vi "main4Ch v2.0.2.vi"() -> ()   [LabVIEW 2024]
doc: "Main VI for FLS imaging system."
uses:
  SubVI/DigitizerConfiguration/FLImDAQ.ctl
  <instrlib>/niScope/Controls/niScope trigger source.ctl
  SubVI/LabJack/LJ Pin Setting.ctl
  ConfigFiles/AimingBeamVideoConfig.ctl
  LaguerreDeconLib/DeconEngineClass/LaguerreDeconEngineClass.lvclass/LaguerreDeconEngineClass.ctl
  <vilib>/Utility/error.llb/DialogType.ctl
  LaguerreDeconLib/DeconEngineClass/LaguerreDeconEngineClass.lvclass
  <vilib>/event_ctls.llb/usereventprio.ctl
  <vilib>/Utility/miscctls.llb/LVMinMaxIncTypeDef.ctl
  SubVI/APD/APDClass.lvclass
  <vilib>/Analysis/baseanly.llb/Mean (DBL).vi
  SubVI/GlobalVariables.vi
  <vilib>/addons/control/pid/pid.llb/PID (DBL).vi
  <instrlib>/niScope/Acquire/Fetch/niScope Multi Fetch Binary 16.vi
  <vilib>/Instr/_visa.llb/VISA Configure Serial Port (Instr).vi
  <vilib>/Python/Open Anaconda Python Session.vi
  C:/Users/MarcuLab/Documents/GitHub/NetDeconForLV/Source/DotNETAssembly1.0.3/output/build/LaguerreDeconRTNative.dll
  Documents/GitHub/NetDeconForLV/Source/DotNETAssembly1.0.3/output/build/LaguerreDeconRTNative.dll
  <userlib>/_OpenG.lib/file/file.llb/openg_file.lvlib
  <userlib>/_OpenG.lib/time/time.llb/openg_time.lvlib
  <vilib>/Analysis/NI_AALBase.lvlib
  <vilib>/Utility/miscctls.llb/LVPointTypeDef.ctl
  <vilib>/addons/control/pid/NI_PID_pid.lvlib
panel:
  out "error out":errorcluster
  in  "488nm Power":u16(ring)=32 items=["3.30mW"=60, "2.35mW"=50, "2.00mW"=47, "1.75mW"=44, "1.48mW"=41, "1.16mW"=38, "0.87mW"=35, "0.57mW"=32, "0.28mW"=29]
  out "Decon Loop timing (ms)":dbl
  out "Ch3 Lifetime (ns)":dbl caption="Lifetime (ns)"
  out "Ch2 Lifetime (ns)":dbl caption="Lifetime (ns)"
  out "Ch1 Lifetime (ns)":dbl caption="Lifetime (ns)"
  out "Cancer Prob":dbl
  in  "Overlay selection":u16(ring) items=["Gain", "Lifetime", "CancerProbability"]
  out "Record Backlog 2":i32
  in  "Auto gain ch4":bool=TRUE caption="Auto gain ch3"
  in  "V 4":dbl caption="Gain 3" min=0.0 max=4.67 step=0.1
  out "Gain4":dbl
  out "IntR4":dbl format="%#_2g"
  out "SNR4":dbl format="%#_3g"
  out "Channel 4":dbl[][](graph) caption="Channel 3"
  out "RunStartTime":u32
  out "Dig1 Temp":dbl
  out "Dig2 Temp":dbl
  out "Visualization PC video source":T1
  in  "V target(1.0)":dbl=1.0 caption="V target(1.5)" min=0.3 max=1.5 step=0.1 format="%#_4g"
  out "SNR3":dbl format="%#_3g"
  out "SNR2":dbl format="%#_3g"
  out "SNR1":dbl format="%#_3g"
  in  "Show BG removed?":bool=TRUE
  out "IntR3":dbl format="%#_2g"
  out "IntR2":dbl format="%#_2g"
  out "IntR1":dbl format="%#_2g"
  in  "Video Display":bool
  out "Gain3":dbl
  out "Gain2":dbl
  out "Gain1":dbl
  in  "Skip Data Save?":bool
  out "Aq Loop?":bool
  out "ML?":bool
  out "aquisition loop Error Out":errorcluster
  out "Laser f (Hz)":dbl
  out "Record Backlog":i32
  out "Fetch Record #":i32
  out "Sync Success?":bool
  out "Disclamer":picture
  out "Calibration #":i8
  out "BG #":i8
  in  "TCP Connect":bool
  out "Help":string
  in  "355nm Laser toggle":bool caption="355nm 460Hz"
  in  "Cali&iRF alignment":bool
  in  "Background":bool
  in  "Aiming beam toggle":bool caption="488nm 0Hz"
  in  "Auto gain ch3":bool=TRUE
  in  "Auto gain ch2":bool=TRUE
  in  "Auto gain ch1":bool=TRUE
  out "Run #":i8
  in  "StopButton":bool caption="Stop"
  out "Aquisition Status:":bool
  in  "StartButton":bool caption="Start"
  in  "V 3":dbl caption="Gain 3" min=0.0 max=4.65 step=0.1
  in  "V 2":dbl caption="Gain 2" min=0.0 max=4.59 step=0.1
  in  "V 1":dbl caption="Gain 1" min=0.0 max=4.63 step=0.1 format="%#_4g"
  in  "Video Source":enum32{"Camera", "FrameGrabber"}(radio)
  out "Case #":string
  out "System Hardware Connection Status":T2
  out "Channel 3":dbl[][](graph)
  out "Channel 2":dbl[][](graph)
  out "Channel 1":dbl[][](graph)
  in  "Tab Control":T3(tab)
  out "display loop timing(ms)":u32
  out "Aquisition loop timing(ms)":u32 format="%.2f"
  out "DisplayLoop":i32
  out "PID loop":i32 caption="processing loop"
  out "PID loop timing(ms)":u32 caption="processing loop timing(ms)"
  out "Communication loop(ms)":u32
  out "laser EM lamp V":dbl format="%0.6f"
  out "Auisition Loop idx":i32
  out "LJ process (ms)":u32
  out "LJ time(ms)":u32[](array[numeric])
  out "output variable":i32
  out ".NetInitialized?":bool
  out "BG Graph":dbl[][](graph)
  out "Lifetime (ns)":cluster{dbl, dbl, dbl}(graph)
  out "DeCon Speed(ms)":dbl(graph)
  out "iRF Graph":dbl[][](graph)
  in  "Show BG":bool
  out "iRF length":i32
  out "BG length":i32
  out "data length":i32
  out "WarmupTime(ms)":u32
  out "BGAll":dbl[][](array[numeric])
  out "DeConOut":dbl[](array[numeric])
  in  "Ch1GainLim":dbl=350.0 format="%#_13g"
  in  "Ch2GainLim":dbl=1750.0 format="%#_13g"
  in  "Ch3GainLim":dbl=1750.0
  out "LJ Pinout":T4={"Ch1 Bias"="DAC0", "Ch2 Bias"="DAC1", "Ch3 Bias"="DAC2", "Ch4 Bias"="DAC0", "355 PWM"="FIO0", "AimingBeam PWM"="FIO2", "Laser Ready"="FIO3", "Interlock"="FIO1", "Laser Start/Stop"="FIO1", "Red LED"="FIO1", "Green LED"="DIO3", "Foot Pedal"="DIO15"}
  out "FLImDAQ":T5={"Digitizer 1"="", "Digitizer 2"="", "Channel"=enum."Channel 0", "trigger source"="VAL_EXTERNAL", "trigger level"=0.5, "trigger delay"=1.35e-07, "min sample rate"=12500000000.0, "min record length"=2500, "vertical range"=1.0, "vertical offset"=-0.25, "Waveform to Avg"=2000} caption="FLIm DAQ Configuration" {"trigger delay" format="%^#.4e"; "trigger level" min=0.0 max=3.5 step=0.5 format="%.2f"; "vertical offset" format="%.4f"; "vertical range" format="%.2f"; "min sample rate" format="%#.2p"}
  in  "Sys Reconfig":bool
  out "data out(communcation loop)":string
  out "PID loop error out":errorcluster caption="processing Error Out"
  out "decon error out":errorcluster
  out "Laser Rep Rate":dbl
  out "V4 Size":i32 caption="V3 Size"
  in  "Data Class":enum16{"Data", "BG", "Cali"}(ring)=enum."BG"
  out "V1 Size":i32
  out "V2 Size":i32
  out "V3 Size":i32
  out "data Size":i32[](array[numeric])
  out "State log":string
  out "SysConfigCluster":T7
  in  "Ch4 PID gains":T8={"proportional gain (Kc)"=30.0, "integral time (Ti, min)"=0.0003, "derivative time (Td, min)"=1e-05}
  in  "Ch3 PID gains":T8={"proportional gain (Kc)"=30.0, "integral time (Ti, min)"=0.0003, "derivative time (Td, min)"=1e-05}
  in  "Ch2 PID gains":T8={"proportional gain (Kc)"=30.0, "integral time (Ti, min)"=0.0003, "derivative time (Td, min)"=1e-05}
  in  "Ch1 PID gains":T8={"proportional gain (Kc)"=30.0, "integral time (Ti, min)"=0.0003, "derivative time (Td, min)"=1e-05}
  in  "Brain model path":path=path "C:/Users/MarcuLab/Desktop/V6 APD LV/V6 APD LV/ClassifierFile/Brain_Agnostic_Model.pkl"
  in  "module path":path=path "C:/Users/MarcuLab/Documents/GitHub/NetDeconForLV/Classifier/ClassifierModule.py"
  in  "HN model path":path=path "C:/Users/MarcuLab/Desktop/V6 APD LV/V6 APD LV/ClassifierFile/xgb_model.pkl"
  in  "Env name":string="HNClassifier"
  in  "Python version":string="3.10"
  out "Python session":refnum<k35>
  out "OverlaySelection":T9(ring)=enum."HN Classifier"
  in  "CancerThreshold":dbl=0.15
  in  "Quit":bool
  in  "Radio Buttons":T10(radio)=enum."Ch2" caption="DeCon Chan"
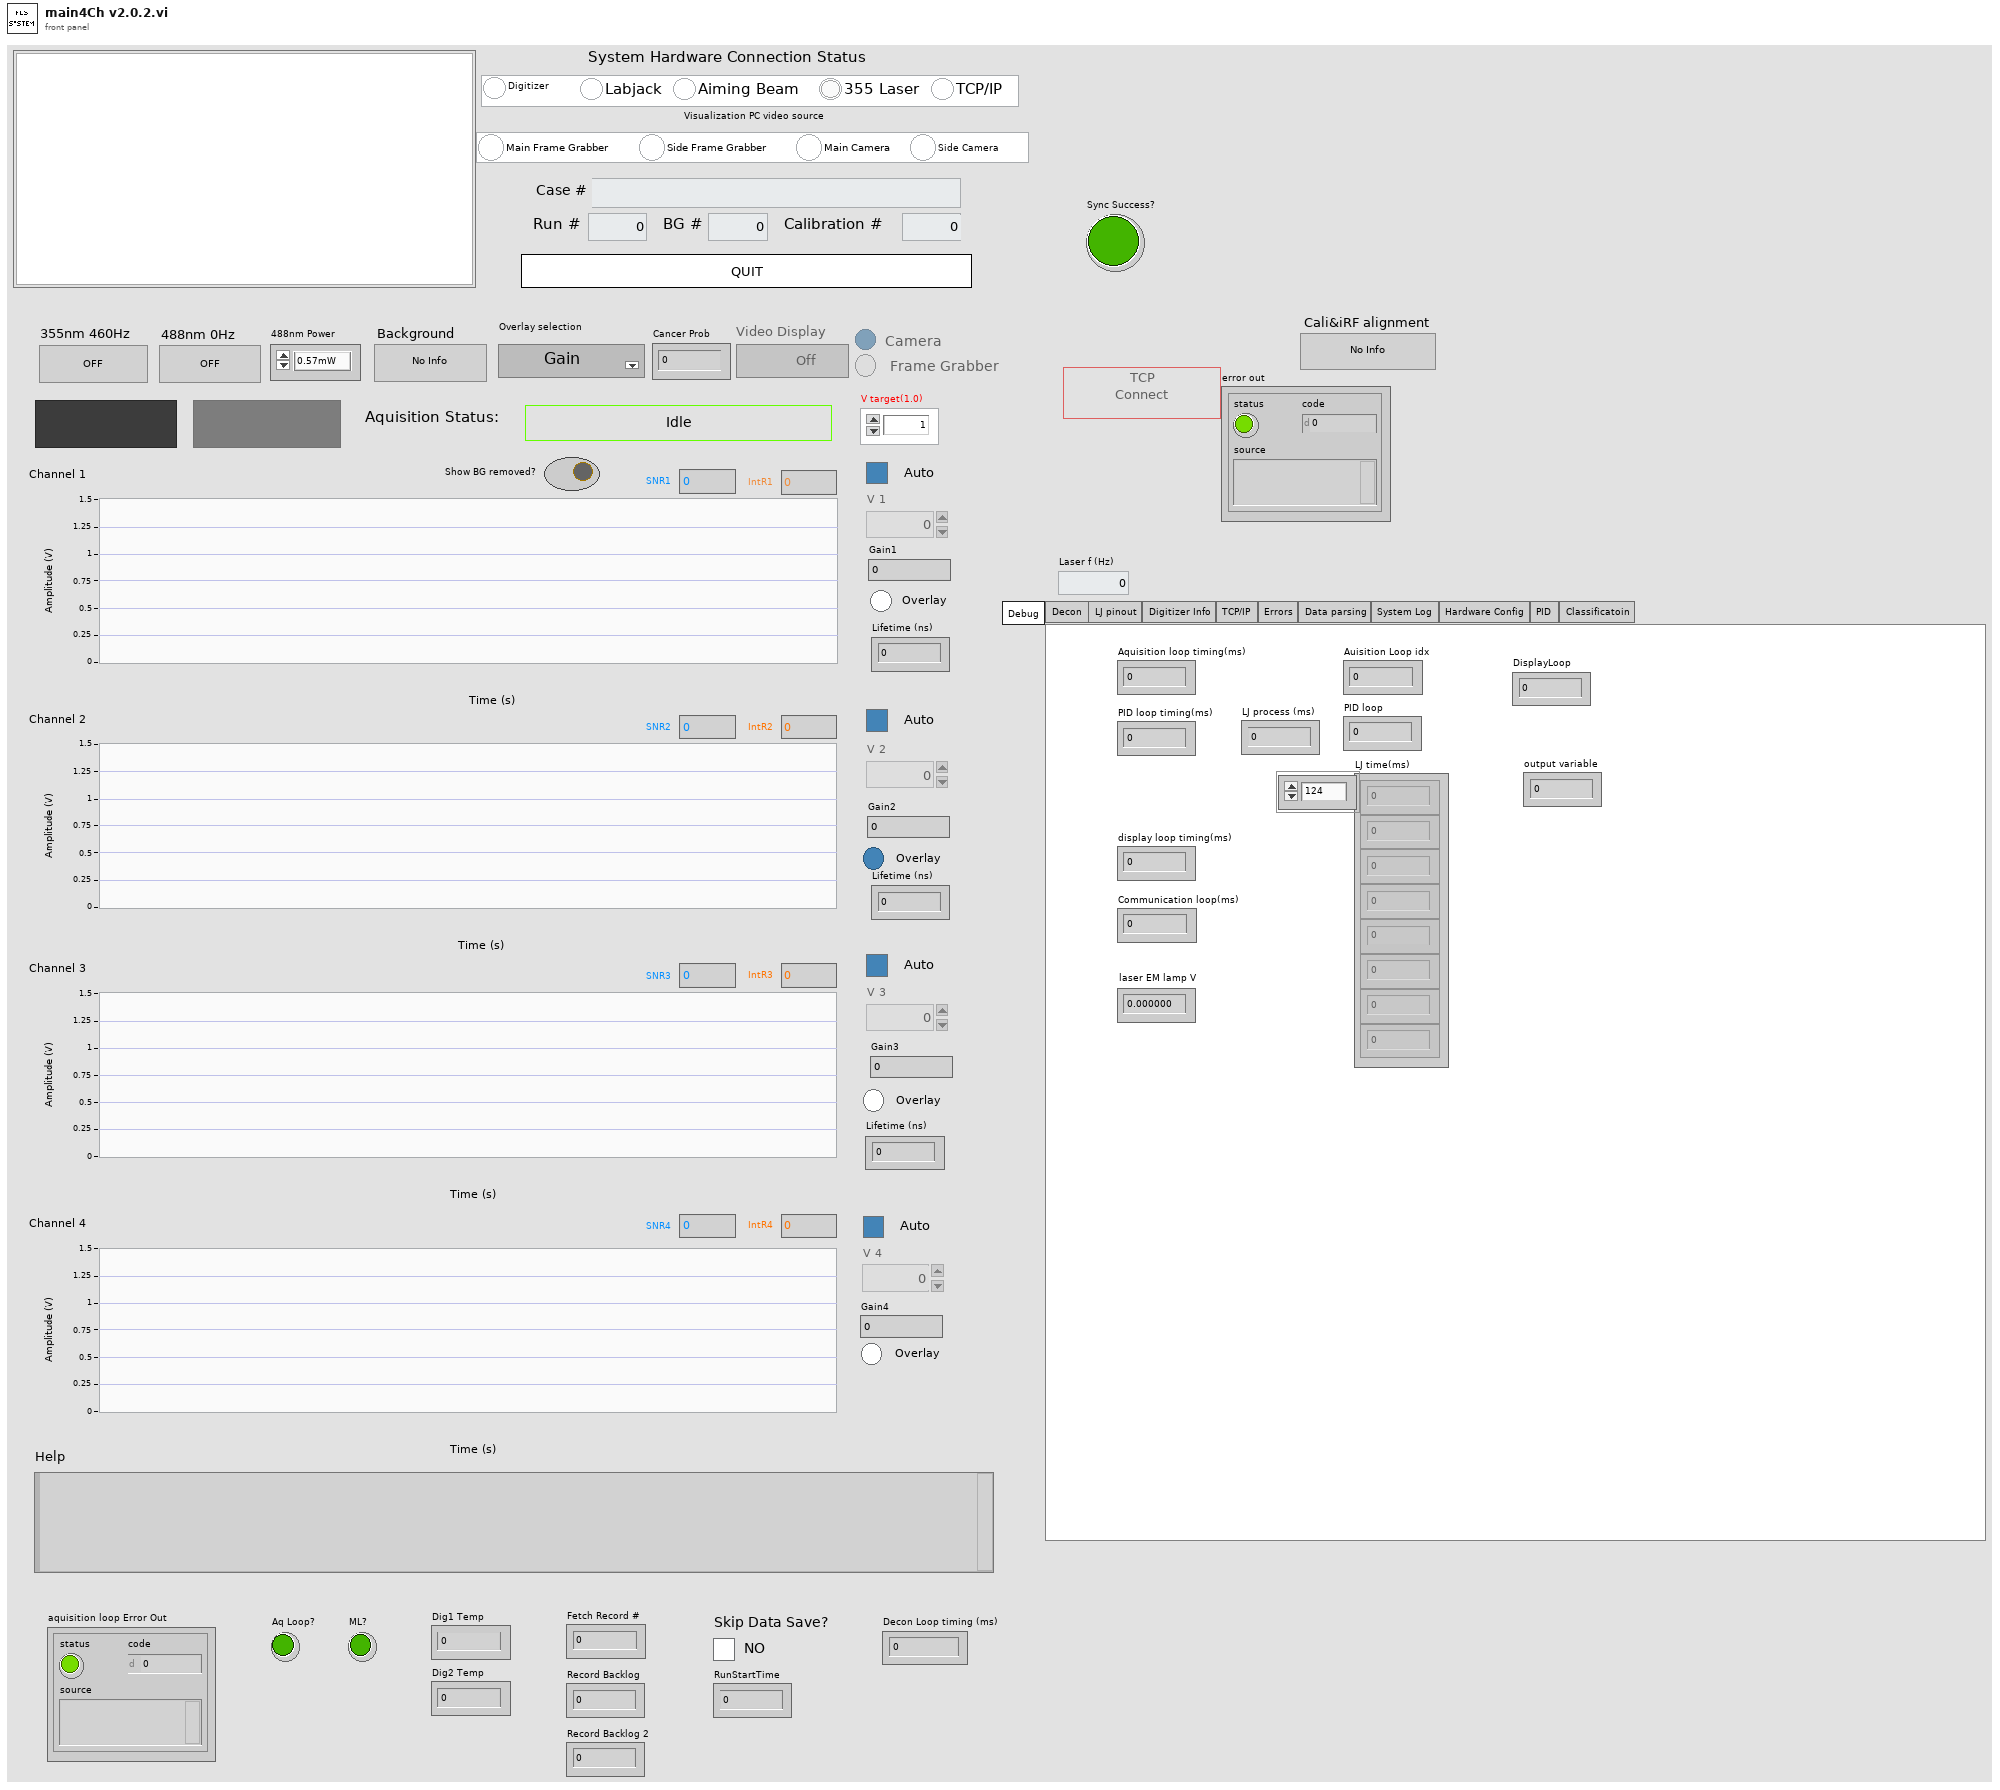
[diagram p1: front panel]
types:
  T1 = cluster{"Main Frame Grabber":bool, "Side Frame Grabber":bool, "Main Camera":bool, "Side Camera":bool}
  T2 = cluster{"Digitizer":bool, "Labjack":bool, "Aiming Beam":bool, "355 Laser":bool, "TCP/IP":bool}
  T3 = enum32{"Debug", "Decon", "LJ pinout", "Digitizer Info", "TCP/IP", "Errors", "Data parsing", "System Log", "Hardware Config", "PID", "Classificatoin"}
  T4 = typedef "LJ Pin Setting.ctl" = cluster{"Ch1 Bias":string, "Ch2 Bias":string, "Ch3 Bias":string, "Ch4 Bias":string, "355 PWM":string, "AimingBeam PWM":string, "Laser Ready":string, "Interlock":string, "Laser Start/Stop":string, "Red LED":string, "Green LED":string, "Foot Pedal":string}
  T5 = typedef "FLImDAQ.ctl" = cluster{"Digitizer 1":refnum<k15>, "Digitizer 2":refnum<k15>, "Channel":enum16{"Channel 0", "Channel 1", "Channel 0&1"}, "trigger source":T6, "trigger level":dbl, "trigger delay":dbl, "min sample rate":dbl, "min record length":i32, "vertical range":dbl, "vertical offset":dbl, "Waveform to Avg":i16}
  T6 = typedef "niScope trigger source.ctl" = string
  T7 = cluster{"Ch1Enable?":bool, "Ch2Enable?":bool, "Ch3Enable?":bool, "Ch1AutoGain?":bool, "Ch2AutoGain?":bool, "Ch3AutoGain?":bool, "AimingBeamEnable?":bool}
  T8 = cluster{"proportional gain (Kc)":dbl, "integral time (Ti, min)":dbl, "derivative time (Td, min)":dbl}
  T9 = enum16{"Gain", "HN Classifier", "Brain Classifier", "Window Close"}
  T10 = enum32{"No Selection", "Ch1", "Ch2", "Ch3", "Ch4"}
  T11 = cluster{"idx":i32, "CH1&2":dbl[][], "CH3&4":dbl[][], "V cluster":cluster{"V1":dbl, "V2":dbl, "V3":dbl, "V4":dbl}}
  T12 = cluster{"remote start event":refnum<user-event>, "remote stop  event":refnum<user-event>}
  T13 = enum8{"Enabled", "Disabled", "Disabled and Grayed Out"}
  T14 = enum16{"open", "replace", "create", "open or create", "replace or create", "replace or create with confirmation"}
  T15 = cluster{"CH1":dbl[][], "CH2":dbl[][], "CH3":dbl[][], "CH4":dbl[][], "Gain cluster":cluster{"V1":dbl, "V2":dbl, "V3":dbl, "V4":dbl}}
  T16 = enum16{"open", "open or create", "create or replace", "create", "open (read-only)"}
  T17 = cluster{"Ch1 iRF":dbl[], "Ch2 iRF":dbl[], "Ch3 iRF":dbl[], "Ch4 iRF":dbl[]}
  T18 = enum32{"Invalid", "Standard", "Closed", "Hidden", "Minimized", "Maximized"}
  T19 = enum32{"invalid app kind", "Development System", "Run Time System", "Student Edition", "Embedded LabVIEW", "Evaluation", "Custom"}
  T20 = typedef "usereventprio.ctl" = enum32{"high priority", "normal priority"}
  T21 = enum32{"Bad", "Idle", "Run top level", "Running"}
  T22 = enum16{"Standard", "Buffered", "CRLF", "Immediate"}
  T23 = typedef "AimingBeamVideoConfig.ctl" = cluster{"DeCon Channel":enum16{"1", "2", "3"}, "Scale Bar":bool, "Scale Low":dbl, "Scale High":dbl, "ANSI":dbl, "Radius":dbl, "3D?":bool, "Firefly?":bool, "Pentero?":bool}
  T24 = cluster{"Core":cluster{"Current VI Reference":refnum<vi>, "Close Panel on Exit?":bool}, "SysConfigCluster":cluster{"Ch1Enable?":bool, "Ch2Enable?":bool, "Ch3Enable?":bool, "Ch1AutoGain?":bool, "Ch2AutoGain?":bool, "Ch3AutoGain?":bool, "AimingBeamEnable?":bool}, "System Status":cluster{"Digitizer":bool, "Labjack":bool, "Aiming Beam":bool, "355 Laser":bool, "TCP/IP":bool}, "IDs":cluster{"RunID":i8, "BG ID":i8, "Cali ID":i8}, "CaseID":string, "DefaultPath":path, "Pathes":cluster{"DataPath":path, "BG Path":path, "iRFPath":path, "CaliPath":path}, "FLImDAQ":cluster{"resource name":refnum<k15>, "resource name 2":refnum<k15>, "Channel":enum16{"Channel 0", "Channel 1", "Channel 0&1"}, "trigger source":T6, "trigger level":dbl, "trigger delay":dbl, "min sample rate":dbl, "min record length":i32, "vertical range":dbl, "vertical offset":dbl, "Waveform to Avg":i32}, "SysRunning?":bool, "AB Cluster":cluster{"Aiming Beam COM Port":refnum<visa-resource-name>, "Min Current":dbl, "Max Current":dbl, "Default Current":dbl, "Freq":i32}, "LJ Pinout":T4, "355 PWM setting":cluster{"DIO_EF_CLOCK1_DIVISOR":i16, "DIO_EF_CLOCK1_ROLL_VALUE":i32, "DIO#_EF_INDEX":i16, "DIO#_EF_OPTIONS":i16, "DIO#_EF_CONFIG_A":i32}, "AB PWM setting":cluster{"DIO_EF_CLOCK1_DIVISOR":i16, "DIO_EF_CLOCK1_ROLL_VALUE":i32, "DIO#_EF_INDEX":i16, "DIO#_EF_OPTIONS":i16, "DIO#_EF_CONFIG_A":i32}, "Last Trigger":u32, "niTClk sessions":refnum<k20>[], "Laser start tic":u32, "TCP attempt count":i32, "Ch1Data":dbl[][], "Ch2Data":dbl[][], "Ch3Data":dbl[][], "Ch4Data":dbl[][], "V1":dbl[], "V2":dbl[], "V3":dbl[], "V4":dbl[], "SlowTimer":u32, "FastTimer":u32, "listener ID":refnum<k5>, "TempPath":path, "CaliPath":path, "LED vi reference":refnum<vi>, "Aquisition Timer":u32, "APDSerialNum":cluster{"Ch1APDSerial#":string, "Ch2APDSerial#":string, "Ch3APDSerial#":string, "Ch4APDSerial#":string}, "VideoConfig":T23, "LED vi ref open?":bool, "video source":cluster{"Main Frame Grabber":bool, "Side Frame Grabber":bool, "Main Camera":bool, "Side Camera":bool}, "bothVidSourceAvail":bool, "OverlaySelection":u16}
  T25 = typedef "LVCursorListTypeDef.ctl" = cluster{"Name":string, "Color":u32, "Style":u8, "Point Style":u8, "Name Visible":bool, "Allow Drag":bool, "Cursor Mode":u32, "Plot":i32, "Index":i32, "Position":cluster{"X":dbl, "Y":dbl}, "X Scale":u32, "Y Scale":u32, "Watch Plots":i32[], "Watch All Plots":bool, "Plot Area":i32, "Label Offset":cluster{"X":dbl, "Y":dbl}}[]
  T26 = cluster{"Name":string, "Color":u32, "Style":u8, "Point Style":u8, "Name Visible":bool, "Allow Drag":bool, "Cursor Mode":u32, "Plot":i32, "Index":i32, "Position":cluster{"X":dbl, "Y":dbl}, "X Scale":u32, "Y Scale":u32, "Watch Plots":i32[], "Watch All Plots":bool, "Plot Area":i32, "Label Offset":cluster{"X":dbl, "Y":dbl}}
  T27 = cluster{"Ch1APDSerial#":string, "Ch2APDSerial#":string, "Ch3APDSerial#":string, "Ch4APDSerial#":string}
  T28 = cluster{"DataPath":path, "BG Path":path, "iRFPath":path, "CaliPath":path}
  T29 = cluster{"DIO_EF_CLOCK1_DIVISOR":i16, "DIO_EF_CLOCK1_ROLL_VALUE":i32, "DIO#_EF_INDEX":i16, "DIO#_EF_OPTIONS":i16, "DIO#_EF_CONFIG_A":i32}
  T30 = cluster{"Aiming Beam COM Port":refnum<visa-resource-name>, "Min Current":dbl, "Max Current":dbl, "Default Current":dbl, "Freq":i32}
  T31 = cluster{"resource name":refnum<k15>, "resource name 2":refnum<k15>, "Channel":enum16{"Channel 0", "Channel 1", "Channel 0&1"}, "trigger source":T6, "trigger level":dbl, "trigger delay":dbl, "min sample rate":dbl, "min record length":i32, "vertical range":dbl, "vertical offset":dbl, "Waveform to Avg":i32}
  T32 = cluster{"Current VI Reference":refnum<vi>, "Close Panel on Exit?":bool}
  T33 = cluster{"Channel 1":dbl[], "Channel 2":dbl[], "Channel 3":dbl[], "Channel 4":dbl[]}
  T34 = cluster{"V 1":dbl[], "V 2":dbl[], "V 3":dbl[], "V 4":dbl[]}
  T35 = cluster{"Ch1 WF":dbl[], "Ch2 WF":dbl[], "Ch3 WF":dbl[], "Ch4 WF":dbl[], "V1":dbl, "V2":dbl, "V3":dbl, "V4":dbl}
  T36 = typedef "iRFData.ctl" = cluster{"dt":dbl, "NumOfWFs":i32, "WFLength":i32, "iRFCtrlV":dbl[], "iRFWFsAvg":dbl[][], "iRFRaw":dbl[][]}
  T37 = cluster{"mean":dbl, "mean":dbl, "mean":dbl, "mean":dbl}
  T38 = cluster{"V1":dbl, "V2":dbl, "V3":dbl, "V4":dbl}[]
  T39 = cluster{"DataPath":path, "CaseID":string, "RunID":i16, "Ch1Data":dbl[][], "Ch2Data":dbl[][], "Ch3Data":dbl[][], "Ch4Data":dbl[][], "V1":dbl[], "V2":dbl[], "V3":dbl[], "V4":dbl[], "LaserRepRate":u16, "WFAverage":i16, "RunStartTime":u64}
  T40 = typedef "DialogType.ctl" = u16
  T41 = typedef "APD.ctl" = cluster{"gainV":dbl[], "gain":dbl[], "irfV":dbl[], "irfTNorm":dbl[][]}
  T42 = typedef "LJ PWM Setting.ctl" = cluster{"DIO_EF_CLOCK1_DIVISOR":i16, "DIO_EF_CLOCK1_ROLL_VALUE":i32, "DIO#_EF_INDEX":i16, "DIO#_EF_OPTIONS":i16, "DIO#_EF_CONFIG_A":i32}
  T43 = typedef "AimingBeam.ctl" = cluster{"Aiming Beam COM Port":refnum<visa-resource-name>, "Min Current":dbl, "Max Current":dbl, "Default Current":dbl, "Frequency(Hz)":u32}
  T44 = cluster{"DC1":i32, "DC2":i32, "BG1":i32, "BG2":i32}
  T45 = typedef "LVMinMaxIncTypeDef.ctl" = cluster{"Minimum":dbl, "Maximum":dbl, "Increment":dbl}
  T46 = typedef "LVBoundsTypeDef.ctl" = cluster{"Width":u32, "Height":u32}
  T47 = typedef "imagedata.ctl" = cluster{"image type":i32, "image depth":i32, "image":u8[], "mask":u8[], "colors":u32[], "Rectangle":cluster{"left":i16, "top":i16, "right":i16, "bottom":i16}}
  T48 = enum16{"Left Button", "Center Button", "Right Button", "Window Close"}
  T49 = cluster{"DC Idx1":i32, "DC Idx2":i32, "BG Idx1":i32, "BG Idx2":i32}
  T50 = cluster{dbl[][], dbl[][], dbl[][], dbl[][], "V cluster":cluster{"V1":dbl, "V2":dbl, "V3":dbl, "V4":dbl}}
  T51 = cluster{"V1 out":dbl, "V2 out":dbl, "V3 out":dbl, "V3 out":dbl}
  T52 = cluster{"actualSamples":i32, "absoluteInitialX":dbl, "relativeInitialX":dbl, "xIncrement":dbl, "offset":dbl, "gain":dbl, "reserved1":dbl, "reserved2":dbl}[]
  T53 = cluster{i32, dbl[][], dbl[][], cluster{"V1 out":dbl, "V2 out":dbl, "V3 out":dbl, "V3 out":dbl}}
  T54 = typedef "LVPointTypeDef.ctl" = cluster{"Horizontal":i16, "Vertical":i16}
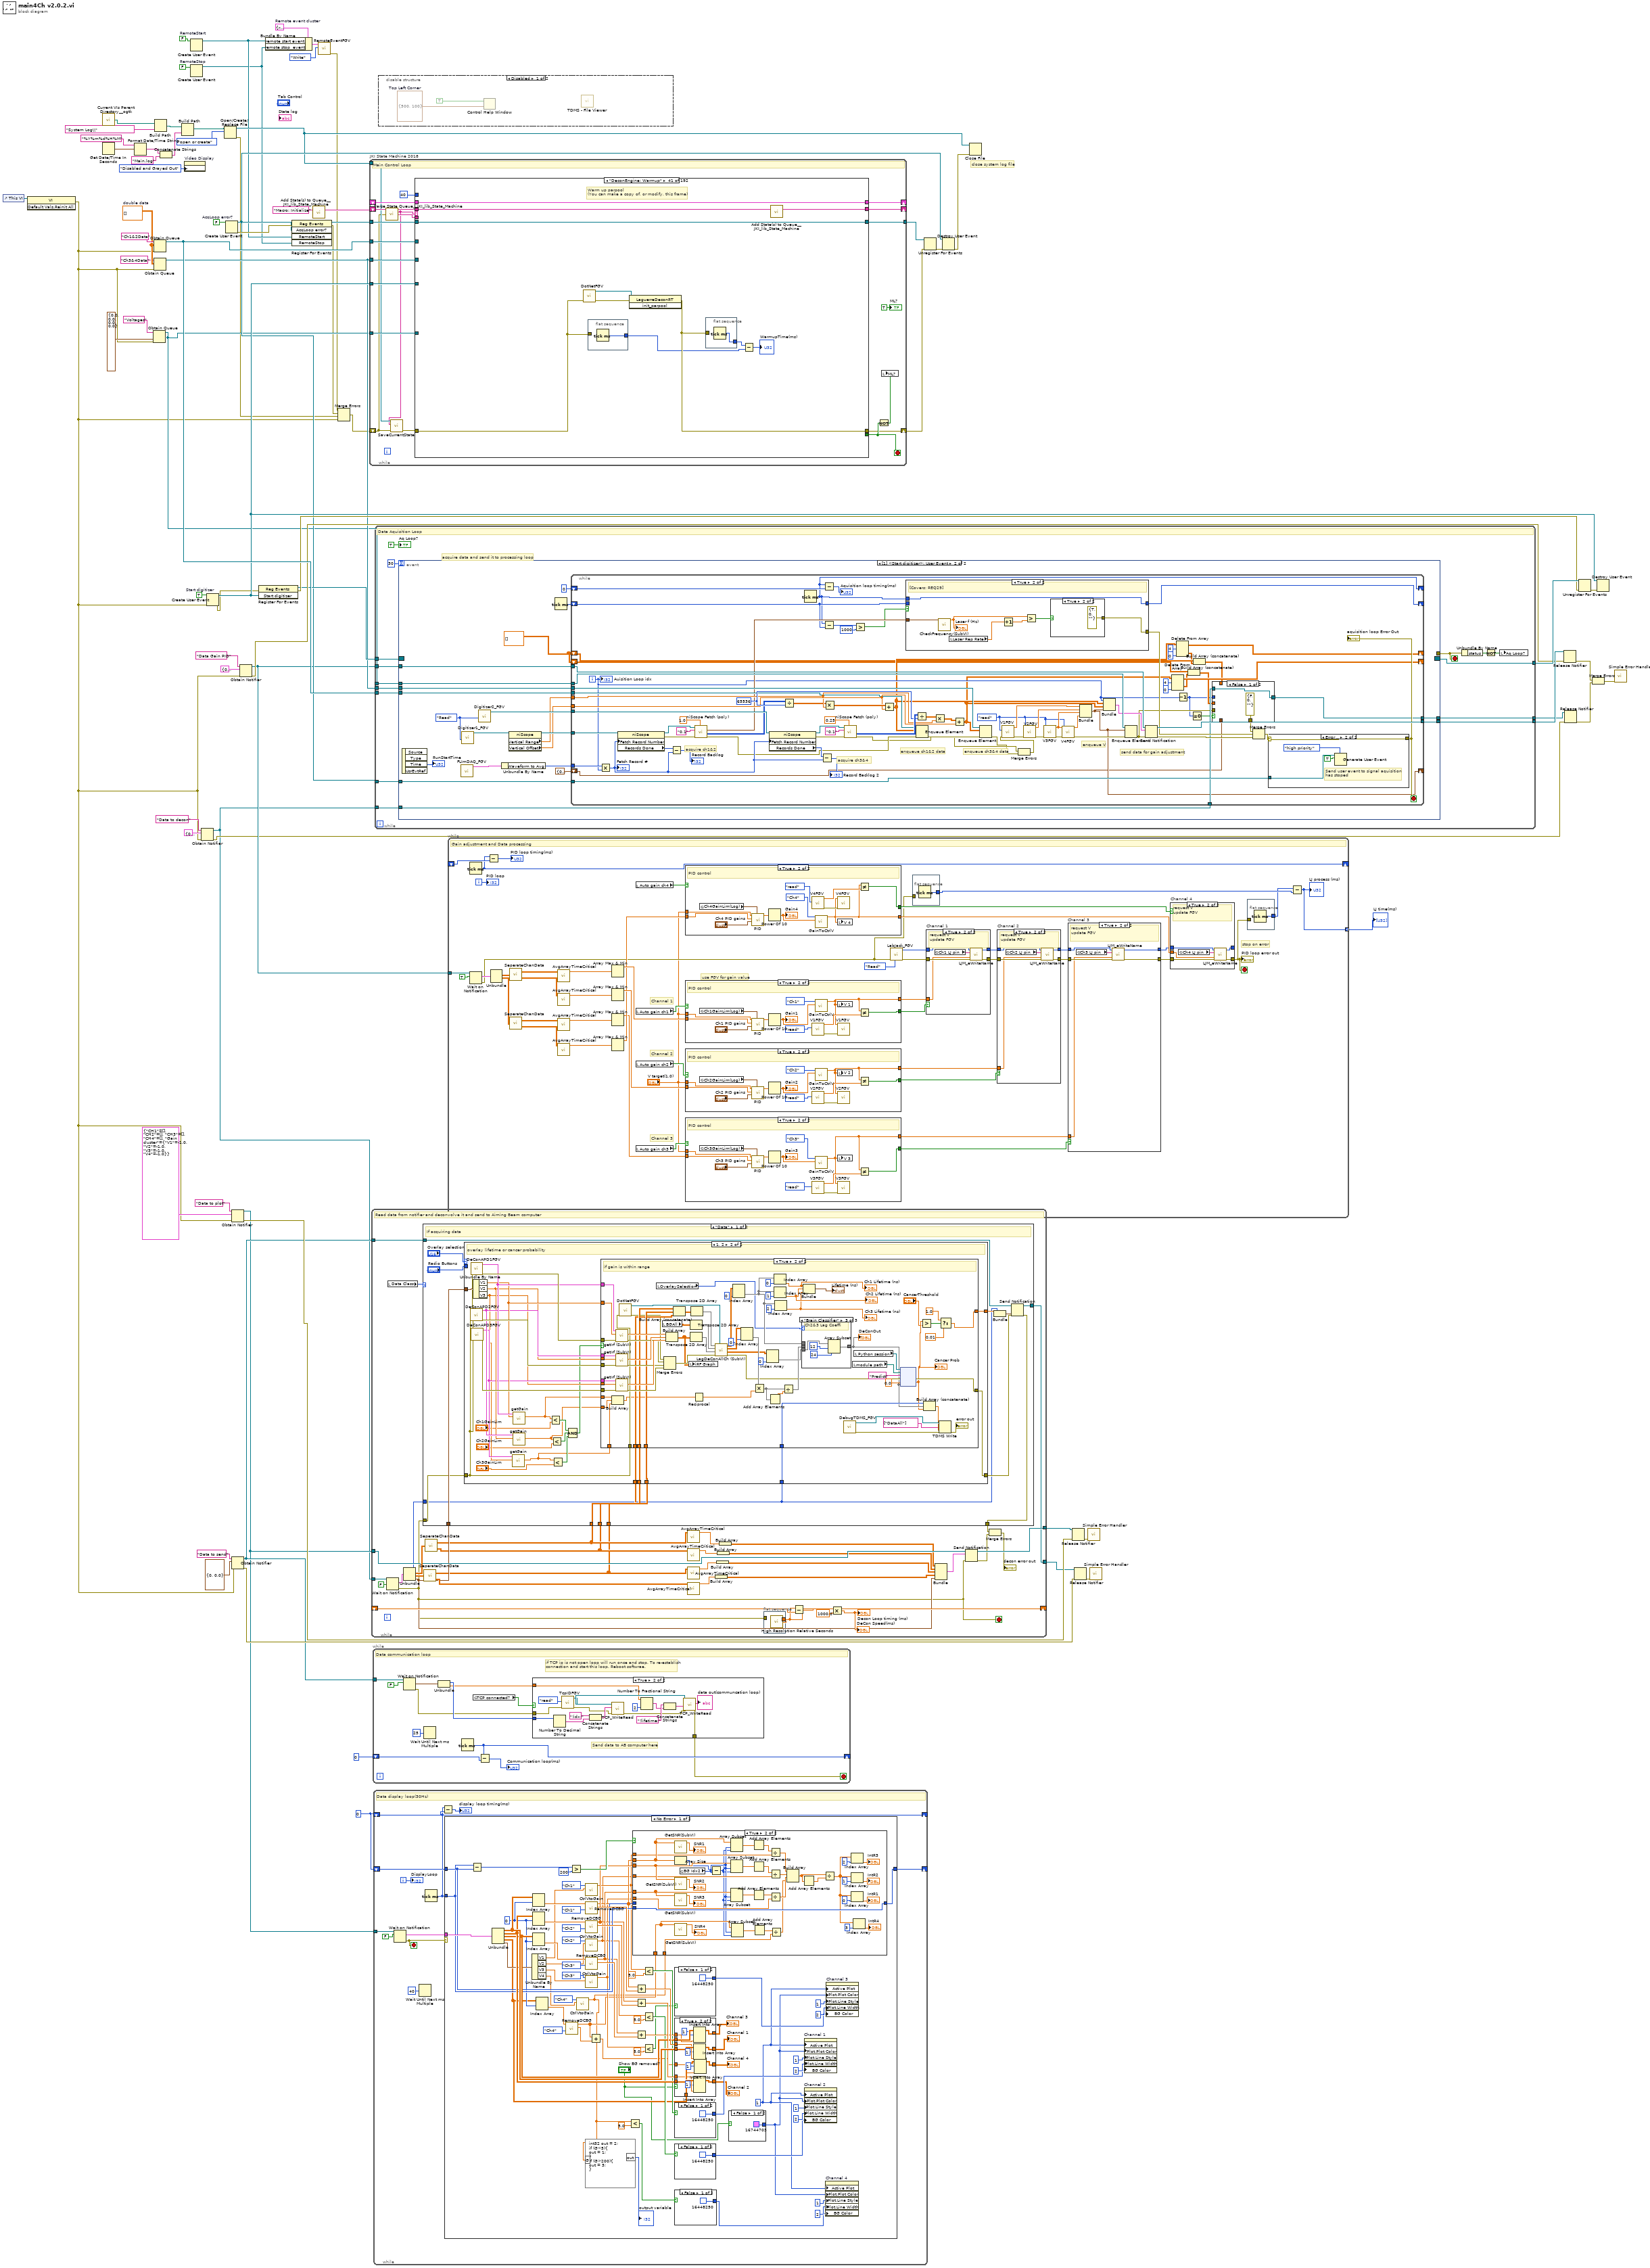
[diagram p0: block diagram]
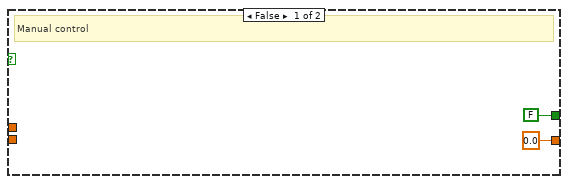
[diagram p6: hidden frame]
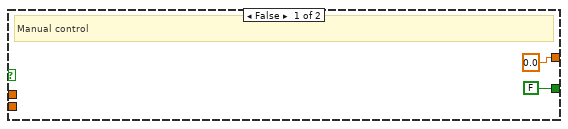
[diagram p7: hidden frame]
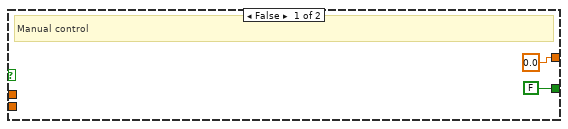
[diagram p8: hidden frame]
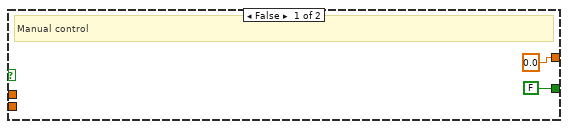
[diagram p9: hidden frame]
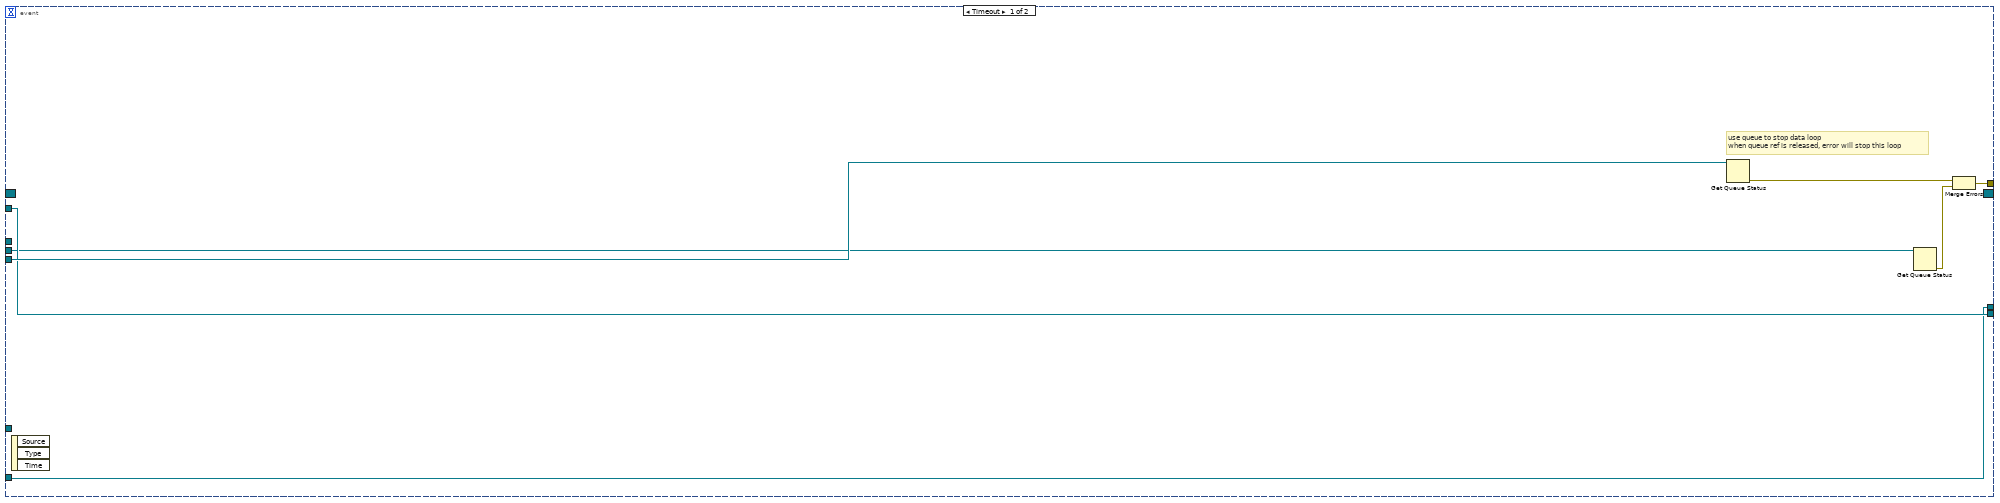
[diagram p10: hidden frame]
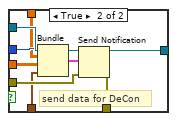
[diagram p11: hidden frame]
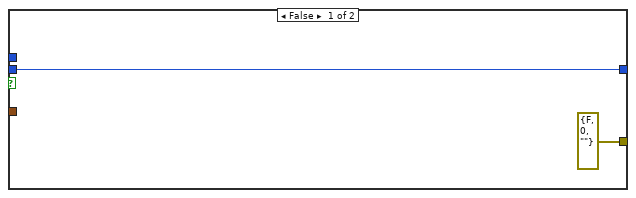
[diagram p12: hidden frame]
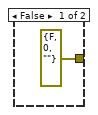
[diagram p13: hidden frame]
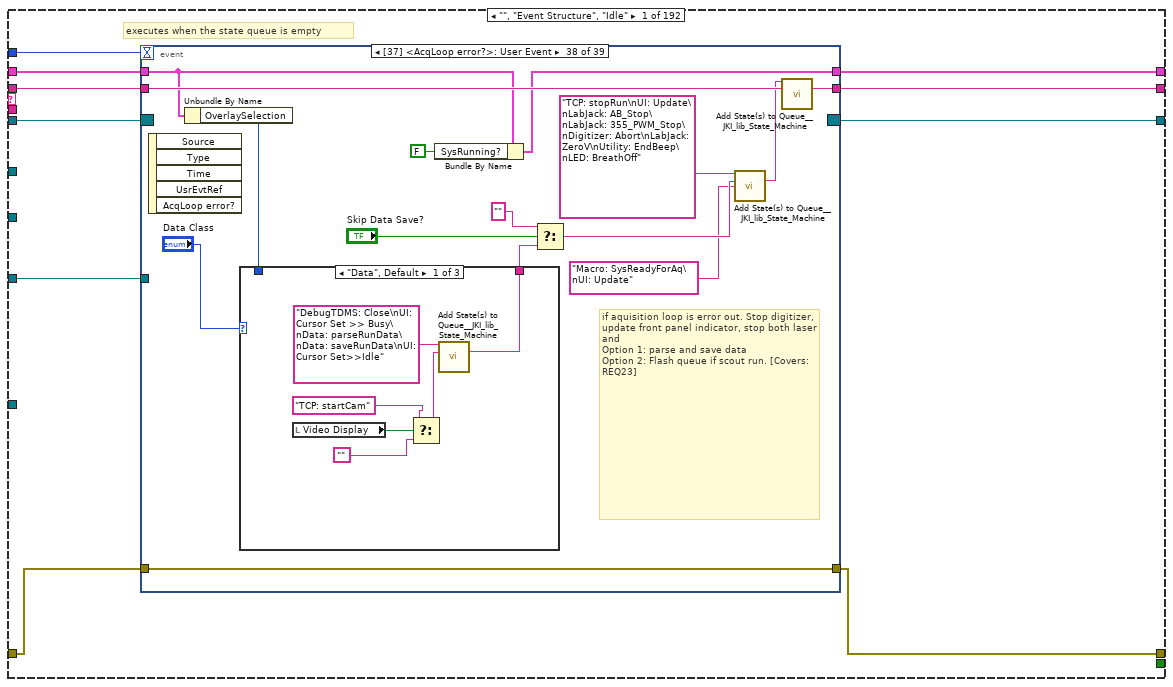
[diagram p15: hidden frame]
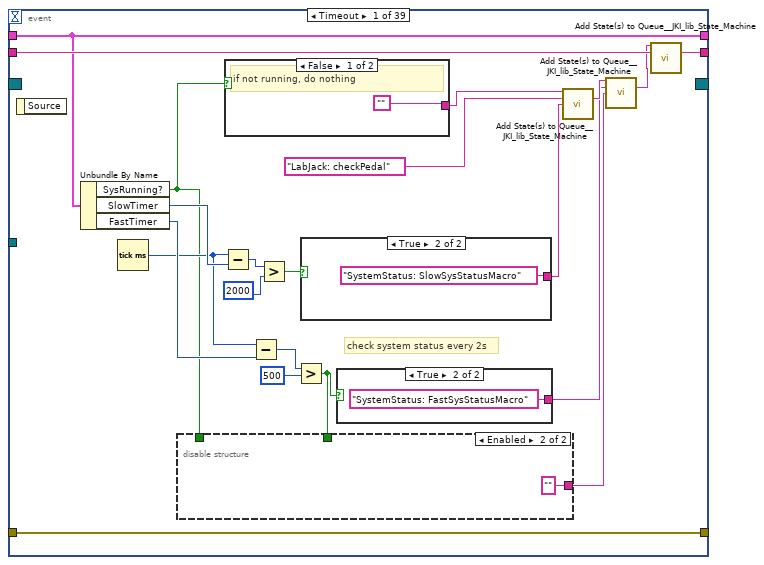
[diagram p16: hidden frame]
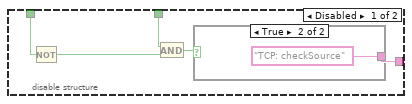
[diagram p17: hidden frame]
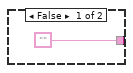
[diagram p18: hidden frame]
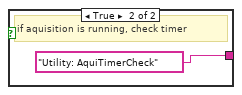
[diagram p19: hidden frame]
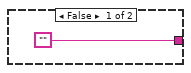
[diagram p20: hidden frame]
diagram:
  w18 = T12 {"remote start event"=refnum, "remote stop  event"=refnum}  # Remote event cluster
  w21 = FALSE  # RemoteStop
  w22 = FALSE  # RemoteStart
  w24 = u32 0 ("millisecond timer value")
  w62 = FALSE  # AcqLoop error?
  w71 = TRUE  # Start digitizer
  w74 = dbl[][] []  # double data
  # "close system log file"
  n1 = control-ref of="This VI"() -> (w76:refnum<vi>)
  n2 = invoke on="Invoke Node" class="VI" method="Default Vals.Reinit All"(reference=w76) -> (error out=w8:errorcluster)  [unwired: 2 in, 2 out]
  n3 = call <userlib>:"Current VIs Parent Directory__ogtk.vi"() -> ("Parent Directory (+ Relative)"=w42:path)  [unwired: 5 in]
  n4 = Get Date/Time In Seconds() -> (seconds since 1Jan1904=w40:timestamp)
  n5 = Format Date/Time String(time format string (%c)="%Y%m%d%H%M", seconds (now)=w40) -> (date/time string=w37:string)  [unwired: 1 in]
  n6 = Obtain Queue(name (unnamed)="Voltages", element data type=cluster{"V1":dbl, "V2":dbl, "V3":dbl, "V4":dbl} {"V1"=0.0, "V2"=0.0, "V3"=0.0, "V4"=0.0}, error in (no error)=w8) -> (queue out=w43:refnum<queue>)  [unwired: 2 in, 2 out]
  n7 = Obtain Queue(name (unnamed)="Ch3&4Data", element data type=w74, error in (no error)=w8) -> (queue out=w56:refnum<queue>)  [unwired: 2 in, 2 out]
  n8 = Obtain Queue(name (unnamed)="Ch1&2Data", element data type=w74, error in (no error)=w8) -> (queue out=w72:refnum<queue>)  [unwired: 2 in, 2 out]
  n9 = Build Path(base path=w42, name or relative path="System Log\\") -> (appended path=w33:path)
  n10 = Concatenate Strings(w37, "Main.log" ("string")) -> (w35:string)
  n11 = Build Path(base path=w33, name or relative path=w35) -> (appended path=w38:path)
  n12 = property on="Video Display" class="Bool (strict)"("DisabledEnum"=T13."Disabled and Grayed Out" ("Disabled")) -> ()  [unwired: 2 in, 2 out]
  n13 = Create User Event(user event datatype=w22) -> (user event=w20:refnum<user-event>)  [unwired: 1 in, 1 out]
  n14 = Create User Event(user event datatype=w21) -> (user event=w19:refnum<user-event>)  [unwired: 1 in, 1 out]
  n15 = Obtain Notifier(name (unnamed)="Data to decon", notification data type=T11 {"idx"=0, "CH1&2"=[], "CH3&4"=[], "V cluster"={"V1"=0.0, "V2"=0.0, "V3"=0.0, "V4"=0.0}}, error in (no error)=w8) -> (notifier out=w2:refnum<notifier>, error out=w6:errorcluster)  [unwired: 1 in, 1 out]
  n16 = Create User Event(user event datatype=w71, error in=w8) -> (user event=w61:refnum<user-event>, error out=w48:errorcluster)
  n17 = Open/Create/Replace File(file path (use dialog)=w38, operation (0:open)=T14."open or create") -> (refnum out=w30:refnum<file>, error out=w31:errorcluster)  [unwired: 4 in, 1 out]
  n18 = Create User Event(user event datatype=w62) -> (user event=w47:refnum<user-event>, error out=w49:errorcluster)  [unwired: 1 in]
  n19 = Obtain Notifier(name (unnamed)="Data to plot", notification data type=T15 {"CH1"=[], "CH2"=[], "CH3"=[], "CH4"=[], "Gain cluster"={"V1"=-1.0, "V2"=-1.0, "V3"=-1.0, "V4"=-1.0}}, error in (no error)=w8) -> (notifier out=w7:refnum<notifier>, error out=w57:errorcluster)  [unwired: 1 in, 1 out]
  n20 = Obtain Notifier(name (unnamed)="Data to send", notification data type=cluster{"idx":i32, "lifetime":dbl} {"idx"=0, "lifetime"=0.0}, error in (no error)=w8) -> (notifier out=w27:refnum<notifier>, error out=w46:errorcluster)  [unwired: 1 in, 1 out]
  n21 = Obtain Notifier(name (unnamed)="Data Gain PID", notification data type=T11 {"idx"=0, "CH1&2"=[], "CH3&4"=[], "V cluster"={"V1"=0.0, "V2"=0.0, "V3"=0.0, "V4"=0.0}}, error in (no error)=w8) -> (notifier out=w28:refnum<notifier>, error out=w65:errorcluster)  [unwired: 1 in, 1 out]
  n22 = register-events(error in=w48, w61) -> (reference out=w63:refnum<event-registration>, error out=w68:errorcluster)  [unwired: 1 in]
  n23 = Bundle By Name(cluster=w18, "remote start event"=w20, "remote stop  event"=w19) -> (w16:T12)
  n24 = register-events(error in=w49, w47, w20, w19) -> (reference out=w55:refnum<event-registration>, error out=w15:errorcluster)  [unwired: 1 in]
  n25 = call <vilib>:"Add State(s) to Queue__JKI_lib_State_Machine.vi"("State(s) in (\"\")"="Macro: Initialize") -> ("States Out"=w78:string)  [unwired: 14 in]
  n26 = call "RemoteEventFGV.vi"("Operation (Read)"=enum16{"Read", "Write"}."Write", "Remote Event in"=w16) -> ("Error Out"=w12:errorcluster)  [unwired: 8 in, 1 out]
  n27 = Merge Errors(w12, w15, w31, w8) -> (w32:errorcluster)
  n28 = while "JKI State Machine 2018" {
    shift-right: [w95] -> _
    shift-left: _ -> [w94]
    shift-right: [w79] -> w14
    shift-left: w32 -> [w81]
    shift-right: [w96] -> _
    shift-left: w78 -> [w97]
    tunnel: w72 -> [w92]
    tunnel: w56 -> [w91]
    tunnel: w61 -> [w90]
    tunnel: w55 -> [w89]
    tunnel: [w88] -> w54
    tunnel: w43 -> [w84]
    tunnel: w30 -> [w83]
    stop <- w87 stop-if-true
    # "Main Control Loop"
    n29 = call <vilib>:"Parse State Queue__JKI_lib_State_Machine.vi"("State Queue"=w97, "Error In (no error)"=w81) -> ("Remaining States"=w99:string, "Current State"=w82:string, "Arguments"=w98:string)  [unwired: 11 in]
    n30 = call "SaveCurrentState.vi"("error in (no error)"=w81, "Current State"=w82, "Byte Stream File in"=w83) -> ("error out"=w80:errorcluster)  [unwired: 8 in]
    n31 = case shown="\"DeconEngine: Warmup\"" w82 {
      selector: w82 -> [_ _ _ _ _ _ _ _ _ _ _ _ _ _ _ _ _ _ _ _ _ _ _ _ _ _ _ _ w1169 _ _ _ _ _ _ _ _ _ _ _ _ _ _ _ _ _ _ _ _ _ _ _ _ _ _ _ _ _ _ _ _ _ _ _ _ _ _ _ _ _ _ _ _ _ _ _ _ _ _ _ _ _ _ _ _ _ _ _ _ _ _ _ _ _ _ _ _ _ _ _ _ _ _ _ _ _ _ _ _ _ _ _ _ _ _ _ _ _ _ _ _ _ _ _ _ _ _ _ _ _ _ _ _ _ _ _ _ _ _ _ _ _ _ _ _ _ _ _ _ _ _ _ _ _ _ _ _ _ _ _ _ _ _ _ _ _ _ _ _ _ _ _ _ _ _ _ _ _ _ _ _ _ _ _ _ _ _ _ _ _ _ _]
      tunnel: w99 -> [w109 w529 w538 w544 w551 w559 w584 w599 w642 w648 w675 w700 w712 w783 w798 w829 w856 w888 w907 w936 w966 w983 w988 w1073 w1110 w1149 w1162 w1167 w1173 w1201 w1209 w1232 w1237 w1250 w1269 w1297 w1325 w1363 w1368 w1377 w1389 w1419 w1427 w1433 w1457 w1481 w1505 w1529 w1534 w1551 w1598 w1620 w1636 w1651 w1671 w1676 w1688 w1717 w1743 w1755 w1793 w1806 w1812 w1823 w1835 w1866 w1879 w1893 w1908 w1927 w1962 w1967 w1981 w1991 w2007 w2019 w2031 w2059 w2074 w2079 w2091 w2103 w2108 w2116 w2124 w2133 w2142 w2147 w2155 w2164 w2182 w2199 w2219 w2230 w2248 w2263 w2280 w2285 w2293 w2301 w2306 w2314 w2321 w2329 w2336 w2346 w2374 w2382 w2389 w2397 w2402 w2410 w2417 w2423 w2432 w2448 w2453 w2460 w2478 w2491 w2561 w2573 w2582 w2596 w2605 w2622 w2645 w2662 w2673 w2686 w2711 w2734 w2740 w2756 w2778 w2786 w2792 w2797 w2804 w2814 w2826 w2835 w2840 w2852 w2857 w2867 w2873 w2879 w2884 w2889 w2894 w2904 w2928 w2949 w2954 w2965 w2990 w3017 w3040 w3045 w3060 w3111 w3157 w3202 w3213 w3231 w3251 w3265 w3278 w3286 w3303 w3325 w3349 w3368 w3386 w3404 w3422 w3436 w3450 w3469 w3483 w3498 w3513 w3522 w3527 w3544 w3554 w3561 w3580 w3588 w3593 w3598]
      tunnel: w98 -> [_ _ _ _ _ _ _ _ _ _ _ _ _ _ _ _ _ _ _ _ _ _ _ _ _ _ _ _ _ _ _ _ _ _ _ _ _ _ _ _ _ _ _ _ _ _ _ _ _ _ _ _ _ _ _ _ _ _ _ _ _ _ _ _ w1833 _ _ _ _ _ _ _ _ _ _ _ _ _ _ _ _ _ _ _ _ _ _ _ _ _ _ _ _ _ _ _ _ _ _ _ _ _ _ _ _ w2337 _ _ _ _ _ _ _ _ _ _ _ w2455 _ w2485 _ _ _ _ w2602 w2619 _ _ _ _ _ w2730 _ _ _ _ _ _ w2799 _ _ _ _ _ _ w2863 _ _ _ _ _ _ _ _ _ _ _ _ _ _ _ _ _ _ _ _ _ _ _ _ _ _ _ _ _ _ _ _ _ _ _ _ _ _ _ _ _ _ _ _ _ _]
      tunnel: w94 -> [w107 w526 w534 w541 w546 w556 w581 w596 _ w644 w671 w697 w708 w780 w789 w826 w848 w879 w904 w933 w963 w980 w985 w1034 w1102 w1137 w1157 w1164 w1171 w1194 w1206 w1230 w1234 w1238 w1259 w1289 w1317 w1359 w1365 w1375 w1387 w1417 w1425 w1430 w1438 w1462 w1487 w1511 w1531 w1544 w1588 w1617 w1621 w1648 w1668 w1673 w1677 w1706 w1733 w1748 w1776 w1804 w1809 w1816 w1831 w1849 w1874 w1885 w1903 w1920 w1945 w1964 w1977 w1985 w2004 w2016 w2028 w2047 w2063 w2076 w2089 w2101 w2105 w2110 w2117 w2129 w2138 w2144 w2151 w2161 w2169 w2186 w2214 w2220 w2245 w2256 w2278 w2282 w2286 w2294 w2303 w2312 w2318 w2326 w2333 w2343 w2371 w2379 w2386 w2394 w2399 w2404 w2415 w2420 w2426 w2445 w2450 w2458 w2469 w2487 w2558 w2563 w2576 w2594 w2603 w2620 w2635 w2659 w2670 w2680 w2704 w2731 w2737 w2749 w2774 w2783 w2789 w2794 w2801 w2808 w2822 w2832 w2837 w2849 w2854 w2860 w2870 w2876 w2881 w2886 w2891 w2901 w2926 w2947 w2951 w2963 w2988 w3015 w3038 w3042 w3053 w3105 w3153 w3199 w3209 w3226 w3246 w3260 w3274 w3280 w3298 w3320 w3344 w3363 w3381 w3399 w3417 w3431 w3445 w3464 w3478 w3493 w3510 w3520 w3524 w3529 w3552 w3558 w3564 w3586 w3590 w3595]
      tunnel: [w100 w527 w536 w542 w549 w557 w582 w597 w640 w646 w667 w685 w704 w757 w785 w827 w836 w868 w898 w924 w956 w967 w986 w1010 w1099 w1136 w1158 w1165 w1175 w1198 errorcluster {"status"=FALSE, "code"=0, "source"=""} ("error out") w1229 w1235 w1248 w1267 w1281 w1304 w1361 w1366 w1370 w1382 w1392 w1421 w1431 w1439 w1463 w1488 w1512 w1532 w1535 w1580 w1611 w1625 w1649 w1659 w1674 w1680 w1704 w1732 w1747 w1763 w1798 w1810 w1821 w1825 w1840 w1869 w1881 w1899 w1919 w1936 w1965 w1969 w1987 w2002 w2014 w2026 w2049 w2064 w2077 w2081 w2098 w2106 w2114 w2122 w2126 w2135 w2145 w2148 w2157 w2172 w2194 w2213 w2224 w2238 w2260 w2276 w2283 w2291 w2299 w2304 w2311 w2319 w2327 w2334 w2344 w2372 w2380 w2387 w2395 w2400 w2408 w2414 w2421 w2429 w2446 w2451 w2456 w2477 w2488 w2559 w2567 w2579 w2586 w2599 w2616 w2636 w2660 w2669 w2682 w2706 w2732 w2738 w2746 w2768 w2784 w2790 w2795 w2802 w2812 w2824 w2833 w2838 w2850 w2855 w2865 w2871 w2877 w2882 w2887 w2892 w2902 w2916 w2940 w2952 w2956 w2975 w3007 w3032 w3043 w3047 w3106 w3154 w3200 w3208 w3228 w3248 w3262 w3276 w3282 w3300 w3322 w3346 w3365 w3383 w3401 w3419 w3433 w3447 w3466 w3480 w3494 w3511 w3518 w3525 w3533 w3547 w3559 w3563 w3582 w3591 w3596] -> w79
      tunnel: w80 -> [w106 w527 w536 w542 w549 w557 w582 w597 w640 w646 w668 w692 w702 w757 w784 w827 w837 w875 w889 w914 w957 w975 w986 w1010 w1100 w1139 w1159 w1165 w1174 w1198 w1202 w1229 w1235 w1248 w1267 w1280 w1316 w1361 w1366 w1371 w1383 w1397 w1420 w1431 w1443 w1467 w1492 w1516 w1532 w1542 w1583 w1610 w1624 w1649 w1661 w1674 w1679 w1705 w1723 w1753 w1774 w1797 w1810 w1818 w1828 w1839 w1868 w1884 w1898 w1918 w1935 w1965 w1975 w1988 w2001 w2013 w2025 w2048 w2065 w2077 w2080 w2093 w2106 w2114 w2122 w2125 w2134 w2145 w2149 w2158 w2177 w2193 w2212 w2223 w2244 w2259 w2275 w2283 w2291 w2299 w2304 w2311 w2319 w2327 w2334 w2344 w2372 w2380 w2387 w2395 w2400 w2408 w2414 w2421 w2429 w2446 w2451 w2457 w2477 w2489 w2559 w2568 w2578 w2585 w2598 w2615 w2637 w2660 w2669 w2677 w2709 w2732 w2738 w2751 w2767 w2784 w2790 w2795 w2802 w2812 w2824 w2833 w2838 w2850 w2855 w2865 w2871 w2877 w2882 w2887 w2892 w2902 w2915 w2939 w2952 w2955 w2974 w2997 w3023 w3043 _ w3107 w3154 w3200 w3207 w3227 w3247 w3261 w3276 w3281 w3299 w3321 w3345 w3364 w3382 w3400 w3418 w3432 w3446 w3465 w3479 w3492 w3511 w3517 w3525 w3538 w3549 w3559 w3562 w3581 w3591 w3596]
      tunnel: [w108 w528 w537 w543 w550 w558 w583 w598 w641 w647 w674 w699 w711 w782 w797 w828 w855 w887 w906 w935 w965 w982 w987 w1072 w1109 w1148 w1161 w1166 w1172 w1200 w1208 w1231 w1236 w1249 w1268 w1296 w1324 w1362 w1367 w1376 w1388 w1418 w1426 w1432 w1456 w1480 w1504 w1528 w1533 w1550 w1597 w1619 w1635 w1650 w1670 w1675 w1687 w1716 w1742 w1754 w1792 w1805 w1811 w1822 w1834 w1865 w1878 w1892 w1907 w1926 w1961 w1966 w1980 w1990 w2006 w2018 w2030 w2058 w2073 w2078 w2090 w2102 w2107 w2115 w2123 w2132 w2141 w2146 w2154 w2163 w2181 w2198 w2218 w2229 w2247 w2262 w2279 w2284 w2292 w2300 w2305 w2313 w2320 w2328 w2335 w2345 w2373 w2381 w2388 w2396 w2401 w2409 w2416 w2422 w2431 w2447 w2452 w2459 w2478 w2490 w2560 w2572 w2581 w2595 w2604 w2621 w2644 w2661 w2672 w2685 w2710 w2733 w2739 w2755 w2777 w2785 w2791 w2796 w2803 w2813 w2825 w2834 w2839 w2851 w2856 w2866 w2872 w2878 w2883 w2888 w2893 w2903 w2927 w2948 w2953 w2964 w2989 w3016 w3039 w3044 w3059 w3110 w3156 w3201 w3212 w3230 w3250 w3264 w3277 w3285 w3302 w3324 w3348 w3367 w3385 w3403 w3421 w3435 w3449 w3468 w3482 w3497 w3512 w3521 w3526 w3543 w3553 w3560 w3579 w3587 w3592 w3597] -> w96
      tunnel: [_ _ _ _ _ _ _ _ _ _ _ _ _ _ _ _ _ _ _ _ _ _ _ _ _ _ _ _ _ _ _ TRUE _ _ _ _ _ _ _ _ _ _ _ _ _ _ _ _ _ _ _ _ _ _ _ _ _ _ _ _ _ _ _ _ _ _ _ _ _ _ _ _ _ _ _ _ _ _ _ _ _ _ _ _ _ _ _ _ _ _ _ _ _ _ _ _ _ _ _ _ _ _ _ _ _ _ _ _ _ _ _ _ _ _ _ _ _ _ _ _ _ _ _ _ _ _ _ _ _ _ _ _ _ _ _ _ _ _ _ _ _ _ _ _ _ _ _ _ _ _ _ _ _ _ _ _ _ _ _ _ _ _ _ _ _ _ _ _ _ _ _ _ _ _ _ _ _ _ _ _ _ _ _ _ _ _ _ _ _ _ _ _] -> w87
      tunnel: [w105 w526 w534 w541 w546 w556 w581 w596 w615 w644 w671 w697 w708 w780 w789 w826 w848 w879 w904 w933 w963 w980 w985 w1034 w1103 w1138 w1157 w1164 w1171 w1199 w1206 w1230 w1234 w1239 w1260 w1290 w1318 w1360 w1365 w1375 w1387 w1417 w1425 w1430 w1438 w1462 w1487 w1511 w1531 w1544 w1589 w1617 w1622 w1648 w1669 w1673 w1678 w1706 w1733 w1752 w1776 w1804 w1809 w1819 w1831 w1849 w1874 w1885 w1903 w1920 w1945 w1964 w1978 w1985 w2004 w2016 w2028 w2047 w2063 w2076 w2089 w2101 w2105 w2111 w2118 w2130 w2139 w2144 w2152 w2162 w2170 w2192 w2201 w2225 w2246 w2257 w2278 w2282 w2287 w2295 w2303 w2312 w2318 w2326 w2333 w2343 w2371 w2379 w2386 w2394 w2399 w2404 w2415 w2420 w2426 w2445 w2450 w2458 w2468 w2487 w2558 w2564 w2577 w2594 w2603 w2620 w2635 w2659 w2670 w2681 w2705 w2731 w2737 w2750 w2774 w2783 w2789 w2794 w2801 w2809 w2822 w2832 w2837 w2849 w2854 w2860 w2870 w2876 w2881 w2886 w2891 w2901 w2926 w2947 w2951 w2963 w2988 w3015 w3038 w3042 w3058 w3104 w3153 w3199 w3209 w3226 w3246 w3260 w3274 w3280 w3298 w3320 w3344 w3363 w3381 w3399 w3417 w3431 w3445 w3464 w3478 w3495 w3510 w3520 w3524 w3529 w3552 w3558 w3564 w3586 w3590 w3595] -> w95
      tunnel: 40 ("Timeout") -> [w104 _ _ _ _ _ _ _ _ _ _ _ _ _ _ _ _ _ _ _ _ _ _ _ _ _ _ _ _ _ _ _ _ _ _ _ _ _ _ _ _ _ _ _ _ _ _ _ _ _ _ _ _ _ _ _ _ _ _ _ _ _ _ _ _ _ _ _ _ _ _ _ _ _ _ _ _ _ _ _ _ _ _ _ _ _ _ _ _ _ _ _ _ _ _ _ _ _ _ _ _ _ _ _ _ _ _ _ _ _ _ _ _ _ _ _ _ _ _ _ _ _ _ _ _ _ _ _ _ _ _ _ _ _ _ _ _ _ _ _ _ _ _ _ _ _ _ _ _ _ _ _ _ _ _ _ _ _ _ _ _ _ _ _ _ _ _ _ _ _ _ _ _ _ _ _ _ _ _ _ _ _ _ _ _ _ _ _ _ _ _ _]
      tunnel: w92 -> [_ _ _ _ _ _ _ _ _ _ _ _ _ _ _ _ _ _ _ _ _ _ _ _ w1107 _ _ _ _ _ _ _ _ _ _ _ _ _ _ _ _ _ _ _ _ _ _ _ _ _ _ _ _ _ _ _ _ _ _ _ _ _ _ _ _ _ _ _ _ _ _ _ _ _ _ _ _ _ _ _ w2086 w2097 _ _ _ _ _ _ _ _ _ _ _ _ _ _ _ _ _ _ _ _ _ _ _ _ _ _ _ _ _ _ _ _ _ _ _ _ _ _ _ _ _ _ _ _ _ _ _ _ _ _ _ _ _ _ _ _ _ _ _ _ _ _ _ _ _ _ _ _ _ _ _ _ _ _ _ _ _ _ _ _ _ _ _ _ _ _ _ _ _ _ _ _ _ _ _ _ _ _ _ _ _ _ _ _ _ _ _ _ _ _]
      tunnel: w91 -> [_ _ _ _ _ _ _ _ _ _ _ _ _ _ _ _ _ _ _ _ _ _ _ _ w1106 _ _ _ _ _ _ _ _ _ _ _ _ _ _ _ _ _ _ _ _ _ _ _ _ _ _ _ _ _ _ _ _ _ _ _ _ _ _ _ _ _ _ _ _ _ _ _ _ _ _ _ _ _ _ _ w2087 w2096 _ _ _ _ _ _ _ _ _ _ _ _ _ _ _ _ _ _ _ _ _ _ _ _ _ _ _ _ _ _ _ _ _ _ _ _ _ _ _ _ _ _ _ _ _ _ _ _ _ _ _ _ _ _ _ _ _ _ _ _ _ _ _ _ _ _ _ _ _ _ _ _ _ _ _ _ _ _ _ _ _ _ _ _ _ _ _ _ _ _ _ _ _ _ _ _ _ _ _ _ _ _ _ _ _ _ _ _ _ _]
      tunnel: w90 -> [w103 _ _ _ _ _ _ _ _ _ _ _ _ _ _ _ _ _ _ _ _ _ _ _ _ _ _ _ _ _ _ _ _ _ _ _ _ _ _ _ _ _ _ _ _ _ _ _ _ _ _ w1613 _ _ _ _ _ _ _ _ _ _ _ _ _ _ _ _ _ _ _ _ _ _ _ _ _ _ _ _ _ _ _ _ _ _ _ _ _ _ _ _ _ _ _ _ _ _ _ _ _ _ _ _ _ _ _ _ _ _ _ _ _ _ _ _ _ _ _ _ _ _ _ _ _ _ _ _ _ _ _ _ _ _ _ _ _ _ _ _ _ _ _ _ _ _ _ _ _ _ _ _ _ _ _ _ _ _ _ _ _ _ _ _ _ _ _ _ _ _ _ _ _ _ _ _ _ _ _ _ _ _ _ _ _ _ _ _ _ _ _ _]
      tunnel: w89 -> [w102 w525 w535 w540 w548 w555 w573 w595 w625 w645 w673 w698 w710 w781 w796 w825 w854 w886 w905 w934 w964 w981 w984 w1071 w1108 w1147 w1156 w1163 w1168 w1186 w1205 w1228 w1233 w1247 w1266 w1295 w1315 w1358 w1364 w1374 w1386 w1416 w1424 w1429 w1437 w1461 w1486 w1510 w1530 w1539 w1563 w1618 w1634 w1647 w1656 w1672 w1686 w1715 w1741 w1746 w1791 w1796 w1808 w1815 w1824 w1836 w1867 w1883 w1897 w1917 w1932 w1963 w1979 w1989 w2005 w2017 w2029 w2057 w2060 w2075 w2088 w2095 w2104 w2113 w2121 w2128 w2137 w2143 w2153 w2156 w2168 w2187 w2202 w2221 w2243 w2261 w2277 w2281 w2289 w2297 w2302 w2310 w2317 w2325 w2332 w2342 w2370 w2378 w2385 w2390 w2398 w2407 w2413 w2419 w2428 w2440 w2449 w2454 w2476 w2484 w2557 w2562 w2574 w2584 w2597 w2614 w2643 w2658 w2671 w2683 w2707 w2727 w2735 w2748 w2776 w2781 w2787 w2793 w2800 w2811 w2823 w2831 w2836 w2848 w2853 w2864 w2869 w2875 w2880 w2885 w2890 w2900 w2925 w2946 w2950 w2962 w2987 w3014 w3037 w3041 w3057 w3109 w3155 w3196 w3211 w3229 w3249 w3263 w3275 w3284 w3301 w3323 w3347 w3366 w3384 w3402 w3420 w3434 w3448 w3467 w3481 w3496 w3509 w3519 w3523 w3542 w3551 w3557 w3578 w3585 w3589 w3594]
      tunnel: [w101 w525 w535 w540 w548 w555 w573 w595 w625 w645 w673 w698 w710 w781 w796 w825 w854 w886 w905 w934 w964 w981 w984 w1071 w1108 w1147 w1156 w1163 w1168 w1186 w1205 w1228 w1233 w1247 w1266 w1295 w1315 w1358 w1364 w1374 w1386 w1416 w1424 w1429 w1437 w1461 w1486 w1510 w1530 w1539 w1563 w1618 w1634 w1647 w1656 w1672 w1686 w1715 w1741 w1746 w1791 w1796 w1808 w1815 w1824 w1836 w1867 w1883 w1897 w1917 w1932 w1963 w1979 w1989 w2005 w2017 w2029 w2057 w2060 w2075 w2088 w2095 w2104 w2113 w2121 w2128 w2137 w2143 w2153 w2156 w2168 w2187 w2202 w2221 w2243 w2261 w2277 w2281 w2289 w2297 w2302 w2310 w2317 w2325 w2332 w2342 w2370 w2378 w2385 w2390 w2398 w2407 w2413 w2419 w2428 w2440 w2449 w2454 w2476 w2484 w2557 w2562 w2574 w2584 w2597 w2614 w2643 w2658 w2671 w2683 w2707 w2727 w2735 w2748 w2776 w2781 w2787 w2793 w2800 w2811 w2823 w2831 w2836 w2848 w2853 w2864 w2869 w2875 w2880 w2885 w2890 w2900 w2925 w2946 w2950 w2962 w2987 w3014 w3037 w3041 w3057 w3109 w3155 w3196 w3211 w3229 w3249 w3263 w3275 w3284 w3301 w3323 w3347 w3366 w3384 w3402 w3420 w3434 w3448 w3467 w3481 w3496 w3509 w3519 w3523 w3542 w3551 w3557 w3578 w3585 w3589 w3594] -> w88
      tunnel: w84 -> [_ _ _ _ _ _ _ _ _ _ _ _ _ _ _ _ _ _ _ _ _ _ _ _ w1101 _ _ _ _ _ _ _ _ _ _ _ _ _ _ _ _ _ _ _ _ _ _ _ _ _ _ _ _ _ _ _ _ _ _ _ _ _ _ _ _ _ _ _ _ _ _ _ _ _ _ _ _ _ _ _ w2085 w2094 _ _ _ _ _ _ _ _ _ _ _ _ _ _ _ _ _ _ _ _ _ _ _ _ _ _ _ _ _ _ _ _ _ _ _ _ _ _ _ _ _ _ _ _ _ _ _ _ _ _ _ _ _ _ _ _ _ _ _ _ _ _ _ _ _ _ _ _ _ _ _ _ _ _ _ _ _ _ _ _ _ _ _ _ _ _ _ _ _ _ _ _ _ _ _ _ _ _ _ _ _ _ _ _ _ _ _ _ _ _]
      frame "", "Event Structure", "Idle" {
        # "executes when the state queue is empty"
        n32 = event shown="[37] <AcqLoop error?>: User Event" {
          selector: w102 -> [_ _ _ _ _ _ _ _ _ _ _ _ _ _ _ _ _ _ _ _ _ _ _ _ _ _ _ _ _ _ _ _ _ _ _ _ _ _ _]
          dyn-events: [_ _ _ _ _ _ _ _ _ _ _ _ _ _ _ _ _ _ _ _ _ _ _ _ _ _ _ _ _ _ _ _ _ _ _ _ _ _ _] -> w101
          timeout: w104 -> [_ _ _ _ _ _ _ _ _ _ _ _ _ _ _ _ _ _ _ _ _ _ _ _ _ _ _ _ _ _ _ _ _ _ _ _ _ _ _]
          tunnel: w109 -> [w129 w148 w156 w160 w164 w172 w178 w186 w194 w204 w211 w240 w260 w280 w300 w304 w311 w334 w348 w362 w376 w381 w384 w390 w397 w404 w410 w416 w422 w429 w442 w453 w465 w472 w476 w480 w487 w502 w524]
          tunnel: [w130 w148 w155 w160 w163 w172 w178 w186 w194 w204 w210 w240 w260 w280 w300 w304 w310 w334 w348 w362 w376 w380 w383 w390 w398 w405 w409 w415 w422 w430 w443 w453 w466 w472 w476 w479 w486 w503 w523] -> w108
          tunnel: w107 -> [w113 w146 w150 w158 w165 w171 w179 w187 w195 w202 w206 w238 w258 w278 w298 w302 w306 w333 w347 w361 w375 w377 w385 w388 w393 w400 w412 w417 w420 w424 w437 w451 w461 w470 w474 w481 w488 w491 w521]
          tunnel: [w128 w147 w151 w159 w166 w170 w177 w185 w193 w203 w212 w239 w259 w279 w299 w303 w312 w331 w335 w358 w373 w379 w386 w389 w394 w401 w413 w418 w421 w428 w441 w452 w462 w471 w475 w482 w489 w504 w522] -> w100
          tunnel: w106 -> [w128 w147 w151 w159 w166 w170 w177 w185 w193 w203 w212 w239 w259 w279 w299 w303 w312 w328 w337 w349 w365 w379 w386 w389 w394 w401 w413 w418 w421 w428 w441 w452 w464 w471 w475 w482 w489 w504 w522]
          tunnel: [w113 w146 w150 w158 w165 w171 w179 w187 w195 w202 w207 w238 w258 w278 w298 w302 w307 w333 w347 w361 w375 w377 w385 w388 w395 w402 w412 w417 w420 w425 w438 w451 w467 w470 w474 w481 w488 w501 w521] -> w105
          tunnel: w103 -> [_ _ _ _ _ _ _ _ _ _ _ _ _ _ _ _ _ _ _ _ _ _ _ _ _ _ _ _ _ _ _ _ _ _ _ _ _ _ _]
          event Timeout {
            # "check system status every 2s"
            n33 = event-data() -> ()  [unwired: 1 in, 1 out]
            n34 = Unbundle By Name(w113) -> ("SysRunning?"=w111:bool, "SlowTimer"=w127:u32, "FastTimer"=w121:u32)
            n35 = Tick Count (ms)() -> (millisecond timer value=w114:u32)
            n36 = Subtract(x=w114, y=w127) -> (x-y=w124:u32)
            n37 = case shown="False" w111 {
              tunnel: ["" "Utility: AquiTimerCheck" ("State(s) in Front (\"\")")] -> w119
              frame False {
                # "if not running, do nothing"
              }
              frame True {
                # "if aquisition is running, check timer"
              }
            }
            n38 = Subtract(x=w114, y=w121) -> (x-y=w122:u32)
            n39 = Greater?(x=w124, y=u32 2000) -> (0:w125:bool)
            n40 = Greater?(x=w122, y=u32 500) -> (0:w112:bool)
            n41 = disable-structure shown="Enabled" {
              disable-tunnel: w112 -> [w135 _]
              disable-tunnel: w111 -> [w134 _]
              disable-tunnel: [w131 "" ("State(s) at Back (\"\")")] -> w110
              frame Disabled {
                n42 = Not(x=w134) -> (.not. x?=w133:bool)
                n43 = And(x=w135, y=w133) -> (x .and. y?=w132:bool)
                n44 = case shown="True" w132 {
                  tunnel: ["" ("Empty String Constant") "TCP: checkSource" ("State(s) in Front (\"\")")] -> w131
                  frame False {
                  }
                  frame True {
                  }
                }
              }
              frame Enabled {
              }
            }
            n45 = case shown="True" w125 {
              tunnel: ["" ("Empty String Constant") "SystemStatus: SlowSysStatusMacro" ("State(s) in Front (\"\")")] -> w117
              frame False {
              }
              frame True {
              }
            }
            n46 = case shown="True" w112 {
              tunnel: ["" ("Empty String Constant") "SystemStatus: FastSysStatusMacro" ("State(s) in Front (\"\")")] -> w115
              frame False {
              }
              frame True {
              }
            }
            n47 = call <vilib>:"Add State(s) to Queue__JKI_lib_State_Machine.vi"("State(s) in Front (\"\")"=w119, "State(s) in (\"\")"="LabJack: checkPedal" ("State(s) in Front (\"\")"), "State(s) at Back (\"\")"=w117) -> ("States Out"=w116:string)  [unwired: 12 in]
            n48 = call <vilib>:"Add State(s) to Queue__JKI_lib_State_Machine.vi"("State(s) in Front (\"\")"=w116, "State(s) in (\"\")"=w115, "State(s) at Back (\"\")"=w110) -> ("States Out"=w120:string)  [unwired: 12 in]
            n49 = call <vilib>:"Add State(s) to Queue__JKI_lib_State_Machine.vi"("State(s) in Front (\"\")"=w120, "State(s) in (\"\")"=w129) -> ("States Out"=w130:string)  [unwired: 13 in]
          }
          event "355nm Laser toggle": Mouse Enter {
            n50 = event-data() -> ()  [unwired: 1 in, 4 out]
            n51 = local write "Help"("Toggle 355nm laser." ("Help")) -> ()
          }
          event "355nm Laser toggle": Value Change {
            # "[Covers: REQ34]"
            n52 = event-data() -> ()  [unwired: 1 in, 6 out]
            n53 = Select(t="LabJack: 355_PWM_Start\nLabJack: AB_Start", s="355nm Laser toggle", f="LabJack: 355_PWM_Stop\nLabJack: AB_Stop") -> (s? t:f=w153:string)
            n54 = call <vilib>:"Add State(s) to Queue__JKI_lib_State_Machine.vi"("State(s) in Front (\"\")"=w153, "State(s) in (\"\")"=w156) -> ("States Out"=w155:string)  [unwired: 13 in]
          }
          event "Aiming beam toggle": Mouse Enter {
            n55 = event-data() -> ()  [unwired: 1 in, 4 out]
            n56 = local write "Help"("Toggle aiming beam laser." ("Help")) -> ()
          }
          event "Aiming beam toggle": Value Change {
            # "[Covers: REQ33]"
            n57 = event-data() -> ()  [unwired: 1 in, 6 out]
            n58 = case shown="True" "Aiming beam toggle" {
              tunnel: ["LabJack: AB_Stop" ("State(s) in Front (\"\")") "LabJack: AB_Start" ("State(s) in Front (\"\")")] -> w162
              frame False {
              }
              frame True {
              }
            }
            n59 = call <vilib>:"Add State(s) to Queue__JKI_lib_State_Machine.vi"("State(s) in Front (\"\")"=w162, "State(s) in (\"\")"=w164) -> ("States Out"=w163:string)  [unwired: 13 in]
          }
          event "Auto gain ch1": Value Change {
            n60 = event-data() -> ("NewVal"=w169:bool)  [unwired: 1 in, 5 out]
            n61 = case shown="True" w169 {
              frame False {
                n62 = local read "V 1"() -> (w173:dbl)
                n63 = call "V1FGV.vi"("action (write)"=enum16{"write", "read"}."write" ("action"), "V1 in"=w173) -> ()  [unwired: 8 in, 2 out]
                n64 = property on="V 1" class="DigNum (strict)"("DisabledEnum"=T13."Enabled" ("Disabled")) -> ()  [unwired: 2 in, 2 out]
              }
              frame True {
                n65 = property on="V 1" class="DigNum (strict)"("DisabledEnum"=T13."Disabled and Grayed Out" ("Disabled")) -> ()  [unwired: 2 in, 2 out]
              }
            }
          }
          event "Auto gain ch2": Value Change {
            n66 = event-data() -> ("NewVal"=w180:bool)  [unwired: 1 in, 5 out]
            n67 = case shown="False" w180 {
              frame False {
                n68 = local read "V 2"() -> (w181:dbl)
                n69 = property on="V 2" class="DigNum (strict)"("DisabledEnum"=T13."Enabled" ("Disabled")) -> ()  [unwired: 2 in, 2 out]
                n70 = call "V2FGV.vi"("action(write)"=enum16{"write", "read"}."write" ("action"), "V2 in"=w181) -> ()  [unwired: 8 in, 2 out]
              }
              frame True {
                n71 = property on="V 2" class="DigNum (strict)"("DisabledEnum"=T13."Disabled and Grayed Out" ("Disabled")) -> ()  [unwired: 2 in, 2 out]
              }
            }
          }
          event "Auto gain ch3": Value Change {
            n72 = event-data() -> ("NewVal"=w188:bool)  [unwired: 1 in, 5 out]
            n73 = case shown="False" w188 {
              frame False {
                n74 = local read "V 3"() -> (w189:dbl)
                n75 = property on="V 3" class="DigNum (strict)"("DisabledEnum"=T13."Enabled" ("Disabled")) -> ()  [unwired: 2 in, 2 out]
                n76 = call "V3FGV.vi"("action(write)"=enum16{"write", "read"}."write" ("action"), "V3 in"=w189) -> ()  [unwired: 8 in, 2 out]
              }
              frame True {
                n77 = property on="V 3" class="DigNum (strict)"("DisabledEnum"=T13."Disabled and Grayed Out" ("Disabled")) -> ()  [unwired: 2 in, 2 out]
              }
            }
          }
          event "Auto gain ch4": Value Change {
            n78 = event-data() -> ("NewVal"=w196:bool)  [unwired: 1 in, 5 out]
            n79 = case shown="False" w196 {
              frame False {
                n80 = local read "V 4"() -> (w197:dbl)
                n81 = property on="V 4" class="DigNum (strict)"("DisabledEnum"=T13."Enabled" ("Disabled")) -> ()  [unwired: 2 in, 2 out]
                n82 = call "V4FGV.vi"("action(write)"=enum16{"write", "read"}."write" ("action"), "V3 in"=w197) -> ()  [unwired: 8 in, 2 out]
              }
              frame True {
                n83 = property on="V 4" class="DigNum (strict)"("DisabledEnum"=T13."Disabled and Grayed Out" ("Disabled")) -> ()  [unwired: 2 in, 2 out]
              }
            }
          }
          event "Background": Mouse Enter {
            n84 = event-data() -> ()  [unwired: 1 in, 4 out]
            n85 = local write "Help"("Click to record a background." ("Help")) -> ()
          }
          event "Background": Value Change {
            n86 = event-data() -> ("NewVal"=w208:bool)  [unwired: 1 in, 5 out]
            n87 = case shown="False" w208 {
              tunnel: ["Utility: SetAllChanManualGain\nQueue: Flash\nUtility: Dewelling >> 2500\nLabJack: 355_PWM_Stop\nLabJack: AB_Stop" "Utility: SetDataClass >> Bg\nUI: Update\nLabJack: 355_PWM_Start\nLabJack: AB_Start\nUtility: SaveDeconChan\nUtility: Dewelling >> 50\nLabJack: SetV\nDigitizer: Start\nUtility: AquiTimerReset\nLED: BreathGreen\nUI: duringBGAcquire"] -> w209
              tunnel: [FALSE TRUE] -> w205
              frame False {
                n88 = local read "Skip Data Save?"() -> (w213:bool)
                n89 = case shown="False" w213 {
                  frame False {
                    n90 = property on="Background" class="Bool (strict)"("BoolText.Text"="Done!" ("Boolean Text.Text")) -> ()  [unwired: 2 in, 2 out]
                  }
                  frame True {
                  }
                }
              }
              frame True {
                # "[Covers: REQ6]"
                n91 = property on="Background" class="Bool (strict)"("BoolText.Text"="Running" ("Boolean Text.Text"), "Colors [4]"=cluster{u32, u32}[] [{6618880, 6618880}, {16711680, 16711680}]) -> ()  [unwired: 2 in, 2 out]
              }
            }
            n92 = Bundle By Name(cluster=w206, "SysRunning?"=w205) -> (w207:T24)
            n93 = call <vilib>:"Add State(s) to Queue__JKI_lib_State_Machine.vi"("State(s) in Front (\"\")"=w209, "State(s) in (\"\")"=w211) -> ("States Out"=w210:string)  [unwired: 13 in]
          }
          event "Channel 1": Cursor Move {
            n94 = event-data() -> ("CursIdx"=w224:i32, "CursLoc"=w236:cluster{"X":dbl, "Y":dbl})  [unwired: 1 in, 7 out]
            n95 = property on="Channel 3" class="WFGraph (strict)"() -> ("CrsrList"=w231:T25)  [unwired: 2 in, 2 out]
            n96 = property on="Channel 4" class="WFGraph (strict)"() -> ("CrsrList"=w223:T25)  [unwired: 2 in, 2 out]
            n97 = property on="Channel 2" class="WFGraph (strict)"() -> ("CrsrList"=w234:T25)  [unwired: 2 in, 2 out]
            n98 = Index Array(array=w231, index=w224) -> (element=w235:T26)
            n99 = Index Array(array=w223, index=w224) -> (element=w226:T26)
            n100 = Unbundle By Name(w236) -> ("X"=w225:dbl)
            n101 = Index Array(array=w234, index=w224) -> (element=w237:T26)
            n102 = Bundle By Name(cluster=w235, "Position.X"=w225) -> (w230:T26)
            n103 = Bundle By Name(cluster=w226, "Position.X"=w225) -> (w222:T26)
            n104 = Bundle By Name(cluster=w237, "Position.X"=w225) -> (w233:T26)
            n105 = control-ref of="Channel 1"() -> (w227:refnum<vi>)
            n106 = Replace Array Subset(array=w231, new element=w230, index=w224) -> (w229:T25)
            n107 = Replace Array Subset(array=w223, new element=w222, index=w224) -> (w221:T25)
            n108 = Replace Array Subset(array=w234, new element=w233, index=w224) -> (w232:T25)
            n109 = property on="Channel 3" class="WFGraph (strict)"("CrsrList"=w229) -> (error out=w228:errorcluster)  [unwired: 2 in, 1 out]
            n110 = property on="Channel 4" class="WFGraph (strict)"("CrsrList"=w221) -> ()  [unwired: 2 in, 2 out]
            n111 = property on="Channel 2" class="WFGraph (strict)"("CrsrList"=w232) -> ()  [unwired: 2 in, 2 out]
            n112 = call "UpdateCurserIdx(SubVI).vi"("error in (no error)"=w228, "WaveformGraph in"=w227) -> ()  [unwired: 9 in, 1 out]
          }
          event "Channel 2": Cursor Move {
            n113 = event-data() -> ("CursIdx"=w243:i32, "CursLoc"=w257:cluster{"X":dbl, "Y":dbl})  [unwired: 1 in, 7 out]
            n114 = Unbundle By Name(w257) -> ("X"=w245:dbl)
            n115 = property on="Channel 1" class="WFGraph (strict)"() -> ("CrsrList"=w251:T25)  [unwired: 2 in, 2 out]
            n116 = property on="Channel 3" class="WFGraph (strict)"() -> ("CrsrList"=w253:T25)  [unwired: 2 in, 2 out]
            n117 = property on="Channel 4" class="WFGraph (strict)"() -> ("CrsrList"=w244:T25)  [unwired: 2 in, 2 out]
            n118 = Index Array(array=w251, index=w243) -> (element=w256:T26)
            n119 = Index Array(array=w253, index=w243) -> (element=w255:T26)
            n120 = Index Array(array=w244, index=w243) -> (element=w246:T26)
            n121 = Bundle By Name(cluster=w246, "Position.X"=w245) -> (w242:T26)
            n122 = Bundle By Name(cluster=w256, "Position.X"=w245) -> (w254:T26)
            n123 = Bundle By Name(cluster=w255, "Position.X"=w245) -> (w252:T26)
            n124 = Replace Array Subset(array=w251, new element=w254, index=w243) -> (w250:T25)
            n125 = Replace Array Subset(array=w253, new element=w252, index=w243) -> (w249:T25)
            n126 = Replace Array Subset(array=w244, new element=w242, index=w243) -> (w241:T25)
            n127 = control-ref of="Channel 1"() -> (w248:refnum<vi>)
            n128 = property on="Channel 1" class="WFGraph (strict)"("CrsrList"=w250) -> ()  [unwired: 2 in, 2 out]
            n129 = property on="Channel 3" class="WFGraph (strict)"("CrsrList"=w249) -> (error out=w247:errorcluster)  [unwired: 2 in, 1 out]
            n130 = property on="Channel 4" class="WFGraph (strict)"("CrsrList"=w241) -> ()  [unwired: 2 in, 2 out]
            n131 = call "UpdateCurserIdx(SubVI).vi"("error in (no error)"=w247, "WaveformGraph in"=w248) -> ()  [unwired: 9 in, 1 out]
          }
          event "Channel 3": Cursor Move {
            n132 = event-data() -> ("CursIdx"=w263:i32, "CursLoc"=w277:cluster{"X":dbl, "Y":dbl})  [unwired: 1 in, 7 out]
            n133 = Unbundle By Name(w277) -> ("X"=w265:dbl)
            n134 = property on="Channel 4" class="WFGraph (strict)"() -> ("CrsrList"=w264:T25)  [unwired: 2 in, 2 out]
            n135 = property on="Channel 1" class="WFGraph (strict)"() -> ("CrsrList"=w274:T25)  [unwired: 2 in, 2 out]
            n136 = property on="Channel 2" class="WFGraph (strict)"() -> ("CrsrList"=w272:T25)  [unwired: 2 in, 2 out]
            n137 = Index Array(array=w264, index=w263) -> (element=w266:T26)
            n138 = Index Array(array=w274, index=w263) -> (element=w276:T26)
            n139 = Index Array(array=w272, index=w263) -> (element=w275:T26)
            n140 = Bundle By Name(cluster=w266, "Position.X"=w265) -> (w262:T26)
            n141 = Bundle By Name(cluster=w276, "Position.X"=w265) -> (w273:T26)
            n142 = Bundle By Name(cluster=w275, "Position.X"=w265) -> (w271:T26)
            n143 = Replace Array Subset(array=w264, new element=w262, index=w263) -> (w261:T25)
            n144 = Replace Array Subset(array=w274, new element=w273, index=w263) -> (w270:T25)
            n145 = Replace Array Subset(array=w272, new element=w271, index=w263) -> (w269:T25)
            n146 = control-ref of="Channel 1"() -> (w267:refnum<vi>)
            n147 = property on="Channel 4" class="WFGraph (strict)"("CrsrList"=w261) -> ()  [unwired: 2 in, 2 out]
            n148 = property on="Channel 1" class="WFGraph (strict)"("CrsrList"=w270) -> ()  [unwired: 2 in, 2 out]
            n149 = property on="Channel 2" class="WFGraph (strict)"("CrsrList"=w269) -> (error out=w268:errorcluster)  [unwired: 2 in, 1 out]
            n150 = call "UpdateCurserIdx(SubVI).vi"("error in (no error)"=w268, "WaveformGraph in"=w267) -> ()  [unwired: 9 in, 1 out]
          }
          event "Channel 4": Cursor Move {
            n151 = event-data() -> ("CursIdx"=w285:i32, "CursLoc"=w297:cluster{"X":dbl, "Y":dbl})  [unwired: 1 in, 7 out]
            n152 = Unbundle By Name(w297) -> ("X"=w283:dbl)
            n153 = property on="Channel 1" class="WFGraph (strict)"() -> ("CrsrList"=w295:T25)  [unwired: 2 in, 2 out]
            n154 = property on="Channel 2" class="WFGraph (strict)"() -> ("CrsrList"=w291:T25)  [unwired: 2 in, 2 out]
            n155 = property on="Channel 3" class="WFGraph (strict)"() -> ("CrsrList"=w286:T25)  [unwired: 2 in, 2 out]
            n156 = Index Array(array=w295, index=w285) -> (element=w296:T26)
            n157 = Index Array(array=w291, index=w285) -> (element=w292:T26)
            n158 = Index Array(array=w286, index=w285) -> (element=w288:T26)
            n159 = Bundle By Name(cluster=w296, "Position.X"=w283) -> (w294:T26)
            n160 = Bundle By Name(cluster=w292, "Position.X"=w283) -> (w290:T26)
            n161 = Bundle By Name(cluster=w288, "Position.X"=w283) -> (w287:T26)
            n162 = Replace Array Subset(array=w295, new element=w294, index=w285) -> (w293:T25)
            n163 = Replace Array Subset(array=w291, new element=w290, index=w285) -> (w289:T25)
            n164 = Replace Array Subset(array=w286, new element=w287, index=w285) -> (w284:T25)
            n165 = control-ref of="Channel 1"() -> (w281:refnum<vi>)
            n166 = call "UpdateCurserIdx(SubVI).vi"() -> ()  [unwired: 11 in, 1 out]
            n167 = call "UpdateCurserIdx(SubVI).vi"() -> ()  [unwired: 11 in, 1 out]
            n168 = property on="Channel 1" class="WFGraph (strict)"("CrsrList"=w293) -> ()  [unwired: 2 in, 2 out]
            n169 = property on="Channel 2" class="WFGraph (strict)"("CrsrList"=w289) -> ()  [unwired: 2 in, 2 out]
            n170 = property on="Channel 3" class="WFGraph (strict)"("CrsrList"=w284) -> (error out=w282:errorcluster)  [unwired: 2 in, 1 out]
            n171 = call "UpdateCurserIdx(SubVI).vi"("error in (no error)"=w282, "WaveformGraph in"=w281) -> ()  [unwired: 9 in, 1 out]
          }
          event "Cali&iRF alignment": Mouse Enter {
            n172 = event-data() -> ()  [unwired: 1 in, 4 out]
            n173 = local write "Help"("Click to run system intensity calibration and irf alignment" ("Help")) -> ()
          }
          event "Cali&iRF alignment": Value Change {
            n174 = event-data() -> ("NewVal"=w308:bool)  [unwired: 1 in, 5 out]
            n175 = case shown="False" w308 {
              tunnel: ["Utility: SetAllChanManualGain\nQueue: Flash\nUtility: Dewelling >> 2500\nLabJack: 355_PWM_Stop\nLabJack: AB_Stop" "Utility: SetDataClass >> Cali\nUI: Update\nUtility: SaveDeconChan\nLabJack: 355_PWM_Start\nLabJack: AB_Start\nLabJack: SetV\nDigitizer: Start\nUtility: AquiTimerReset\nLED: BreathGreen\nUI: duringIRFAlign"] -> w309
              tunnel: [FALSE TRUE] -> w305
              frame False {
                n176 = local read "Skip Data Save?"() -> (w313:bool)
                n177 = case shown="False" w313 {
                  frame False {
                    n178 = property on="Cali&iRF alignment" class="Bool (strict)"("BoolText.Text"="Done!" ("Boolean Text.Text")) -> ()  [unwired: 2 in, 2 out]
                  }
                  frame True {
                  }
                }
              }
              frame True {
                n179 = property on="Cali&iRF alignment" class="Bool (strict)"("BoolText.Text"="Running" ("Boolean Text.Text"), "Colors [4]"=cluster{u32, u32}[] [{6618880, 6618880}, {16711680, 16711680}]) -> ()  [unwired: 2 in, 2 out]
              }
            }
            n180 = Bundle By Name(cluster=w306, "SysRunning?"=w305) -> (w307:T24)
            n181 = call <vilib>:"Add State(s) to Queue__JKI_lib_State_Machine.vi"("State(s) in Front (\"\")"=w309, "State(s) in (\"\")"=w311) -> ("States Out"=w310:string)  [unwired: 13 in]
          }
          event "V 1": Value Change {
            n182 = event-data() -> ()  [unwired: 1 in, 6 out]
            n183 = call "LabJack_FGV.vi"("Operation(Read)"=enum16{"Write", "Read"}."Read" ("Operation"), "error in (no error)"=w328) -> ("error out"=w325:errorcluster, "Read data"=w326:i32)  [unwired: 8 in]
            n184 = global read "GlobalVariables.vi" "Ch1 LJ pin"() -> (w324:string)
            n185 = call "LJM_eWriteName.vi"("Handle In"=w326, "Name"=w324, "Value"="V 1", "error in"=w325) -> ("error out"=w322:errorcluster)  [unwired: 10 in, 1 out]
            n186 = call "V1FGV.vi"("Error In"=w322, "action (write)"=enum16{"write", "read"}."write" ("action"), "V1 in"="V 1") -> ("Error Out"=w321:errorcluster)  [unwired: 7 in, 1 out]
            n187 = call "CtrlVtoGain.vi"("error in (no error)"=w321, "CtrlV(V)"="V 1", "Channel"=enum16{"Ch1", "Ch2", "Ch3"}."Ch1" ("Enum")) -> ("error out"=w331:errorcluster, "Gain"=w330:dbl)  [unwired: 7 in]
            n188 = local write "Gain1"(w330) -> ()
          }
          event "V 2": Value Change {
            n189 = event-data() -> ()  [unwired: 1 in, 6 out]
            n190 = call "LabJack_FGV.vi"("Operation(Read)"=enum16{"Write", "Read"}."Read" ("Operation"), "error in (no error)"=w337) -> ("error out"=w342:errorcluster, "Read data"=w343:i32)  [unwired: 8 in]
            n191 = global read "GlobalVariables.vi" "Ch2 LJ pin"() -> (w341:string)
            n192 = call "LJM_eWriteName.vi"("Handle In"=w343, "Name"=w341, "Value"="V 2", "error in"=w342) -> ("error out"=w340:errorcluster)  [unwired: 10 in, 1 out]
            n193 = call "V2FGV.vi"("Error In"=w340, "action(write)"=enum16{"write", "read"}."write" ("action"), "V2 in"="V 2") -> ("Error Out"=w339:errorcluster)  [unwired: 7 in, 1 out]
            n194 = call "CtrlVtoGain.vi"("error in (no error)"=w339, "CtrlV(V)"="V 2", "Channel"=enum16{"Ch1", "Ch2", "Ch3"}."Ch2" ("Enum")) -> ("error out"=w335:errorcluster, "Gain"=w336:dbl)  [unwired: 7 in]
            n195 = local write "Gain2"(w336) -> ()
          }
          event "V 3": Value Change {
            n196 = event-data() -> ()  [unwired: 1 in, 6 out]
            n197 = call "LabJack_FGV.vi"("Operation(Read)"=enum16{"Write", "Read"}."Read" ("Operation"), "error in (no error)"=w349) -> ("error out"=w354:errorcluster, "Read data"=w355:i32)  [unwired: 8 in]
            n198 = global read "GlobalVariables.vi" "Ch3 LJ pin"() -> (w353:string)
            n199 = call "LJM_eWriteName.vi"("Handle In"=w355, "Name"=w353, "Value"="V 3", "error in"=w354) -> ("error out"=w351:errorcluster)  [unwired: 10 in, 1 out]
            n200 = call "V3FGV.vi"("Error In"=w351, "action(write)"=enum16{"write", "read"}."write" ("action"), "V3 in"="V 3") -> ("Error Out"=w350:errorcluster)  [unwired: 7 in, 1 out]
            n201 = call "CtrlVtoGain.vi"("error in (no error)"=w350, "CtrlV(V)"="V 3", "Channel"=enum16{"Ch1", "Ch2", "Ch3"}."Ch3" ("Enum")) -> ("error out"=w358:errorcluster, "Gain"=w357:dbl)  [unwired: 7 in]
            n202 = local write "Gain3"(w357) -> ()
          }
          event "V 4": Value Change {
            n203 = event-data() -> ()  [unwired: 1 in, 6 out]
            n204 = call "LabJack_FGV.vi"("Operation(Read)"=enum16{"Write", "Read"}."Read" ("Operation"), "error in (no error)"=w365) -> ("error out"=w369:errorcluster, "Read data"=w370:i32)  [unwired: 8 in]
            n205 = global read "GlobalVariables.vi" "Ch4 LJ pin"() -> (w368:string)
            n206 = call "LJM_eWriteName.vi"("Handle In"=w370, "Name"=w368, "Value"="V 4", "error in"=w369) -> ("error out"=w367:errorcluster)  [unwired: 10 in, 1 out]
            n207 = call "V4FGV.vi"("Error In"=w367, "action(write)"=enum16{"write", "read"}."write" ("action"), "V3 in"="V 4") -> ("Error Out"=w366:errorcluster)  [unwired: 7 in, 1 out]
            n208 = call "CtrlVtoGain.vi"("error in (no error)"=w366, "CtrlV(V)"="V 4", "Channel"=enum16{"Ch1", "Ch2", "Ch3", "Ch4"}."Ch4") -> ("error out"=w373:errorcluster, "Gain"=w372:dbl)  [unwired: 7 in]
            n209 = local write "Gain4"(w372) -> ()
          }
          event "Quit": Value Change {
            # "Exit Button Value Change (pressed) Event\n(when pressed.  quite)"
            n210 = event-data() -> ()  [unwired: 1 in, 1 out]
            n211 = call <vilib>:"Add State(s) to Queue__JKI_lib_State_Machine.vi"("State(s) in Front (\"\")"="LED: Off\nMacro: Exit", "State(s) in (\"\")"=w381) -> ("States Out"=w380:string)  [unwired: 13 in]
          }
          event "Show BG": Value Change {
            n212 = event-data() -> ()  [unwired: 1 in, 6 out]
            n213 = call <vilib>:"Add State(s) to Queue__JKI_lib_State_Machine.vi"("State(s) in Front (\"\")"="Data: showBG" ("State(s) in Front (\"\")"), "State(s) in (\"\")"=w384) -> ("States Out"=w383:string)  [unwired: 13 in]
          }
          event "StartButton": Mouse Enter {
            n214 = event-data() -> ()  [unwired: 1 in, 4 out]
            n215 = local write "Help"("Press to start aquisition." ("Help")) -> ()
          }
          event "StartButton": Value Change {
            # "[Covers: REQ32]"
            # "start PWM before acquisition"
            # "Initialize both digitizer aquisition and\n send user event to trigger aquisition loop"
            n216 = event-data() -> ()  [unwired: 1 in, 6 out]
            n217 = local write "StartButton"(FALSE ("StartButton")) -> ()
            n218 = Bundle By Name(cluster=w393, "SysRunning?"=TRUE) -> (w395:T24)
            n219 = call <vilib>:"Add State(s) to Queue__JKI_lib_State_Machine.vi"("State(s) in Front (\"\")"="TCP: stopCam\nUtility: SetDataClass >> Data\nQueue: Flash\nUI: Update\nDebugTDMS: Open\nUtility: StartBeep\nLabJack: 355_PWM_Start\nLabJack: AB_Start\nLabJack: SetV\nDigitizer: Start\nUtility: AquiTimerReset\nUI: DuringAquisition\nLED: BreathGreen\nTCP: sendRunNum\nTCP: sendVideoSource\nTCP: sendChannel\nTCP: startRun", "State(s) in (\"\")"=w397) -> ("States Out"=w398:string)  [unwired: 13 in]
          }
          event User Event {
            # "[Covers: REQ32]"
            # "start PWM before acquisition"
            # "Initialize both digitizer aquisition and\n send user event to trigger aquisition loop"
            n220 = event-data() -> ()  [unwired: 1 in, 5 out]
            n221 = Bundle By Name(cluster=w400, "SysRunning?"=TRUE) -> (w402:T24)
            n222 = call <vilib>:"Add State(s) to Queue__JKI_lib_State_Machine.vi"("State(s) in Front (\"\")"="TCP: stopCam\nUtility: SetDataClass >> Data\nQueue: Flash\nUI: Update\nUtility: StartBeep\nLabJack: 355_PWM_Start\nLabJack: AB_Start\nLabJack: SetV\nDigitizer: Start\nUtility: AquiTimerReset\nUI: DuringAquisition\nLED: BreathGreen\nTCP: sendRunNum\nTCP: sendVideoSource\nTCP: sendChannel\nTCP: startRun", "State(s) in (\"\")"=w404) -> ("States Out"=w405:string)  [unwired: 13 in]
          }
          event "Video Display": Value Change {
            n223 = event-data() -> ("NewVal"=w411:bool)  [unwired: 1 in, 5 out]
            n224 = Select(t="TCP: startCam", s=w411, f="TCP: stopCam") -> (s? t:f=w408:string)
            n225 = call <vilib>:"Add State(s) to Queue__JKI_lib_State_Machine.vi"("State(s) in (\"\")"=w410, "State(s) at Back (\"\")"=w408) -> ("States Out"=w409:string)  [unwired: 13 in]
          }
          event "Video Source": Value Change {
            n226 = event-data() -> ()  [unwired: 1 in, 6 out]
            n227 = call <vilib>:"Add State(s) to Queue__JKI_lib_State_Machine.vi"("State(s) in Front (\"\")"="TCP: sendVideoSource" ("State(s) in Front (\"\")"), "State(s) in (\"\")"=w416) -> ("States Out"=w415:string)  [unwired: 13 in]
          }
          event "StopButton": Mouse Enter {
            n228 = event-data() -> ()  [unwired: 1 in, 4 out]
            n229 = local write "Help"("Press to stop data aquisition." ("Help")) -> ()
          }
          event "StopButton": Value Change {
            # "if system is running, send stop command, if not do nothing."
            # "stop aquisition\nupdate UI"
            n230 = event-data() -> ()  [unwired: 1 in, 6 out]
            n231 = Unbundle By Name(w424) -> ("SysRunning?"=w426:bool)
            n232 = case shown="True" w426 {
              tunnel: ["" ("Empty String Constant") "LabJack: AB_Stop\nLabJack: 355_PWM_Stop\n/*Digitizer: Abort"] -> w427
              tunnel: w424 -> [w431 w435]
              tunnel: [w431 w434] -> w425
              frame False {
              }
              frame True {
                n233 = Bundle By Name(cluster=w435, "SysRunning?"=FALSE) -> (w434:T24)
              }
            }
            n234 = call <vilib>:"Add State(s) to Queue__JKI_lib_State_Machine.vi"("State(s) in Front (\"\")"=w427, "State(s) in (\"\")"=w429) -> ("States Out"=w430:string)  [unwired: 13 in]
            n235 = local write "StopButton"(FALSE ("StopButton")) -> ()
          }
          event User Event {
            # "if system is running, send stop command, if not do nothing."
            # "stop aquisition\nupdate UI"
            n236 = event-data() -> ()  [unwired: 1 in, 5 out]
            n237 = Unbundle By Name(w437) -> ("SysRunning?"=w439:bool)
            n238 = case shown="True" w439 {
              tunnel: ["" ("Empty String Constant") "LabJack: AB_Stop\nLabJack: 355_PWM_Stop\n/*Digitizer: Abort"] -> w440
              tunnel: w437 -> [w444 w448]
              tunnel: [w444 w447] -> w438
              frame False {
              }
              frame True {
                n239 = Bundle By Name(cluster=w448, "SysRunning?"=FALSE) -> (w447:T24)
              }
            }
            n240 = call <vilib>:"Add State(s) to Queue__JKI_lib_State_Machine.vi"("State(s) in Front (\"\")"=w440, "State(s) in (\"\")"=w442) -> ("States Out"=w443:string)  [unwired: 13 in]
          }
          event "Sys Reconfig": Mouse Enter {
            n241 = event-data() -> ()  [unwired: 1 in, 4 out]
            n242 = local write "Help"("Click to reconfig digitizer settings." ("Help")) -> ()
          }
          event "Sys Reconfig": Value Change {
            # "everytime the user change data aquisition setting, need to reinitilize decon engine and realign iRF.\ncheck whether data length has changed, if changed, reinitialize Decon engine\nreset BG ready, need a new BG"
            # "update DAQ FGV"
            n243 = event-data() -> ()  [unwired: 1 in, 6 out]
            n244 = call "SystemConfigEditorV6.vi"("error in"=w464) -> ("error out"=w463:errorcluster, "FLImDAQ out"=w458:T5)  [unwired: 1 in]
            n245 = Unbundle By Name(w461) -> ("FLImDAQ.min record length"=w460:i32)
            n246 = Unbundle By Name(w458) -> ("min record length"=w459:i32)
            n247 = call "FLImDAQ_FGV.vi"("error in (no error)"=w463, "Operation (Read)"=enum16{"Write", "Read"}."Write" ("Operation"), "Write data"=w458) -> ("error out"=w462:errorcluster, "Read data"=w457:T5)  [unwired: 7 in]
            n248 = Equal?(x=w460, y=w459) -> (x = y?=w456:bool)
            n249 = case shown="False" w456 {
              tunnel: ["UI: Cursor Set >> Busy\nDigitizer: Config\nDeconEngine: InitializeCh1\nDeconEngine: InitializeCh2\nDeconEngine: InitializeCh3\nUI: CaliAndiRFNotReady\n/*UI iRF not ready\nUI: Update\nUI: Cursor Set >> Idle" "UI: Cursor Set >> Busy\nDigitizer: Config\nUI: Update\nUI: Cursor Set >> Idle"] -> w455
              frame False {
              }
              frame True {
              }
            }
            n250 = Bundle By Name(cluster=w461, "FLImDAQ"=w457) -> (w467:T24)
            n251 = call <vilib>:"Add State(s) to Queue__JKI_lib_State_Machine.vi"("State(s) in Front (\"\")"=w455, "State(s) in (\"\")"=w465) -> ("States Out"=w466:string)  [unwired: 13 in]
          }
          event "System Hardware Connection Status", "StartButton", "StopButton", "355nm Laser toggle", "Aiming beam toggle", "Cali&iRF alignment", "Background", "Sys Reconfig": Mouse Leave {
            n252 = event-data() -> ()  [unwired: 1 in, 4 out]
            n253 = invoke on="Help" class="Str" method="Reinit To Default"() -> ()  [unwired: 3 in, 3 out]
          }
          event "System Hardware Connection Status.Digitizer": Mouse Enter {
            n254 = event-data() -> ()  [unwired: 1 in, 4 out]
            n255 = local write "Help"("Status of hardware connections. TCP/IP is optional." ("Help")) -> ()
          }
          event "TCP Connect": Value Change {
            n256 = event-data() -> ("NewVal"=w477:bool)  [unwired: 1 in, 5 out]
            n257 = case shown="True" w477 {
              tunnel: ["TCP: Close\nUI: Update" ("State(s) in Front (\"\")") "TCP: SendSettingMacro\nUI: Update" ("State(s) in Front (\"\")")] -> w478
              frame False {
              }
              frame True {
              }
            }
            n258 = call <vilib>:"Add State(s) to Queue__JKI_lib_State_Machine.vi"("State(s) in Front (\"\")"=w478, "State(s) in (\"\")"=w480) -> ("States Out"=w479:string)  [unwired: 13 in]
          }
          event "488nm Power": Value Change {
            n259 = event-data() -> ()  [unwired: 1 in, 6 out]
            n260 = call <vilib>:"Add State(s) to Queue__JKI_lib_State_Machine.vi"("State(s) in Front (\"\")"="AimingBeam: Set Current" ("State(s) in Front (\"\")"), "State(s) in (\"\")"=w487) -> ("States Out"=w486:string)  [unwired: 13 in]
          }
          event User Event {
            # "if aquisition loop is error out. Stop digitizer, update front panel indicator, stop both laser and \nOption 1: parse and save data\nOption 2: Flash queue if scout run. [Covers: REQ23]"
            n261 = event-data() -> ()  [unwired: 1 in, 5 out]
            n262 = Unbundle By Name(w491) -> ("OverlaySelection"=w490:u16)
            n263 = case shown="\"Data\", Default" "Data Class" {
              tunnel: [w508 "UI: Cursor Set >> Busy\nUtility: SetAllChanAutoGain\nUtility: RestoreDeConChan\nData: parseRunData\nData: irfAlignment\nUI: Cursor Set >> Idle" w512] -> w499
              tunnel: w490 -> [_ _ w515]
              frame "Data", Default {
                n264 = local read "Video Display"() -> (w510:bool)
                n265 = Select(t="TCP: startCam", s=w510, f="") -> (s? t:f=w506:string)
                n266 = call <vilib>:"Add State(s) to Queue__JKI_lib_State_Machine.vi"("State(s) in Front (\"\")"="DebugTDMS: Close\nUI: Cursor Set >> Busy\nData: parseRunData\nData: saveRunData\nUI: Cursor Set>>Idle" ("State(s) in Front (\"\")"), "State(s) in (\"\")"=w506) -> ("States Out"=w508:string)  [unwired: 13 in]
              }
              frame "Cali" {
              }
              frame "BG" {
                w516 = "UI: Cursor Set >> Busy\nUtility: SetAllChanAutoGain\nUtility: RestoreDeConChan\nData: parseRunData\nData: saveBGtoFGV\nData: saveBGtoFile\nUI: Cursor Set >> Idle\nData: showBG\nRun: BGIncrement"  # UI: Cursor Set >> Busy Utility: SetAllChanAutoGain Utility: RestoreDeConChan Data: parseRunData Data: saveBGtoFGV Data: saveBGtoFile UI: Cursor Set >> Idle Data: showBG Run: BGIncrement
                n267 = Greater Than 0?(x=w515) -> (x > 0?=w514:bool)
                n268 = case shown="True" w514 {
                  tunnel: ["" ("State(s) in (\"\")") "Data: processDeConBG\nData: saveDeConBGtoFile" ("State(s) in (\"\")")] -> w513
                  frame False {
                  }
                  frame True {
                  }
                }
                n269 = call <vilib>:"Add State(s) to Queue__JKI_lib_State_Machine.vi"("State(s) in Front (\"\")"=w516, "State(s) in (\"\")"=w513) -> ("States Out"=w512:string)  [unwired: 13 in]
              }
            }
            n270 = Bundle By Name(cluster=w491, "SysRunning?"=FALSE) -> (w501:T24)
            n271 = Select(t="" ("State(s) in Front (\"\")"), s="Skip Data Save?", f=w499) -> (s? t:f=w496:string)
            n272 = call <vilib>:"Add State(s) to Queue__JKI_lib_State_Machine.vi"("State(s) in Front (\"\")"="TCP: stopRun\nUI: Update\nLabJack: AB_Stop\nLabJack: 355_PWM_Stop\nDigitizer: Abort\nLabJack: ZeroV\nUtility: EndBeep\nLED: BreathOff" ("State(s) in Front (\"\")"), "State(s) in (\"\")"=w496, "State(s) at Back (\"\")"="Macro: SysReadyForAq\nUI: Update" ("State(s) in Front (\"\")")) -> ("States Out"=w494:string)  [unwired: 12 in]
            n273 = call <vilib>:"Add State(s) to Queue__JKI_lib_State_Machine.vi"("State(s) in Front (\"\")"=w494, "State(s) in (\"\")"=w502) -> ("States Out"=w503:string)  [unwired: 13 in]
          }
          event Panel Close? {
            # "Discard the event because we'll close the front panel ourselves in Macro: Exit"
            # "Close Panel button (pressed) Event\n(this executes Macro: Exit to terminate the VI)"
            n274 = event-data() -> ()  [unwired: 1 in, 1 out]
            n275 = event-data ("Event Filter Node")("Discard?"=TRUE) -> ()  [unwired: 1 in, 1 out]
            n276 = call <vilib>:"Add State(s) to Queue__JKI_lib_State_Machine.vi"("State(s) in Front (\"\")"="Macro: Exit", "State(s) in (\"\")"=w524) -> ("States Out"=w523:string)  [unwired: 13 in]
          }
        }
      }
      frame "---------- Macro ----------" {
        # "Do not put any code in this frame.\n(It is a separator no-op. You can make a copy of this frame to create a new Macro frame)"
        n277 = call <vilib>:"Add State(s) to Queue__JKI_lib_State_Machine.vi"("State(s) in (\"\")"=w529) -> ("States Out"=w528:string)  [unwired: 14 in]
      }
      frame "Macro: Initialize" {
        # "load Labjack setting 1st as it contaisn laser pin infortmation"
        # "start laser 1st, need 7.5s for laser to get ready"
        # "Initialization Macro\n(This is called once, when the VI starts)"
        n278 = call <vilib>:"Add State(s) to Queue__JKI_lib_State_Machine.vi"("State(s) in Front (\"\")"="UI: showDisclaimer\nData: Initialize\nInitialize Core Data\nUI: OverlayDialog\nUI: Cursor Set >> Busy\nUI: Initialize\nUI: Front Panel State >> Open\nMacro: LoadSysConfig\nTCP: InitializeNew\nTCP: checkSource\nUI: Update\nLabJack: Open\nLabJack: SetDefaultSub\nLED: OpenVIRef\nLED: BreathOrange\nUI: Update\n355 Laser: CheckControllerStatus\n355 Laser: Laser enable\n355 Laser: Dewelling>>500\n355 Laser: CheckControllerStatus\nUI: Update\nLabJack: 355_PWM_Config\nLabJack: AB_PWM_Config", "State(s) in (\"\")"="Digitizer: Initialize\nDigitizer: Config\nUI: Update\nAimingBeam: Initialize\nAimingBeam: Set APC Status>>Disable\nAimingBeam: Set ACC Status>>Enable\nAimingBeam: Set Current\nUI: Update\n355 Laser: Check Dewelling\nUI: Cursor Set >> Idle\nCase: GetID\nUI: Update\nTCP: SendSettingMacro\nCase: CreatFileStruct\nUI: Update\nData: loadLastUseMacro\nGraph: SetXMultiplier\nGraph: AddCursors\nAPD: Initialize\nAPD: LoadFromSerial\nAPD: UpdateCtrlVLimit\nAPD: GetGainLimits\nPID: loadPID\nMacro: InitDeConAndClassifier\nLED: BreathOff\nMacro: SysReadyForAq") -> ("States Out"=w530:string)  [unwired: 13 in]
        n279 = call <vilib>:"Add State(s) to Queue__JKI_lib_State_Machine.vi"("State(s) in Front (\"\")"=w530, "State(s) in (\"\")"=w538) -> ("States Out"=w537:string)  [unwired: 13 in]
        "Help" <- "Hover over controls to see help!" ("Help")
      }
      frame "Macro: LoadSysConfig" {
        # "System configuration Macro. [Covers: REQ15]\n(Load configurations for different component of the system)"
        n280 = call <vilib>:"Add State(s) to Queue__JKI_lib_State_Machine.vi"("State(s) in Front (\"\")"="SysConfig: Load Sys Config\nSysConfig: Load Digitizer Setting\nSysConfig: Load AB setting\nSysConfig: Load LJ Pinout\nSysConfig: Load 355 PWM\nSysConfig: LoadAPDSerialNumber\nSysConfig: LoadABVideoSetting\nSysConfig: LoadCursorLocation", "State(s) in (\"\")"=w544) -> ("States Out"=w543:string)  [unwired: 13 in]
      }
      frame "Macro: InitDeConAndClassifier" {
        # "Initilized realtime Decon and classifier if needed"
        n281 = Unbundle By Name(w546) -> ("OverlaySelection"=w545:u16)
        n282 = case shown="1, 2" w545 {
          tunnel: ["" ("State(s) in Front (\"\")") "DeconEngine: InitDotNet\nDeconEngine: loadIRF\nDeconEngine: Warmup\nClassifier: Init" ("State(s) in Front (\"\")")] -> w547
          frame 0, Default {
          }
          frame 1, 2 {
          }
        }
        n283 = call <vilib>:"Add State(s) to Queue__JKI_lib_State_Machine.vi"("State(s) in Front (\"\")"=w547, "State(s) in (\"\")"=w551) -> ("States Out"=w550:string)  [unwired: 13 in]
      }
      frame "Macro: SysReadyForAq" {
        # "Macro for system ready\n(It is a separator no-op. You can make a copy of this frame to create a new Macro frame)"
        n284 = call <vilib>:"Add State(s) to Queue__JKI_lib_State_Machine.vi"("State(s) in Front (\"\")"="UI: ReadyForAquisition\nLED: Green" ("State(s) in Front (\"\")"), "State(s) in (\"\")"=w559) -> ("States Out"=w558:string)  [unwired: 13 in]
      }
      frame "Macro: Exit" {
        # "close LJ last"
        # "check whether hardware is initilized, if so close, if not do nothing"
        # "Exit Macro, close all hardware\n(This is called once, when the VI exits)"
        n285 = Unbundle By Name(w581) -> ("System Status.Digitizer"=w577:bool, "System Status.Aiming Beam"=w576:bool, "System Status.355 Laser"=w575:bool, "System Status.Labjack"=w567:bool, "Core.Close Panel on Exit?"=w571:bool)
        n286 = local read ".NetInitialized?"() -> (w560:bool)
        n287 = case shown="True" w560 {
          tunnel: ["" "DeconEngine: CloseNetRef\nClassifier: Close"] -> w562
          frame False {
          }
          frame True {
          }
        }
        n288 = case shown="True" w567 {
          tunnel: ["" ("Empty String Constant") "LabJack: SetDefaultAndClose"] -> w564
          frame False {
          }
          frame True {
          }
        }
        n289 = case shown="True" w576 {
          tunnel: ["" ("Empty String Constant") "AimingBeam: Set ACC Status >> Disable\nAimingBeam: Close"] -> w566
          frame False {
          }
          frame True {
          }
        }
        n290 = case shown="True" w575 {
          tunnel: ["" ("Empty String Constant") "355 Laser: Close\n355 Laser: CheckControllerStatus"] -> w565
          frame False {
          }
          frame True {
          }
        }
        n291 = case shown="True" w577 {
          tunnel: ["" ("Empty String Constant") "Digitizer: Close"] -> w572
          frame False {
          }
          frame True {
          }
        }
        n292 = call <vilib>:"Add State(s) to Queue__JKI_lib_State_Machine.vi"("State(s) in Front (\"\")"="TCP: Close", "State(s) in (\"\")"=w562) -> ("States Out"=w561:string)  [unwired: 13 in]
        n293 = Select(t="UI: Front Panel State >> Close", s=w571, f="" ("Empty String Constant")) -> (s? t:f=w568:string)
        n294 = call <vilib>:"Add State(s) to Queue__JKI_lib_State_Machine.vi"("State(s) in Front (\"\")"=w561, "State(s) in (\"\")"=w572, "State(s) at Back (\"\")"=w566) -> ("States Out"=w574:string)  [unwired: 12 in]
        n295 = call <vilib>:"Add State(s) to Queue__JKI_lib_State_Machine.vi"("State(s) in Front (\"\")"=w574, "State(s) in (\"\")"=w565, "State(s) at Back (\"\")"=w564) -> ("States Out"=w570:string)  [unwired: 12 in]
        n296 = call <vilib>:"Add State(s) to Queue__JKI_lib_State_Machine.vi"("State(s) in Front (\"\")"=w570, "State(s) in (\"\")"="UI: Update\nUI: Reset\nGraph: SaveCursorLoc\nLED: CloseVIRef\nQueue: Destory\nData: Cleanup\nExit", "State(s) at Back (\"\")"=w568) -> ("States Out"=w578:string)  [unwired: 12 in]
        n297 = call <vilib>:"Add State(s) to Queue__JKI_lib_State_Machine.vi"("State(s) in Front (\"\")"=w578, "State(s) in (\"\")"=w584) -> ("States Out"=w583:string)  [unwired: 13 in]
      }
      frame "---------- Data ----------" {
        # "Do not put any code in this frame.\n(It is a separator no-op. You can make a copy of this frame to create a new Data frame)"
        n298 = call <vilib>:"Add State(s) to Queue__JKI_lib_State_Machine.vi"("State(s) in (\"\")"=w599) -> ("States Out"=w598:string)  [unwired: 14 in]
      }
      frame "Data: Initialize" {
        w600 = u16 0  # OverlaySelection
        w601 = path ""  # CaliPath
        w602 = dbl[] []  # V4
        w603 = dbl[][] []  # Ch4Data
        w604 = FALSE  # bothVidSourceAvail
        w605 = T1 {"Main Frame Grabber"=FALSE, "Side Frame Grabber"=FALSE, "Main Camera"=FALSE, "Side Camera"=FALSE}  # video source
        w606 = FALSE  # LED vi ref open?
        w608 = T23 {"DeCon Channel"=enum."1", "Scale Bar"=FALSE, "Scale Low"=3.0, "Scale High"=8.0, "ANSI"=20.0, "Radius"=1.0, "3D?"=FALSE, "Firefly?"=FALSE, "Pentero?"=FALSE}  # VideoConfig
        w609 = T27 {"Ch1APDSerial#"="", "Ch2APDSerial#"="", "Ch3APDSerial#"="", "Ch4APDSerial#"=""}  # APDSerialNum
        w610 = u32 0  # Aquisition Timer
        w611 = cluster{"RunID":i8, "BG ID":i8, "Cali ID":i8} {"RunID"=1, "BG ID"=1, "Cali ID"=1}  # IDs
        w612 = refnum<vi> refnum  # LED vi reference
        w613 = path ""  # TempPath
        w614 = T28 {"DataPath"=path "", "BG Path"=path "", "iRFPath"=path "", "CaliPath"=path ""}  # Pathes
        w616 = dbl[] []  # V3
        w617 = dbl[] []  # V2
        w618 = dbl[] []  # V1
        w620 = u32 0  # FastTimer
        w621 = u32 0  # SlowTimer
        w622 = dbl[][] []  # Ch3Data
        w623 = dbl[][] []  # Ch2Data
        w607 = dbl[][] []  # Ch1Data
        w626 = T2 {"Digitizer"=FALSE, "Labjack"=FALSE, "Aiming Beam"=FALSE, "355 Laser"=FALSE, "TCP/IP"=FALSE}  # System Status
        w627 = T29 {"DIO_EF_CLOCK1_DIVISOR"=16, "DIO_EF_CLOCK1_ROLL_VALUE"=25000, "DIO#_EF_INDEX"=0, "DIO#_EF_OPTIONS"=1, "DIO#_EF_CONFIG_A"=6250}  # AB PWM setting
        w628 = T4 {"Ch1 Bias"="TDA11", "Ch2 Bias"="DAC10", "Ch3 Bias"="DAC0", "Ch4 Bias"="DAC0", "355 PWM"="FIO0", "AimingBeam PWM"="FIO2", "Laser Ready"="FIO3", "Interlock"="FIO1", "Laser Start/Stop"="FIO1", "Red LED"="FIO1", "Green LED"="FIO1", "Foot Pedal"="DIO15"}  # LJ Pinout
        w629 = 0  # TCP attempt count
        w630 = u32 0  # Laser start tic
        w631 = refnum<k20>[] []  # niTClk sessions
        w632 = u32 0  # Last Trigger
        w633 = T29 {"DIO_EF_CLOCK1_DIVISOR"=16, "DIO_EF_CLOCK1_ROLL_VALUE"=25000, "DIO#_EF_INDEX"=0, "DIO#_EF_OPTIONS"=1, "DIO#_EF_CONFIG_A"=6250}  # 355 PWM setting
        w634 = T30 {"Aiming Beam COM Port"="COM3", "Min Current"=0.0, "Max Current"=63.0, "Default Current"=20.0, "Freq"=0}  # AB Cluster
        w635 = T31 {"resource name"="", "resource name 2"="", "Channel"=enum."Channel 0", "trigger source"="VAL_EXTERNAL", "trigger level"=0.5, "trigger delay"=1.35e-07, "min sample rate"=12500000000.0, "min record length"=2500, "vertical range"=1.0, "vertical offset"=-0.25, "Waveform to Avg"=2000}  # FLImDAQ
        w636 = FALSE  # SysRunning?
        w624 = path ""  # DefaultPath
        w637 = ""  # CaseID
        w638 = T7 {"Ch1Enable?"=FALSE, "Ch2Enable?"=FALSE, "Ch3Enable?"=FALSE, "Ch1AutoGain?"=FALSE, "Ch2AutoGain?"=FALSE, "Ch3AutoGain?"=FALSE, "AimingBeamEnable?"=FALSE}  # SysConfigCluster
        w639 = T32 {"Current VI Reference"=refnum, "Close Panel on Exit?"=FALSE}  # Core
        # "Initialize the shift-register data, here.\n(data names are defined by what you wire into the bundle function)"
        n299 = Bundle("Core"=w639, "SysConfigCluster"=w638, "System Status"=w626, "IDs"=w611, "CaseID"=w637, "DefaultPath"=w624, "Pathes"=w614, "FLImDAQ"=w635, "SysRunning?"=w636, "AB Cluster"=w634, "LJ Pinout"=w628, "355 PWM setting"=w633, "AB PWM setting"=w627, "Last Trigger"=w632, "niTClk sessions"=w631, "Laser start tic"=w630, "TCP attempt count"=w629, "Ch1Data"=w607, "Ch2Data"=w623, "Ch3Data"=w622, "Ch4Data"=w603, "V1"=w618, "V2"=w617, "V3"=w616, "V4"=w602, "SlowTimer"=w621, "FastTimer"=w620, "listener ID"=refnum<k5> refnum, "TempPath"=w613, "CaliPath"=w601, "LED vi reference"=w612, "Aquisition Timer"=w610, "APDSerialNum"=w609, "VideoConfig"=w608, "LED vi ref open?"=w606, "video source"=w605, "bothVidSourceAvail"=w604, "OverlaySelection"=w600) -> (w615:T24)  [unwired: 1 in]
        n300 = call <vilib>:"Add State(s) to Queue__JKI_lib_State_Machine.vi"("State(s) in (\"\")"=w642) -> ("States Out"=w641:string)  [unwired: 14 in]
      }
      frame "Data: loadLastUseMacro" {
        # "Load last use BG and Cali and iRF.\n(It is a separator no-op. You can make a copy of this frame to create a new Data frame)"
        n301 = call <vilib>:"Add State(s) to Queue__JKI_lib_State_Machine.vi"("State(s) in Front (\"\")"="Data: loadLastUseBG\nData: LoadRealtimeDeConBG\nData: loadSystemCali\nData: loadLastUseiRF\n/*Data: LoadiRFFromAPDFile\nUI: CaliAndiRFLoaded\nData: ShowiRF" ("State(s) in Front (\"\")"), "State(s) in (\"\")"=w648) -> ("States Out"=w647:string)  [unwired: 13 in]
      }
      frame "Data: loadLastUseBG" {
        w652 = enum16{"write", "read"}."write" ("action")
        # "Load last use BG.\n()"
        n302 = Unbundle By Name(w671) -> ("TempPath"=w670:path)
        n303 = call "FLImDAQ_FGV.vi"() -> ("Read data"=w666:T5)  [unwired: 10 in, 1 out]
        n304 = Build Path(base path=w670, name or relative path="Background.tdms") -> (appended path=w669:path)
        n305 = call "ReadBGorCali (SubVI).vi"("DataType"=enum16{"BG", "Cali"}."BG", "error in (no error)"=w668, "file path in"=w669) -> ("error out"=w667:errorcluster, "AvgDataCluster"=w662:T33)  [unwired: 6 in, 1 out]
        n306 = Unbundle By Name(w662) -> ("Channel 1"=w649:dbl[], "Channel 2"=w661:dbl[], "Channel 3"=w654:dbl[], "Channel 4"=w651:dbl[])
        n307 = Unbundle By Name(w666) -> ("min record length"=w658:i32)
        n308 = Array Size(array=w649) -> (size(s)=w660:i32)
        "BG length" <- w660
        n309 = Equal?(x=w660, y=w658) -> (x = y?=w659:bool)
        n310 = Select(t="UI: BGLoaded" ("State(s) in Front (\"\")"), s=w659, f="UI: BGSizeError" ("State(s) in Front (\"\")")) -> (s? t:f=w663:string)
        n311 = case shown="True" w659 {
          tunnel: w649 -> [_ w682]
          tunnel: w661 -> [_ w681]
          tunnel: w654 -> [_ w680]
          tunnel: w658 -> [w677 _]
          tunnel: [w676 w682] -> w657
          tunnel: [w676 w681] -> w656
          tunnel: [w676 w680] -> w655
          tunnel: w651 -> [_ w679]
          tunnel: [w676 w679] -> w650
          frame False {
            # "If error set BG all 0, update UI"
            n312 = for {
              N: w677 -> [_]
              tunnel: [0.0] -> w676 mode=indexing
            }
          }
          frame True {
            # "If no error, check size match"
          }
        }
        n313 = call "BG4FGV.vi"("action"=w652, "BG4 in"=w650) -> ()  [unwired: 8 in, 2 out]
        n314 = call "BG3FGV.vi"("action"=w652, "BG3 in"=w655) -> ()  [unwired: 8 in, 2 out]
        n315 = call "BG1FGV.vi"("action"=w652, "BG1 in"=w657) -> ()  [unwired: 8 in, 2 out]
        n316 = call "BG2FGV.vi"("action"=w652, "BG2 in"=w656) -> ()  [unwired: 8 in, 2 out]
        n317 = call <vilib>:"Add State(s) to Queue__JKI_lib_State_Machine.vi"("State(s) in Front (\"\")"=w663, "State(s) in (\"\")"=w675) -> ("States Out"=w674:string)  [unwired: 13 in]
      }
      frame "Data: LoadRealtimeDeConBG" {
        # "Load saved realtime DeCon BG from Temp file"
        n318 = Unbundle By Name(w697) -> ("TempPath"=w696:path)
        n319 = Build Path(base path=w696, name or relative path="RealTimeDeConBGTemp.tdms") -> (appended path=w694:path)
        n320 = TDMS Open(8:w692, 10:T16."open" ("operation (0:open)"), 11:w694) -> (0:w689:errorcluster, 3:w691:refnum<k34>)  [unwired: 4 in]
        n321 = TDMS Read(0:w691, 5:"Realtime DeCon BG" ("group name in (Untitled)"), 7:string[] ["Ch1", "Ch2", "Ch3"], 11:w689, 12:dbl[][] [] ("BGAll")) -> (4:w687:refnum<k34>, 10:w683:dbl[][], 15:w686:errorcluster)  [unwired: 3 in, 3 out]
        n322 = local write "BGAll"(w683) -> ()
        n323 = TDMS Close(8:w686, 11:w687) -> (0:w685:errorcluster)  [unwired: 1 out]
        n324 = local write "BG Graph"(w683) -> ()
        n325 = call <vilib>:"Add State(s) to Queue__JKI_lib_State_Machine.vi"("State(s) in (\"\")"=w700) -> ("States Out"=w699:string)  [unwired: 14 in]
      }
      frame "Data: loadSystemCali" {
        # "Load last use calibration.\n()"
        n326 = Unbundle By Name(w708) -> ("CaliPath"=w707:path)
        n327 = Build Path(base path=w707, name or relative path="Calibration.tdms") -> (appended path=w703:path)
        n328 = call "ReadBGorCali (SubVI).vi"("DataType"=enum16{"BG", "Cali"}."Cali", "error in (no error)"=w702, "file path in"=w703) -> ("error out"=w704:errorcluster, "CtrlVCluster"=w706:T34, "AvgDataCluster"=w705:T33)  [unwired: 6 in]
        n329 = case shown="No Error" w704 {
          tunnel: w706 -> [w727 _]
          tunnel: w705 -> [w726 _]
          frame No Error {
            w717 = T35 {"Ch1 WF"=[], "Ch2 WF"=[], "Ch3 WF"=[], "Ch4 WF"=[], "V1"=0.0, "V2"=0.0, "V3"=0.0, "V4"=0.0}  # SysCaliData
            n330 = Unbundle By Name(w726) -> ("Channel 1"=w725:dbl[], "Channel 2"=w724:dbl[], "Channel 3"=w723:dbl[], "Channel 4"=w716:dbl[])
            n331 = Unbundle By Name(w727) -> ("V 1"=w722:dbl[], "V 2"=w721:dbl[], "V 3"=w715:dbl[], "V 4"=w713:dbl[])
            n332 = Index Array(array=w722) -> (element=w720:dbl)  [unwired: 1 in]
            n333 = Index Array(array=w721) -> (element=w719:dbl)  [unwired: 1 in]
            n334 = Index Array(array=w715) -> (element=w718:dbl)  [unwired: 1 in]
            n335 = Index Array(array=w713) -> (element=w714:dbl)  [unwired: 1 in]
            n336 = Bundle By Name(cluster=w717, "Ch1 WF"=w725, "Ch2 WF"=w724, "Ch3 WF"=w723, "Ch4 WF"=w716, "V1"=w720, "V2"=w719, "V3"=w718, "V4"=w714) -> (w728:T35)
            n337 = global write "GlobalVariables.vi" "SysCaliData"(w728) -> ()
          }
          frame Error {
          }
        }
        n338 = call <vilib>:"Add State(s) to Queue__JKI_lib_State_Machine.vi"("State(s) in (\"\")"=w712) -> ("States Out"=w711:string)  [unwired: 14 in]
      }
      frame "Data: LoadiRFFromAPDFile" {
        w758 = T17 {"Ch1 iRF"=[], "Ch2 iRF"=[], "Ch3 iRF"=[], "Ch4 iRF"=[]}  # LastUseiRF
        # "only load the last 5th  iRF for the moment"
        # "Load APD detector data\n(It is a separator no-op. You can make a copy of this frame to create a new Data frame)"
        n339 = Unbundle By Name(w780) -> ("APDSerialNum.Ch1APDSerial#"=w779:string, "APDSerialNum.Ch2APDSerial#"=w760:string, "APDSerialNum.Ch3APDSerial#"=w759:string, "APDSerialNum.Ch4APDSerial#"=w756:string)
        n340 = call "CreatFromSerialNumNoRaw.vi"("error in (no error)"=w757, "APD Serial #"=w779) -> ("error out"=w777:errorcluster, "APDClass out"=w778:refnum<class "APDClass.lvclass">)  [unwired: 8 in]
        n341 = call "CreatFromSerialNumNoRaw.vi"("error in (no error)"=w757, "APD Serial #"=w760) -> ("error out"=w768:errorcluster, "APDClass out"=w769:refnum<class "APDClass.lvclass">)  [unwired: 8 in]
        n342 = call "CreatFromSerialNumNoRaw.vi"("error in (no error)"=w757, "APD Serial #"=w759) -> ("error out"=w762:errorcluster, "APDClass out"=w763:refnum<class "APDClass.lvclass">)  [unwired: 8 in]
        n343 = call "CreatFromSerialNumNoRaw.vi"("error in (no error)"=w757, "APD Serial #"=w756) -> ("error out"=w754:errorcluster, "APDClass out"=w755:refnum<class "APDClass.lvclass">)  [unwired: 8 in]
        n344 = call-dynamic "Read iRFData.vi"("error in (no error)"=w777, "APDClass in"=w778) -> ("iRFData"=w776:T36)  [unwired: 7 in, 2 out]
        n345 = call-dynamic "Read iRFData.vi"("error in (no error)"=w768, "APDClass in"=w769) -> ("iRFData"=w772:T36)  [unwired: 7 in, 2 out]
        n346 = call-dynamic "Read iRFData.vi"("error in (no error)"=w762, "APDClass in"=w763) -> ("iRFData"=w766:T36)  [unwired: 7 in, 2 out]
        n347 = call-dynamic "Read iRFData.vi"("error in (no error)"=w754, "APDClass in"=w755) -> ("iRFData"=w753:T36)  [unwired: 7 in, 2 out]
        n348 = Unbundle By Name(w776) -> ("iRFWFsAvg"=w775:dbl[][])
        n349 = Unbundle By Name(w772) -> ("iRFWFsAvg"=w771:dbl[][])
        n350 = Unbundle By Name(w766) -> ("iRFWFsAvg"=w765:dbl[][])
        n351 = Unbundle By Name(w753) -> ("iRFWFsAvg"=w750:dbl[][])
        n352 = Array Size(array=w775) -> (size(s)=w774:i32[])
        n353 = Array Size(array=w771) -> (size(s)=w767:i32[])
        n354 = Array Size(array=w765) -> (size(s)=w761:i32[])
        n355 = Array Size(array=w750) -> (size(s)=w751:i32[])
        n356 = Index Array(array=w774, index=0) -> (element=w749:i32)
        n357 = Index Array(array=w767, index=0) -> (element=w745:i32)
        n358 = Index Array(array=w761, index=0) -> (element=w742:i32)
        n359 = Index Array(array=w751, index=0) -> (element=w739:i32)
        n360 = Subtract(x=w749, y=5) -> (x-y=w747:i32)
        n361 = Subtract(x=w745, y=5) -> (x-y=w744:i32)
        n362 = Subtract(x=w742, y=5) -> (x-y=w741:i32)
        n363 = Subtract(x=w739, y=5) -> (x-y=w738:i32)
        n364 = Index Array(array=w775, index (row)=w747) -> (element=w737:dbl[])  [unwired: 1 in]
        n365 = Index Array(array=w771, index (row)=w744) -> (element=w736:dbl[])  [unwired: 1 in]
        n366 = Index Array(array=w765, index (row)=w741) -> (element=w735:dbl[])  [unwired: 1 in]
        n367 = Index Array(array=w750, index (row)=w738) -> (element=w734:dbl[])  [unwired: 1 in]
        n368 = call "DownSampleAndShiftiRF (SubVI).vi"("ArrayIn"=w737) -> ("ArrayOut"=w733:dbl[])  [unwired: 10 in]
        n369 = call "DownSampleAndShiftiRF (SubVI).vi"("ArrayIn"=w736) -> ("ArrayOut"=w729:dbl[])  [unwired: 10 in]
        n370 = call "DownSampleAndShiftiRF (SubVI).vi"("ArrayIn"=w735) -> ("ArrayOut"=w730:dbl[])  [unwired: 10 in]
        n371 = call "DownSampleAndShiftiRF (SubVI).vi"("ArrayIn"=w734) -> ("ArrayOut"=w732:dbl[])  [unwired: 10 in]
        n372 = call <vilib>:"Add State(s) to Queue__JKI_lib_State_Machine.vi"("State(s) in (\"\")"=w783) -> ("States Out"=w782:string)  [unwired: 14 in]
        n373 = Bundle(cluster=w758, "Ch1 iRF"=w733, "Ch2 iRF"=w729, "Ch3 iRF"=w730, "Ch4 iRF"=w732) -> (w731:T17)
        n374 = global write "GlobalVariables.vi" "LastUseiRF"(w731) -> ()
      }
      frame "Data: loadLastUseiRF" {
        # "Load last use iRF.\n()"
        n375 = Unbundle By Name(w789) -> ("TempPath"=w788:path)
        n376 = Build Path(base path=w788, name or relative path="iRF.tdms") -> (appended path=w794:path)
        n377 = TDMS Open(8:w784, 11:w794) -> (0:w792:errorcluster, 3:w793:refnum<k34>)  [unwired: 5 in]
        n378 = TDMS Read(0:w793, 11:w792, 12:dbl[][] []) -> (4:w787:refnum<k34>, 10:w790:dbl[][], 15:w786:errorcluster)  [unwired: 5 in, 3 out]
        n379 = TDMS Close(8:w786, 11:w787) -> (0:w785:errorcluster)  [unwired: 1 out]
        n380 = case shown="No Error" w786 {
          tunnel: w790 -> [w804 _]
          frame No Error {
            w807 = T17 {"Ch1 iRF"=[], "Ch2 iRF"=[], "Ch3 iRF"=[], "Ch4 iRF"=[]}  # LastUseiRF
            n381 = Index Array(array=w804, index (row)=0) -> (element=w799:dbl[])  [unwired: 1 in]
            n382 = Index Array(array=w804, index (row)=1) -> (element=w800:dbl[])  [unwired: 1 in]
            n383 = Index Array(array=w804, index (row)=2) -> (element=w801:dbl[])  [unwired: 1 in]
            n384 = Index Array(array=w804, index (row)=3) -> (element=w802:dbl[])  [unwired: 1 in]
            n385 = Add Array Elements(numeric array=w799) -> (sum=w813:dbl)
            n386 = Add Array Elements(numeric array=w800) -> (sum=w811:dbl)
            n387 = Add Array Elements(numeric array=w801) -> (sum=w809:dbl)
            n388 = Add Array Elements(numeric array=w802) -> (sum=w805:dbl)
            n389 = Divide(x=w799, y=w813) -> (x/y=w812:dbl[])
            n390 = Divide(x=w800, y=w811) -> (x/y=w810:dbl[])
            n391 = Divide(x=w801, y=w809) -> (x/y=w808:dbl[])
            n392 = Divide(x=w802, y=w805) -> (x/y=w803:dbl[])
            n393 = Bundle(cluster=w807, "Ch1 iRF"=w812, "Ch2 iRF"=w810, "Ch3 iRF"=w808, "Ch4 iRF"=w803) -> (w815:T17)
            n394 = Array Size(array=w799) -> (size(s)=→"iRF length":i32)
            n395 = global write "GlobalVariables.vi" "LastUseiRF"(w815) -> ()
          }
          frame Error {
          }
        }
        n396 = call <vilib>:"Add State(s) to Queue__JKI_lib_State_Machine.vi"("State(s) in (\"\")"=w798) -> ("States Out"=w797:string)  [unwired: 14 in]
      }
      frame "Data: ShowiRF" {
        # "Show loaded iRF.\n(It is a separator no-op. You can make a copy of this frame to create a new Data frame)"
        n397 = global read "GlobalVariables.vi" "LastUseiRF"() -> (w824:T17)
        n398 = Unbundle By Name(w824) -> ("Ch1 iRF"=w823:dbl[], "Ch2 iRF"=w822:dbl[], "Ch3 iRF"=w821:dbl[], "Ch4 iRF"=w820:dbl[])
        n399 = Build Array(w823, w822, w821, w820) -> (→"iRF Graph":dbl[][])
        n400 = call <vilib>:"Add State(s) to Queue__JKI_lib_State_Machine.vi"("State(s) in (\"\")"=w829) -> ("States Out"=w828:string)  [unwired: 14 in]
      }
      frame "Data: saveCalibration" {
        # "Average data and save calibration file. [Covers: REQ11]\n(It is a separator no-op. You can make a copy of this frame to create a new Data frame)"
        n401 = Unbundle By Name(w848) -> ("Ch1Data"=w847:dbl[][], "V1"=w846:dbl[], "Ch2Data"=w845:dbl[][], "V2"=w844:dbl[], "Ch3Data"=w843:dbl[][], "V3"=w842:dbl[], "Ch4Data"=w833:dbl[][], "V4"=w832:dbl[], "Pathes.CaliPath"=w851:path, "IDs.Cali ID"=w850:i8)
        n402 = Increment(x=w850) -> (x+1=w834:i8)
        n403 = Bundle("Ch1Data"=w847, "V1"=w846) -> (w841:cluster{"Ch1Data":dbl[][], "V1":dbl[]})  [unwired: 1 in]
        n404 = Bundle("Ch4Data"=w833, "V4"=w832) -> (w831:cluster{"Ch4Data":dbl[][], "V4":dbl[]})  [unwired: 1 in]
        n405 = Bundle("Ch2Data"=w845, "V2"=w844) -> (w840:cluster{"Ch2Data":dbl[][], "V2":dbl[]})  [unwired: 1 in]
        n406 = Bundle("Ch3Data"=w843, "V3"=w842) -> (w839:cluster{"Ch3Data":dbl[][], "V3":dbl[]})  [unwired: 1 in]
        n407 = Format Value(string ("")="Calibration" ("default name"), format string="%02d", value (0)=w834) -> (output string=w853:string)
        n408 = Build Path(base path=w851, name or relative path=w853) -> (appended path=w838:path)
        n409 = call "SaveBGorCali(SubVI).vi"("Channel1"=w841, "BG path"=w838, "DataType"=enum16{"BG", "Cali"}."Cali", "Channel 2"=w840, "Channel 3"=w839, "Channel 4"=w831, "error in (no error)"=w837, "SytemID"="UCDVetMed") -> ("error out"=w836:errorcluster)  [unwired: 7 in]
        n410 = call <vilib>:"Add State(s) to Queue__JKI_lib_State_Machine.vi"("State(s) in (\"\")"=w856) -> ("States Out"=w855:string)  [unwired: 14 in]
      }
      frame "Data: saveiRF" {
        w862 = enum16{"write", "read"}."read" ("action")
        # "Get iRF from decon stracture and save it on disk.\n(It is a separator no-op. You can make a copy of this frame to create a new Data frame)"
        n411 = Unbundle By Name(w879) -> ("TempPath"=w878:path)
        n412 = call "Ch1DeconEngineFGV.vi"("action(read)"=w862) -> ("Error Out"=w884:errorcluster, "Ch1DeconEngine out"=w885:refnum<class "LaguerreDeconEngineClass.lvclass">)  [unwired: 9 in]
        n413 = call "Ch2DeconEngineFGV.vi"("action(read)"=w862) -> ("Error Out"=w882:errorcluster, "Ch2DeconEngine out"=w883:refnum<class "LaguerreDeconEngineClass.lvclass">)  [unwired: 9 in]
        n414 = call "Ch3DeconEngineFGV.vi"("action(read)"=w862) -> ("Error Out"=w880:errorcluster, "Ch3DeconEngine out"=w881:refnum<class "LaguerreDeconEngineClass.lvclass">)  [unwired: 9 in]
        n415 = call "Ch4DeconEngineFGV.vi"("action(read)"=w862) -> ("Error Out"=w861:errorcluster, "Ch3DeconEngine out"=w860:refnum<class "LaguerreDeconEngineClass.lvclass">)  [unwired: 9 in]
        n416 = Build Path(base path=w878, name or relative path="iRF" ("default name")) -> (appended path=w876:path)
        n417 = call "getIRF.vi"("error in (no error)"=w861, "LaguerreDeconEngineClass in"=w860) -> ("iRF"=w859:dbl[])  [unwired: 7 in, 2 out]
        n418 = call "getIRF.vi"("error in (no error)"=w884, "LaguerreDeconEngineClass in"=w885) -> ("iRF"=w867:dbl[])  [unwired: 7 in, 2 out]
        n419 = call "getIRF.vi"("error in (no error)"=w882, "LaguerreDeconEngineClass in"=w883) -> ("iRF"=w866:dbl[])  [unwired: 7 in, 2 out]
        n420 = call "getIRF.vi"("error in (no error)"=w880, "LaguerreDeconEngineClass in"=w881) -> ("iRF"=w865:dbl[])  [unwired: 7 in, 2 out]
        n421 = TDMS Open(8:w875, 10:T16."create or replace" ("operation (0:open)"), 11:w876) -> (0:w872:errorcluster, 3:w873:refnum<k34>)  [unwired: 4 in]
        n422 = Bundle(cluster=T17 {"Ch1 iRF"=[], "Ch2 iRF"=[], "Ch3 iRF"=[], "Ch4 iRF"=[]} ("LastUseiRF"), "Ch1 iRF"=w867, "Ch2 iRF"=w866, "Ch3 iRF"=w865, "Ch4 iRF"=w859) -> (w863:T17)
        n423 = Build Array(w867, w866, w865, w859) -> (w871:dbl[][])
        n424 = global write "GlobalVariables.vi" "LastUseiRF"(w863) -> ()
        n425 = TDMS Write(0:w873, 5:"iRF" ("group name in (Untitled)"), 7:string[] ["Ch1", "Ch2", "Ch3", "Ch4"] ("channel name(s) in (Untitled)"), 9:w871, 11:w872) -> (4:w870:refnum<k34>, 15:w869:errorcluster)  [unwired: 1 in, 2 out]
        n426 = TDMS Close(8:w869, 11:w870) -> (0:w868:errorcluster)  [unwired: 1 out]
        n427 = call <vilib>:"Add State(s) to Queue__JKI_lib_State_Machine.vi"("State(s) in (\"\")"=w888) -> ("States Out"=w887:string)  [unwired: 14 in]
      }
      frame "Data: saveBGtoFGV" {
        w903 = enum16{"write", "read"}."write" ("action")
        # "Save BG and pass it to FGV.\n(save BG to disk and set it to FGV)"
        n428 = Unbundle By Name(w904) -> ("Ch1Data"=w897:dbl[][], "Ch2Data"=w895:dbl[][], "Ch3Data"=w893:dbl[][], "Ch4Data"=w891:dbl[][])
        n429 = call "AvgArrayTimeCritical.vi"("2D array"=w895) -> ("1D Avg"=w894:dbl[])  [unwired: 10 in]
        n430 = call "AvgArrayTimeCritical.vi"("2D array"=w893) -> ("1D Avg"=w892:dbl[])  [unwired: 10 in]
        n431 = call "AvgArrayTimeCritical.vi"("2D array"=w897) -> ("1D Avg"=w896:dbl[])  [unwired: 10 in]
        n432 = call "AvgArrayTimeCritical.vi"("2D array"=w891) -> ("1D Avg"=w890:dbl[])  [unwired: 10 in]
        n433 = call "BG1FGV.vi"("Error In"=w889, "action"=w903, "BG1 in"=w896) -> ("Error Out"=w902:errorcluster)  [unwired: 7 in, 1 out]
        n434 = call "BG2FGV.vi"("Error In"=w889, "action"=w903, "BG2 in"=w894) -> ("Error Out"=w901:errorcluster)  [unwired: 7 in, 1 out]
        n435 = call "BG3FGV.vi"("Error In"=w889, "action"=w903, "BG3 in"=w892) -> ("Error Out"=w900:errorcluster)  [unwired: 7 in, 1 out]
        n436 = call "BG4FGV.vi"("Error In"=w889, "action"=w903, "BG4 in"=w890) -> ("Error Out"=w899:errorcluster)  [unwired: 7 in, 1 out]
        n437 = Merge Errors(w902, w901, w900, w899) -> (w898:errorcluster)
        n438 = call <vilib>:"Add State(s) to Queue__JKI_lib_State_Machine.vi"("State(s) in (\"\")"=w907) -> ("States Out"=w906:string)  [unwired: 14 in]
      }
      frame "Data: saveBGtoFile" {
        w929 = "Background" ("name or relative path")
        # "Save BG to file.\n(save BG to disk both data folder and temp folder)"
        n439 = Unbundle By Name(w933) -> ("Pathes.BG Path"=w926:path, "IDs.BG ID"=w925:i8, "Ch1Data"=w923:dbl[][], "V1"=w922:dbl[], "Ch2Data"=w921:dbl[][], "V2"=w920:dbl[], "Ch3Data"=w919:dbl[][], "V3"=w918:dbl[], "Ch4Data"=w910:dbl[][], "V4"=w909:dbl[], "TempPath"=w931:path)
        n440 = Increment(x=w925) -> (x+1=w930:i8)
        n441 = Format Value(string ("")=w929, format string="%02d", value (0)=w930) -> (output string=w928:string)
        n442 = Build Path(base path=w931, name or relative path=w929) -> (appended path=w912:path)
        n443 = call "File Dialog2"("start path"=w926, "prompt"="Please select BG name, DO NOT CANCEL!", "default name"=w928) -> ("selected path"=w913:path)  [unwired: 9 in, 3 out]
        n444 = Bundle("Ch1Data"=w923, "V1"=w922) -> (w917:cluster{"Ch1Data":dbl[][], "V1":dbl[]})  [unwired: 1 in]
        n445 = Bundle("Ch4Data"=w910, "V4"=w909) -> (w908:cluster{"Ch4Data":dbl[][], "V4":dbl[]})  [unwired: 1 in]
        n446 = Bundle("Ch2Data"=w921, "V2"=w920) -> (w916:cluster{"Ch2Data":dbl[][], "V2":dbl[]})  [unwired: 1 in]
        n447 = Bundle("Ch3Data"=w919, "V3"=w918) -> (w915:cluster{"Ch3Data":dbl[][], "V3":dbl[]})  [unwired: 1 in]
        n448 = Build Array(w913, w912) -> (w911:path[])
        n449 = for {
          tunnel: w917 -> [w944]
          tunnel: w916 -> [w943]
          tunnel: w915 -> [w942]
          shift-right: [w945] -> w924
          shift-left: w914 -> [w941]
          tunnel: w911 -> [w940] mode=indexing
          tunnel: w908 -> [w938]
          n450 = call "SaveBGorCali(SubVI).vi"("Channel1"=w944, "BG path"=w940, "DataType"=enum16{"BG", "Cali"}."BG", "Channel 2"=w943, "Channel 3"=w942, "Channel 4"=w938, "error in (no error)"=w941, "SytemID"="UCDMC") -> ("error out"=w945:errorcluster)  [unwired: 7 in]
        }
        n451 = call <vilib>:"Add State(s) to Queue__JKI_lib_State_Machine.vi"("State(s) in (\"\")"=w936) -> ("States Out"=w935:string)  [unwired: 14 in]
      }
      frame "Data: processDeConBG" {
        # "Save BG and pass it to FGV.\n(save BG to disk and set it to FGV)"
        n452 = call "DotNetFGV.vi"("Error In"=w957) -> ("Error Out"=w958:errorcluster, "reference out"=w959:refnum<k24>)  [unwired: 9 in]
        n453 = Unbundle By Name(w963) -> ("Ch1Data"=w952:dbl[][], "Ch2Data"=w950:dbl[][], "Ch3Data"=w951:dbl[][])  [unwired: 1 out]
        n454 = Transpose 2D Array(2D array=w952) -> (transposed array=w962:dbl[][])
        n455 = Transpose 2D Array(2D array=w950) -> (transposed array=w961:dbl[][])
        n456 = Transpose 2D Array(2D array=w951) -> (transposed array=w960:dbl[][])
        n457 = call "WaveformTUABG(SubVI).vi"("error in (no error)"=w958, "WF in"=w962, "new reference"=w959) -> ("error out"=w949:errorcluster, "WF out"=w953:dbl[])  [unwired: 6 in, 1 out]
        n458 = call "WaveformTUABG(SubVI).vi"("error in (no error)"=w958, "WF in"=w961, "new reference"=w959) -> ("error out"=w948:errorcluster, "WF out"=w955:dbl[])  [unwired: 6 in, 1 out]
        n459 = call "WaveformTUABG(SubVI).vi"("error in (no error)"=w958, "WF in"=w960, "new reference"=w959) -> ("error out"=w947:errorcluster, "WF out"=w954:dbl[])  [unwired: 6 in, 1 out]
        n460 = Build Array(w953, w955, w954) -> (→"BGAll" →"BG Graph":dbl[][])
        n461 = Merge Errors(w949, w948, w947) -> (w956:errorcluster)
        n462 = call <vilib>:"Add State(s) to Queue__JKI_lib_State_Machine.vi"("State(s) in (\"\")"=w966) -> ("States Out"=w965:string)  [unwired: 14 in]
      }
      frame "Data: saveDeConBGtoFile" {
        # "Save realtime DeCon BG to temp file.\n(It is a separator no-op. You can make a copy of this frame to create a new Data frame)"
        n463 = Unbundle By Name(w980) -> ("TempPath"=w979:path)
        n464 = Build Path(base path=w979, name or relative path="RealTimeDeConBGTemp") -> (appended path=w977:path)
        n465 = local read "BGAll"() -> (w973:dbl[][])
        n466 = TDMS Open(8:w975, 10:T16."create or replace" ("operation (0:open)"), 11:w977) -> (0:w972:errorcluster, 3:w974:refnum<k34>)  [unwired: 4 in]
        n467 = TDMS Write(0:w974, 5:"Realtime DeCon BG" ("group name in (Untitled)"), 7:string[] ["Ch1", "Ch2", "Ch3"], 9:w973, 11:w972) -> (4:w969:refnum<k34>, 15:w968:errorcluster)  [unwired: 1 in, 2 out]
        n468 = TDMS Close(8:w968, 11:w969) -> (0:w967:errorcluster)  [unwired: 1 out]
        n469 = call <vilib>:"Add State(s) to Queue__JKI_lib_State_Machine.vi"("State(s) in (\"\")"=w983) -> ("States Out"=w982:string)  [unwired: 14 in]
      }
      frame "Data: showBG" {
        # "Show BG in seperate window.\n()"
        n470 = call "showBG.vi"() -> ()  [unwired: 12 in]
        n471 = call <vilib>:"Add State(s) to Queue__JKI_lib_State_Machine.vi"("State(s) in (\"\")"=w988) -> ("States Out"=w987:string)  [unwired: 14 in]
      }
      frame "Data: irfAlignment" {
        w989 = enum16{"write", "read"}."write" ("action")
        # "do iRF alignment in this state\n(It is a separator no-op. You can make a copy of this frame to create a new Data frame)"
        n472 = Unbundle By Name(w1034) -> ("Ch1Data"=w1070:dbl[][], "Ch2Data"=w1069:dbl[][], "Ch3Data"=w1068:dbl[][], "Ch4Data"=w1011:dbl[][])
        n473 = call "Ch1DeconEngineFGV.vi"("Error In"=w1010) -> ("Error Out"=w1066:errorcluster, "Ch1DeconEngine out"=w1067:refnum<class "LaguerreDeconEngineClass.lvclass">)  [unwired: 9 in]
        n474 = call "Ch2DeconEngineFGV.vi"("Error In"=w1010) -> ("Error Out"=w1064:errorcluster, "Ch2DeconEngine out"=w1065:refnum<class "LaguerreDeconEngineClass.lvclass">)  [unwired: 9 in]
        n475 = call "Ch3DeconEngineFGV.vi"("Error In"=w1010) -> ("Error Out"=w1062:errorcluster, "Ch3DeconEngine out"=w1063:refnum<class "LaguerreDeconEngineClass.lvclass">)  [unwired: 9 in]
        n476 = call "Ch4DeconEngineFGV.vi"("Error In"=w1010) -> ("Error Out"=w1001:errorcluster, "Ch3DeconEngine out"=w1000:refnum<class "LaguerreDeconEngineClass.lvclass">)  [unwired: 9 in]
        n477 = call "AvgArray.vi"("2D array in"=w1069) -> ("1D Avg out"=w1016:dbl[])  [unwired: 10 in]
        n478 = call "AvgArray.vi"("2D array in"=w1068) -> ("1D Avg out"=w1015:dbl[])  [unwired: 10 in]
        n479 = call "AvgArray.vi"("2D array in"=w1011) -> ("1D Avg out"=w990:dbl[])  [unwired: 10 in]
        n480 = call "AvgArray.vi"("2D array in"=w1070) -> ("1D Avg out"=w1017:dbl[])  [unwired: 10 in]
        n481 = call "RemoveDCBG.vi"("WF in"=w1017) -> ("DC"=w1024:dbl, "WF out"=w1014:dbl[])  [unwired: 8 in, 1 out]
        n482 = call "RemoveDCBG.vi"("WF in"=w1016) -> ("DC"=w1021:dbl, "WF out"=w1027:dbl[])  [unwired: 8 in, 1 out]
        n483 = call "RemoveDCBG.vi"("WF in"=w1015) -> ("DC"=w1019:dbl, "WF out"=w1026:dbl[])  [unwired: 8 in, 1 out]
        n484 = call "RemoveDCBG.vi"("WF in"=w990) -> ("DC"=w994:dbl, "WF out"=w992:dbl[])  [unwired: 8 in, 1 out]
        n485 = call "computeIRFAlignment.vi"("error in (no error)"=w1066, "fIRF temp"=w1014, "LaguerreDeconEngineClass in"=w1067) -> ("error out"=w1058:errorcluster, "LaguerreDeconEngineClass out"=w1059:refnum<class "LaguerreDeconEngineClass.lvclass">)  [unwired: 6 in, 1 out]
        n486 = call "computeIRFAlignment.vi"("error in (no error)"=w1064, "fIRF temp"=w1027, "LaguerreDeconEngineClass in"=w1065) -> ("error out"=w1056:errorcluster, "LaguerreDeconEngineClass out"=w1057:refnum<class "LaguerreDeconEngineClass.lvclass">)  [unwired: 6 in, 1 out]
        n487 = call "computeIRFAlignment.vi"("error in (no error)"=w1062, "fIRF temp"=w1026, "LaguerreDeconEngineClass in"=w1063) -> ("error out"=w1060:errorcluster, "LaguerreDeconEngineClass out"=w1061:refnum<class "LaguerreDeconEngineClass.lvclass">)  [unwired: 6 in, 1 out]
        n488 = call "computeIRFAlignment.vi"("error in (no error)"=w1001, "fIRF temp"=w992, "LaguerreDeconEngineClass in"=w1000) -> ("error out"=w1008:errorcluster, "LaguerreDeconEngineClass out"=w1009:refnum<class "LaguerreDeconEngineClass.lvclass">)  [unwired: 6 in, 1 out]
        n489 = call "Ch1DeconEngineFGV.vi"("Error In"=w1058, "action(read)"=w989, "Ch1DeconEngine in"=w1059) -> ("Error Out"=w1054:errorcluster, "Ch1DeconEngine out"=w1055:refnum<class "LaguerreDeconEngineClass.lvclass">)  [unwired: 7 in]
        n490 = call "Ch2DeconEngineFGV.vi"("Error In"=w1056, "action(read)"=w989, "Ch2DeconEngine in"=w1057) -> ("Error Out"=w1044:errorcluster, "Ch2DeconEngine out"=w1045:refnum<class "LaguerreDeconEngineClass.lvclass">)  [unwired: 7 in]
        n491 = call "Ch3DeconEngineFGV.vi"("Error In"=w1060, "action(read)"=w989, "Ch3DeconEngine in"=w1061) -> ("Error Out"=w1038:errorcluster, "Ch3DeconEngine out"=w1039:refnum<class "LaguerreDeconEngineClass.lvclass">)  [unwired: 7 in]
        n492 = call "Ch4DeconEngineFGV.vi"("Error In"=w1008, "action(read)"=w989, "Ch3DeconEngine in"=w1009) -> ("Error Out"=w1002:errorcluster, "Ch3DeconEngine out"=w1003:refnum<class "LaguerreDeconEngineClass.lvclass">)  [unwired: 7 in]
        n493 = call "setfIRF.vi"("error in (no error)"=w1038, "fIRF"=w1026, "LaguerreDeconEngineClass in"=w1039) -> ("error out"=w1042:errorcluster, "LaguerreDeconEngineClass out"=w1043:refnum<class "LaguerreDeconEngineClass.lvclass">)  [unwired: 7 in]
        n494 = call "setfIRF.vi"("error in (no error)"=w1002, "fIRF"=w992, "LaguerreDeconEngineClass in"=w1003) -> ("error out"=w1006:errorcluster, "LaguerreDeconEngineClass out"=w1007:refnum<class "LaguerreDeconEngineClass.lvclass">)  [unwired: 7 in]
        n495 = call "setfIRF.vi"("error in (no error)"=w1044, "fIRF"=w1027, "LaguerreDeconEngineClass in"=w1045) -> ("error out"=w1048:errorcluster, "LaguerreDeconEngineClass out"=w1049:refnum<class "LaguerreDeconEngineClass.lvclass">)  [unwired: 7 in]
        n496 = call "setfIRF.vi"("error in (no error)"=w1054, "fIRF"=w1014, "LaguerreDeconEngineClass in"=w1055) -> ("error out"=w1052:errorcluster, "LaguerreDeconEngineClass out"=w1053:refnum<class "LaguerreDeconEngineClass.lvclass">)  [unwired: 7 in]
        n497 = Unbundle By Name(w1034) -> ("V1"=w1013:dbl[], "V2"=w1033:dbl[], "V3"=w1032:dbl[], "V4"=w999:dbl[])
        n498 = call "computeLCs.vi"("error in (no error)"=w1052, "LaguerreDeconClass in"=w1053) -> ("error out"=w1050:errorcluster, "LaguerreDeconClass out"=w1051:refnum<class "LaguerreDeconEngineClass.lvclass">)  [unwired: 8 in]
        n499 = call "computeLCs.vi"("error in (no error)"=w1048, "LaguerreDeconClass in"=w1049) -> ("error out"=w1046:errorcluster, "LaguerreDeconClass out"=w1047:refnum<class "LaguerreDeconEngineClass.lvclass">)  [unwired: 8 in]
        n500 = call "computeLCs.vi"("error in (no error)"=w1042, "LaguerreDeconClass in"=w1043) -> ("error out"=w1040:errorcluster, "LaguerreDeconClass out"=w1041:refnum<class "LaguerreDeconEngineClass.lvclass">)  [unwired: 8 in]
        n501 = call "computeLCs.vi"("error in (no error)"=w1006, "LaguerreDeconClass in"=w1007) -> ("error out"=w1004:errorcluster, "LaguerreDeconClass out"=w1005:refnum<class "LaguerreDeconEngineClass.lvclass">)  [unwired: 8 in]
        n502 = call-poly <vilib>:"Mean.vi"("X"=w1013) -> ("mean"=w1012:dbl)  [unwired: 1 out]
        n503 = call-poly <vilib>:"Mean.vi"("X"=w999) -> ("mean"=w998:dbl)  [unwired: 1 out]
        n504 = call-poly <vilib>:"Mean.vi"("X"=w1033) -> ("mean"=w1031:dbl)  [unwired: 1 out]
        n505 = call "getFitting.vi"("error in (no error)"=w1050, "LaguerreDeconEngineClass in"=w1051) -> ("Fitting"=w1023:dbl[])  [unwired: 7 in, 2 out]
        n506 = call "getFitting.vi"("error in (no error)"=w1046, "LaguerreDeconEngineClass in"=w1047) -> ("Fitting"=w1020:dbl[])  [unwired: 7 in, 2 out]
        n507 = call "getFitting.vi"("error in (no error)"=w1040, "LaguerreDeconEngineClass in"=w1041) -> ("Fitting"=w996:dbl[])  [unwired: 7 in, 2 out]
        n508 = call "getFitting.vi"("error in (no error)"=w1004, "LaguerreDeconEngineClass in"=w1005) -> ("Fitting"=w995:dbl[])  [unwired: 7 in, 2 out]
        n509 = Add(x=w1024, y=w1023) -> (x+y=w1025:dbl[])
        n510 = Add(x=w1021, y=w1020) -> (x+y=w1022:dbl[])
        n511 = call-poly <vilib>:"Mean.vi"("X"=w1032) -> ("mean"=w1030:dbl)  [unwired: 1 out]
        n512 = Add(x=w1019, y=w996) -> (x+y=w1018:dbl[])
        n513 = Build Array(w1017, w1025) -> (w1037:dbl[][])
        n514 = Build Array(w1016, w1022) -> (w1036:dbl[][])
        n515 = Build Array(w1015, w1018) -> (w1035:dbl[][])
        n516 = Add(x=w994, y=w995) -> (x+y=w993:dbl[])
        n517 = Bundle("mean"=w1012, "mean"=w1031, "mean"=w1030, "mean"=w998) -> (w997:T37)  [unwired: 1 in]
        n518 = Build Array(w990, w993) -> (w991:dbl[][])
        n519 = call "Calib_and_iRFAlign_confirm.vi"("Current V"=w997, "Ch4 Data"=w991, "Ch3 Data"=w1035, "Ch2 Data"=w1036, "Ch1 Data"=w1037) -> ("Save?"=w1029:bool)  [unwired: 6 in]
        n520 = case shown="True" w1029 {
          tunnel: ["" ("Empty String Constant") "Data: saveCalibration\nData: saveiRF\nRun: CaliIncrement"] -> w1028
          frame False {
          }
          frame True {
            # "[Covers: REQ2]"
          }
        }
        n521 = call <vilib>:"Add State(s) to Queue__JKI_lib_State_Machine.vi"("State(s) in Front (\"\")"=w1028, "State(s) in (\"\")"=w1073) -> ("States Out"=w1072:string)  [unwired: 13 in]
      }
      frame "Data: parseRunData" {
        # "All APD bias"
        # "flash queue"
        # "Ch3&4"
        # "Ch1&2"
        # "Flash data from queue and save it in structure\n()"
        n522 = Flush Queue(queue=w1101, error in (no error)=w1100) -> (remaining elements=w1095:T38, error out=w1096:errorcluster)  [unwired: 1 out]
        n523 = Flush Queue(queue=w1106, error in (no error)=w1100) -> (remaining elements=w1104:cluster{"double data":dbl[][]}[], error out=w1097:errorcluster)  [unwired: 1 out]
        n524 = Flush Queue(queue=w1107, error in (no error)=w1100) -> (remaining elements=w1105:cluster{"double data":dbl[][]}[], error out=w1098:errorcluster)  [unwired: 1 out]
        n525 = for {
          tunnel: w1105 -> [w1123] mode=indexing
          tunnel: [w1121] -> w1090 mode=concatenating
          tunnel: [w1120] -> w1091 mode=concatenating
          n526 = Unbundle By Name(w1123) -> ("double data"=w1122:dbl[][])
          n527 = call "SeperateChanData.vi"("Input (Ch1&2)"=w1122) -> ("Ch1"=w1121:dbl[][], "Ch2"=w1120:dbl[][])
        }
        n528 = for {
          tunnel: w1104 -> [w1119] mode=indexing
          tunnel: [w1118] -> w1080 mode=concatenating
          tunnel: [w1116] -> w1081 mode=concatenating
          n529 = Unbundle By Name(w1119) -> ("double data"=w1117:dbl[][])
          n530 = call "SeperateChanData.vi"("Input (Ch1&2)"=w1117) -> ("Ch1"=w1118:dbl[][], "Ch2"=w1116:dbl[][])
        }
        n531 = call "FLImDAQ_FGV.vi"() -> ("Read data"=w1088:T5)  [unwired: 10 in, 1 out]
        n532 = Unbundle By Name(w1088) -> ("Waveform to Avg"=w1078:i16)
        n533 = for {
          tunnel: w1095 -> [w1115] mode=indexing
          tunnel: [w1114] -> w1087 mode=indexing
          tunnel: [w1113] -> w1085 mode=indexing
          tunnel: [w1112] -> w1083 mode=indexing
          tunnel: [w1111] -> w1079 mode=indexing
          n534 = Unbundle By Name(w1115) -> ("V1"=w1114:dbl, "V2"=w1113:dbl, "V3"=w1112:dbl, "V4"=w1111:dbl)
        }
        n535 = call "DuplicateV(SubVI).vi"("Averaging"=w1078, "V in"=w1087) -> ("V out"=w1086:dbl[])  [unwired: 9 in]
        n536 = Array Size(array=w1080) -> (size(s)=→"data Size":i32[])
        n537 = call "DuplicateV(SubVI).vi"("Averaging"=w1078, "V in"=w1085) -> ("V out"=w1084:dbl[])  [unwired: 9 in]
        n538 = call "DuplicateV(SubVI).vi"("Averaging"=w1078, "V in"=w1083) -> ("V out"=w1082:dbl[])  [unwired: 9 in]
        n539 = call "DuplicateV(SubVI).vi"("Averaging"=w1078, "V in"=w1079) -> ("V out"=w1076:dbl[])  [unwired: 9 in]
        n540 = Bundle By Name(cluster=w1102, "Ch1Data"=w1090, "Ch2Data"=w1091, "Ch3Data"=w1080, "Ch4Data"=w1081, "V1"=w1086, "V2"=w1084, "V3"=w1082, "V4"=w1076) -> (w1103:T24)
        n541 = Merge Errors(w1098, w1097, w1096) -> (w1099:errorcluster)
        n542 = Array Size(array=w1086) -> (size(s)=→"V1 Size":i32)
        n543 = Array Size(array=w1084) -> (size(s)=→"V2 Size":i32)
        n544 = Array Size(array=w1082) -> (size(s)=→"V3 Size":i32)
        n545 = Array Size(array=w1076) -> (size(s)=→"V4 Size":i32)
        n546 = call <vilib>:"Add State(s) to Queue__JKI_lib_State_Machine.vi"("State(s) in (\"\")"=w1110) -> ("States Out"=w1109:string)  [unwired: 14 in]
      }
      frame "Data: saveRunData" {
        w1126 = T39 {"DataPath"=path "", "CaseID"="", "RunID"=0, "Ch1Data"=[], "Ch2Data"=[], "Ch3Data"=[], "Ch4Data"=[], "V1"=[], "V2"=[], "V3"=[], "V4"=[], "LaserRepRate"=0, "WFAverage"=0, "RunStartTime"=0}  # Data cluster
        # "Save FLIm data to disk.\n(Save to LV tdms file format)"
        n547 = Unbundle By Name(w1137) -> ("Pathes.DataPath"=w1133:path, "CaseID"=w1145:string, "IDs.RunID"=w1135:i8, "Ch1Data"=w1144:dbl[][], "Ch2Data"=w1143:dbl[][], "Ch3Data"=w1132:dbl[][], "Ch4Data"=w1125:dbl[][], "V1"=w1127:dbl[], "V2"=w1142:dbl[], "V3"=w1141:dbl[], "V4"=w1124:dbl[])
        n548 = call "FLImDAQ_FGV.vi"() -> ("Read data"=w1130:T5)  [unwired: 10 in, 1 out]
        n549 = Unbundle By Name(w1130) -> ("Waveform to Avg"=w1129:i16)
        n550 = local read "RunStartTime"() -> (w1128:u32)
        n551 = local read "Laser Rep Rate"() -> (w1131:dbl)
        n552 = Increment(x=w1135) -> (x+1=w1134:i8)
        n553 = Bundle By Name(cluster=w1126, "DataPath"=w1133, "CaseID"=w1145, "RunID"=w1134, "Ch1Data"=w1144, "Ch2Data"=w1143, "Ch3Data"=w1132, "Ch4Data"=w1125, "V1"=w1127, "V2"=w1142, "V3"=w1141, "V4"=w1124, "LaserRepRate"=w1131, "WFAverage"=w1129, "RunStartTime"=w1128) -> (w1140:T39)
        n554 = call "SaveRunData(SubVI).vi"("Data cluster"=w1140, "error in (no error)"=w1139) -> ("error out"=w1136:errorcluster)  [unwired: 13 in]
        n555 = flat-sequence {
          tunnel: w1137 -> [w1153]
          tunnel: [w1152] -> w1138
          tunnel: w1136 -> [_]
          frame #0 {
            w1150 = dbl[][] [] ("Ch1Data")
            w1151 = dbl[] [] ("V1")
            # "reset local data"
            n556 = Bundle By Name(cluster=w1153, "Ch1Data"=w1150, "Ch2Data"=w1150, "Ch3Data"=w1150, "Ch4Data"=w1150, "V1"=w1151, "V2"=w1151, "V3"=w1151, "V4"=w1151) -> (w1152:T24)
          }
        }
        n557 = case shown="No Error" w1136 {
          tunnel: ["Run: Increment" "" ("Empty String Constant")] -> w1146
          frame No Error {
          }
          frame Error {
          }
        }
        n558 = call <vilib>:"Add State(s) to Queue__JKI_lib_State_Machine.vi"("State(s) in Front (\"\")"=w1146, "State(s) in (\"\")"=w1149) -> ("States Out"=w1148:string)  [unwired: 13 in]
      }
      frame "Data: Cleanup" {
        # "Cleanup any data and references, here.\n(this is called automatically, by the Macro: Exit)"
        n559 = Unbundle By Name(w1157) -> ("Core.Current VI Reference"=w1160:refnum<vi>)
        n560 = Close Reference(reference=w1160, error in (no error)=w1159) -> (error out=w1158:errorcluster)
        n561 = call <vilib>:"Add State(s) to Queue__JKI_lib_State_Machine.vi"("State(s) in (\"\")"=w1162) -> ("States Out"=w1161:string)  [unwired: 14 in]
      }
      frame "---------- Core ----------" {
        # "Do not put any code in this frame.\n(it is a separator no-op)"
        n562 = call <vilib>:"Add State(s) to Queue__JKI_lib_State_Machine.vi"("State(s) in (\"\")"=w1167) -> ("States Out"=w1166:string)  [unwired: 14 in]
      }
      frame Default {
        w1178 = 42 items=["No error", "Argument error", "Memory is full", "Out of zone", "End of file", "File already open", "Generic file I/O error", "File not found", "File permission error", "Disk is full", "Duplicate path", "Too many files open", "System feature not enabled", "Resource file not found", "Cannot add resource", "Resource not found", "Image not found", "Image memory error", "Pen does not exist", "Config type invalid", "Config token not found", "Config parse error", "Config memory error", "Bad external code format", "Bad external code offset", "External code not present", "Null window", "Destroy window error", "Null menu", "Print aborted", "Bad print record", "Print driver error", "Windows error during printing", "Memory error during printing", "Print dialog error", "Generic print error", "Invalid device refnum", "Device not found", "Device parameter error", "Device unit error", "Cannot open device", "Device call aborted", "Generic error", "Cancelled by user", "Object ID too low", "Object ID too high", "Object not in heap", "Unknown heap", "Unknown object (invalid DefProc)", "Unknown object (DefProc not in table)", "Message out of range", "Invalid (null) method", "Unknown message", "Manager call not supported", "Bad address", "Network operation in progress", "Network operation timed out", "Connection is busy", "Network attribute not supported", "Network error", "Address in use", "System out of memory", "Connection aborted", "Connection refused", "Not connected", "Already connected", "Connection closed", "Initialization error (interapplication manager)", "Bad occurrence", "Wait on unbound occurrence handler", "Occurrence queue overflow", "Datalog type conflict", "Unused", "Unrecognized type (interapplication manager)", "Memory corrupt", "Failed to make temporary DLL", "Old CIN version", "Drag socket not found", "Failed to load drop-object", "Failed to register OLE object", "Failed to release OLE object", "Format specifier type mismatch", "Unknown format specifier", "Too few format specifiers", "Too many format specifiers", "Scan failed", "Newer CIN version", "Error converting to variant", "Runtime menu error", "Password tampered", "Variant attribute not found", "Incompatible variant data type", "Event data is not available", "Event Store is not present", "Occurrence is not found", "Event Queue is not created", "Event info is not available", "Refnum passed is NULL", "Error retrieving Class GUID", "Error retrieving CoClass GUID", "Error retrieving TypeLib GUID.", "Bad built application magic bytes.", "Specific driver is different from the specific driver associated with the Logical Name.", "There is no session opened to the class driver.", "Max Error", "MAX - Error with config objects", "MAX - Error loading configuration", "MAX - Group not supported"]
        # "Current State"
        # "Do not delete, rename, or modify this frame.\n(this is used to capture unhandled states and typos)"
        # "Handle mistyped state name (developer tool)"
        n563 = Format Into String(format string="Software Exception: Unhandled State \"%s\"." ("message"), error in=w1174, w1169) -> (resulting string=w1177:string, error out=w1176:errorcluster)  [unwired: 1 in]
        n564 = call <vilib>:"Error Cluster From Error Code.vi"("show call chain? (False)"=TRUE, "error in (no error)"=w1176, "error message (\"\")"=w1177, "error code (0)"=w1178) -> ("error out"=w1175:errorcluster)  [unwired: 5 in]
        n565 = call <vilib>:"Add State(s) to Queue__JKI_lib_State_Machine.vi"("State(s) in (\"\")"=w1173) -> ("States Out"=w1172:string)  [unwired: 14 in]
      }
      frame "Initialize Core Data" {
        # "Build default path based on the location of project"
        # "Do not delete, rename, or modify this frame.\n(this is used to determine panel behavior on exit)"
        # "originally closed?"
        # "exe?"
        # "If panel starts closed or is an EXE, then close it when we exit"
        n566 = call <vilib>:"Application Directory.vi"() -> ("Application Directory"=w1181:path)
        n567 = property on="Property Node" class="App"() -> ("App.Kind"=w1197:T19)  [unwired: 2 in, 2 out]
        n568 = property on="Property Node" class="VI"() -> ("FP.State"=w1191:T18)  [unwired: 2 in, 2 out]
        n569 = control-ref of="Current VI Reference"() -> (w1192:refnum<vi>)
        n570 = Equal?(x=w1191, y=T18."Closed" ("Front Panel Window:State")) -> (x = y?=w1189:bool)
        n571 = Strip Path(path=w1181) -> (stripped path=w1180:path)  [unwired: 1 out]
        n572 = Equal?(x=w1197, y=T19."Run Time System" ("Application:Kind")) -> (x = y?=w1195:bool)
        n573 = Build Path(base path=w1180, name or relative path="Data") -> (appended path=w1187:path)
        n574 = Build Path(base path=w1181, name or relative path="SystemTemp") -> (appended path=w1184:path)
        n575 = Build Path(base path=w1181, name or relative path="SystemCalibrationFile") -> (appended path=w1182:path)
        n576 = Or(x=w1189, y=w1195) -> (x .or. y?=w1193:bool)
        n577 = Bundle By Name(cluster=w1194, "Core.Current VI Reference"=w1192, "Core.Close Panel on Exit?"=w1193, "DefaultPath"=w1187, "TempPath"=w1184, "CaliPath"=w1182) -> (w1199:T24)
        n578 = call <vilib>:"Add State(s) to Queue__JKI_lib_State_Machine.vi"("State(s) in (\"\")"=w1201) -> ("States Out"=w1200:string)  [unwired: 14 in]
      }
      frame "Error Handler" {
        # "Unhandled Error -- Display it"
        # "Handle any errors here.\nYou can also output any states to clean-up after errors occur"
        # "Clear error"
        n579 = Unbundle By Name(w1202) -> ("code"=w1204:i32)
        n580 = case shown="Default" w1204 {
          tunnel: ["Macro: Exit" w1214 w1220] -> w1203
          tunnel: w1202 -> [w1210 _ _]
          frame Default {
            w1212 = T40 1 items=["no dialog", "OK message", "continue or stop message", "OK message + warnings", "continue/stop + warnings"] ("type of dialog (OK msg:1)")
            n581 = call <vilib>:"General Error Handler.vi"("type of dialog (OK msg:1)"=w1212, "error in (no error)"=w1210) -> ()  [unwired: 9 in, 5 out]
          }
          frame 5002 {
            n582 = Two Button Dialog(message="Laser interlock open! Please close interlock and try again! ", 1:"Safely Shutdown" ("F button name (\"Cancel\")"), 2:"OK" ("T button name (\"OK\")")) -> (T button?=w1215:bool)
            n583 = case shown="True" w1215 {
              tunnel: ["Macro: Exit" "355 Laser: CheckControllerStatus"] -> w1214
              frame False {
              }
              frame True {
              }
            }
          }
          frame 5001 {
            n584 = Two Button Dialog(message="Unable to connect to imaging computer, do you want to run data aquisiton alone? ", 1:"No" ("F button name (\"Cancel\")"), 2:"Yes" ("T button name (\"OK\")")) -> (T button?=w1221:bool)
            n585 = case shown="False" w1221 {
              tunnel: ["Macro: Exit" "" ("Empty String Constant")] -> w1220
              frame False {
              }
              frame True {
              }
            }
          }
        }
        n586 = call <vilib>:"Add State(s) to Queue__JKI_lib_State_Machine.vi"("State(s) in Front (\"\")"=w1203, "State(s) in (\"\")"=w1209) -> ("States Out"=w1208:string)  [unwired: 13 in]
      }
      frame "Exit" {
        # "Do not put any code in this frame.\n(No errors that occur here will be handled.)"
        n587 = call <vilib>:"Add State(s) to Queue__JKI_lib_State_Machine.vi"("State(s) in (\"\")"=w1232) -> ("States Out"=w1231:string)  [unwired: 14 in]
      }
      frame "---------- Case ----------" {
        # "Template Separator\n(You can make a copy of, or modify, this frame)"
        n588 = call <vilib>:"Add State(s) to Queue__JKI_lib_State_Machine.vi"("State(s) in (\"\")"=w1237) -> ("States Out"=w1236:string)  [unwired: 14 in]
      }
      frame "Case: getCaliID" {
        # "Get Calibration file #\n(You can make a copy of, or modify, this frame)"
        n589 = Unbundle By Name(w1238) -> ("Pathes.CaliPath"=w1241:path)
        n590 = call <vilib>:"Recursive File List.vi"("pattern"="*.tdms", "Treat LLBs as Folders?"=FALSE, "Folder Path"=w1241) -> ("All Files in Dir"=w1246:path[])  [unwired: 4 in, 4 out]
        n591 = for {
          tunnel: w1246 -> [w1256] mode=indexing
          tunnel: [w1255] -> w1245 mode=indexing
          tunnel: "Calibration" -> [w1252]
          n592 = Strip Path(path=w1256) -> (name=w1253:string)  [unwired: 1 out]
          n593 = Search and Replace String(input string=w1253, search string=w1252) -> (result string=w1251:string)  [unwired: 6 in, 3 out]
          n594 = Scan From String(format string="%d" ("string"), input string=w1251) -> (output 1=w1255:i32)  [unwired: 3 in, 3 out]
        }
        n595 = Array Max & Min(array=w1245) -> (max value=w1244:i32)  [unwired: 3 out]
        n596 = Bundle By Name(cluster=w1238, "IDs.Cali ID"=w1244) -> (w1239:T24)
        n597 = call <vilib>:"Add State(s) to Queue__JKI_lib_State_Machine.vi"("State(s) in (\"\")"=w1250) -> ("States Out"=w1249:string)  [unwired: 14 in]
      }
      frame "Case: getBGID" {
        # "Get background #\n(You can make a copy of, or modify, this frame)"
        n598 = Unbundle By Name(w1259) -> ("Pathes.BG Path"=w1264:path)
        n599 = call <vilib>:"Recursive File List.vi"("pattern"="*.tdms", "Treat LLBs as Folders?"=FALSE, "Folder Path"=w1264) -> ("All Files in Dir"=w1262:path[])  [unwired: 4 in, 4 out]
        n600 = for {
          tunnel: w1262 -> [w1279] mode=indexing
          tunnel: "Background" ("name or relative path") -> [w1277]
          shift-right: [w1270] -> w1257
          shift-left: 0 -> [w1274]
          n601 = Strip Path(path=w1279) -> (name=w1278:string)  [unwired: 1 out]
          n602 = Search and Replace String(input string=w1278, search string=w1277) -> (number of replacements=w1276:i32)  [unwired: 6 in, 3 out]
          n603 = Greater Than 0?(x=w1276) -> (x > 0?=w1275:bool)
          n604 = Select(t=1, s=w1275, f=0) -> (s? t:f=w1273:i32)
          n605 = Add(x=w1273, y=w1274) -> (x+y=w1270:i32)
        }
        n606 = Bundle By Name(cluster=w1259, "IDs.BG ID"=w1257) -> (w1260:T24)
        n607 = call <vilib>:"Add State(s) to Queue__JKI_lib_State_Machine.vi"("State(s) in (\"\")"=w1269) -> ("States Out"=w1268:string)  [unwired: 14 in]
      }
      frame "Case: getRunID" {
        # "Check folder for run ID\n(You can make a copy of, or modify, this frame)"
        n608 = Unbundle By Name(w1289) -> ("Pathes.DataPath"=w1288:path, "CaseID"=w1284:string)
        n609 = Build Array("Background" ("name or relative path"), "Calibration", "3DScanData" ("element")) -> (w1294:string[])
        n610 = call <vilib>:"Recursive File List.vi"("Folders to Exclude"=w1294, "pattern"="*.tdms", "Treat LLBs as Folders?"=FALSE, "Folder Path"=w1288) -> ("All Files in Dir"=w1285:path[])  [unwired: 3 in, 4 out]
        n611 = for {
          tunnel: w1285 -> [w1303] mode=indexing
          tunnel: [w1302] -> w1291 mode=indexing
          tunnel: w1284 -> [w1299]
          n612 = Strip Path(path=w1303) -> (name=w1300:string)  [unwired: 1 out]
          n613 = Search and Replace String(input string=w1300, search string=w1299) -> (result string=w1298:string)  [unwired: 6 in, 3 out]
          n614 = Scan From String(format string="_%d" ("string"), input string=w1298) -> (output 1=w1302:i32)  [unwired: 3 in, 3 out]
        }
        n615 = Array Max & Min(array=w1291) -> (max value=w1282:i32)  [unwired: 3 out]
        n616 = Bundle By Name(cluster=w1289, "IDs.RunID"=w1282) -> (w1290:T24)
        n617 = call "RunIDFGV.vi"("Error In"=w1280, "RunID in"=w1282) -> ("Error Out"=w1281:errorcluster)  [unwired: 8 in, 1 out]
        n618 = call <vilib>:"Add State(s) to Queue__JKI_lib_State_Machine.vi"("State(s) in (\"\")"=w1297) -> ("States Out"=w1296:string)  [unwired: 14 in]
      }
      frame "Case: CreatFileStruct" {
        # "Creat case file structure"
        n619 = Unbundle By Name(w1317) -> ("DefaultPath"=w1323:path, "CaseID"=w1310:string)
        n620 = Build Path(base path=w1323, name or relative path=w1310) -> (appended path=w1322:path)
        n621 = call <vilib>:"Check if File or Folder Exists.vi"("error in (no error)"=w1316, "path"=w1322) -> ("error out"=w1319:errorcluster, "file or folder exists?"=w1321:bool, "dup path"=w1320:path)  [unwired: 7 in]
        n622 = case shown="True" w1321 {
          tunnel: w1320 -> [w1340 w1348]
          tunnel: w1319 -> [w1338 w1343]
          tunnel: [w1332 w1348] -> w1308
          tunnel: [w1336 w1350] -> w1307
          tunnel: [u32 0 u32 0] -> w1306
          tunnel: [w1334 w1353] -> w1314
          tunnel: "Background" ("name or relative path") -> [w1333 w1345]
          tunnel: "Calibration" -> [w1331 w1344]
          tunnel: [w1327 w1346] -> w1311
          tunnel: w1310 -> [_ _]
          tunnel: ["" ("Empty String Constant") "Case: getRunID\nCase: getBGID\nCase: getCaliID\nUI: Update"] -> w1309
          frame False {
            # "Folder not exist. Creat folders."
            n623 = Create Folder(path (use dialog)=w1340, error in=w1338) -> (created path=w1332:path, error out=w1329:errorcluster)  [unwired: 1 in, 1 out]
            n624 = Build Path(base path=w1332, name or relative path=w1331) -> (appended path=w1330:path)
            n625 = Build Path(base path=w1332, name or relative path=w1333) -> (appended path=w1339:path)
            n626 = Create Folder(path (use dialog)=w1339, error in=w1329) -> (created path=w1334:path, error out=w1335:errorcluster)  [unwired: 1 in, 1 out]
            n627 = Create Folder(path (use dialog)=w1330, error in=w1329) -> (created path=w1327:path, error out=w1328:errorcluster)  [unwired: 1 in, 1 out]
            n628 = Merge Errors(w1335, w1328) -> (w1336:errorcluster)
          }
          frame True {
            # "Folder exsit, check file #"
            n629 = Build Path(base path=w1348, name or relative path=w1344) -> (appended path=w1349:path)
            n630 = Build Path(base path=w1348, name or relative path=w1345) -> (appended path=w1354:path)
            n631 = call <vilib>:"Check if File or Folder Exists.vi"("path"=w1349) -> ("file or folder exists?"=w1347:bool, "dup path"=w1346:path)  [unwired: 8 in, 1 out]
            n632 = call <vilib>:"Check if File or Folder Exists.vi"("path"=w1354) -> ("file or folder exists?"=w1352:bool, "dup path"=w1353:path)  [unwired: 8 in, 1 out]
            n633 = And(x=w1352, y=w1347) -> (x .and. y?=w1351:bool)
            n634 = case shown="False" w1351 {
              tunnel: w1343 -> [_ w1356]
              tunnel: [errorcluster {"status"=TRUE, "code"=5003, "source"="File structure error."} ("error out") w1356] -> w1350
              frame False {
              }
              frame True {
              }
            }
          }
        }
        n635 = Bundle By Name(cluster=w1317, "Pathes.DataPath"=w1308, "Pathes.BG Path"=w1314, "Pathes.CaliPath"=w1311, "IDs.RunID"=w1306, "IDs.BG ID"=w1306, "IDs.Cali ID"=w1306) -> (w1318:T24)
        n636 = call "DataRootPathFGV.vi"("Error In"=w1307, "PathIn"=w1308) -> ("Error Out"=w1305:errorcluster)  [unwired: 8 in, 1 out]
        n637 = call "RunIDFGV.vi"("Error In"=w1305, "RunID in"=w1306) -> ("Error Out"=w1304:errorcluster)  [unwired: 8 in, 1 out]
        n638 = call <vilib>:"Add State(s) to Queue__JKI_lib_State_Machine.vi"("State(s) in Front (\"\")"=w1309, "State(s) in (\"\")"=w1325) -> ("States Out"=w1324:string)  [unwired: 13 in]
      }
      frame "Case: GetID" {
        # "Template Separator\n(You can make a copy of, or modify, this frame)"
        n639 = call "set_subjectID.vi"() -> ("subject_id"=w1357:string)  [unwired: 10 in]
        n640 = Bundle By Name(cluster=w1359, "CaseID"=w1357) -> (w1360:T24)
        n641 = call <vilib>:"Add State(s) to Queue__JKI_lib_State_Machine.vi"("State(s) in (\"\")"=w1363) -> ("States Out"=w1362:string)  [unwired: 14 in]
      }
      frame "---------- DeconEngine ----------" {
        # "start data aquisition and then set irfAligh to ture and decon channel to 1,2 and 3."
        # "Template Separator\n(You can make a copy of, or modify, this frame)"
        n642 = call <vilib>:"Add State(s) to Queue__JKI_lib_State_Machine.vi"("State(s) in (\"\")"=w1368) -> ("States Out"=w1367:string)  [unwired: 14 in]
      }
      frame "DeconEngine: InitDotNet" {
        # "Initialize Dot Net Decon and save the FGV"
        # "Initilize Dot Net \n(You can make a copy of, or modify, this frame)"
        n643 = constructor on="Constructor Node" class="LaguerreDeconRT"(error in=w1371) -> (reference out=w1369:refnum<k24>, error out=w1372:errorcluster)  [unwired: 2 in, 1 out]
        n644 = call "DotNetFGV.vi"("Error In"=w1372, "Operation (Read)"=enum16{"Read", "Write"}."Write", "reference in"=w1369) -> ("Error Out"=w1370:errorcluster)  [unwired: 7 in, 1 out]
        n645 = case shown="No Error" w1370 {
          frame No Error {
            ".NetInitialized?" <- TRUE (".NetInitialized?")
          }
          frame Error {
          }
        }
        n646 = call <vilib>:"Add State(s) to Queue__JKI_lib_State_Machine.vi"("State(s) in (\"\")"=w1377) -> ("States Out"=w1376:string)  [unwired: 14 in]
      }
      frame "DeconEngine: Warmup" {
        # "Warm up parpool\n(You can make a copy of, or modify, this frame)"
        n647 = call "DotNetFGV.vi"("Error In"=w1383) -> ("Error Out"=w1384:errorcluster, "reference out"=w1385:refnum<k24>)  [unwired: 9 in]
        n648 = flat-sequence {
          tunnel: w1383 -> [_]
          tunnel: [w1391] -> w1380
          frame #0 {
            n649 = Tick Count (ms)() -> (millisecond timer value=w1391:u32)
          }
        }
        n650 = invoke class="LaguerreDeconRT" method="init_parpool"(reference=w1385, error in=w1384) -> (error out=w1382:errorcluster)  [unwired: 1 in, 2 out]
        n651 = flat-sequence {
          tunnel: w1382 -> [_]
          tunnel: [w1390] -> w1381
          frame #0 {
            n652 = Tick Count (ms)() -> (millisecond timer value=w1390:u32)
          }
        }
        n653 = Subtract(x=w1381, y=w1380) -> (x-y=→"WarmupTime(ms)":u32)
        n654 = call <vilib>:"Add State(s) to Queue__JKI_lib_State_Machine.vi"("State(s) in (\"\")"=w1389) -> ("States Out"=w1388:string)  [unwired: 14 in]
      }
      frame "DeconEngine: loadIRF" {
        # "Load IRF for decon and save to FGV\n(You can make a copy of, or modify, this frame)"
        n655 = Current VI's Path() -> (path=w1409:path)
        n656 = Strip Path(path=w1409) -> (stripped path=w1408:path)  [unwired: 1 out]
        n657 = Build Path(base path=w1408, name or relative path="DotNetDecon") -> (appended path=w1396:path)
        n658 = Build Path(base path=w1396, name or relative path="Channel1.tdms") -> (appended path=w1413:path)
        n659 = Build Path(base path=w1396, name or relative path="Channel3.tdms") -> (appended path=w1398:path)
        n660 = Build Path(base path=w1396, name or relative path="Channel2.tdms") -> (appended path=w1399:path)
        n661 = call "LoadIRF.vi"("error in (no error)"=w1397, "file path"=w1413) -> ("error out"=w1411:errorcluster, "APD"=w1412:T41)  [unwired: 8 in]
        n662 = call "LoadIRF.vi"("error in (no error)"=w1397, "file path"=w1399) -> ("error out"=w1404:errorcluster, "APD"=w1405:T41)  [unwired: 8 in]
        n663 = call "LoadIRF.vi"("error in (no error)"=w1397, "file path"=w1398) -> ("error out"=w1401:errorcluster, "APD"=w1402:T41)  [unwired: 8 in]
        n664 = call "DeConAPD1FGV.vi"("Error In"=w1411, "Operation (Read)"=enum16{"Read", "Write"}."Write", "APDClass in"=w1412) -> ("Error Out"=w1395:errorcluster)  [unwired: 7 in, 1 out]
        n665 = call "DeConAPD2FGV.vi"("Error In"=w1404, "Operation (Read)"=enum16{"Read", "Write"}."Write", "APDClass in"=w1405) -> ("Error Out"=w1394:errorcluster)  [unwired: 7 in, 1 out]
        n666 = call "DeConAPD3FGV.vi"("Error In"=w1401, "Operation (Read)"=enum16{"Read", "Write"}."Write", "APDClass in"=w1402) -> ("Error Out"=w1393:errorcluster)  [unwired: 7 in, 1 out]
        n667 = Merge Errors(w1395, w1394, w1393) -> (w1392:errorcluster)
        n668 = call <vilib>:"Add State(s) to Queue__JKI_lib_State_Machine.vi"("State(s) in (\"\")"=w1419) -> ("States Out"=w1418:string)  [unwired: 14 in]
      }
      frame "DeconEngine: CloseNetRef" {
        # "Template Separator\n(You can make a copy of, or modify, this frame)"
        n669 = call "DotNetFGV.vi"("Error In"=w1420) -> ("Error Out"=w1422:errorcluster, "reference out"=w1423:refnum<k24>)  [unwired: 9 in]
        n670 = Close Reference(reference=w1423, error in (no error)=w1422) -> (error out=w1421:errorcluster)
        n671 = call <vilib>:"Add State(s) to Queue__JKI_lib_State_Machine.vi"("State(s) in (\"\")"=w1427) -> ("States Out"=w1426:string)  [unwired: 14 in]
      }
      frame "DeconEngine: InitilizeMacro" {
        # "start data aquisition and then set irfAligh to ture and decon channel to 1,2 and 3."
        # "Initilize Decon Engine for all channel\n(You can make a copy of, or modify, this frame)"
        n672 = call <vilib>:"Add State(s) to Queue__JKI_lib_State_Machine.vi"("State(s) in Front (\"\")"="DeconEngine: InitializeCh1\nDeconEngine: InitializeCh2\nDeconEngine: InitializeCh3\nDeconEngine: InitializeCh4" ("State(s) in Front (\"\")"), "State(s) in (\"\")"=w1433) -> ("States Out"=w1432:string)  [unwired: 13 in]
      }
      frame "DeconEngine: InitializeCh1" {
        w1455 = refnum<class "LaguerreDeconEngineClass.lvclass"> refnum  # Ch1DeconObj
        # "Initilize Laguerre Deconvolution engine Object\n(You can make a copy of, or modify, this frame)"
        n673 = global read "GlobalVariables.vi" "LastUseiRF"() -> (w1436:T17)
        n674 = call "setLaguerreOrder.vi"("error in (no error)"=w1443, "LaguerreOrder"=u32 12, "LaguerreDeconClass in"=w1455) -> ("error out"=w1452:errorcluster, "LaguerreDeconClass out"=w1453:refnum<class "LaguerreDeconEngineClass.lvclass">)  [unwired: 7 in]
        n675 = Unbundle By Name(w1436) -> ("Ch1 iRF"=w1435:dbl[])
        n676 = call "setDataLength.vi"("error in (no error)"=w1452, "dataLength"=u32 600, "LaguerreDeconClass in"=w1453) -> ("error out"=w1451:errorcluster, "LaguerreDeconClass out"=w1450:refnum<class "LaguerreDeconEngineClass.lvclass">)  [unwired: 7 in]
        n677 = call "setIRF.vi"("error in (no error)"=w1451, "iRF"=w1435, "LaguerreDeconClass in"=w1450) -> ("error out"=w1448:errorcluster, "LaguerreDeconClass out"=w1449:refnum<class "LaguerreDeconEngineClass.lvclass">)  [unwired: 7 in]
        n678 = call "computeAlpha.vi"("error in (no error)"=w1448, "LaguerreDeconClass in"=w1449) -> ("error out"=w1446:errorcluster, "LaguerreDeconClass out"=w1447:refnum<class "LaguerreDeconEngineClass.lvclass">)  [unwired: 8 in]
        n679 = call "dataInitilize.vi"("error in (no error)"=w1446, "LaguerreDeconClass in"=w1447) -> ("error out"=w1444:errorcluster, "LaguerreDeconClass out"=w1445:refnum<class "LaguerreDeconEngineClass.lvclass">)  [unwired: 8 in]
        n680 = call "computeDeconMatrix.vi"("error in (no error)"=w1444, "LaguerreDeconClass in"=w1445) -> ("error out"=w1440:errorcluster, "LaguerreDeconClass out"=w1442:refnum<class "LaguerreDeconEngineClass.lvclass">)  [unwired: 8 in]
        n681 = call "Ch1DeconEngineFGV.vi"("Error In"=w1440, "action(read)"=enum16{"write", "read"}."write" ("action"), "Ch1DeconEngine in"=w1442) -> ("Error Out"=w1439:errorcluster)  [unwired: 7 in, 1 out]
        n682 = call <vilib>:"Add State(s) to Queue__JKI_lib_State_Machine.vi"("State(s) in (\"\")"=w1457) -> ("States Out"=w1456:string)  [unwired: 14 in]
      }
      frame "DeconEngine: InitializeCh2" {
        w1479 = refnum<class "LaguerreDeconEngineClass.lvclass"> refnum  # Ch2DeconObj
        # "Initilize Laguerre Deconvolution engine Object\n(You can make a copy of, or modify, this frame)"
        n683 = global read "GlobalVariables.vi" "LastUseiRF"() -> (w1460:T17)
        n684 = call "setLaguerreOrder.vi"("error in (no error)"=w1467, "LaguerreOrder"=u32 12, "LaguerreDeconClass in"=w1479) -> ("error out"=w1476:errorcluster, "LaguerreDeconClass out"=w1477:refnum<class "LaguerreDeconEngineClass.lvclass">)  [unwired: 7 in]
        n685 = Unbundle By Name(w1460) -> ("Ch2 iRF"=w1459:dbl[])
        n686 = call "setDataLength.vi"("error in (no error)"=w1476, "dataLength"=u32 600, "LaguerreDeconClass in"=w1477) -> ("error out"=w1475:errorcluster, "LaguerreDeconClass out"=w1474:refnum<class "LaguerreDeconEngineClass.lvclass">)  [unwired: 7 in]
        n687 = call "setIRF.vi"("error in (no error)"=w1475, "iRF"=w1459, "LaguerreDeconClass in"=w1474) -> ("error out"=w1472:errorcluster, "LaguerreDeconClass out"=w1473:refnum<class "LaguerreDeconEngineClass.lvclass">)  [unwired: 7 in]
        n688 = call "computeAlpha.vi"("error in (no error)"=w1472, "LaguerreDeconClass in"=w1473) -> ("error out"=w1470:errorcluster, "LaguerreDeconClass out"=w1471:refnum<class "LaguerreDeconEngineClass.lvclass">)  [unwired: 8 in]
        n689 = call "dataInitilize.vi"("error in (no error)"=w1470, "LaguerreDeconClass in"=w1471) -> ("error out"=w1468:errorcluster, "LaguerreDeconClass out"=w1469:refnum<class "LaguerreDeconEngineClass.lvclass">)  [unwired: 8 in]
        n690 = call "computeDeconMatrix.vi"("error in (no error)"=w1468, "LaguerreDeconClass in"=w1469) -> ("error out"=w1464:errorcluster, "LaguerreDeconClass out"=w1466:refnum<class "LaguerreDeconEngineClass.lvclass">)  [unwired: 8 in]
        n691 = call "Ch2DeconEngineFGV.vi"("Error In"=w1464, "action(read)"=enum16{"write", "read"}."write" ("action"), "Ch2DeconEngine in"=w1466) -> ("Error Out"=w1463:errorcluster)  [unwired: 7 in, 1 out]
        n692 = call <vilib>:"Add State(s) to Queue__JKI_lib_State_Machine.vi"("State(s) in (\"\")"=w1481) -> ("States Out"=w1480:string)  [unwired: 14 in]
      }
      frame "DeconEngine: InitializeCh3" {
        w1483 = refnum<class "LaguerreDeconEngineClass.lvclass"> refnum  # Ch3DeconObj
        # "Initilize Laguerre Deconvolution engine Object\n(You can make a copy of, or modify, this frame)"
        n693 = global read "GlobalVariables.vi" "LastUseiRF"() -> (w1485:T17)
        n694 = call "setLaguerreOrder.vi"("error in (no error)"=w1492, "LaguerreOrder"=u32 12, "LaguerreDeconClass in"=w1483) -> ("error out"=w1501:errorcluster, "LaguerreDeconClass out"=w1502:refnum<class "LaguerreDeconEngineClass.lvclass">)  [unwired: 7 in]
        n695 = Unbundle By Name(w1485) -> ("Ch3 iRF"=w1484:dbl[])
        n696 = call "setDataLength.vi"("error in (no error)"=w1501, "dataLength"=600, "LaguerreDeconClass in"=w1502) -> ("error out"=w1500:errorcluster, "LaguerreDeconClass out"=w1499:refnum<class "LaguerreDeconEngineClass.lvclass">)  [unwired: 7 in]
        n697 = call "setIRF.vi"("error in (no error)"=w1500, "iRF"=w1484, "LaguerreDeconClass in"=w1499) -> ("error out"=w1497:errorcluster, "LaguerreDeconClass out"=w1498:refnum<class "LaguerreDeconEngineClass.lvclass">)  [unwired: 7 in]
        n698 = call "computeAlpha.vi"("error in (no error)"=w1497, "LaguerreDeconClass in"=w1498) -> ("error out"=w1495:errorcluster, "LaguerreDeconClass out"=w1496:refnum<class "LaguerreDeconEngineClass.lvclass">)  [unwired: 8 in]
        n699 = call "dataInitilize.vi"("error in (no error)"=w1495, "LaguerreDeconClass in"=w1496) -> ("error out"=w1493:errorcluster, "LaguerreDeconClass out"=w1494:refnum<class "LaguerreDeconEngineClass.lvclass">)  [unwired: 8 in]
        n700 = call "computeDeconMatrix.vi"("error in (no error)"=w1493, "LaguerreDeconClass in"=w1494) -> ("error out"=w1489:errorcluster, "LaguerreDeconClass out"=w1491:refnum<class "LaguerreDeconEngineClass.lvclass">)  [unwired: 8 in]
        n701 = call "Ch3DeconEngineFGV.vi"("Error In"=w1489, "action(read)"=enum16{"write", "read"}."write" ("action"), "Ch3DeconEngine in"=w1491) -> ("Error Out"=w1488:errorcluster)  [unwired: 7 in, 1 out]
        n702 = call <vilib>:"Add State(s) to Queue__JKI_lib_State_Machine.vi"("State(s) in (\"\")"=w1505) -> ("States Out"=w1504:string)  [unwired: 14 in]
      }
      frame "DeconEngine: InitializeCh4" {
        w1507 = refnum<class "LaguerreDeconEngineClass.lvclass"> refnum  # Ch3DeconObj
        # "Initilize Laguerre Deconvolution engine Object\n(You can make a copy of, or modify, this frame)"
        n703 = global read "GlobalVariables.vi" "LastUseiRF"() -> (w1509:T17)
        n704 = call "setLaguerreOrder.vi"("error in (no error)"=w1516, "LaguerreOrder"=u32 12, "LaguerreDeconClass in"=w1507) -> ("error out"=w1525:errorcluster, "LaguerreDeconClass out"=w1526:refnum<class "LaguerreDeconEngineClass.lvclass">)  [unwired: 7 in]
        n705 = Unbundle By Name(w1509) -> ("Ch4 iRF"=w1508:dbl[])
        n706 = call "setDataLength.vi"("error in (no error)"=w1525, "dataLength"=u32 600, "LaguerreDeconClass in"=w1526) -> ("error out"=w1524:errorcluster, "LaguerreDeconClass out"=w1523:refnum<class "LaguerreDeconEngineClass.lvclass">)  [unwired: 7 in]
        n707 = call "setIRF.vi"("error in (no error)"=w1524, "iRF"=w1508, "LaguerreDeconClass in"=w1523) -> ("error out"=w1521:errorcluster, "LaguerreDeconClass out"=w1522:refnum<class "LaguerreDeconEngineClass.lvclass">)  [unwired: 7 in]
        n708 = call "computeAlpha.vi"("error in (no error)"=w1521, "LaguerreDeconClass in"=w1522) -> ("error out"=w1519:errorcluster, "LaguerreDeconClass out"=w1520:refnum<class "LaguerreDeconEngineClass.lvclass">)  [unwired: 8 in]
        n709 = call "dataInitilize.vi"("error in (no error)"=w1519, "LaguerreDeconClass in"=w1520) -> ("error out"=w1517:errorcluster, "LaguerreDeconClass out"=w1518:refnum<class "LaguerreDeconEngineClass.lvclass">)  [unwired: 8 in]
        n710 = call "computeDeconMatrix.vi"("error in (no error)"=w1517, "LaguerreDeconClass in"=w1518) -> ("error out"=w1513:errorcluster, "LaguerreDeconClass out"=w1515:refnum<class "LaguerreDeconEngineClass.lvclass">)  [unwired: 8 in]
        n711 = call "Ch4DeconEngineFGV.vi"("Error In"=w1513, "action(read)"=enum16{"write", "read"}."write" ("action"), "Ch3DeconEngine in"=w1515) -> ("Error Out"=w1512:errorcluster)  [unwired: 7 in, 1 out]
        n712 = call <vilib>:"Add State(s) to Queue__JKI_lib_State_Machine.vi"("State(s) in (\"\")"=w1529) -> ("States Out"=w1528:string)  [unwired: 14 in]
      }
      frame "---------- Digitizer ----------" {
        # "Template Separator\n(You can make a copy of, or modify, this frame)"
        n713 = call <vilib>:"Add State(s) to Queue__JKI_lib_State_Machine.vi"("State(s) in (\"\")"=w1534) -> ("States Out"=w1533:string)  [unwired: 14 in]
      }
      frame "Digitizer: Initialize" {
        # "reset digitizer to everytime the system runs"
        # "reset digitizer to everytime the system runs"
        # "Initialize digitizer.\nInitialize both digitizer and update status."
        n714 = call "FLImDAQ_FGV.vi"("error in (no error)"=w1542) -> ("error out"=w1536:errorcluster, "Read data"=w1541:T5)  [unwired: 9 in]
        n715 = Unbundle By Name(w1544) -> ("SysConfigCluster.Ch1Enable?"=w1549:bool, "SysConfigCluster.Ch2Enable?"=w1548:bool, "SysConfigCluster.Ch3Enable?"=w1546:bool)
        n716 = Unbundle By Name(w1541) -> ("Digitizer 1"=w1537:refnum<k15>, "Digitizer 2"=w1540:refnum<k15>)
        n717 = property on="Digitizer" class="Bool (strict)"("Blinking"=TRUE) -> ()  [unwired: 2 in, 2 out]
        n718 = Or(x=w1549, y=w1548) -> (x .or. y?=w1547:bool)
        n719 = case shown="True" w1547 {
          tunnel: w1536 -> [w1557 w1560]
          tunnel: [w1557 w1559] -> w1538
          tunnel: w1537 -> [_ w1561]
          frame False {
          }
          frame True {
            n720 = call <instrlib>:"niScope Initialize.vi"("resource name"=w1561, "reset device"=TRUE, "error in"=w1560) -> ("error out"=w1559:errorcluster)  [unwired: 11 in, 1 out]
          }
        }
        n721 = case shown="True" w1546 {
          tunnel: w1536 -> [w1552 w1554]
          tunnel: [w1552 w1556] -> w1543
          tunnel: w1540 -> [_ w1555]
          frame False {
          }
          frame True {
            n722 = call <instrlib>:"niScope Initialize.vi"("resource name"=w1555, "reset device"=TRUE, "error in"=w1554) -> ("error out"=w1556:errorcluster)  [unwired: 11 in, 1 out]
          }
        }
        n723 = Merge Errors(w1538, w1543) -> (w1535:errorcluster)
        n724 = call <vilib>:"Add State(s) to Queue__JKI_lib_State_Machine.vi"("State(s) in (\"\")"=w1551) -> ("States Out"=w1550:string)  [unwired: 14 in]
      }
      frame "Digitizer: Config" {
        # "Synchronize is taking time ~3s."
        # "Config  digitizer\nCall subVi to config digitizer"
        n725 = call "FLImDAQ_FGV.vi"() -> ("Read data"=w1579:T5)  [unwired: 10 in, 1 out]
        n726 = Unbundle By Name(w1588) -> ("SysConfigCluster.Ch1Enable?"=w1596:bool, "SysConfigCluster.Ch2Enable?"=w1595:bool, "SysConfigCluster.Ch3Enable?"=w1593:bool, "FLImDAQ"=w1590:T31)
        n727 = Unbundle By Name(w1579) -> ("Digitizer 1"=w1582:refnum<k15>, "Digitizer 2"=w1581:refnum<k15>)
        n728 = property on="Digitizer" class="Bool (strict)"(error in=w1583, "Blinking"=TRUE) -> (error out=w1584:errorcluster)  [unwired: 1 in, 1 out]
        n729 = Or(x=w1596, y=w1595) -> (x .or. y?=w1594:bool)
        n730 = case shown="True" w1594 {
          tunnel: w1590 -> [_ w1609]
          tunnel: w1584 -> [w1605 w1608]
          tunnel: [w1605 w1607] -> w1591
          tunnel: w1582 -> [_ w1606]
          frame False {
          }
          frame True {
            n731 = call "DigitizerConfig.vi"("error in (no error)"=w1608, "FLImDAQ"=w1609, "IVI Refnum in"=w1606) -> ("error out"=w1607:errorcluster)  [unwired: 7 in, 1 out]
          }
        }
        n732 = case shown="True" w1593 {
          tunnel: w1590 -> [_ w1604]
          tunnel: w1591 -> [w1599 w1603]
          tunnel: [w1599 w1602] -> w1567
          tunnel: w1581 -> [_ w1600]
          frame False {
          }
          frame True {
            n733 = call "DigitizerConfig.vi"("Config Trigger? (T)"=FALSE ("Config Trigge(T)r:"), "error in (no error)"=w1603, "FLImDAQ"=w1604, "IVI Refnum in"=w1600) -> ("error out"=w1602:errorcluster)  [unwired: 6 in, 1 out]
          }
        }
        n734 = call "Digitizer1_FGV.vi"("error in (no error)"=w1567) -> ("error out"=w1577:errorcluster, "Read data"=w1578:refnum<k15>)  [unwired: 9 in]
        n735 = call <instrlib>:"niScope Get Session Reference.vi"("instrument handle"=w1578, "error in"=w1577) -> ("session reference"=w1571:refnum<k20>, "error out"=w1569:errorcluster)  [unwired: 11 in, 1 out]
        n736 = call "Digitizer2_FGV.vi"("error in (no error)"=w1569) -> ("error out"=w1575:errorcluster, "Read data"=w1576:refnum<k15>)  [unwired: 9 in]
        n737 = call <instrlib>:"niScope Get Session Reference.vi"("instrument handle"=w1576, "error in"=w1575) -> ("session reference"=w1570:refnum<k20>, "error out"=w1568:errorcluster)  [unwired: 11 in, 1 out]
        n738 = Build Array(w1571, w1570) -> (w1574:refnum<k20>[])
        n739 = call <instrlib>:"niTClk Configure For Homogeneous Triggers.vi"("error in (no error)"=w1568, "sessions"=w1574) -> ("error out"=w1573:errorcluster, "sessions out"=w1572:refnum<k20>[])  [unwired: 8 in]
        n740 = call <instrlib>:"niTClk Synchronize.vi"("error in (no error)"=w1573, "sessions"=w1572) -> ("error out"=w1566:errorcluster, "sessions out"=w1564:refnum<k20>[])  [unwired: 8 in]
        n741 = call <userlib>:"Wait (ms)__ogtk.vi"("error in (no error)"=w1566, "milliseconds to wait"=u32 1500) -> ("error out"=w1562:errorcluster)  [unwired: 8 in, 1 out]
        n742 = Unbundle By Name(w1562) -> ("status"=w1587:bool)
        n743 = Not(x=w1587) -> (.not. x?=w1586:bool)
        n744 = Bundle By Name(cluster=w1588, "System Status.Digitizer"=w1586, "niTClk sessions"=w1564) -> (w1589:T24)
        n745 = property on="Digitizer" class="Bool (strict)"(error in=w1562, "Blinking"=FALSE) -> (error out=w1580:errorcluster)  [unwired: 1 in, 1 out]
        n746 = call <vilib>:"Add State(s) to Queue__JKI_lib_State_Machine.vi"("State(s) in (\"\")"=w1598) -> ("States Out"=w1597:string)  [unwired: 14 in]
      }
      frame "Digitizer: Start" {
        # "send trigger to start acquisition loop"
        # "initilize aquisition"
        # "Start Digitizer\n(TClk start)"
        n747 = Unbundle By Name(w1617) -> ("niTClk sessions"=w1616:refnum<k20>[])
        n748 = call <instrlib>:"niTClk Initiate.vi"("error in (no error)"=w1610, "sessions"=w1616) -> ("error out"=w1612:errorcluster)  [unwired: 8 in, 1 out]
        n749 = Generate User Event(priority (normal)=usereventprio."high priority", user event=w1613, event data cluster=TRUE ("event data"), error in=w1612) -> (error out=w1611:errorcluster)  [unwired: 1 out]
        n750 = call <vilib>:"Add State(s) to Queue__JKI_lib_State_Machine.vi"("State(s) in (\"\")"=w1620) -> ("States Out"=w1619:string)  [unwired: 14 in]
      }
      frame "Digitizer: Abort" {
        # "Template Separator\n(You can make a copy of, or modify, this frame)"
        n751 = call "Digitizer1_FGV.vi"("error in (no error)"=w1624, "Operation (Read)"=enum16{"Write", "Read"}."Read" ("Operation")) -> ("error out"=w1631:errorcluster, "Read data"=w1628:refnum<k15>)  [unwired: 8 in]
        n752 = call "Digitizer2_FGV.vi"("error in (no error)"=w1624, "Operation (Read)"=enum16{"Write", "Read"}."Read" ("Operation")) -> ("error out"=w1627:errorcluster, "Read data"=w1629:refnum<k15>)  [unwired: 8 in]
        n753 = Bundle By Name(cluster=w1621, "SysRunning?"=FALSE ("System Status")) -> (w1622:T24)
        n754 = call <instrlib>:"niScope Abort.vi"("instrument handle"=w1628, "error in"=w1631) -> ("error out"=w1633:errorcluster)  [unwired: 12 in, 1 out]
        n755 = call <instrlib>:"niScope Abort.vi"("instrument handle"=w1629, "error in"=w1627) -> ("error out"=w1632:errorcluster)  [unwired: 12 in, 1 out]
        n756 = Merge Errors(w1633, w1632) -> (w1625:errorcluster)
        n757 = call <vilib>:"Add State(s) to Queue__JKI_lib_State_Machine.vi"("State(s) in (\"\")"=w1636) -> ("States Out"=w1635:string)  [unwired: 14 in]
      }
      frame "Digitizer: checkTemp" {
        w1639 = 65.0 ("y")
        w1644 = enum16{"Write", "Read"}."Read" ("Operation")
        # "Template Separator\n(You can make a copy of, or modify, this frame)"
        n758 = call "Digitizer1_FGV.vi"("Operation (Read)"=w1644) -> ("error out"=w1645:errorcluster, "Read data"=w1646:refnum<k15>)  [unwired: 9 in]
        n759 = call "Digitizer2_FGV.vi"("Operation (Read)"=w1644) -> ("error out"=w1642:errorcluster, "Read data"=w1643:refnum<k15>)  [unwired: 9 in]
        n760 = property on="Property Node" class="niScope"(reference=w1643, error in=w1642) -> ("Device Temperature"=w1640:dbl)  [unwired: 2 out]
        "Dig2 Temp" <- w1640
        n761 = property on="Property Node" class="niScope"(reference=w1646, error in=w1645) -> ("Device Temperature"=w1641:dbl)  [unwired: 2 out]
        "Dig1 Temp" <- w1641
        n762 = Greater?(x=w1641, y=w1639) -> (0:w1638:bool)
        n763 = Greater?(x=w1640, y=w1639) -> (0:w1637:bool)
        n764 = case shown="True" w1638 {
          frame False {
          }
          frame True {
            n765 = One Button Dialog(message="Digitizer 1 over heating!", button name ("OK")="OK") -> ()  [unwired: 1 out]
          }
        }
        n766 = case shown="True" w1637 {
          frame False {
          }
          frame True {
            n767 = One Button Dialog(message="Digitizer 2 over heating!", button name ("OK")="OK") -> ()  [unwired: 1 out]
          }
        }
        n768 = call <vilib>:"Add State(s) to Queue__JKI_lib_State_Machine.vi"("State(s) in (\"\")"=w1651) -> ("States Out"=w1650:string)  [unwired: 14 in]
      }
      frame "Digitizer: Close" {
        # "Close Digitizer"
        n769 = call "Digitizer1_FGV.vi"("error in (no error)"=w1661, "Operation (Read)"=enum16{"Write", "Read"}."Read" ("Operation")) -> ("error out"=w1663:errorcluster, "Read data"=w1667:refnum<k15>)  [unwired: 8 in]
        n770 = call "Digitizer2_FGV.vi"("error in (no error)"=w1661, "Operation (Read)"=enum16{"Write", "Read"}."Read" ("Operation")) -> ("error out"=w1662:errorcluster, "Read data"=w1665:refnum<k15>)  [unwired: 8 in]
        n771 = call <instrlib>:"niScope Close.vi"("instrument handle"=w1667, "error in"=w1663) -> ("error out"=w1660:errorcluster)  [unwired: 13 in]
        n772 = call <instrlib>:"niScope Close.vi"("instrument handle"=w1665, "error in"=w1662) -> ("error out"=w1659:errorcluster)  [unwired: 13 in]
        n773 = Merge Errors(w1660, w1659) -> (w1658:errorcluster)
        n774 = Unbundle By Name(w1658) -> ("status"=w1657:bool)
        n775 = Bundle By Name(cluster=w1668, "System Status.Digitizer"=w1657) -> (w1669:T24)
        n776 = call <vilib>:"Add State(s) to Queue__JKI_lib_State_Machine.vi"("State(s) in (\"\")"=w1671) -> ("States Out"=w1670:string)  [unwired: 14 in]
      }
      frame "---------- LabJack ----------" {
        # "Template Separator\n(You can make a copy of, or modify, this frame)"
        n777 = call <vilib>:"Add State(s) to Queue__JKI_lib_State_Machine.vi"("State(s) in (\"\")"=w1676) -> ("States Out"=w1675:string)  [unwired: 14 in]
      }
      frame "LabJack: checkPedal" {
        # "Template Separator\n(You can make a copy of, or modify, this frame)"
        n778 = Unbundle By Name(w1677) -> ("LJ Pinout.Foot Pedal"=w1681:string)
        n779 = call "LabJack_FGV.vi"("Operation(Read)"=enum16{"Write", "Read"}."Read" ("Operation"), "error in (no error)"=w1679) -> ("error out"=w1683:errorcluster, "Read data"=w1684:i32)  [unwired: 8 in]
        n780 = call "LJM_eReadName.vi"("Handle In"=w1684, "Name"=w1681, "error in"=w1683) -> ("Value"=w1682:dbl, "error out"=w1680:errorcluster)  [unwired: 10 in, 1 out]
        n781 = case shown="1" w1682 {
          tunnel: w1677 -> [w1689 w1692]
          tunnel: [w1689 w1690] -> w1678
          frame 0, Default {
          }
          frame 1 {
            # "If Pedal pressed"
            n782 = Tick Count (ms)() -> (millisecond timer value=w1696:u32)
            n783 = Unbundle By Name(w1692) -> ("Last Trigger"=w1691:u32)
            n784 = Subtract(x=w1696, y=w1691) -> (x-y=w1695:u32)
            n785 = Greater Or Equal?(x=w1695, y=u32 2000) -> (x >= y?=w1693:bool)
            n786 = case shown="True" w1693 {
              tunnel: w1692 -> [w1697 w1698]
              tunnel: w1691 -> [_ _]
              tunnel: [w1697 w1699] -> w1690
              frame False {
              }
              frame True {
                n787 = Tick Count (ms)() -> (millisecond timer value=w1700:u32)
                n788 = Unbundle By Name(w1698) -> ("SysRunning?"=w1701:bool)
                n789 = case shown="False" w1701 {
                  frame False {
                    n790 = property on="StartButton" class="Bool (strict)"("Val(Sgnl)"=TRUE ("Value (Signaling)")) -> ()  [unwired: 2 in, 2 out]
                  }
                  frame True {
                    n791 = property on="StopButton" class="Bool (strict)"("Val(Sgnl)"=TRUE ("Value (Signaling)")) -> ()  [unwired: 2 in, 2 out]
                  }
                }
                n792 = Bundle By Name(cluster=w1698, "Last Trigger"=w1700) -> (w1699:T24)
              }
            }
          }
        }
        n793 = call <vilib>:"Add State(s) to Queue__JKI_lib_State_Machine.vi"("State(s) in (\"\")"=w1688) -> ("States Out"=w1687:string)  [unwired: 14 in]
      }
      frame "LabJack: ZeroV" {
        # "Just Zero V\nDO not update FGV and front panel\nWIll resume from last V"
        # "set bias to 0"
        # "Zero APD bias\n(You can make a copy of, or modify, this frame)"
        n794 = Unbundle By Name(w1706) -> ("LJ Pinout.Ch1 Bias"=w1711:string, "LJ Pinout.Ch2 Bias"=w1710:string, "LJ Pinout.Ch3 Bias"=w1709:string)
        n795 = Build Array(w1711, w1710, w1709) -> (w1708:string[])
        n796 = call "LabJack_FGV.vi"("Operation(Read)"=enum16{"Write", "Read"}."Read" ("Operation"), "error in (no error)"=w1705) -> ("error out"=w1712:errorcluster, "Read data"=w1713:i32)  [unwired: 8 in]
        n797 = call "LJM_eWriteNames.vi"("Handle In"=w1713, "aNames"=w1708, "aValuesIn"=dbl[] [0.0, 0.0, 0.0], "error in"=w1712) -> ("error out"=w1704:errorcluster)  [unwired: 9 in, 2 out]
        n798 = call <vilib>:"Add State(s) to Queue__JKI_lib_State_Machine.vi"("State(s) in (\"\")"=w1717) -> ("States Out"=w1716:string)  [unwired: 14 in]
      }
      frame "LabJack: SetV" {
        w1724 = enum16{"write", "read"}."read" ("action (write)")
        # "set bias to user specifid"
        # "Set APD bias\n(You can make a copy of, or modify, this frame)"
        n799 = Unbundle By Name(w1733) -> ("LJ Pinout.Ch1 Bias"=w1737:string, "LJ Pinout.Ch2 Bias"=w1736:string, "LJ Pinout.Ch3 Bias"=w1735:string, "LJ Pinout.Ch4 Bias"=w1727:string)
        n800 = call "V2FGV.vi"("Error In"=w1723, "action(write)"=w1724) -> ("Error Out"=w1721:errorcluster, "V2 out"=w1729:dbl)  [unwired: 8 in]
        n801 = call "V4FGV.vi"("Error In"=w1723, "action(write)"=w1724) -> ("Error Out"=w1719:errorcluster, "V3 out"=w1725:dbl)  [unwired: 8 in]
        n802 = call "V1FGV.vi"("Error In"=w1723, "action (write)"=w1724) -> ("Error Out"=w1722:errorcluster, "V1 out"=w1726:dbl)  [unwired: 8 in]
        n803 = call "V3FGV.vi"("Error In"=w1723, "action(write)"=w1724) -> ("Error Out"=w1720:errorcluster, "V3 out"=w1728:dbl)  [unwired: 8 in]
        n804 = local write "V 3"(w1728) -> ()
        n805 = local write "V 2"(w1729) -> ()
        n806 = local write "V 4"(w1725) -> ()
        n807 = local write "V 1"(w1726) -> ()
        n808 = Build Array(w1737, w1736, w1735, w1727) -> (w1734:string[])
        n809 = call "LabJack_FGV.vi"("Operation(Read)"=enum16{"Write", "Read"}."Read" ("Operation"), "error in (no error)"=w1723) -> ("error out"=w1738:errorcluster, "Read data"=w1739:i32)  [unwired: 8 in]
        n810 = Build Array(w1726, w1729, w1728, w1725) -> (w1730:dbl[])
        n811 = call "LJM_eWriteNames.vi"("Handle In"=w1739, "aNames"=w1734, "aValuesIn"=w1730, "error in"=w1738) -> ("error out"=w1731:errorcluster)  [unwired: 9 in, 2 out]
        n812 = Merge Errors(w1722, w1721, w1720, w1719) -> (w1718:errorcluster)
        n813 = call <vilib>:"Add State(s) to Queue__JKI_lib_State_Machine.vi"("State(s) in (\"\")"=w1743) -> ("States Out"=w1742:string)  [unwired: 14 in]
        n814 = Merge Errors(w1718, w1731) -> (w1732:errorcluster)
      }
      frame "LabJack: Open" {
        # "Initialize LabJack T7\nEstablish connection and initialize pins"
        n815 = call "LJ_Open.vi"("error in"=w1753, "DeviceType"="LJM_dtT7") -> ("error out"=w1750:errorcluster, "Success?"=w1751:bool, "Handle Out"=w1745:i32)  [unwired: 7 in]
        n816 = call "LabJack_FGV.vi"("Operation(Read)"=enum16{"Write", "Read"}."Write" ("Operation"), "error in (no error)"=w1750, "Write data"=w1745) -> ("error out"=w1747:errorcluster)  [unwired: 7 in, 1 out]
        n817 = Bundle By Name(cluster=w1748, "System Status.Labjack"=w1751) -> (w1752:T24)
        n818 = call <vilib>:"Add State(s) to Queue__JKI_lib_State_Machine.vi"("State(s) in (\"\")"=w1755) -> ("States Out"=w1754:string)  [unwired: 14 in]
      }
      frame "LabJack: SetDefaultSub" {
        w1765 = enum16{"write", "read"}."write" ("action")
        w1766 = 0.0 ("V1 in")
        w1779 = "_EF_ENABLE" ("string")
        # "1. Disable PWM\n2. Set all V to 0\n3. Set 355 relay to open\n4. Set LED to off"
        # "read once to set DIO to input"
        # "set all initila V to 0. Set footpedal to input. Set PWM to low. Set laser relay to open. Set LEDs to yellow."
        # "Set Labjack to correct input and output state and initial values"
        n819 = disable-structure shown="Disabled" {
          frame Disabled {
            (unwired) dbl[] [0.0, 0.0, 0.0, 0.0, 0.0, 0.0, 0.0, 0.0, 0.0] ("aValuesIn")
          }
          frame Enabled {
          }
        }
        n820 = Unbundle By Name(w1776) -> ("LJ Pinout.355 PWM"=w1781:string, "LJ Pinout.AimingBeam PWM"=w1780:string, "LJ Pinout.Ch1 Bias"=w1786:string, "LJ Pinout.Ch2 Bias"=w1756:string, "LJ Pinout.Ch3 Bias"=w1790:string, "LJ Pinout.Ch4 Bias"=w1770:string, "LJ Pinout.Laser Start/Stop"=w1789:string, "LJ Pinout.Red LED"=w1788:string, "LJ Pinout.Green LED"=w1787:string)
        n821 = call "V1FGV.vi"("Error In"=w1774, "action (write)"=w1765, "V1 in"=w1766) -> ("Error Out"=w1769:errorcluster, "V1 out"=w1773:dbl)  [unwired: 7 in]
        n822 = local write "V 1"(w1773) -> ()
        n823 = call "V2FGV.vi"("Error In"=w1769, "action(write)"=w1765, "V2 in"=w1766) -> ("Error Out"=w1768:errorcluster, "V2 out"=w1772:dbl)  [unwired: 7 in]
        n824 = call "LabJack_FGV.vi"("Operation(Read)"=enum16{"Write", "Read"}."Read" ("Operation"), "error in (no error)"=w1774) -> ("error out"=w1762:errorcluster, "Read data"=w1784:i32)  [unwired: 8 in]
        n825 = Concatenate Strings(w1781, w1779) -> (w1778:string)
        n826 = Concatenate Strings(w1780, w1779) -> (w1777:string)
        n827 = local write "V 2"(w1772) -> ()
        n828 = call "V3FGV.vi"("Error In"=w1768, "action(write)"=w1765, "V3 in"=w1766) -> ("Error Out"=w1767:errorcluster, "V3 out"=w1771:dbl)  [unwired: 7 in]
        n829 = Build Array(w1778, w1777, w1786, w1756, w1790, w1770, w1789, w1788, w1787) -> (w1760:string[])
        n830 = local write "V 3"(w1771) -> ()
        n831 = call "V4FGV.vi"("Error In"=w1767, "action(write)"=w1765, "V3 in"=w1766) -> ("Error Out"=w1763:errorcluster, "V3 out"=w1764:dbl)  [unwired: 7 in]
        n832 = Array Size(array=w1760) -> (size(s)=w1759:i32)
        n833 = local write "V 4"(w1764) -> ()
        n834 = Initialize Array(0.0 ("element"), w1759) -> (w1757:dbl[])
        n835 = Unbundle By Name(w1776) -> ("LJ Pinout.Foot Pedal"=w1775:string)
        n836 = call "LJM_eWriteNames.vi"("Handle In"=w1784, "aNames"=w1760, "aValuesIn"=w1757, "error in"=w1762) -> ("Handle Out"=w1783:i32, "error out"=w1782:errorcluster)  [unwired: 9 in, 1 out]
        n837 = call "LJM_eReadName.vi"("Handle In"=w1783, "Name"=w1775, "error in"=w1782) -> ("error out"=w1761:errorcluster)  [unwired: 10 in, 2 out]
        n838 = case shown="Error .." w1761 {
          frame No Error {
            # "no error"
          }
          frame Error {
            # "handle error"
            n839 = One Button Dialog(message="Labjack error! The pin assignment is likely wrong. Please check pin setting of Labjack. Program will terminate.", button name ("OK")="OK") -> ()  [unwired: 1 out]
          }
        }
        n840 = call <vilib>:"Add State(s) to Queue__JKI_lib_State_Machine.vi"("State(s) in (\"\")"=w1793) -> ("States Out"=w1792:string)  [unwired: 14 in]
      }
      frame "LabJack: FootPedalConfig" {
        # "Setup footPedal\n(You can make a copy of, or modify, this frame)"
        n841 = call "LabJack_FGV.vi"("Operation(Read)"=enum16{"Write", "Read"}."Read" ("Operation"), "error in (no error)"=w1797) -> ("error out"=w1801:errorcluster, "Read data"=w1802:i32)  [unwired: 8 in]
        n842 = call "LJM_eWriteName.vi"("Handle In"=w1802, "Name"="DIO15", "Value"=1.0, "error in"=w1801) -> ("error out"=w1798:errorcluster)  [unwired: 10 in, 1 out]
        n843 = call <vilib>:"Add State(s) to Queue__JKI_lib_State_Machine.vi"("State(s) in (\"\")"=w1806) -> ("States Out"=w1805:string)  [unwired: 14 in]
      }
      frame "LabJack: SetDefaultAndClose" {
        # "Template Separator\n(You can make a copy of, or modify, this frame)"
        n844 = call <vilib>:"Add State(s) to Queue__JKI_lib_State_Machine.vi"("State(s) in Front (\"\")"="LabJack: SetDefaultSub\nLabJack: Close" ("State(s) in Front (\"\")"), "State(s) in (\"\")"=w1812) -> ("States Out"=w1811:string)  [unwired: 13 in]
      }
      frame "LabJack: Close" {
        # "Close LabJack Refnum"
        n845 = call "LabJack_FGV.vi"("Operation(Read)"=enum16{"Write", "Read"}."Read" ("Operation"), "error in (no error)"=w1818) -> ("error out"=w1813:errorcluster, "Read data"=w1814:i32)  [unwired: 8 in]
        n846 = Bundle By Name(cluster=w1816, "System Status.Labjack"=FALSE ("System Status.Gain Control")) -> (w1819:T24)
        n847 = call "LJM_Close.vi"("error in"=w1813, "Handle"=w1814) -> ("error out"=w1821:errorcluster)  [unwired: 9 in]
        n848 = call <vilib>:"Add State(s) to Queue__JKI_lib_State_Machine.vi"("State(s) in (\"\")"=w1823) -> ("States Out"=w1822:string)  [unwired: 14 in]
      }
      frame "LabJack: Interlock enable/disable" {
        w1832 = i8 0  # int8
        # "[Covers: REQ8]"
        # "Interlock enable/disable\n(Usage: \"LabJack: Interlock enable/disable >> 1|0\")"
        n849 = Fract/Exp String To Number(string=w1833, default (0 dbl)=w1832) -> (number=w1829:i8)  [unwired: 2 in, 1 out]
        n850 = Unbundle By Name(w1831) -> ("LJ Pinout.Interlock"=w1830:string)
        n851 = call "LabJack_FGV.vi"("Operation(Read)"=enum16{"Write", "Read"}."Read" ("Operation")) -> ("Read data"=w1827:i32)  [unwired: 9 in, 1 out]
        n852 = call "LJM_eWriteName.vi"("Handle In"=w1827, "Name"=w1830, "Value"=w1829, "error in"=w1828) -> ("error out"=w1825:errorcluster)  [unwired: 10 in, 1 out]
        n853 = call <vilib>:"Add State(s) to Queue__JKI_lib_State_Machine.vi"("State(s) in (\"\")"=w1835) -> ("States Out"=w1834:string)  [unwired: 14 in]
      }
      frame "LabJack: 355_PWM_Config" {
        w1837 = 0.0 ("element")
        w1857 = "DIO_EF_CLOCK1_ENABLE"
        # "Config PWM frequency"
        n854 = Unbundle By Name(w1849) -> ("LJ Pinout.355 PWM"=w1856:string)
        n855 = Unbundle By Name(w1849) -> ("355 PWM setting.DIO_EF_CLOCK1_DIVISOR"=w1848:i16, "355 PWM setting.DIO_EF_CLOCK1_ROLL_VALUE"=w1847:i32, "355 PWM setting.DIO#_EF_INDEX"=w1844:i16, "355 PWM setting.DIO#_EF_OPTIONS"=w1843:i16, "355 PWM setting.DIO#_EF_CONFIG_A"=w1842:i32)
        n856 = Concatenate Strings(w1856, "_EF_ENABLE" ("string")) -> (w1852:string)
        n857 = Concatenate Strings(w1856, "_EF_INDEX") -> (w1855:string)
        n858 = Concatenate Strings(w1856, "_EF_OPTIONS") -> (w1854:string)
        n859 = Concatenate Strings(w1856, "_EF_CONFIG_A") -> (w1853:string)
        n860 = call "LabJack_FGV.vi"("Operation(Read)"=enum16{"Write", "Read"}."Read" ("Operation")) -> ("Read data"=w1850:i32)  [unwired: 9 in, 1 out]
        n861 = Build Array(w1837, w1837, w1848, w1847, 1.0 ("element"), 0.0 ("element"), w1844, w1843, w1842) -> (w1841:dbl[])
        n862 = Build Array("DIO_EF_CLOCK0_ENABLE", w1857, "DIO_EF_CLOCK1_DIVISOR", "DIO_EF_CLOCK1_ROLL_VALUE", w1857, w1852, w1855, w1854, w1853) -> (w1851:string[])
        n863 = call "LJM_eWriteNames.vi"("Handle In"=w1850, "aNames"=w1851, "aValuesIn"=w1841, "error in"=w1839) -> ("error out"=w1840:errorcluster)  [unwired: 9 in, 2 out]
        n864 = call <vilib>:"Add State(s) to Queue__JKI_lib_State_Machine.vi"("State(s) in (\"\")"=w1866) -> ("States Out"=w1865:string)  [unwired: 14 in]
      }
      frame "LabJack: 355_PWM_Start" {
        # "Template Separator\n(You can make a copy of, or modify, this frame)"
        n865 = Unbundle By Name(w1874) -> ("LJ Pinout.355 PWM"=w1873:string)
        n866 = call "LabJack_FGV.vi"("Operation(Read)"=enum16{"Write", "Read"}."Read" ("Operation"), "error in (no error)"=w1868) -> ("error out"=w1875:errorcluster, "Read data"=w1876:i32)  [unwired: 8 in]
        n867 = Concatenate Strings(w1873, "_EF_ENABLE" ("string")) -> (w1871:string)
        n868 = call "LJM_eWriteName.vi"("Handle In"=w1876, "Name"=w1871, "Value"=1.0, "error in"=w1875) -> ("error out"=w1869:errorcluster)  [unwired: 10 in, 1 out]
        n869 = call <vilib>:"Add State(s) to Queue__JKI_lib_State_Machine.vi"("State(s) in (\"\")"=w1879) -> ("States Out"=w1878:string)  [unwired: 14 in]
      }
      frame "LabJack: 355_PWM_Stop" {
        # "Template Separator\n(You can make a copy of, or modify, this frame)"
        n870 = Unbundle By Name(w1885) -> ("LJ Pinout.355 PWM"=w1889:string)
        n871 = call "LabJack_FGV.vi"("Operation(Read)"=enum16{"Write", "Read"}."Read" ("Operation"), "error in (no error)"=w1884) -> ("error out"=w1890:errorcluster, "Read data"=w1882:i32)  [unwired: 8 in]
        n872 = Concatenate Strings(w1889, "_EF_ENABLE" ("string")) -> (w1887:string)
        n873 = call "LJM_eWriteName.vi"("Handle In"=w1882, "Name"=w1887, "Value"=0.0, "error in"=w1890) -> ("error out"=w1881:errorcluster)  [unwired: 10 in, 1 out]
        n874 = local write "355nm Laser toggle"(FALSE ("355nm Laser toggle")) -> ()
        n875 = call <vilib>:"Add State(s) to Queue__JKI_lib_State_Machine.vi"("State(s) in (\"\")"=w1893) -> ("States Out"=w1892:string)  [unwired: 14 in]
      }
      frame "LabJack: AB_Start" {
        # "Aiming Beam Start\n(Based on aimging beam frequency, set LabJack pin)"
        n876 = Unbundle By Name(w1903) -> ("AB Cluster.Freq"=w1895:i32, "LJ Pinout.AimingBeam PWM"=w1902:string)
        n877 = Greater Than 0?(x=w1895) -> (x > 0?=w1894:bool)
        n878 = case shown="False" w1894 {
          tunnel: w1902 -> [w1909 w1912]
          tunnel: [w1909 w1910] -> w1901
          frame False {
            # "if 0 freq, set PWM pin"
          }
          frame True {
            # "if non zero freq, set PWM enable"
            n879 = Concatenate Strings(w1912, "_EF_ENABLE" ("string")) -> (w1910:string)
          }
        }
        n880 = call "LabJack_FGV.vi"("Operation(Read)"=enum16{"Write", "Read"}."Read" ("Operation"), "error in (no error)"=w1898) -> ("error out"=w1904:errorcluster, "Read data"=w1905:i32)  [unwired: 8 in]
        n881 = call "LJM_eWriteName.vi"("Handle In"=w1905, "Name"=w1901, "Value"=1.0, "error in"=w1904) -> ("error out"=w1899:errorcluster)  [unwired: 10 in, 1 out]
        n882 = local write "Aiming beam toggle"(TRUE ("Aiming beam toggle")) -> ()
        n883 = call <vilib>:"Add State(s) to Queue__JKI_lib_State_Machine.vi"("State(s) in (\"\")"=w1908) -> ("States Out"=w1907:string)  [unwired: 14 in]
      }
      frame "LabJack: AB_Stop" {
        # "Aiming Beam Stop\n(Based on aiming beam frequency, set LabJack pin low)"
        n884 = Unbundle By Name(w1920) -> ("AB Cluster.Freq"=w1915:i32, "LJ Pinout.AimingBeam PWM"=w1922:string)
        n885 = Greater Than 0?(x=w1915) -> (x > 0?=w1914:bool)
        n886 = case shown="False" w1914 {
          tunnel: w1922 -> [w1928 w1931]
          tunnel: [w1928 w1929] -> w1913
          frame False {
          }
          frame True {
            n887 = Concatenate Strings(w1931, "_EF_ENABLE" ("string")) -> (w1929:string)
          }
        }
        n888 = call "LabJack_FGV.vi"("Operation(Read)"=enum16{"Write", "Read"}."Read" ("Operation"), "error in (no error)"=w1918) -> ("error out"=w1923:errorcluster, "Read data"=w1924:i32)  [unwired: 8 in]
        n889 = call "LJM_eWriteName.vi"("Handle In"=w1924, "Name"=w1913, "Value"=0.0, "error in"=w1923) -> ("error out"=w1919:errorcluster)  [unwired: 10 in, 1 out]
        n890 = local write "Aiming beam toggle"(FALSE ("Aiming beam toggle")) -> ()
        n891 = call <vilib>:"Add State(s) to Queue__JKI_lib_State_Machine.vi"("State(s) in (\"\")"=w1927) -> ("States Out"=w1926:string)  [unwired: 14 in]
      }
      frame "LabJack: AB_PWM_Config" {
        w1933 = 0.0 ("element")
        w1953 = "DIO_EF_CLOCK2_ENABLE"
        # "Config PWM frequency"
        n892 = Unbundle By Name(w1945) -> ("LJ Pinout.AimingBeam PWM"=w1952:string)
        n893 = Unbundle By Name(w1945) -> ("AB PWM setting.DIO_EF_CLOCK1_DIVISOR"=w1944:i16, "AB PWM setting.DIO_EF_CLOCK1_ROLL_VALUE"=w1943:i32, "AB PWM setting.DIO#_EF_INDEX"=w1940:i16, "AB PWM setting.DIO#_EF_OPTIONS"=w1939:i16, "AB PWM setting.DIO#_EF_CONFIG_A"=w1938:i32)
        n894 = Concatenate Strings(w1952, "_EF_ENABLE" ("string")) -> (w1948:string)
        n895 = Concatenate Strings(w1952, "_EF_INDEX") -> (w1951:string)
        n896 = Concatenate Strings(w1952, "_EF_OPTIONS") -> (w1950:string)
        n897 = Concatenate Strings(w1952, "_EF_CONFIG_A") -> (w1949:string)
        n898 = call "LabJack_FGV.vi"("Operation(Read)"=enum16{"Write", "Read"}."Read" ("Operation")) -> ("Read data"=w1946:i32)  [unwired: 9 in, 1 out]
        n899 = Build Array(w1933, w1933, w1944, w1943, 1.0 ("element"), 0.0 ("element"), w1940, w1939, w1938) -> (w1937:dbl[])
        n900 = Build Array("DIO_EF_CLOCK0_ENABLE", w1953, "DIO_EF_CLOCK2_DIVISOR", "DIO_EF_CLOCK2_ROLL_VALUE", w1953, w1948, w1951, w1950, w1949) -> (w1947:string[])
        n901 = call "LJM_eWriteNames.vi"("Handle In"=w1946, "aNames"=w1947, "aValuesIn"=w1937, "error in"=w1935) -> ("error out"=w1936:errorcluster)  [unwired: 9 in, 2 out]
        n902 = call <vilib>:"Add State(s) to Queue__JKI_lib_State_Machine.vi"("State(s) in (\"\")"=w1962) -> ("States Out"=w1961:string)  [unwired: 14 in]
      }
      frame "---------- LED ----------" {
        # "Template Separator\n(You can make a copy of, or modify, this frame)"
        n903 = call <vilib>:"Add State(s) to Queue__JKI_lib_State_Machine.vi"("State(s) in (\"\")"=w1967) -> ("States Out"=w1966:string)  [unwired: 14 in]
      }
      frame "LED: OpenVIRef" {
        # "Template Separator\n(You can make a copy of, or modify, this frame)"
        n904 = call <vilib>:"Application Directory.vi"() -> ("Application Directory"=w1974:path)
        n905 = Build Path(base path=w1974, name or relative path="SubVI") -> (appended path=w1972:path)
        n906 = Build Path(base path=w1972, name or relative path="LEDBreath.vi") -> (appended path=w1970:path)
        n907 = Open VI Reference(vi path=w1970, error in (no error)=w1975) -> (vi reference=w1976:refnum<vi>, error out=w1969:errorcluster)  [unwired: 4 in]
        n908 = case shown="Error .." w1969 {
          tunnel: [TRUE FALSE] -> w1968
          frame No Error {
          }
          frame Error {
          }
        }
        n909 = Bundle By Name(cluster=w1977, "LED vi reference"=w1976, "LED vi ref open?"=w1968) -> (w1978:T24)
        n910 = call <vilib>:"Add State(s) to Queue__JKI_lib_State_Machine.vi"("State(s) in (\"\")"=w1981) -> ("States Out"=w1980:string)  [unwired: 14 in]
      }
      frame "LED: CloseVIRef" {
        # "Template Separator\n(You can make a copy of, or modify, this frame)"
        n911 = Unbundle By Name(w1985) -> ("LED vi reference"=w1986:refnum<vi>, "LED vi ref open?"=w1984:bool)
        n912 = case shown="True" w1984 {
          tunnel: w1988 -> [w1992 w1995]
          tunnel: [w1992 w1994] -> w1987
          tunnel: w1986 -> [_ w1993]
          frame False {
          }
          frame True {
            n913 = Close Reference(reference=w1993, error in (no error)=w1995) -> (error out=w1994:errorcluster)
          }
        }
        n914 = call <vilib>:"Add State(s) to Queue__JKI_lib_State_Machine.vi"("State(s) in (\"\")"=w1991) -> ("States Out"=w1990:string)  [unwired: 14 in]
      }
      frame "LED: BreathGreen" {
        w1996 = FALSE ("Wait Until Done")
        # "Breath system LED\n(LED: Breath >> True/False)"
        n915 = Unbundle By Name(w2004) -> ("LED vi reference"=w2003:refnum<vi>)
        n916 = invoke class="VI" method="Ctrl Val.Set"(reference=w2003, error in=w2001, "Control Name"="Color", "Value"=0) -> (reference out=w2000:refnum<vi>, error out=w1999:errorcluster)  [unwired: 1 in, 3 out]
        n917 = invoke on="Invoke Node" class="VI" method="Run VI"(reference=w2000, error in=w1999, "Wait until done"=w1996, "Auto Dispose Ref"=w1996) -> (error out=w2002:errorcluster)  [unwired: 1 in, 4 out]
        n918 = call <vilib>:"Add State(s) to Queue__JKI_lib_State_Machine.vi"("State(s) in (\"\")"=w2007) -> ("States Out"=w2006:string)  [unwired: 14 in]
      }
      frame "LED: BreathOrange" {
        w2008 = FALSE ("Wait Until Done")
        # "Breath system LED\n(LED: Breath >> True/False)"
        n919 = Unbundle By Name(w2016) -> ("LED vi reference"=w2015:refnum<vi>)
        n920 = invoke class="VI" method="Ctrl Val.Set"(reference=w2015, error in=w2013, "Control Name"="Color", "Value"=1) -> (reference out=w2012:refnum<vi>, error out=w2011:errorcluster)  [unwired: 1 in, 3 out]
        n921 = invoke on="Invoke Node" class="VI" method="Run VI"(reference=w2012, error in=w2011, "Wait until done"=w2008, "Auto Dispose Ref"=w2008) -> (error out=w2014:errorcluster)  [unwired: 1 in, 4 out]
        n922 = call <vilib>:"Add State(s) to Queue__JKI_lib_State_Machine.vi"("State(s) in (\"\")"=w2019) -> ("States Out"=w2018:string)  [unwired: 14 in]
      }
      frame "LED: BreathOff" {
        # "System LED Breath Off\n(Breath off, check VI status to make sure it is off)"
        n923 = Unbundle By Name(w2028) -> ("LED vi reference"=w2027:refnum<vi>)
        n924 = invoke on="Invoke Node" class="VI" method="Ctrl Val.Set"(reference=w2027, error in=w2025, "Control Name"="Stop", "Value"=TRUE) -> (reference out=w2020:refnum<vi>, error out=w2021:errorcluster)  [unwired: 1 in, 3 out]
        n925 = case shown="No Error" w2021 {
          selector: w2021 -> [w2033 _]
          tunnel: [w2032 errorcluster {"status"=FALSE, "code"=0, "source"=""} ("error IO")] -> w2026
          tunnel: ["" ("State(s) in Front (\"\")") "LED: BreathOff" ("State(s) in Front (\"\")")] -> w2024
          tunnel: w2020 -> [w2034 _]
          frame No Error {
            # "No error, wait for VI to stop"
            n926 = while {
              tunnel: w2034 -> [w2042]
              shift-right: [w2036] -> w2032
              shift-left: w2033 -> [w2041]
              stop <- w2038 stop-if-true
              # "continue check whether vi is running"
              n927 = property class="VI"(reference=w2042, error in=w2041) -> (error out=w2036:errorcluster, "Exec.State"=w2040:T21)  [unwired: 1 out]
              n928 = Wait (ms)(milliseconds to wait=u32 50) -> ()  [unwired: 1 out]
              n929 = Equal?(x=w2040, y=T21."Idle") -> (x = y?=w2038:bool)
            }
          }
          frame Error {
            # "try again when error"
          }
        }
        n930 = call <vilib>:"Add State(s) to Queue__JKI_lib_State_Machine.vi"("State(s) in Front (\"\")"=w2024, "State(s) in (\"\")"=w2031) -> ("States Out"=w2030:string)  [unwired: 13 in]
      }
      frame "LED: Off" {
        # "set LED to red"
        # "Template Separator\n(You can make a copy of, or modify, this frame)"
        n931 = Unbundle By Name(w2047) -> ("LJ Pinout.Red LED"=w2046:string, "LJ Pinout.Green LED"=w2045:string)
        n932 = call "LabJack_FGV.vi"("Operation(Read)"=enum16{"Write", "Read"}."Read" ("Operation"), "error in (no error)"=w2048) -> ("error out"=w2055:errorcluster, "Read data"=w2054:i32)  [unwired: 8 in]
        n933 = call "LJM_eWriteName.vi"("Handle In"=w2054, "Name"=w2046, "Value"=0.0, "error in"=w2055) -> ("Handle Out"=w2052:i32, "error out"=w2051:errorcluster)  [unwired: 10 in]
        n934 = call "LJM_eWriteName.vi"("Handle In"=w2052, "Name"=w2045, "Value"=0.0, "error in"=w2051) -> ("error out"=w2049:errorcluster)  [unwired: 10 in, 1 out]
        n935 = call <vilib>:"Add State(s) to Queue__JKI_lib_State_Machine.vi"("State(s) in (\"\")"=w2059) -> ("States Out"=w2058:string)  [unwired: 14 in]
      }
      frame "LED: Green" {
        # "set LED to green"
        # "Template Separator\n(You can make a copy of, or modify, this frame)"
        n936 = Unbundle By Name(w2063) -> ("LJ Pinout.Red LED"=w2061:string, "LJ Pinout.Green LED"=w2062:string)
        n937 = call "LabJack_FGV.vi"("Operation(Read)"=enum16{"Write", "Read"}."Read" ("Operation"), "error in (no error)"=w2065) -> ("error out"=w2071:errorcluster, "Read data"=w2070:i32)  [unwired: 8 in]
        n938 = call "LJM_eWriteName.vi"("Handle In"=w2070, "Name"=w2061, "Value"=0.0, "error in"=w2071) -> ("Handle Out"=w2068:i32, "error out"=w2067:errorcluster)  [unwired: 10 in]
        n939 = call "LJM_eWriteName.vi"("Handle In"=w2068, "Name"=w2062, "Value"=9.0, "error in"=w2067) -> ("error out"=w2064:errorcluster)  [unwired: 10 in, 1 out]
        n940 = call <vilib>:"Add State(s) to Queue__JKI_lib_State_Machine.vi"("State(s) in (\"\")"=w2074) -> ("States Out"=w2073:string)  [unwired: 14 in]
      }
      frame "---------- Queue ----------" {
        # "Template Separator\n(You can make a copy of, or modify, this frame)"
        n941 = call <vilib>:"Add State(s) to Queue__JKI_lib_State_Machine.vi"("State(s) in (\"\")"=w2079) -> ("States Out"=w2078:string)  [unwired: 14 in]
      }
      frame "Queue: Flash" {
        # "Clear queue contnet\n(clear queue content by flash it)"
        n942 = Flush Queue(queue=w2086, error in (no error)=w2080) -> (error out=w2084:errorcluster)  [unwired: 2 out]
        n943 = Flush Queue(queue=w2087, error in (no error)=w2080) -> (error out=w2083:errorcluster)  [unwired: 2 out]
        n944 = Flush Queue(queue=w2085, error in (no error)=w2080) -> (error out=w2082:errorcluster)  [unwired: 2 out]
        n945 = Merge Errors(w2084, w2083, w2082) -> (w2081:errorcluster)
        n946 = call <vilib>:"Add State(s) to Queue__JKI_lib_State_Machine.vi"("State(s) in (\"\")"=w2091) -> ("States Out"=w2090:string)  [unwired: 14 in]
      }
      frame "Queue: Destory" {
        # "Destory Data Queue\nDistory data queue ref so the aquisition loop stop"
        n947 = Release Queue(queue=w2097, error in (no error)=w2093) -> (error out=w2100:errorcluster)  [unwired: 1 in, 2 out]
        n948 = Release Queue(queue=w2096, error in (no error)=w2093) -> (error out=w2099:errorcluster)  [unwired: 1 in, 2 out]
        n949 = Release Queue(queue=w2094, error in (no error)=w2093) -> (error out=w2092:errorcluster)  [unwired: 1 in, 2 out]
        n950 = Merge Errors(w2100, w2099, w2092) -> (w2098:errorcluster)
        n951 = call <vilib>:"Simple Error Handler.vi"("error in (no error)"=w2098) -> ()  [unwired: 4 in, 5 out]
        n952 = call <vilib>:"Add State(s) to Queue__JKI_lib_State_Machine.vi"("State(s) in (\"\")"=w2103) -> ("States Out"=w2102:string)  [unwired: 14 in]
      }
      frame "---------- Run ----------" {
        # "Template Separator\n(You can make a copy of, or modify, this frame)"
        n953 = call <vilib>:"Add State(s) to Queue__JKI_lib_State_Machine.vi"("State(s) in (\"\")"=w2108) -> ("States Out"=w2107:string)  [unwired: 14 in]
      }
      frame "Run: CaliIncrement" {
        # "Increment Calibration #\n(You can make a copy of, or modify, this frame)"
        n954 = Unbundle By Name(w2110) -> ("IDs.Cali ID"=w2112:i8)
        n955 = Increment(x=w2112) -> (x+1=w2109:i8)
        n956 = Bundle By Name(cluster=w2110, "IDs.Cali ID"=w2109) -> (w2111:T24)
        n957 = call <vilib>:"Add State(s) to Queue__JKI_lib_State_Machine.vi"("State(s) in (\"\")"=w2116) -> ("States Out"=w2115:string)  [unwired: 14 in]
      }
      frame "Run: BGIncrement" {
        # "Increment BG #\n(You can make a copy of, or modify, this frame)"
        n958 = Unbundle By Name(w2117) -> ("IDs.BG ID"=w2120:i8)
        n959 = Increment(x=w2120) -> (x+1=w2119:i8)
        n960 = Bundle By Name(cluster=w2117, "IDs.BG ID"=w2119) -> (w2118:T24)
        n961 = call <vilib>:"Add State(s) to Queue__JKI_lib_State_Machine.vi"("State(s) in (\"\")"=w2124) -> ("States Out"=w2123:string)  [unwired: 14 in]
      }
      frame "Run: Increment" {
        # "Increase Run# by 1"
        n962 = Unbundle By Name(w2129) -> ("IDs.RunID"=w2131:i8)
        n963 = Increment(x=w2131) -> (x+1=w2127:i8)
        n964 = Bundle By Name(cluster=w2129, "IDs.RunID"=w2127) -> (w2130:T24)
        n965 = call "RunIDFGV.vi"("Error In"=w2125, "RunID in"=w2127) -> ("Error Out"=w2126:errorcluster)  [unwired: 8 in, 1 out]
        n966 = call <vilib>:"Add State(s) to Queue__JKI_lib_State_Machine.vi"("State(s) in (\"\")"=w2133) -> ("States Out"=w2132:string)  [unwired: 14 in]
      }
      frame "Run: Decrement" {
        # "Increase Run# by 1"
        n967 = Unbundle By Name(w2138) -> ("IDs.RunID"=w2140:i8)
        n968 = Decrement(x=w2140) -> (x-1=w2136:i8)
        n969 = Bundle By Name(cluster=w2138, "IDs.RunID"=w2136) -> (w2139:T24)
        n970 = call "RunIDFGV.vi"("Error In"=w2134, "RunID in"=w2136) -> ("Error Out"=w2135:errorcluster)  [unwired: 8 in, 1 out]
        n971 = call <vilib>:"Add State(s) to Queue__JKI_lib_State_Machine.vi"("State(s) in (\"\")"=w2142) -> ("States Out"=w2141:string)  [unwired: 14 in]
      }
      frame "---------- SysConfig ----------" {
        # "Template Separator\n(You can make a copy of, or modify, this frame)"
        n972 = call <vilib>:"Add State(s) to Queue__JKI_lib_State_Machine.vi"("State(s) in (\"\")"=w2147) -> ("States Out"=w2146:string)  [unwired: 14 in]
      }
      frame "SysConfig: LoadAPDSerialNumber" {
        # "Template Separator\n(You can make a copy of, or modify, this frame)"
        n973 = call "readAPDSerial.vi"("Error In"=w2149) -> ("Error Out"=w2148:errorcluster, "output cluster"=w2150:T27)  [unwired: 9 in]
        n974 = Bundle By Name(cluster=w2151, "APDSerialNum"=w2150) -> (w2152:T24)
        n975 = call <vilib>:"Add State(s) to Queue__JKI_lib_State_Machine.vi"("State(s) in (\"\")"=w2155) -> ("States Out"=w2154:string)  [unwired: 14 in]
      }
      frame "SysConfig: Load Sys Config" {
        # "[Covers: REQ5]"
        # "Load System config"
        # "Load system configuration\n(Load both hardware and DAQ config)"
        n976 = call "LoadSysConfig.vi"("Error In"=w2158, "Enum"=enum16{"LastUse", "Default"}."LastUse") -> ("Error Out"=w2157:errorcluster, "SysConfigCluster"=w2160:T7)  [unwired: 8 in]
        "SysConfigCluster" <- w2160
        n977 = Bundle By Name(cluster=w2161, "SysConfigCluster"=w2160) -> (w2162:T24)
        n978 = call <vilib>:"Add State(s) to Queue__JKI_lib_State_Machine.vi"("State(s) in (\"\")"=w2164) -> ("States Out"=w2163:string)  [unwired: 14 in]
      }
      frame "SysConfig: Load Digitizer Setting" {
        w2165 = enum16{"Write", "Read"}."Write" ("Operation")
        # "Load DAQ config\nSave to FGV"
        # "Template Separator\n(You can make a copy of, or modify, this frame)"
        n979 = call <userlib>:"Current VIs Parent Directory__ogtk.vi"() -> ("Parent Directory (+ Relative)"=w2179:path)  [unwired: 5 in]
        n980 = Build Path(base path=w2179, name or relative path="SubVI\\DigitizerConfiguration\\V6_Scope_last_use.config") -> (appended path=w2180:path)
        n981 = call "ReadDigitizerConfig(SubVI).vi"("error in (no error)"=w2177, "appended path"=w2180) -> ("error out"=w2173:errorcluster, "FLImDAQ"=w2171:T5)  [unwired: 8 in]
        n982 = call "FLImDAQ_FGV.vi"("error in (no error)"=w2173, "Operation (Read)"=w2165, "Write data"=w2171) -> ("error out"=w2175:errorcluster)  [unwired: 7 in, 1 out]
        n983 = Unbundle By Name(w2171) -> ("min record length"=→"data length":i32, "Digitizer 1"=w2167:refnum<k15>, "Digitizer 2"=w2174:refnum<k15>)
        n984 = Bundle By Name(cluster=w2169, "FLImDAQ"=w2171) -> (w2170:T24)
        n985 = call "Digitizer1_FGV.vi"("error in (no error)"=w2175, "Operation (Read)"=w2165, "Write data"=w2167) -> ("error out"=w2176:errorcluster)  [unwired: 7 in, 1 out]
        n986 = call "Digitizer2_FGV.vi"("error in (no error)"=w2176, "Operation (Read)"=w2165, "Write data"=w2174) -> ("error out"=w2172:errorcluster)  [unwired: 7 in, 1 out]
        n987 = call <vilib>:"Add State(s) to Queue__JKI_lib_State_Machine.vi"("State(s) in (\"\")"=w2182) -> ("States Out"=w2181:string)  [unwired: 14 in]
      }
      frame "SysConfig: Load LJ Pinout" {
        # "Template Separator\n(You can make a copy of, or modify, this frame)"
        n988 = call <userlib>:"Current VIs Parent Directory__ogtk.vi"() -> ("Parent Directory (+ Relative)"=w2197:path)  [unwired: 5 in]
        n989 = Build Path(base path=w2197, name or relative path="SubVI\\LabJack\\LJ_pin_setting.config") -> (appended path=w2195:path)
        n990 = call "ReadLabjackConfig(SubVI).vi"("error in (no error)"=w2193, "appended path"=w2195) -> ("error out"=w2194:errorcluster, "Utility"=w2191:T4)  [unwired: 8 in]
        n991 = Unbundle By Name(w2191) -> ("Ch1 Bias"=w2190:string, "Ch2 Bias"=w2189:string, "Ch3 Bias"=w2188:string, "Ch4 Bias"=w2183:string, "Red LED"=w2185:string, "Green LED"=w2184:string)
        n992 = global write "GlobalVariables.vi" "LED Green pin"(w2184) -> ()
        n993 = global write "GlobalVariables.vi" "Ch1 LJ pin"(w2190) -> ()
        n994 = global write "GlobalVariables.vi" "Ch2 LJ pin"(w2189) -> ()
        n995 = global write "GlobalVariables.vi" "Ch3 LJ pin"(w2188) -> ()
        n996 = global write "GlobalVariables.vi" "Ch4 LJ pin"(w2183) -> ()
        n997 = global write "GlobalVariables.vi" "LED Red pin"(w2185) -> ()
        n998 = Bundle By Name(cluster=w2186, "LJ Pinout"=w2191) -> (w2192:T24)
        n999 = call <vilib>:"Add State(s) to Queue__JKI_lib_State_Machine.vi"("State(s) in (\"\")"=w2199) -> ("States Out"=w2198:string)  [unwired: 14 in]
      }
      frame "SysConfig: Load 355 PWM" {
        # "Template Separator\n(You can make a copy of, or modify, this frame)"
        n1000 = call <userlib>:"Current VIs Parent Directory__ogtk.vi"() -> ("Parent Directory (+ Relative)"=w2217:path)  [unwired: 5 in]
        n1001 = Build Path(base path=w2217, name or relative path="SubVI\\LabJack\\PWM_setting_355.config") -> (appended path=w2215:path)
        n1002 = call "ReadPWMConfig(SubVI).vi"("error in (no error)"=w2212, "appended path"=w2215) -> ("error out"=w2213:errorcluster, "PWM Setting"=w2211:T42)  [unwired: 8 in]
        n1003 = Unbundle By Name(w2211) -> ("DIO_EF_CLOCK1_DIVISOR"=w2208:i16, "DIO_EF_CLOCK1_ROLL_VALUE"=w2207:i32)
        n1004 = Multiply(x=w2208, y=w2207) -> (x*y=w2209:i32)
        n1005 = Bundle By Name(cluster=w2214, "355 PWM setting"=w2211) -> (w2201:T24)
        n1006 = Divide(x=80000000.0, y=w2209) -> (x/y=w2206:dbl)
        "Laser Rep Rate" <- w2206
        n1007 = Number To Decimal String(number=w2206) -> (decimal integer string=w2205:string)  [unwired: 1 in]
        n1008 = Concatenate Strings("355nm " ("string"), w2205, "Hz" ("string")) -> (w2203:string)
        n1009 = property on="355nm Laser toggle" class="Bool (strict)"("Caption.Text"=w2203) -> ()  [unwired: 2 in, 2 out]
        n1010 = call <vilib>:"Add State(s) to Queue__JKI_lib_State_Machine.vi"("State(s) in (\"\")"=w2219) -> ("States Out"=w2218:string)  [unwired: 14 in]
      }
      frame "SysConfig: Load AB PWM" {
        # "Template Separator\n(You can make a copy of, or modify, this frame)"
        n1011 = call <userlib>:"Current VIs Parent Directory__ogtk.vi"() -> ("Parent Directory (+ Relative)"=w2228:path)  [unwired: 5 in]
        n1012 = Build Path(base path=w2228, name or relative path="SubVI\\LabJack\\PWM_setting_AB.config") -> (appended path=w2226:path)
        n1013 = call "ReadPWMConfig(SubVI).vi"("error in (no error)"=w2223, "appended path"=w2226) -> ("error out"=w2224:errorcluster, "PWM Setting"=w2222:T42)  [unwired: 8 in]
        n1014 = Bundle By Name(cluster=w2220, "AB PWM setting"=w2222) -> (w2225:T24)
        n1015 = call <vilib>:"Add State(s) to Queue__JKI_lib_State_Machine.vi"("State(s) in (\"\")"=w2230) -> ("States Out"=w2229:string)  [unwired: 14 in]
      }
      frame "SysConfig: Load AB setting" {
        # "load aming beam setting\n(check frequency, if 0 do nothing, if not zero, config PWM)"
        n1016 = call "readAimingBeamSetting.vi"("error in (no error)"=w2244) -> ("error out"=w2239:errorcluster, "Aiming Beam Setting"=w2232:T43)  [unwired: 9 in]
        n1017 = Unbundle By Name(w2232) -> ("Frequency(Hz)"=w2231:u32)
        n1018 = Equal To 0?(x=w2231) -> (x = 0?=w2237:bool)
        n1019 = Select(t="", s=w2237, f="SysConfig: Load AB PWM" ("State(s) in Front (\"\")")) -> (s? t:f=w2240:string)
        n1020 = Number To Decimal String(number=w2231) -> (decimal integer string=w2236:string)  [unwired: 1 in]
        n1021 = Concatenate Strings("488nm " ("string"), w2236, "Hz " ("string")) -> (w2235:string)
        n1022 = property on="Aiming beam toggle" class="Bool (strict)"("Caption.Text"=w2235) -> ()  [unwired: 2 in, 2 out]
        n1023 = case shown="False" w2237 {
          tunnel: w2239 -> [w2252 w2255]
          tunnel: [w2251 w2255] -> w2238
          tunnel: w2231 -> [w2250 _]
          frame False {
            n1024 = call "LJ_calculate_PWM_parameters.vi"("Duty Cycle (%)"=u32 10, "Error In"=w2252, "Show Confirmation"=FALSE, "Laser Rep Rate (Hz)"=w2250, "Laser"=enum16{"355nm", "AimingBeam"}."AimingBeam") -> ("Error Out"=w2251:errorcluster)  [unwired: 5 in, 1 out]
          }
          frame True {
          }
        }
        n1025 = Bundle By Name(cluster=w2245, "AB Cluster"=w2232) -> (w2246:T24)
        n1026 = call <vilib>:"Add State(s) to Queue__JKI_lib_State_Machine.vi"("State(s) in Front (\"\")"=w2240, "State(s) in (\"\")"=w2248) -> ("States Out"=w2247:string)  [unwired: 13 in]
      }
      frame "SysConfig: LoadABVideoSetting" {
        # "Load AB video setting form ini file\n()"
        n1027 = call "readVideoConfig.vi"("error in (no error)"=w2259) -> ("error out"=w2260:errorcluster, "Aiming Beam Config"=w2258:T23)  [unwired: 8 in, 1 out]
        n1028 = Bundle By Name(cluster=w2256, "VideoConfig"=w2258) -> (w2257:T24)
        n1029 = call <vilib>:"Add State(s) to Queue__JKI_lib_State_Machine.vi"("State(s) in (\"\")"=w2263) -> ("States Out"=w2262:string)  [unwired: 14 in]
      }
      frame "SysConfig: LoadCursorLocation" {
        # "Load cursor location from ini file\n(load cursor from system setting ini file)"
        n1030 = call "readCursorConfigMain.vi"("error in (no error)"=w2275) -> ("error out"=w2276:errorcluster, "Cursor Locations"=w2274:T44)  [unwired: 9 in]
        n1031 = Unbundle By Name(w2274) -> ("DC1"=w2273:i32, "DC2"=w2272:i32, "BG1"=w2267:i32, "BG2"=w2266:i32)
        n1032 = Build Array(w2273, w2272) -> (w2271:i32[])
        n1033 = Build Array(w2267, w2266) -> (w2268:i32[])
        n1034 = Array Max & Min(array=w2271) -> (max value=w2270:i32, min value=w2269:i32)  [unwired: 2 out]
        n1035 = Array Max & Min(array=w2268) -> (max value=w2265:i32, min value=w2264:i32)  [unwired: 2 out]
        n1036 = global write "GlobalVariables.vi" "DC Idx2"(w2270) -> ()
        n1037 = global write "GlobalVariables.vi" "DC Idx1"(w2269) -> ()
        n1038 = global write "GlobalVariables.vi" "BG Idx2"(w2265) -> ()
        n1039 = global write "GlobalVariables.vi" "BG Idx1"(w2264) -> ()
        n1040 = call <vilib>:"Add State(s) to Queue__JKI_lib_State_Machine.vi"("State(s) in (\"\")"=w2280) -> ("States Out"=w2279:string)  [unwired: 14 in]
      }
      frame "---------- SystemStatus ----------" {
        # "Template Separator\n(You can make a copy of, or modify, this frame)"
        n1041 = call <vilib>:"Add State(s) to Queue__JKI_lib_State_Machine.vi"("State(s) in (\"\")"=w2285) -> ("States Out"=w2284:string)  [unwired: 14 in]
      }
      frame "SystemStatus: SlowSysStatusMacro" {
        # "store system check time"
        # "Template Separator\n(You can make a copy of, or modify, this frame)"
        n1042 = Tick Count (ms)() -> (millisecond timer value=w2288:u32)
        n1043 = Bundle By Name(cluster=w2286, "SlowTimer"=w2288) -> (w2287:T24)
        n1044 = call <vilib>:"Add State(s) to Queue__JKI_lib_State_Machine.vi"("State(s) in Front (\"\")"="Digitizer: checkTemp\nTCP: CheckConnection" ("State(s) in Front (\"\")"), "State(s) in (\"\")"=w2293) -> ("States Out"=w2292:string)  [unwired: 13 in]
      }
      frame "SystemStatus: FastSysStatusMacro" {
        # "store system check time"
        # "Template Separator\n(You can make a copy of, or modify, this frame)"
        n1045 = Tick Count (ms)() -> (millisecond timer value=w2296:u32)
        n1046 = Bundle By Name(cluster=w2294, "FastTimer"=w2296) -> (w2295:T24)
        n1047 = call <vilib>:"Add State(s) to Queue__JKI_lib_State_Machine.vi"("State(s) in Front (\"\")"="355 Laser: CheckPWMStatus\nAimingBeam: GetPWMStatus\n/*355 Laser: CheckControllerStatus" ("State(s) in Front (\"\")"), "State(s) in (\"\")"=w2301) -> ("States Out"=w2300:string)  [unwired: 13 in]
      }
      frame "---------- UI ----------" {
        # "Do not put any code in this frame.\n(It is a separator no-op. You can make a copy of this frame to create a new UI frame)"
        n1048 = call <vilib>:"Add State(s) to Queue__JKI_lib_State_Machine.vi"("State(s) in (\"\")"=w2306) -> ("States Out"=w2305:string)  [unwired: 14 in]
      }
      frame "UI: Initialize" {
        w2308 = T45 {"Minimum"=0.0, "Maximum"=4.6, "Increment"=0.1} ("Data Entry Limits")
        w2307 = T13."Disabled and Grayed Out" ("Disabled")
        # "Disable all button on startup"
        # "Initialize the User Interface, here.\n(this is called automatically, by the Macro: Init)"
        n1049 = property on="V 1" class="DigNum (strict)"("DisabledEnum"=w2307) -> ()  [unwired: 2 in, 2 out]
        n1050 = property on="V 2" class="DigNum (strict)"("DisabledEnum"=w2307) -> ()  [unwired: 2 in, 2 out]
        n1051 = property on="StopButton" class="Bool (strict)"("DisabledEnum"=w2307) -> ()  [unwired: 2 in, 2 out]
        n1052 = property on="Sys Reconfig" class="Bool"("DisabledEnum"=w2307) -> ()  [unwired: 2 in, 2 out]
        n1053 = property on="StartButton" class="Bool (strict)"("DisabledEnum"=w2307) -> ()  [unwired: 2 in, 2 out]
        n1054 = property on="355nm Laser toggle" class="Bool (strict)"("DisabledEnum"=w2307) -> ()  [unwired: 2 in, 2 out]
        n1055 = property on="Aiming beam toggle" class="Bool (strict)"("DisabledEnum"=w2307) -> ()  [unwired: 2 in, 2 out]
        n1056 = property on="Background" class="Bool (strict)"("DisabledEnum"=w2307) -> ()  [unwired: 2 in, 2 out]
        n1057 = property on="Cali&iRF alignment" class="Bool (strict)"("DisabledEnum"=w2307) -> ()  [unwired: 2 in, 2 out]
        n1058 = property on="V 3" class="DigNum (strict)"("DisabledEnum"=w2307) -> ()  [unwired: 2 in, 2 out]
        n1059 = property on="Video Source" class="RadioBtnsControl (strict)"("DisabledEnum"=w2307) -> ()  [unwired: 2 in, 2 out]
        n1060 = property on="V 1" class="DigNum (strict)"("Data Range"=w2308) -> ()  [unwired: 2 in, 2 out]
        n1061 = property on="V 2" class="DigNum (strict)"("Data Range"=w2308) -> ()  [unwired: 2 in, 2 out]
        n1062 = property on="V 3" class="DigNum (strict)"("Data Range"=w2308) -> ()  [unwired: 2 in, 2 out]
        n1063 = call <vilib>:"Add State(s) to Queue__JKI_lib_State_Machine.vi"("State(s) in Front (\"\")"="UI: CaliAndiRFNotReady" ("State(s) in Front (\"\")"), "State(s) in (\"\")"=w2314) -> ("States Out"=w2313:string)  [unwired: 13 in]
      }
      frame "UI: BGLoaded" {
        # "[Covers: REQ24]"
        # "Do not put any code in this frame.\n(It is a separator no-op. You can make a copy of this frame to create a new UI frame)"
        n1064 = property on="Background" class="Bool (strict)"("BoolText.Text"="Loaded!" ("Boolean Text.Text"), "Colors [4]"=cluster{u32, u32}[] [{15764023, 15764023}, {16711680, 16711680}]) -> ()  [unwired: 2 in, 2 out]
        n1065 = call <vilib>:"Add State(s) to Queue__JKI_lib_State_Machine.vi"("State(s) in (\"\")"=w2321) -> ("States Out"=w2320:string)  [unwired: 14 in]
      }
      frame "UI: BGSizeError" {
        # "[Covers: REQ24]"
        # "Do not put any code in this frame.\n(It is a separator no-op. You can make a copy of this frame to create a new UI frame)"
        n1066 = property on="Background" class="Bool (strict)"("BoolText.Text"="Loaded!" ("Boolean Text.Text"), "Colors [4]"=cluster{u32, u32}[] [{7171459, 7171459}, {16711680, 16711680}]) -> ()  [unwired: 2 in, 2 out]
        n1067 = One Button Dialog(message="Background waveform length and current digitizer setting mismatch! Please take a new background before any aquisition!") -> ()  [unwired: 1 in, 1 out]
        n1068 = call <vilib>:"Add State(s) to Queue__JKI_lib_State_Machine.vi"("State(s) in (\"\")"=w2329) -> ("States Out"=w2328:string)  [unwired: 14 in]
      }
      frame "UI: CaliAndiRFLoaded" {
        # "[Covers: REQ24]"
        # "Do not put any code in this frame.\n(It is a separator no-op. You can make a copy of this frame to create a new UI frame)"
        n1069 = property on="Cali&iRF alignment" class="Bool (strict)"("BoolText.Text"="Loaded!" ("Boolean Text.Text"), "Colors [4]"=cluster{u32, u32}[] [{15764023, 15764023}, {16711680, 16711680}]) -> ()  [unwired: 2 in, 2 out]
        n1070 = call <vilib>:"Add State(s) to Queue__JKI_lib_State_Machine.vi"("State(s) in (\"\")"=w2336) -> ("States Out"=w2335:string)  [unwired: 14 in]
      }
      frame "UI: WFAutoScale" {
        # "Set graph auto scale.\n(UI: WFAutoScale >> T/F)"
        n1071 = Equal?(x=w2337, y="F") -> (x = y?=w2338:bool)
        n1072 = Equal?(x=w2337, y="T") -> (x = y?=w2340:bool)
        n1073 = case shown="True" w2340 {
          frame False {
          }
          frame True {
            w2356 = u8 2 ("Y Scale.Scale Fit")
            n1074 = property on="Channel 1" class="WFGraph (strict)"("YScale.ScaleFit"=w2356) -> ()  [unwired: 2 in, 2 out]
            n1075 = property on="Channel 2" class="WFGraph (strict)"("YScale.ScaleFit"=w2356) -> ()  [unwired: 2 in, 2 out]
            n1076 = property on="Channel 3" class="WFGraph (strict)"("YScale.ScaleFit"=w2356) -> ()  [unwired: 2 in, 2 out]
          }
        }
        n1077 = case shown="True" w2338 {
          frame False {
          }
          frame True {
            w2353 = 0.0 ("Y Scale.Range:Maximum")
            w2354 = 2.0 ("Y Scale.Range:Maximum")
            w2355 = u8 0 ("Y Scale.Scale Fit")
            n1078 = property on="Channel 1" class="WFGraph (strict)"("YScale.ScaleFit"=w2355) -> (error out=w2352:errorcluster)  [unwired: 2 in, 1 out]
            n1079 = property on="Channel 2" class="WFGraph (strict)"("YScale.ScaleFit"=w2355) -> (error out=w2351:errorcluster)  [unwired: 2 in, 1 out]
            n1080 = property on="Channel 3" class="WFGraph (strict)"("YScale.ScaleFit"=w2355) -> (error out=w2350:errorcluster)  [unwired: 2 in, 1 out]
            n1081 = property on="Channel 1" class="WFGraph (strict)"(error in=w2352, "YScale.Maximum"=w2354) -> (error out=w2349:errorcluster)  [unwired: 1 in, 1 out]
            n1082 = property on="Channel 2" class="WFGraph (strict)"(error in=w2351, "YScale.Maximum"=w2354) -> (error out=w2348:errorcluster)  [unwired: 1 in, 1 out]
            n1083 = property on="Channel 3" class="WFGraph (strict)"(error in=w2350, "YScale.Maximum"=w2354) -> (error out=w2347:errorcluster)  [unwired: 1 in, 1 out]
            n1084 = property on="Channel 1" class="WFGraph (strict)"(error in=w2349, "YScale.Minimum"=w2353) -> ()  [unwired: 1 in, 2 out]
            n1085 = property on="Channel 2" class="WFGraph (strict)"(error in=w2348, "YScale.Minimum"=w2353) -> ()  [unwired: 1 in, 2 out]
            n1086 = property on="Channel 3" class="WFGraph (strict)"(error in=w2347, "YScale.Minimum"=w2353) -> ()  [unwired: 1 in, 2 out]
          }
        }
        n1087 = call <vilib>:"Add State(s) to Queue__JKI_lib_State_Machine.vi"("State(s) in (\"\")"=w2346) -> ("States Out"=w2345:string)  [unwired: 14 in]
      }
      frame "UI: showDisclaimer" {
        # "Show disclamer window.\n(It is a separator no-op. You can make a copy of this frame to create a new UI frame)"
        n1088 = call <vilib>:"Application Directory.vi"() -> ("Application Directory"=w2369:path)
        n1089 = Build Path(base path=w2369, name or relative path="Disclamer.png") -> (appended path=w2367:path)
        n1090 = property on="Disclamer" class="Pict"() -> ("Draw Area Size"=w2365:T46)  [unwired: 2 in, 2 out]
        n1091 = disable-structure "Diagram Disable Structure" shown="Disabled" {
          frame Disabled {
            n1092 = flat-sequence {
              frame #0 {
                n1093 = call "disclaimer.vi"() -> ()  [unwired: 12 in]
              }
              frame #1 {
                n1094 = Wait (ms)(milliseconds to wait=u32 250) -> ()  [unwired: 1 out]
              }
              frame #2 {
                n1095 = call "SoftwareNote.vi"() -> ()  [unwired: 12 in]
              }
            }
          }
          frame Enabled {
          }
        }
        n1096 = call <vilib>:"Read PNG File.vi"("path to PNG file"=w2367) -> ("image data"=w2364:T47)  [unwired: 8 in, 2 out]
        n1097 = Unbundle By Name(w2364) -> ("Rectangle.right"=w2362:i16, "Rectangle.bottom"=w2360:i16)
        n1098 = Unbundle By Name(w2365) -> ("Width"=w2363:u32, "Height"=w2361:u32)
        n1099 = call <vilib>:"Draw Flattened Pixmap.vi"("image data"=w2364) -> ("new picture"=→"Disclamer":picture)  [unwired: 8 in]
        n1100 = Divide(x=w2363, y=w2362) -> (x/y=w2359:dbl)
        n1101 = Divide(x=w2361, y=w2360) -> (x/y=w2358:dbl)
        n1102 = Max & Min(x=w2359, y=w2358) -> (min(x,y)=w2357:dbl)  [unwired: 1 out]
        n1103 = property on="Disclamer" class="Pict"("ZoomFactor"=w2357) -> ()  [unwired: 2 in, 2 out]
        n1104 = call <vilib>:"Add State(s) to Queue__JKI_lib_State_Machine.vi"("State(s) in (\"\")"=w2374) -> ("States Out"=w2373:string)  [unwired: 14 in]
      }
      frame "UI: CaliAndiRFNotReady" {
        # "Do not put any code in this frame.\n(It is a separator no-op. You can make a copy of this frame to create a new UI frame)"
        n1105 = property on="Cali&iRF alignment" class="Bool (strict)"("BoolText.Text"="No Info" ("Boolean Text.Text"), "Colors [4]"=cluster{u32, u32}[] [{13816530, 13816530}, {16711680, 16711680}]) -> ()  [unwired: 2 in, 2 out]
        n1106 = call <vilib>:"Add State(s) to Queue__JKI_lib_State_Machine.vi"("State(s) in (\"\")"=w2382) -> ("States Out"=w2381:string)  [unwired: 14 in]
      }
      frame "UI: BGnotReady" {
        # "Do not put any code in this frame.\n(It is a separator no-op. You can make a copy of this frame to create a new UI frame)"
        n1107 = property on="Background" class="Bool (strict)"("BoolText.Text"="No Info" ("Boolean Text.Text"), "Colors [4]"=cluster{u32, u32}[] [{13816530, 13816530}, {16711680, 16711680}]) -> ()  [unwired: 2 in, 2 out]
        n1108 = call <vilib>:"Add State(s) to Queue__JKI_lib_State_Machine.vi"("State(s) in (\"\")"=w2389) -> ("States Out"=w2388:string)  [unwired: 14 in]
      }
      frame "UI: Reset" {
        w2391 = cluster{u32, u32}[] [{13816530, 13816530}, {13816530, 13816530}] ("Colors [4]")
        # "Do not put any code in this frame.\n(It is a separator no-op. You can make a copy of this frame to create a new UI frame)"
        n1109 = property on="Cali&iRF alignment" class="Bool (strict)"("BoolText.Text"="No Info" ("Boolean Text.Text"), "Colors [4]"=w2391) -> ()  [unwired: 2 in, 2 out]
        n1110 = property on="Background" class="Bool (strict)"("BoolText.Text"="No Info" ("Boolean Text.Text"), "Colors [4]"=w2391) -> ()  [unwired: 2 in, 2 out]
        n1111 = call <vilib>:"Add State(s) to Queue__JKI_lib_State_Machine.vi"("State(s) in (\"\")"=w2397) -> ("States Out"=w2396:string)  [unwired: 14 in]
      }
      frame "UI: SetButtonText" {
        # "Set button text of 355nm laser and aiming beam."
        n1112 = call <vilib>:"Add State(s) to Queue__JKI_lib_State_Machine.vi"("State(s) in (\"\")"=w2402) -> ("States Out"=w2401:string)  [unwired: 14 in]
      }
      frame "UI: DuringAquisition" {
        w2405 = T13."Disabled and Grayed Out" ("Disabled")
        # "Do not put any code in this frame.\n(It is a separator no-op. You can make a copy of this frame to create a new UI frame)"
        n1113 = Unbundle By Name(w2404) -> ("bothVidSourceAvail"=w2403:bool)
        n1114 = case shown="True" w2403 {
          tunnel: w2405 -> [_ w2411]
          frame False {
          }
          frame True {
            n1115 = property on="Video Source" class="RadioBtnsControl (strict)"("DisabledEnum"=w2411) -> ()  [unwired: 2 in, 2 out]
          }
        }
        n1116 = property on="StartButton" class="Bool (strict)"("DisabledEnum"=w2405) -> ()  [unwired: 2 in, 2 out]
        n1117 = property on="Sys Reconfig" class="Bool"("DisabledEnum"=w2405) -> ()  [unwired: 2 in, 2 out]
        n1118 = property on="355nm Laser toggle" class="Bool (strict)"("DisabledEnum"=w2405) -> ()  [unwired: 2 in, 2 out]
        n1119 = property on="Aiming beam toggle" class="Bool (strict)"("DisabledEnum"=w2405) -> ()  [unwired: 2 in, 2 out]
        n1120 = property on="Background" class="Bool (strict)"("DisabledEnum"=w2405) -> ()  [unwired: 2 in, 2 out]
        n1121 = property on="Radio Buttons" class="RadioBtnsControl (strict)"("DisabledEnum"=w2405) -> ()  [unwired: 2 in, 2 out]
        n1122 = property on="Cali&iRF alignment" class="Bool (strict)"("DisabledEnum"=w2405) -> ()  [unwired: 2 in, 2 out]
        n1123 = property on="Quit" class="Bool"("DisabledEnum"=w2405) -> ()  [unwired: 2 in, 2 out]
        n1124 = property on="Skip Data Save?" class="Bool (strict)"("DisabledEnum"=w2405) -> ()  [unwired: 2 in, 2 out]
        n1125 = property on="Video Display" class="Bool (strict)"("DisabledEnum"=w2405) -> ()  [unwired: 2 in, 2 out]
        n1126 = property on="StopButton" class="Bool (strict)"("DisabledEnum"=T13."Enabled" ("Disabled")) -> ()  [unwired: 2 in, 2 out]
        n1127 = call <vilib>:"Add State(s) to Queue__JKI_lib_State_Machine.vi"("State(s) in (\"\")"=w2410) -> ("States Out"=w2409:string)  [unwired: 14 in]
      }
      frame "UI: duringIRFAlign" {
        w2412 = T13."Disabled and Grayed Out" ("Disabled")
        # "Set UI to during iRF alignment\n(It is a separator no-op. You can make a copy of this frame to create a new UI frame)"
        n1128 = property on="StartButton" class="Bool (strict)"("DisabledEnum"=w2412) -> ()  [unwired: 2 in, 2 out]
        n1129 = property on="Sys Reconfig" class="Bool"("DisabledEnum"=w2412) -> ()  [unwired: 2 in, 2 out]
        n1130 = property on="355nm Laser toggle" class="Bool (strict)"("DisabledEnum"=w2412) -> ()  [unwired: 2 in, 2 out]
        n1131 = property on="Aiming beam toggle" class="Bool (strict)"("DisabledEnum"=w2412) -> ()  [unwired: 2 in, 2 out]
        n1132 = property on="Background" class="Bool (strict)"("DisabledEnum"=w2412) -> ()  [unwired: 2 in, 2 out]
        n1133 = property on="StopButton" class="Bool (strict)"("DisabledEnum"=w2412) -> ()  [unwired: 2 in, 2 out]
        n1134 = call <vilib>:"Add State(s) to Queue__JKI_lib_State_Machine.vi"("State(s) in (\"\")"=w2417) -> ("States Out"=w2416:string)  [unwired: 14 in]
      }
      frame "UI: duringBGAcquire" {
        w2418 = T13."Disabled and Grayed Out" ("Disabled")
        # "Do not put any code in this frame.\n(It is a separator no-op. You can make a copy of this frame to create a new UI frame)"
        n1135 = property on="StartButton" class="Bool (strict)"("DisabledEnum"=w2418) -> ()  [unwired: 2 in, 2 out]
        n1136 = property on="StopButton" class="Bool (strict)"("DisabledEnum"=w2418) -> ()  [unwired: 2 in, 2 out]
        n1137 = property on="Sys Reconfig" class="Bool"("DisabledEnum"=w2418) -> ()  [unwired: 2 in, 2 out]
        n1138 = property on="355nm Laser toggle" class="Bool (strict)"("DisabledEnum"=w2418) -> ()  [unwired: 2 in, 2 out]
        n1139 = property on="Aiming beam toggle" class="Bool (strict)"("DisabledEnum"=w2418) -> ()  [unwired: 2 in, 2 out]
        n1140 = property on="Cali&iRF alignment" class="Bool (strict)"("DisabledEnum"=w2418) -> ()  [unwired: 2 in, 2 out]
        n1141 = call <vilib>:"Add State(s) to Queue__JKI_lib_State_Machine.vi"("State(s) in (\"\")"=w2423) -> ("States Out"=w2422:string)  [unwired: 14 in]
      }
      frame "UI: ReadyForAquisition" {
        w2427 = T13."Enabled" ("Disabled")
        # "Do not put any code in this frame.\n(It is a separator no-op. You can make a copy of this frame to create a new UI frame)"
        n1142 = Unbundle By Name(w2426) -> ("System Status.TCP/IP"=w2425:bool, "bothVidSourceAvail"=w2424:bool)
        n1143 = property on="StartButton" class="Bool (strict)"("DisabledEnum"=w2427) -> ()  [unwired: 2 in, 2 out]
        n1144 = property on="Sys Reconfig" class="Bool"("DisabledEnum"=w2427) -> ()  [unwired: 2 in, 2 out]
        n1145 = property on="355nm Laser toggle" class="Bool (strict)"("DisabledEnum"=w2427) -> ()  [unwired: 2 in, 2 out]
        n1146 = property on="Aiming beam toggle" class="Bool (strict)"("DisabledEnum"=w2427) -> ()  [unwired: 2 in, 2 out]
        n1147 = property on="Cali&iRF alignment" class="Bool (strict)"("DisabledEnum"=w2427) -> ()  [unwired: 2 in, 2 out]
        n1148 = property on="Background" class="Bool (strict)"("DisabledEnum"=w2427) -> ()  [unwired: 2 in, 2 out]
        n1149 = property on="Quit" class="Bool"("DisabledEnum"=w2427) -> ()  [unwired: 2 in, 2 out]
        n1150 = property on="Radio Buttons" class="RadioBtnsControl (strict)"("DisabledEnum"=w2427) -> ()  [unwired: 2 in, 2 out]
        n1151 = case shown="True" w2424 {
          tunnel: w2427 -> [_ w2433]
          frame False {
          }
          frame True {
            n1152 = property on="Video Source" class="RadioBtnsControl (strict)"("DisabledEnum"=w2433) -> ()  [unwired: 2 in, 2 out]
          }
        }
        n1153 = property on="Skip Data Save?" class="Bool (strict)"("DisabledEnum"=w2427) -> ()  [unwired: 2 in, 2 out]
        n1154 = case shown="True" w2425 {
          tunnel: w2427 -> [_ w2434]
          frame False {
          }
          frame True {
            n1155 = property on="Video Display" class="Bool (strict)"("DisabledEnum"=w2434) -> ()  [unwired: 2 in, 2 out]
          }
        }
        n1156 = property on="StopButton" class="Bool (strict)"("DisabledEnum"=T13."Disabled and Grayed Out" ("Disabled")) -> ()  [unwired: 2 in, 2 out]
        n1157 = call <vilib>:"Add State(s) to Queue__JKI_lib_State_Machine.vi"("State(s) in (\"\")"=w2432) -> ("States Out"=w2431:string)  [unwired: 14 in]
      }
      frame "UI: Update" {
        # "Do not put any code in this frame.\n(It is a separator no-op. You can make a copy of this frame to create a new UI frame)"
        n1158 = Unbundle By Name(w2445) -> ("System Status"=→"System Hardware Connection Status":T2, "IDs.RunID"=→"Run #":i8, "CaseID"=→"Case #":string, "FLImDAQ"=→"FLImDAQ":T31, "SysRunning?"=→"Aquisition Status:":bool, "LJ Pinout"=→"LJ Pinout":T4, "IDs.BG ID"=→"BG #":i8, "IDs.Cali ID"=→"Calibration #":i8, "video source"=→"Visualization PC video source":T1)
        n1159 = call <vilib>:"Add State(s) to Queue__JKI_lib_State_Machine.vi"("State(s) in (\"\")"=w2448) -> ("States Out"=w2447:string)  [unwired: 14 in]
      }
      frame "UI: updateVideoToggle" {
        # "Set video toggle based on visualization PC video source.\n(take )"
        n1160 = call <vilib>:"Add State(s) to Queue__JKI_lib_State_Machine.vi"("State(s) in (\"\")"=w2453) -> ("States Out"=w2452:string)  [unwired: 14 in]
      }
      frame "UI: Cursor Set" {
        # "Argument"
        # "Set and Unset Cursor Busy.\n(Usage: \"UI: Cursor Set >> Busy|Idle\")"
        n1161 = case shown="\"Idle\", Default" w2455 {
          tunnel: w2457 -> [w2462 w2464]
          tunnel: [w2461 w2463] -> w2456
          frame "Idle", Default {
            n1162 = call <vilib>:"Unset Busy.vi"("error in (no error)"=w2462) -> ("error out"=w2461:errorcluster)  [unwired: 10 in]
          }
          frame "Busy" {
            n1163 = call <vilib>:"Set Busy.vi"("error in (no error)"=w2464) -> ("error out"=w2463:errorcluster)  [unwired: 9 in, 1 out]
          }
        }
        n1164 = call <vilib>:"Add State(s) to Queue__JKI_lib_State_Machine.vi"("State(s) in (\"\")"=w2460) -> ("States Out"=w2459:string)  [unwired: 14 in]
      }
      frame "UI: OverlayDialog" {
        # "0: Gain\n1: HN Classifier\n2: Brain Classifier"
        # "Ask user to selection overlay option\n(It is a separator no-op. You can make a copy of this frame to create a new UI frame)"
        n1165 = call <vilib>:"Three Button Dialog.vi"("Allow user to close window? (TRUE)"=FALSE, "Window Title (\"\")"="Overlay selection" ("Window Title (\"\")"), "Right Button Text (\"Cancel\")"="Brain Classifier" ("Right Button Text (\"Cancel\")"), "Center Button Text (\"No\")"="HN Classifier" ("Center Button Text (\"No\")"), "Left Button Text (\"Yes\")"="Gain" ("Left Button Text (\"Yes\")"), "message"="Please comfirm aiming beam colorbar setting and select overlay type! \nUpdate overlay colorbar if needed and restart aiming beam before selection.  ") -> ("Which Button?"=w2467:T48)  [unwired: 5 in]
        n1166 = To Unsigned Word Integer(number=w2467) -> (unsigned 16bit integer=w2466:u16)
        "OverlaySelection" <- w2466
        n1167 = Bundle By Name(cluster=w2469, "OverlaySelection"=w2467) -> (w2468:T24)
        n1168 = case shown="2" w2466 {
          tunnel: [w2479 w2481 w2483] -> w2465
          frame 0, Default {
            w2479 = u16 0 items=["Gain", "Lifetime", "CancerProbability"] ("Overlay selection")
          }
          frame 1 {
            w2481 = u16 2 items=["Gain", "Lifetime", "CancerProbability"] ("Overlay selection")
            n1169 = local write "CancerThreshold"(0.15 ("CancerThreshold")) -> ()
          }
          frame 2 {
            w2483 = u16 2 items=["Gain", "Lifetime", "CancerProbability"] ("Overlay selection")
            n1170 = local write "CancerThreshold"(0.35 ("CancerThreshold")) -> ()
          }
        }
        n1171 = local write "Overlay selection"(w2465) -> ()
      }
      frame "UI: Front Panel State" {
        # "Argument"
        # "Set Front Panel Open or Closed\n(Usage: \"UI: Front Panel State >> Open|Close\")"
        n1172 = Unbundle By Name(w2487) -> ("Core.Current VI Reference"=w2486:refnum<vi>)
        n1173 = case shown="\"Open\", \"Standard\", Default" w2485 {
          tunnel: w2489 -> [w2497 w2512 w2523 w2536 w2549]
          tunnel: [w2499 w2513 w2525 w2538 w2551] -> w2488
          tunnel: w2486 -> [w2498 w2510 w2524 w2537 w2550]
          frame "Open", "Standard", Default {
            w2492 = T18."Standard" ("State")
            n1174 = property on="Property Node" class="VI"(reference=w2498, error in=w2497) -> (reference out=w2495:refnum<vi>, error out=w2496:errorcluster, "FP.State"=w2494:T18)
            n1175 = Not Equal?(x=w2494, y=w2492) -> (x != y?=w2493:bool)
            n1176 = case shown="True" w2493 {
              tunnel: [w2503 w2505] -> w2499
              tunnel: w2496 -> [w2502 w2505]
              tunnel: w2495 -> [w2501 _]
              tunnel: w2492 -> [w2500 _]
              frame True {
                n1177 = invoke on="Invoke Node" class="VI" method="FP.Open"(reference=w2501, error in=w2502, "Activate"=TRUE, "State"=w2500) -> (error out=w2503:errorcluster)  [unwired: 1 in, 4 out]
              }
              frame False {
              }
            }
          }
          frame "Close", "Closed" {
            n1178 = property on="Property Node" class="VI"(reference=w2510, error in=w2512) -> (reference out=w2509:refnum<vi>, error out=w2511:errorcluster, "FP.State"=w2507:T18)
            n1179 = Not Equal?(x=w2507, y=T18."Closed" ("Front Panel Window:State")) -> (x != y?=w2506:bool)
            n1180 = case shown="True" w2506 {
              tunnel: [w2514 w2517] -> w2513
              tunnel: w2511 -> [w2514 w2516]
              tunnel: w2509 -> [_ w2515]
              frame False {
              }
              frame True {
                n1181 = invoke on="Invoke Node" class="VI" method="FP.Close"(reference=w2515, error in=w2516) -> (error out=w2517:errorcluster)  [unwired: 1 in, 2 out]
              }
            }
          }
          frame "Hidden", "Hide" {
            w2518 = T18."Hidden" ("State")
            n1182 = property on="Property Node" class="VI"(reference=w2524, error in=w2523) -> (reference out=w2521:refnum<vi>, error out=w2522:errorcluster, "FP.State"=w2520:T18)
            n1183 = Not Equal?(x=w2520, y=w2518) -> (x != y?=w2519:bool)
            n1184 = case shown="True" w2519 {
              tunnel: [w2529 w2530] -> w2525
              tunnel: w2522 -> [w2528 w2530]
              tunnel: w2521 -> [w2527 _]
              tunnel: w2518 -> [w2526 _]
              frame True {
                n1185 = invoke on="Invoke Node" class="VI" method="FP.Open"(reference=w2527, error in=w2528, "State"=w2526) -> (error out=w2529:errorcluster)  [unwired: 2 in, 4 out]
              }
              frame False {
              }
            }
          }
          frame "Minimize", "Minimized" {
            w2531 = T18."Minimized" ("State")
            n1186 = property on="Property Node" class="VI"(reference=w2537, error in=w2536) -> (reference out=w2534:refnum<vi>, error out=w2535:errorcluster, "FP.State"=w2533:T18)
            n1187 = Not Equal?(x=w2533, y=w2531) -> (x != y?=w2532:bool)
            n1188 = case shown="True" w2532 {
              tunnel: [w2542 w2543] -> w2538
              tunnel: w2535 -> [w2541 w2543]
              tunnel: w2534 -> [w2540 _]
              tunnel: w2531 -> [w2539 _]
              frame True {
                n1189 = invoke on="Invoke Node" class="VI" method="FP.Open"(reference=w2540, error in=w2541, "State"=w2539) -> (error out=w2542:errorcluster)  [unwired: 2 in, 4 out]
              }
              frame False {
              }
            }
          }
          frame "Maximize", "Maximized" {
            w2544 = T18."Maximized" ("State")
            n1190 = property on="Property Node" class="VI"(reference=w2550, error in=w2549) -> (reference out=w2547:refnum<vi>, error out=w2548:errorcluster, "FP.State"=w2546:T18)
            n1191 = Not Equal?(x=w2546, y=w2544) -> (x != y?=w2545:bool)
            n1192 = case shown="True" w2545 {
              tunnel: [w2555 w2556] -> w2551
              tunnel: w2548 -> [w2554 w2556]
              tunnel: w2547 -> [w2553 _]
              tunnel: w2544 -> [w2552 _]
              frame True {
                n1193 = invoke on="Invoke Node" class="VI" method="FP.Open"(reference=w2553, error in=w2554, "State"=w2552) -> (error out=w2555:errorcluster)  [unwired: 2 in, 4 out]
              }
              frame False {
              }
            }
          }
        }
        n1194 = call <vilib>:"Add State(s) to Queue__JKI_lib_State_Machine.vi"("State(s) in (\"\")"=w2491) -> ("States Out"=w2490:string)  [unwired: 14 in]
      }
      frame "---------- AimingBeam ----------" {
        # "Template Separator\n(You can make a copy of, or modify, this frame)"
        n1195 = call <vilib>:"Add State(s) to Queue__JKI_lib_State_Machine.vi"("State(s) in (\"\")"=w2561) -> ("States Out"=w2560:string)  [unwired: 14 in]
      }
      frame "AimingBeam: Initialize" {
        # "set aiming beam button color"
        # "Open COM port for Aiming Beam\n(Require USB connection)"
        n1196 = Unbundle By Name(w2563) -> ("AB Cluster.Aiming Beam COM Port"=w2571:refnum<visa-resource-name>)
        n1197 = call-poly "VISA Configure Serial Port"("VISA resource name"=w2571, "Enable Termination\nChar (T)"=TRUE ("Enable Termination\nChar (T)"), "baud rate (9600)"=u32 9600, "error in (no error)"=w2568) -> ("error out"=w2567:errorcluster)  [unwired: 10 in, 1 out]
        n1198 = Unbundle By Name(w2567) -> ("status"=w2566:bool)
        n1199 = Not(x=w2566) -> (.not. x?=w2565:bool)
        n1200 = Bundle By Name(cluster=w2563, "System Status.Aiming Beam"=w2565) -> (w2564:T24)
        n1201 = call <vilib>:"Add State(s) to Queue__JKI_lib_State_Machine.vi"("State(s) in (\"\")"=w2573) -> ("States Out"=w2572:string)  [unwired: 14 in]
      }
      frame "AimingBeam: Close" {
        # "Close Aiming Beam COM port\n(Require USB connection to Aiming Beam Laser)"
        n1202 = Unbundle By Name(w2576) -> ("AB Cluster.Aiming Beam COM Port"=w2580:refnum<visa-resource-name>)
        n1203 = VISA Close(VISA resource name=w2580, error in (no error)=w2578) -> (error out=w2579:errorcluster)
        n1204 = Bundle By Name(cluster=w2576, "System Status.Aiming Beam"=FALSE) -> (w2577:T24)
        n1205 = call <vilib>:"Add State(s) to Queue__JKI_lib_State_Machine.vi"("State(s) in (\"\")"=w2582) -> ("States Out"=w2581:string)  [unwired: 14 in]
      }
      frame "AimingBeam: Set Current" {
        # "Set Aiming Beam Current\n(You can make a copy of, or modify, this frame)"
        n1206 = Unbundle By Name(w2594) -> ("AB Cluster.Aiming Beam COM Port"=w2587:refnum<visa-resource-name>)
        n1207 = Number To Fractional String(number="488nm Power", precision (6)=i16 2) -> (F-format string=w2588:string)  [unwired: 2 in]
        n1208 = Concatenate Strings("slc:", w2588, "\r" ("Carriage Return Constant"), "\n" ("Line Feed Constant")) -> (w2591:string)
        n1209 = VISA Write(VISA resource name=w2587, write buffer=w2591, error in (no error)=w2585) -> (error out=w2586:errorcluster)  [unwired: 2 out]
        n1210 = call <vilib>:"Add State(s) to Queue__JKI_lib_State_Machine.vi"("State(s) in (\"\")"=w2596) -> ("States Out"=w2595:string)  [unwired: 14 in]
      }
      frame "AimingBeam: Set ACC Status" {
        # "Enable Aiming Beam\n(Usage: \"AimingBeam: Set >> Enable|Disable\")"
        n1211 = Unbundle By Name(w2603) -> ("AB Cluster.Aiming Beam COM Port"=w2600:refnum<visa-resource-name>)
        n1212 = case shown="\"Enable\"" w2602 {
          tunnel: [w2606 w2610] -> w2601
          frame "Disable", Default {
            n1213 = Concatenate Strings("cof", "\r" ("Carriage Return Constant"), "\n" ("Line Feed Constant")) -> (w2606:string)
          }
          frame "Enable" {
            n1214 = Concatenate Strings("con", "\r" ("Carriage Return Constant"), "\n" ("Line Feed Constant")) -> (w2610:string)
          }
        }
        n1215 = VISA Write(VISA resource name=w2600, write buffer=w2601, error in (no error)=w2598) -> (error out=w2599:errorcluster)  [unwired: 2 out]
        n1216 = call <vilib>:"Add State(s) to Queue__JKI_lib_State_Machine.vi"("State(s) in (\"\")"=w2605) -> ("States Out"=w2604:string)  [unwired: 14 in]
      }
      frame "AimingBeam: Set APC Status" {
        # "Enable Aiming Beam\n(Usage: \"AimingBeam: Set >> Enable|Disable\")"
        n1217 = Unbundle By Name(w2620) -> ("AB Cluster.Aiming Beam COM Port"=w2617:refnum<visa-resource-name>)
        n1218 = case shown="\"Disable\", Default" w2619 {
          tunnel: [w2623 w2627] -> w2618
          frame "Disable", Default {
            n1219 = Concatenate Strings("lof", "\r" ("Carriage Return Constant"), "\n" ("Line Feed Constant")) -> (w2623:string)
          }
          frame "Enable" {
            n1220 = Concatenate Strings("lon", "\r" ("Carriage Return Constant"), "\n" ("Line Feed Constant")) -> (w2627:string)
          }
        }
        n1221 = VISA Write(VISA resource name=w2617, write buffer=w2618, error in (no error)=w2615) -> (error out=w2616:errorcluster)  [unwired: 2 out]
        n1222 = call <vilib>:"Add State(s) to Queue__JKI_lib_State_Machine.vi"("State(s) in (\"\")"=w2622) -> ("States Out"=w2621:string)  [unwired: 14 in]
      }
      frame "AimingBeam: GetPWMStatus" {
        # "Get aiming beam PWM status\n()"
        n1223 = Unbundle By Name(w2635) -> ("AB Cluster.Freq"=w2634:i32, "LJ Pinout.AimingBeam PWM"=w2641:string)
        n1224 = Equal To 0?(x=w2634) -> (x = 0?=w2633:bool)
        n1225 = call "LabJack_FGV.vi"("Operation(Read)"=enum16{"Write", "Read"}."Read" ("Operation"), "error in (no error)"=w2637) -> ("error out"=w2639:errorcluster, "Read data"=w2640:i32)  [unwired: 8 in]
        n1226 = case shown="True" w2633 {
          tunnel: w2641 -> [w2654 _]
          tunnel: [w2652 "DIO_STATE"] -> w2638
          frame False {
            n1227 = Concatenate Strings(w2654, "_EF_ENABLE" ("string")) -> (w2652:string)
          }
          frame True {
          }
        }
        n1228 = call "LJM_eReadName.vi"("Handle In"=w2640, "Name"=w2638, "error in"=w2639) -> ("Value"=w2632:dbl, "error out"=w2636:errorcluster)  [unwired: 10 in, 1 out]
        n1229 = case shown="True" w2633 {
          tunnel: w2632 -> [w2647 w2651]
          tunnel: [w2646 w2648] -> w2631
          frame False {
            n1230 = Greater Than 0?(x=w2647) -> (x > 0?=w2646:bool)
          }
          frame True {
            n1231 = Number To Boolean Array(number=w2651) -> (Boolean array=w2650:bool[])
            n1232 = Index Array(array=w2650, index=3) -> (element=w2648:bool)
          }
        }
        n1233 = case shown="False" w2631 {
          frame False {
            # "PWM is off\nset color to dark green"
            n1234 = local write "Aiming beam toggle"(FALSE ("Aimging beam")) -> ()
          }
          frame True {
            # "PWM is on\nset color to light green"
            n1235 = local write "Aiming beam toggle"(TRUE ("Aimging beam")) -> ()
          }
        }
        n1236 = call <vilib>:"Add State(s) to Queue__JKI_lib_State_Machine.vi"("State(s) in (\"\")"=w2645) -> ("States Out"=w2644:string)  [unwired: 14 in]
      }
      frame "---------- 355 Laser ----------" {
        # "Template Separator\n(You can make a copy of, or modify, this frame)"
        n1237 = call <vilib>:"Add State(s) to Queue__JKI_lib_State_Machine.vi"("State(s) in (\"\")"=w2662) -> ("States Out"=w2661:string)  [unwired: 14 in]
      }
      frame "355 Laser: Check Dewelling" {
        # "if time laser start time is less than 7.5s before, wait 250ms then check again."
        # "Template Separator\n(You can make a copy of, or modify, this frame)"
        n1238 = Unbundle By Name(w2670) -> ("Laser start tic"=w2667:u32)
        n1239 = Tick Count (ms)() -> (millisecond timer value=w2668:u32)
        n1240 = Subtract(x=w2668, y=w2667) -> (x-y=w2666:u32)
        n1241 = Greater?(x=w2666, y=u32 5000) -> (0:w2664:bool)
        n1242 = case shown="False" w2664 {
          tunnel: ["355 Laser: Check Dewelling" ""] -> w2663
          frame False {
            n1243 = Wait (ms)(milliseconds to wait=u32 250) -> ()  [unwired: 1 out]
          }
          frame True {
          }
        }
        n1244 = call <vilib>:"Add State(s) to Queue__JKI_lib_State_Machine.vi"("State(s) in Front (\"\")"=w2663, "State(s) in (\"\")"=w2673) -> ("States Out"=w2672:string)  [unwired: 13 in]
      }
      frame "355 Laser: Laser enable" {
        # "Laser enable/disable\n(Usage: \"LabJack: Laser enable/disable >> 1|0\")"
        n1245 = Unbundle By Name(w2680) -> ("LJ Pinout.Laser Start/Stop"=w2684:string, "System Status.355 Laser"=w2678:bool)
        n1246 = case shown="False" w2678 {
          tunnel: w2677 -> [w2699 w2700]
          tunnel: w2684 -> [w2693 _]
          tunnel: [w2688 w2700] -> w2682
          tunnel: [w2687 u32 0 ("millisecond timer value")] -> w2679
          frame False {
            n1247 = call "LabJack_FGV.vi"("Operation(Read)"=enum16{"Write", "Read"}."Read" ("Operation")) -> ("Read data"=w2695:i32)  [unwired: 9 in, 1 out]
            n1248 = call "LJM_eWriteName.vi"("Handle In"=w2695, "Name"=w2693, "Value"=1.0, "error in"=w2699) -> ("Handle Out"=w2694:i32, "error out"=w2692:errorcluster)  [unwired: 10 in]
            n1249 = call <userlib>:"Wait (ms)__ogtk.vi"("error in (no error)"=w2692, "milliseconds to wait"=u32 250) -> ("error out"=w2691:errorcluster)  [unwired: 8 in, 1 out]
            n1250 = call "LJM_eWriteName.vi"("Handle In"=w2694, "Name"=w2693, "Value"=0.0, "error in"=w2691) -> ("error out"=w2689:errorcluster)  [unwired: 10 in, 1 out]
            n1251 = call <userlib>:"Tick Count (ms)__ogtk.vi"("error in (no error)"=w2689) -> ("error out"=w2688:errorcluster, "millisecond timer value"=w2687:u32)  [unwired: 9 in]
          }
          frame True {
          }
        }
        n1252 = Bundle By Name(cluster=w2680, "Laser start tic"=w2679) -> (w2681:T24)
        n1253 = call <vilib>:"Add State(s) to Queue__JKI_lib_State_Machine.vi"("State(s) in (\"\")"=w2686) -> ("States Out"=w2685:string)  [unwired: 14 in]
      }
      frame "355 Laser: Laser disable" {
        # "Laser enable/disable\n(Usage: \"LabJack: Laser enable/disable >> 1|0\")"
        n1254 = Unbundle By Name(w2704) -> ("LJ Pinout.Laser Start/Stop"=w2708:string, "System Status.355 Laser"=w2702:bool)
        n1255 = case shown="True" w2702 {
          tunnel: w2709 -> [w2712 w2726]
          tunnel: w2708 -> [_ w2720]
          tunnel: [w2712 w2715] -> w2706
          tunnel: [u32 0 ("millisecond timer value") w2714] -> w2703
          frame False {
          }
          frame True {
            n1256 = call "LabJack_FGV.vi"("Operation(Read)"=enum16{"Write", "Read"}."Read" ("Operation")) -> ("Read data"=w2722:i32)  [unwired: 9 in, 1 out]
            n1257 = call "LJM_eWriteName.vi"("Handle In"=w2722, "Name"=w2720, "Value"=1.0, "error in"=w2726) -> ("Handle Out"=w2721:i32, "error out"=w2719:errorcluster)  [unwired: 10 in]
            n1258 = call <userlib>:"Wait (ms)__ogtk.vi"("error in (no error)"=w2719, "milliseconds to wait"=u32 250) -> ("error out"=w2718:errorcluster)  [unwired: 8 in, 1 out]
            n1259 = call "LJM_eWriteName.vi"("Handle In"=w2721, "Name"=w2720, "Value"=0.0, "error in"=w2718) -> ("error out"=w2716:errorcluster)  [unwired: 10 in, 1 out]
            n1260 = call <userlib>:"Tick Count (ms)__ogtk.vi"("error in (no error)"=w2716) -> ("error out"=w2715:errorcluster, "millisecond timer value"=w2714:u32)  [unwired: 9 in]
          }
        }
        n1261 = Bundle By Name(cluster=w2704, "Laser start tic"=w2703) -> (w2705:T24)
        n1262 = call <vilib>:"Add State(s) to Queue__JKI_lib_State_Machine.vi"("State(s) in (\"\")"=w2711) -> ("States Out"=w2710:string)  [unwired: 14 in]
      }
      frame "355 Laser: Dewelling" {
        # "Wait some time (ms)\n(355 Laser: Dewelling >> #)"
        n1263 = Fract/Exp String To Number(string=w2730, default (0 dbl)=0) -> (number=w2728:i32)  [unwired: 2 in, 1 out]
        n1264 = Wait (ms)(milliseconds to wait=w2728) -> ()  [unwired: 1 out]
        n1265 = call <vilib>:"Add State(s) to Queue__JKI_lib_State_Machine.vi"("State(s) in (\"\")"=w2734) -> ("States Out"=w2733:string)  [unwired: 14 in]
      }
      frame "355 Laser: Close" {
        # "Template Separator\n(You can make a copy of, or modify, this frame)"
        n1266 = call <vilib>:"Add State(s) to Queue__JKI_lib_State_Machine.vi"("State(s) in Front (\"\")"="355 Laser: CheckControllerStatus\n355 Laser: Laser disable\n355 Laser: Dewelling >>1000", "State(s) in (\"\")"=w2740) -> ("States Out"=w2739:string)  [unwired: 13 in]
      }
      frame "355 Laser: CheckControllerStatus" {
        # "if average < 2, laser no power\nif average 2 < average < 9.3, laser on\nif 9.3<average<10, interlock open, blink indicator\nif average > 10, laser off\n[Covers: REQ30]"
        # "take 10 measuremt and look at average"
        # "Check 355 laser controller status\nBy probing Emisison Lamp negative terminal voltage"
        n1267 = Unbundle By Name(w2749) -> ("LJ Pinout.Laser Ready"=w2752:string)
        n1268 = call "LabJack_FGV.vi"("Operation(Read)"=enum16{"Write", "Read"}."Read" ("Operation")) -> ("Read data"=w2753:i32)  [unwired: 9 in, 1 out]
        n1269 = for {
          N: 20 -> [_]
          tunnel: w2753 -> [w2764]
          tunnel: w2752 -> [w2763]
          shift-right: [w2762] -> w2745
          shift-left: w2751 -> [w2761]
          tunnel: [w2759] -> w2744 mode=indexing
          n1270 = call "LJM_eReadName.vi"("Handle In"=w2764, "Name"=w2763, "error in"=w2761) -> ("Value"=w2759:dbl, "error out"=w2762:errorcluster)  [unwired: 10 in, 1 out]
          n1271 = Wait (ms)(milliseconds to wait=u32 25) -> ()  [unwired: 1 out]
        }
        n1272 = call "checkLaserStatus.vi"("error in (no error)"=w2745, "Laser LED voltage"=w2744) -> ("error out"=w2746:errorcluster, "Interlock open?"=w2741:bool, "Laser on?"=w2743:bool, "Mean voltage"=→"laser EM lamp V":dbl)  [unwired: 6 in]
        n1273 = Bundle By Name(cluster=w2749, "System Status.355 Laser"=w2743) -> (w2750:T24)
        n1274 = case shown="True" w2741 {
          frame False {
            n1275 = property on="355 Laser" class="Bool (strict)"("Blinking"=FALSE) -> ()  [unwired: 2 in, 2 out]
          }
          frame True {
            n1276 = property on="355 Laser" class="Bool (strict)"("Blinking"=TRUE) -> ()  [unwired: 2 in, 2 out]
          }
        }
        n1277 = call <vilib>:"Add State(s) to Queue__JKI_lib_State_Machine.vi"("State(s) in (\"\")"=w2756) -> ("States Out"=w2755:string)  [unwired: 14 in]
      }
      frame "355 Laser: CheckPWMStatus" {
        # "Check 355 laser PWM status\n(Read LJ DIO#EF_ENABLE register to determine PWM status)"
        n1278 = Unbundle By Name(w2774) -> ("LJ Pinout.355 PWM"=w2773:string)
        n1279 = call "LabJack_FGV.vi"("Operation(Read)"=enum16{"Write", "Read"}."Read" ("Operation"), "error in (no error)"=w2767) -> ("error out"=w2770:errorcluster, "Read data"=w2771:i32)  [unwired: 8 in]
        n1280 = Concatenate Strings(w2773, "_EF_ENABLE" ("string")) -> (w2769:string)
        n1281 = call "LJM_eReadName.vi"("Handle In"=w2771, "Name"=w2769, "error in"=w2770) -> ("Value"=w2766:dbl, "error out"=w2768:errorcluster)  [unwired: 10 in, 1 out]
        n1282 = Greater Than 0?(x=w2766) -> (x > 0?=w2765:bool)
        n1283 = case shown="False" w2765 {
          frame False {
            # "PWM is off\nset color to gray"
            n1284 = local write "355nm Laser toggle"(FALSE ("355nm Laser")) -> ()
          }
          frame True {
            # "PWM is on\nset color to light green"
            n1285 = local write "355nm Laser toggle"(TRUE ("355nm Laser")) -> ()
          }
        }
        n1286 = call <vilib>:"Add State(s) to Queue__JKI_lib_State_Machine.vi"("State(s) in (\"\")"=w2778) -> ("States Out"=w2777:string)  [unwired: 14 in]
      }
      frame "355 Laser: Start" {
        # "Template Separator\n(You can make a copy of, or modify, this frame)"
        n1287 = call <vilib>:"Add State(s) to Queue__JKI_lib_State_Machine.vi"("State(s) in Front (\"\")"="LabJack: 355_PWM_Start", "State(s) in (\"\")"=w2786) -> ("States Out"=w2785:string)  [unwired: 13 in]
      }
      frame "355 Laser: Stop" {
        # "Template Separator\n(You can make a copy of, or modify, this frame)"
        n1288 = call <vilib>:"Add State(s) to Queue__JKI_lib_State_Machine.vi"("State(s) in Front (\"\")"="LabJack: 355_PWM_Stop", "State(s) in (\"\")"=w2792) -> ("States Out"=w2791:string)  [unwired: 13 in]
      }
      frame "---------- Utility ----------" {
        # "Template Separator\n(You can make a copy of, or modify, this frame)"
        n1289 = call <vilib>:"Add State(s) to Queue__JKI_lib_State_Machine.vi"("State(s) in (\"\")"=w2797) -> ("States Out"=w2796:string)  [unwired: 14 in]
      }
      frame "Utility: SetDataClass" {
        # "Set Data Class in Queues\n(Set data class to either Data, Bg or Cali)"
        n1290 = case shown="\"Cali\"" w2799 {
          tunnel: [enum16{"Data", "BG", "Cali"}."Data" ("Data Class") enum16{"Data", "BG", "Cali"}."BG" ("Data Class") enum16{"Data", "BG", "Cali"}."Cali" ("Data Class")] -> w2798
          frame "Data", Default {
          }
          frame "Bg" {
          }
          frame "Cali" {
          }
        }
        n1291 = local write "Data Class"(w2798) -> ()
        n1292 = call <vilib>:"Add State(s) to Queue__JKI_lib_State_Machine.vi"("State(s) in (\"\")"=w2804) -> ("States Out"=w2803:string)  [unwired: 14 in]
      }
      frame "Utility: AquiTimerReset" {
        # "Set Aquisition Timer\n(You can make a copy of, or modify, this frame)"
        n1293 = Tick Count (ms)() -> (millisecond timer value=w2810:u32)
        n1294 = Bundle By Name(cluster=w2808, "Aquisition Timer"=w2810) -> (w2809:T24)
        n1295 = call <vilib>:"Add State(s) to Queue__JKI_lib_State_Machine.vi"("State(s) in (\"\")"=w2814) -> ("States Out"=w2813:string)  [unwired: 14 in]
      }
      frame "Utility: AquiTimerCheck" {
        # "5min to ms"
        # "Set Aquisition Timer\n([Covers: REQ35])"
        n1296 = Unbundle By Name(w2822) -> ("Aquisition Timer"=w2820:u32)
        n1297 = Tick Count (ms)() -> (millisecond timer value=w2821:u32)
        n1298 = Subtract(x=w2821, y=w2820) -> (x-y=w2819:u32)
        n1299 = Multiply(x=1000, y=300) -> (x*y=w2816:i32)
        n1300 = Greater Or Equal?(x=w2819, y=w2816) -> (x >= y?=w2815:bool)
        n1301 = case shown="True" w2815 {
          frame False {
            # "do nothing"
          }
          frame True {
            # "if timed out, stop aquisition"
            n1302 = property on="StopButton" class="Bool (strict)"("Val(Sgnl)"=TRUE ("Value (Signaling)")) -> ()  [unwired: 2 in, 2 out]
          }
        }
        n1303 = call <vilib>:"Add State(s) to Queue__JKI_lib_State_Machine.vi"("State(s) in (\"\")"=w2826) -> ("States Out"=w2825:string)  [unwired: 14 in]
      }
      frame "Utility: StartBeep" {
        # "Beep\n([Covers: REQ18])"
        n1304 = call <vilib>:"Beep.vi"("use system alert? (T)"=FALSE, "duration (msec)"=u32 1000, "frequency (Hz)"=u32 2000) -> ()  [unwired: 9 in]
        n1305 = call <vilib>:"Add State(s) to Queue__JKI_lib_State_Machine.vi"("State(s) in (\"\")"=w2835) -> ("States Out"=w2834:string)  [unwired: 14 in]
      }
      frame "Utility: EndBeep" {
        # "Beep\n([Covers: REQ18])"
        n1306 = flat-sequence {
          frame #0 {
            n1307 = call <vilib>:"Beep.vi"("use system alert? (T)"=FALSE, "duration (msec)"=u32 500, "frequency (Hz)"=u32 2000) -> ()  [unwired: 9 in]
          }
          frame #1 {
            n1308 = call <vilib>:"Beep.vi"("use system alert? (T)"=FALSE, "duration (msec)"=u32 500, "frequency (Hz)"=u32 2000) -> ()  [unwired: 9 in]
          }
        }
        n1309 = call <vilib>:"Add State(s) to Queue__JKI_lib_State_Machine.vi"("State(s) in (\"\")"=w2840) -> ("States Out"=w2839:string)  [unwired: 14 in]
      }
      frame "Utility: RestoreDeConChan" {
        # "Template Separator\n(You can make a copy of, or modify, this frame)"
        n1310 = global read "GlobalVariables.vi" "DeconChan Temp"() -> (w2847:T10)
        n1311 = local write "Radio Buttons"(w2847) -> ()
        n1312 = call <vilib>:"Add State(s) to Queue__JKI_lib_State_Machine.vi"("State(s) in (\"\")"=w2852) -> ("States Out"=w2851:string)  [unwired: 14 in]
      }
      frame "Utility: SaveDeconChan" {
        # "Save Decon Channel to global temp\n(You can make a copy of, or modify, this frame)"
        n1313 = flat-sequence {
          frame #0 {
            n1314 = local read "Radio Buttons"() -> (w2858:T10)
            n1315 = global write "GlobalVariables.vi" "DeconChan Temp"(w2858) -> ()
          }
          frame #1 {
            n1316 = local write "Radio Buttons"(T10."No Selection" ("Radio Buttons")) -> ()
          }
        }
        n1317 = flat-sequence {
          frame #0 {
          }
          frame #1 {
            (unwired) enum32{"No Selection", "Ch1", "Ch2", "Ch3"}."No Selection" ("Radio Buttons")
          }
        }
        n1318 = call <vilib>:"Add State(s) to Queue__JKI_lib_State_Machine.vi"("State(s) in (\"\")"=w2857) -> ("States Out"=w2856:string)  [unwired: 14 in]
      }
      frame "Utility: Dewelling" {
        # "Main loop dewell\n(Dewelling >> #)"
        n1319 = Fract/Exp String To Number(string=w2863, default (0 dbl)=0) -> (number=w2861:i32)  [unwired: 2 in, 1 out]
        n1320 = Wait (ms)(milliseconds to wait=w2861) -> ()  [unwired: 1 out]
        n1321 = call <vilib>:"Add State(s) to Queue__JKI_lib_State_Machine.vi"("State(s) in (\"\")"=w2867) -> ("States Out"=w2866:string)  [unwired: 14 in]
      }
      frame "Utility: SetAllChanManualGain" {
        w2868 = FALSE ("Value (Signaling)")
        # "Set all channel to manual gain\n(You can make a copy of, or modify, this frame)"
        n1322 = property on="Auto gain ch1" class="Bool (strict)"("Val(Sgnl)"=w2868) -> ()  [unwired: 2 in, 2 out]
        n1323 = property on="Auto gain ch2" class="Bool (strict)"("Val(Sgnl)"=w2868) -> ()  [unwired: 2 in, 2 out]
        n1324 = property on="Auto gain ch3" class="Bool (strict)"("Val(Sgnl)"=w2868) -> ()  [unwired: 2 in, 2 out]
        n1325 = property on="Auto gain ch4" class="Bool (strict)"("Val(Sgnl)"=w2868) -> ()  [unwired: 2 in, 2 out]
        n1326 = call <vilib>:"Add State(s) to Queue__JKI_lib_State_Machine.vi"("State(s) in (\"\")"=w2873) -> ("States Out"=w2872:string)  [unwired: 14 in]
      }
      frame "Utility: SetAllChanAutoGain" {
        w2874 = TRUE ("Value (Signaling)")
        # "Set all channels to auto gain\n(You can make a copy of, or modify, this frame)"
        n1327 = property on="Auto gain ch1" class="Bool (strict)"("Val(Sgnl)"=w2874) -> ()  [unwired: 2 in, 2 out]
        n1328 = property on="Auto gain ch2" class="Bool (strict)"("Val(Sgnl)"=w2874) -> ()  [unwired: 2 in, 2 out]
        n1329 = property on="Auto gain ch3" class="Bool (strict)"("Val(Sgnl)"=w2874) -> ()  [unwired: 2 in, 2 out]
        n1330 = property on="Auto gain ch4" class="Bool (strict)"("Val(Sgnl)"=w2874) -> ()  [unwired: 2 in, 2 out]
        n1331 = call <vilib>:"Add State(s) to Queue__JKI_lib_State_Machine.vi"("State(s) in (\"\")"=w2879) -> ("States Out"=w2878:string)  [unwired: 14 in]
      }
      frame "---------- SysLog ----------" {
        # "Template Separator\n(You can make a copy of, or modify, this frame)"
        n1332 = call <vilib>:"Add State(s) to Queue__JKI_lib_State_Machine.vi"("State(s) in (\"\")"=w2884) -> ("States Out"=w2883:string)  [unwired: 14 in]
      }
      frame "SysLog: OpenLogFile" {
        # "Template Separator\n(You can make a copy of, or modify, this frame)"
        n1333 = call <vilib>:"Add State(s) to Queue__JKI_lib_State_Machine.vi"("State(s) in (\"\")"=w2889) -> ("States Out"=w2888:string)  [unwired: 14 in]
      }
      frame "---------- Graph ----------" {
        # "Template Separator\n(You can make a copy of, or modify, this frame)"
        n1334 = call <vilib>:"Add State(s) to Queue__JKI_lib_State_Machine.vi"("State(s) in (\"\")"=w2894) -> ("States Out"=w2893:string)  [unwired: 14 in]
      }
      frame "Graph: SetXMultiplier" {
        # "Set X multiplier of WF graphs\n(You can make a copy of, or modify, this frame)"
        n1335 = call "Digitizer1_FGV.vi"() -> ("error out"=w2898:errorcluster, "Read data"=w2899:refnum<k15>)  [unwired: 10 in]
        n1336 = property class="niScope"(reference=w2899, error in=w2898) -> ("Min Sample Rate"=w2897:dbl)  [unwired: 2 out]
        n1337 = Divide(x=1.0, y=w2897) -> (x/y=w2895:dbl)
        n1338 = property on="Channel 1" class="WFGraph (strict)"("XScale.Multiplier"=w2895) -> ()  [unwired: 2 in, 2 out]
        n1339 = property on="Channel 2" class="WFGraph (strict)"("XScale.Multiplier"=w2895) -> ()  [unwired: 2 in, 2 out]
        n1340 = property on="Channel 3" class="WFGraph (strict)"("XScale.Multiplier"=w2895) -> ()  [unwired: 2 in, 2 out]
        n1341 = property on="Channel 4" class="WFGraph (strict)"("XScale.Multiplier"=w2895) -> ()  [unwired: 2 in, 2 out]
        n1342 = call <vilib>:"Add State(s) to Queue__JKI_lib_State_Machine.vi"("State(s) in (\"\")"=w2904) -> ("States Out"=w2903:string)  [unwired: 14 in]
      }
      frame "Graph: AddCursors" {
        # "Add BG and DC cursor to all graphs\n(You can make a copy of, or modify, this frame)"
        n1343 = property on="Channel 1" class="WFGraph (strict)"() -> ("XScale.Multiplier"=w2913:dbl)  [unwired: 2 in, 2 out]
        n1344 = global read "GlobalVariables.vi" "DC Idx1"() -> (w2912:i32)
        n1345 = global read "GlobalVariables.vi" "DC Idx2"() -> (w2911:i32)
        n1346 = global read "GlobalVariables.vi" "BG Idx1"() -> (w2910:i32)
        n1347 = global read "GlobalVariables.vi" "BG Idx2"() -> (w2909:i32)
        n1348 = property on="Channel 1" class="WFGraph (strict)"(error in=w2915) -> ("CrsrList"=w2924:T25)  [unwired: 1 in, 2 out]
        n1349 = property on="Channel 2" class="WFGraph (strict)"() -> ("CrsrList"=w2921:T25)  [unwired: 2 in, 2 out]
        n1350 = property on="Channel 3" class="WFGraph (strict)"() -> ("CrsrList"=w2920:T25)  [unwired: 2 in, 2 out]
        n1351 = property on="Channel 4" class="WFGraph (strict)"() -> ("CrsrList"=w2906:T25)  [unwired: 2 in, 2 out]
        n1352 = Build Array(w2912, w2911, w2910, w2909) -> (w2908:i32[])
        n1353 = Multiply(x=w2908, y=w2913) -> (x*y=w2907:dbl[])
        n1354 = for {
          tunnel: w2924 -> [w2938] mode=indexing
          tunnel: w2907 -> [w2931] mode=indexing
          tunnel: [w2937] -> w2923 mode=indexing
          tunnel: u32[] [6618880, 6618880, 16711680, 16711680] -> [w2930] mode=indexing
          tunnel: w2921 -> [w2936] mode=indexing
          tunnel: w2920 -> [w2935] mode=indexing
          tunnel: [w2934] -> w2919 mode=indexing
          tunnel: [w2933] -> w2918 mode=indexing
          tunnel: w2906 -> [w2932] mode=indexing
          tunnel: [w2929] -> w2905 mode=indexing
          n1355 = Bundle By Name(cluster=w2938, "Position.X"=w2931, "Color"=w2930) -> (w2937:T26)
          n1356 = Bundle By Name(cluster=w2936, "Position.X"=w2931, "Color"=w2930) -> (w2934:T26)
          n1357 = Bundle By Name(cluster=w2935, "Position.X"=w2931, "Color"=w2930) -> (w2933:T26)
          n1358 = Bundle By Name(cluster=w2932, "Position.X"=w2931, "Color"=w2930) -> (w2929:T26)
        }
        n1359 = property on="Channel 1" class="WFGraph (strict)"("CrsrList"=w2923) -> (error out=w2914:errorcluster)  [unwired: 2 in, 1 out]
        n1360 = property on="Channel 2" class="WFGraph (strict)"("CrsrList"=w2919) -> ()  [unwired: 2 in, 2 out]
        n1361 = property on="Channel 3" class="WFGraph (strict)"("CrsrList"=w2918) -> ()  [unwired: 2 in, 2 out]
        n1362 = property on="Channel 4" class="WFGraph (strict)"("CrsrList"=w2905) -> ()  [unwired: 2 in, 2 out]
        n1363 = control-ref of="Channel 1"() -> (w2917:refnum<vi>)
        n1364 = call <vilib>:"Add State(s) to Queue__JKI_lib_State_Machine.vi"("State(s) in (\"\")"=w2928) -> ("States Out"=w2927:string)  [unwired: 14 in]
        n1365 = call "UpdateCurserIdx(SubVI).vi"("error in (no error)"=w2914, "WaveformGraph in"=w2917) -> ("error out"=w2916:errorcluster)  [unwired: 9 in]
      }
      frame "Graph: SaveCursorLoc" {
        # "Save cursor location to ini file\n(Save cursor location to system setting ini file)"
        n1366 = global read "GlobalVariables.vi" "DC Idx1"() -> (w2945:i32)
        n1367 = global read "GlobalVariables.vi" "DC Idx2"() -> (w2944:i32)
        n1368 = global read "GlobalVariables.vi" "BG Idx1"() -> (w2943:i32)
        n1369 = global read "GlobalVariables.vi" "BG Idx2"() -> (w2942:i32)
        n1370 = Bundle("DC Idx1"=w2945, "DC Idx2"=w2944, "BG Idx1"=w2943, "BG Idx2"=w2942) -> (w2941:T49)  [unwired: 1 in]
        n1371 = call "writeCursorConfigMain.vi"("error in (no error)"=w2939, "Cursor Locations"=w2941) -> ("error out"=w2940:errorcluster)  [unwired: 9 in]
        n1372 = call <vilib>:"Add State(s) to Queue__JKI_lib_State_Machine.vi"("State(s) in (\"\")"=w2949) -> ("States Out"=w2948:string)  [unwired: 14 in]
      }
      frame "---------- APD ----------" {
        # "Template Separator\n(You can make a copy of, or modify, this frame)"
        n1373 = call <vilib>:"Add State(s) to Queue__JKI_lib_State_Machine.vi"("State(s) in (\"\")"=w2954) -> ("States Out"=w2953:string)  [unwired: 14 in]
      }
      frame "APD: Initialize" {
        w2961 = enum16{"Read", "Write"}."Write" ("Operation (Read)")
        w2960 = refnum<class "APDClass.lvclass"> refnum  # APDClass.lvclass
        # "Initialize APD FGV\n(Initialized APD FGV for holding data)"
        n1374 = call "APD1FGV.vi"("Error In"=w2955, "Operation (Read)"=w2961, "APDClass in"=w2960) -> ("Error Out"=w2959:errorcluster)  [unwired: 7 in, 1 out]
        n1375 = call "APD2FGV.vi"("Error In"=w2955, "Operation (Read)"=w2961, "APDClass in"=w2960) -> ("Error Out"=w2958:errorcluster)  [unwired: 7 in, 1 out]
        n1376 = call "APD3FGV.vi"("Error In"=w2955, "Operation (Read)"=w2961, "APDClass in"=w2960) -> ("Error Out"=w2957:errorcluster)  [unwired: 7 in, 1 out]
        n1377 = Merge Errors(w2959, w2958, w2957) -> (w2956:errorcluster)
        n1378 = call <vilib>:"Add State(s) to Queue__JKI_lib_State_Machine.vi"("State(s) in (\"\")"=w2965) -> ("States Out"=w2964:string)  [unwired: 14 in]
      }
      frame "APD: LoadFromSerial" {
        w2967 = enum16{"Read", "Write"}."Write" ("Operation (Read)")
        # "Load APD data from tdms file\n(load and update FGV)"
        n1379 = call "readAPDSerial.vi"("Error In"=w2974) -> ("Error Out"=w2970:errorcluster, "output cluster"=w2973:T27)  [unwired: 9 in]
        n1380 = Unbundle By Name(w2973) -> ("Ch1APDSerial#"=w2986:string, "Ch2APDSerial#"=w2972:string, "Ch3APDSerial#"=w2985:string, "Ch4APDSerial#"=w2971:string)
        n1381 = call "CreatFromSerialNumNoRaw.vi"("error in (no error)"=w2970, "APD Serial #"=w2986) -> ("error out"=w2983:errorcluster, "APDClass out"=w2984:refnum<class "APDClass.lvclass">)  [unwired: 8 in]
        n1382 = call "CreatFromSerialNumNoRaw.vi"("error in (no error)"=w2970, "APD Serial #"=w2972) -> ("error out"=w2981:errorcluster, "APDClass out"=w2982:refnum<class "APDClass.lvclass">)  [unwired: 8 in]
        n1383 = call "CreatFromSerialNumNoRaw.vi"("error in (no error)"=w2970, "APD Serial #"=w2985) -> ("error out"=w2979:errorcluster, "APDClass out"=w2980:refnum<class "APDClass.lvclass">)  [unwired: 8 in]
        n1384 = call "CreatFromSerialNumNoRaw.vi"("error in (no error)"=w2970, "APD Serial #"=w2971) -> ("error out"=w2968:errorcluster, "APDClass out"=w2969:refnum<class "APDClass.lvclass">)  [unwired: 8 in]
        n1385 = call "APD1FGV.vi"("Error In"=w2983, "Operation (Read)"=w2967, "APDClass in"=w2984) -> ("Error Out"=w2978:errorcluster)  [unwired: 7 in, 1 out]
        n1386 = call "APD2FGV.vi"("Error In"=w2981, "Operation (Read)"=w2967, "APDClass in"=w2982) -> ("Error Out"=w2976:errorcluster)  [unwired: 7 in, 1 out]
        n1387 = call "APD3FGV.vi"("Error In"=w2979, "Operation (Read)"=w2967, "APDClass in"=w2980) -> ("Error Out"=w2977:errorcluster)  [unwired: 7 in, 1 out]
        n1388 = call "APD4FGV.vi"("Error In"=w2968, "Operation (Read)"=w2967, "APDClass in"=w2969) -> ("Error Out"=w2966:errorcluster)  [unwired: 7 in, 1 out]
        n1389 = Merge Errors(w2978, w2976, w2977, w2966) -> (w2975:errorcluster)
        n1390 = call <vilib>:"Add State(s) to Queue__JKI_lib_State_Machine.vi"("State(s) in (\"\")"=w2990) -> ("States Out"=w2989:string)  [unwired: 14 in]
      }
      frame "APD: UpdateCtrlVLimit" {
        w2996 = enum16{"Read", "Write"}."Read" ("Operation (Read)")
        # "Set V limit\n(You can make a copy of, or modify, this frame)"
        n1391 = call "APD1FGV.vi"("Error In"=w2997, "Operation (Read)"=w2996) -> ("Error Out"=w3012:errorcluster, "APDClass out"=w3013:refnum<class "APDClass.lvclass">)  [unwired: 8 in]
        n1392 = call "APD2FGV.vi"("Error In"=w2997, "Operation (Read)"=w2996) -> ("Error Out"=w3010:errorcluster, "APDClass out"=w3011:refnum<class "APDClass.lvclass">)  [unwired: 8 in]
        n1393 = call "APD3FGV.vi"("Error In"=w2997, "Operation (Read)"=w2996) -> ("Error Out"=w3008:errorcluster, "APDClass out"=w3009:refnum<class "APDClass.lvclass">)  [unwired: 8 in]
        n1394 = call "APD4FGV.vi"("Error In"=w2997, "Operation (Read)"=w2996) -> ("Error Out"=w2994:errorcluster, "APDClass out"=w2995:refnum<class "APDClass.lvclass">)  [unwired: 8 in]
        n1395 = call-dynamic "ReadMaxCtrlV.vi"("error in (no error)"=w3012, "APDClass in"=w3013) -> ("error out"=w3003:errorcluster, "Numeric"=w3006:dbl)  [unwired: 7 in, 1 out]
        n1396 = call-dynamic "ReadMaxCtrlV.vi"("error in (no error)"=w3010, "APDClass in"=w3011) -> ("error out"=w3001:errorcluster, "Numeric"=w3005:dbl)  [unwired: 7 in, 1 out]
        n1397 = call-dynamic "ReadMaxCtrlV.vi"("error in (no error)"=w3008, "APDClass in"=w3009) -> ("error out"=w2999:errorcluster, "Numeric"=w3004:dbl)  [unwired: 7 in, 1 out]
        n1398 = call-dynamic "ReadMaxCtrlV.vi"("error in (no error)"=w2994, "APDClass in"=w2995) -> ("error out"=w2992:errorcluster, "Numeric"=w2993:dbl)  [unwired: 7 in, 1 out]
        n1399 = property on="V 1" class="DigNum (strict)"(error in=w3003, "Maximum"=w3006) -> (error out=w3002:errorcluster)  [unwired: 1 in, 1 out]
        n1400 = property on="V 2" class="DigNum (strict)"(error in=w3001, "Maximum"=w3005) -> (error out=w3000:errorcluster)  [unwired: 1 in, 1 out]
        n1401 = property on="V 4" class="DigNum (strict)"(error in=w2992, "Maximum"=w2993) -> (error out=w2991:errorcluster)  [unwired: 1 in, 1 out]
        n1402 = property on="V 3" class="DigNum (strict)"(error in=w2999, "Maximum"=w3004) -> (error out=w2998:errorcluster)  [unwired: 1 in, 1 out]
        n1403 = Merge Errors(w3002, w3000, w2998, w2991) -> (w3007:errorcluster)
        n1404 = call <vilib>:"Add State(s) to Queue__JKI_lib_State_Machine.vi"("State(s) in (\"\")"=w3017) -> ("States Out"=w3016:string)  [unwired: 14 in]
      }
      frame "APD: GetGainLimits" {
        w3022 = enum16{"Read", "Write"}."Read" ("Operation (Read)")
        # "Template Separator\n(You can make a copy of, or modify, this frame)"
        n1405 = call "APD1FGV.vi"("Error In"=w3023, "Operation (Read)"=w3022) -> ("Error Out"=w3028:errorcluster, "APDClass out"=w3029:refnum<class "APDClass.lvclass">)  [unwired: 8 in]
        n1406 = call "APD2FGV.vi"("Error In"=w3023, "Operation (Read)"=w3022) -> ("Error Out"=w3035:errorcluster, "APDClass out"=w3036:refnum<class "APDClass.lvclass">)  [unwired: 8 in]
        n1407 = call "APD3FGV.vi"("Error In"=w3023, "Operation (Read)"=w3022) -> ("Error Out"=w3033:errorcluster, "APDClass out"=w3034:refnum<class "APDClass.lvclass">)  [unwired: 8 in]
        n1408 = call "APD4FGV.vi"("Error In"=w3023, "Operation (Read)"=w3022) -> ("Error Out"=w3020:errorcluster, "APDClass out"=w3021:refnum<class "APDClass.lvclass">)  [unwired: 8 in]
        n1409 = call-dynamic "Read Gain Limits(Log).vi"("error in (no error)"=w3028, "APDClass in"=w3029) -> ("error out"=w3027:errorcluster, "GainLimits(Log)"=w3024:cluster{"GainMax":dbl, "GainMin":dbl})  [unwired: 7 in, 1 out]
        n1410 = call-dynamic "Read Gain Limits(Log).vi"("error in (no error)"=w3035, "APDClass in"=w3036) -> ("error out"=w3031:errorcluster, "GainLimits(Log)"=w3026:cluster{"GainMax":dbl, "GainMin":dbl})  [unwired: 7 in, 1 out]
        n1411 = call-dynamic "Read Gain Limits(Log).vi"("error in (no error)"=w3033, "APDClass in"=w3034) -> ("error out"=w3030:errorcluster, "GainLimits(Log)"=w3025:cluster{"GainMax":dbl, "GainMin":dbl})  [unwired: 7 in, 1 out]
        n1412 = call-dynamic "Read Gain Limits(Log).vi"("error in (no error)"=w3020, "APDClass in"=w3021) -> ("error out"=w3018:errorcluster, "GainLimits(Log)"=w3019:cluster{"GainMax":dbl, "GainMin":dbl})  [unwired: 7 in, 1 out]
        n1413 = Merge Errors(w3027, w3031, w3030, w3018) -> (w3032:errorcluster)
        n1414 = global write "GlobalVariables.vi" "Ch1GainLim(Log)"(w3024) -> ()
        n1415 = global write "GlobalVariables.vi" "Ch2GainLim(Log)"(w3026) -> ()
        n1416 = global write "GlobalVariables.vi" "Ch3GainLim(Log)"(w3025) -> ()
        n1417 = global write "GlobalVariables.vi" "Ch4GainLim(Log)"(w3019) -> ()
        n1418 = call <vilib>:"Add State(s) to Queue__JKI_lib_State_Machine.vi"("State(s) in (\"\")"=w3040) -> ("States Out"=w3039:string)  [unwired: 14 in]
      }
      frame "---------- TCP ----------" {
        # "Template Separator\n(You can make a copy of, or modify, this frame)"
        n1419 = call <vilib>:"Add State(s) to Queue__JKI_lib_State_Machine.vi"("State(s) in (\"\")"=w3045) -> ("States Out"=w3044:string)  [unwired: 14 in]
      }
      frame "TCP: InitializeNew" {
        # "if unsuccessful and count <10, increament count \nand try again"
        # "Initialize TCP connection to aimging beam computer\n(You can make a copy of, or modify, this frame)"
        n1420 = TCP Create Listener(10:u16 2100 ("port"), 11:"RTLT" ("service name")) -> (0:w3054:errorcluster, 3:w3046:refnum<k5>)  [unwired: 3 in, 1 out]
        n1421 = while {
          tunnel: w3046 -> [w3074]
          tunnel: w3054 -> [w3073]
          tunnel: [w3064] -> w3052
          tunnel: [w3061] -> w3048
          i -> [w3070]
          stop <- w3061 stop-if-true
          n1422 = TCP Wait On Listener(8:w3073, 9:200 ("timeout ms (wait forever: -1)"), 11:w3074) -> (0:w3071:errorcluster, 4:w3068:refnum<k5>)  [unwired: 1 in, 3 out]
          n1423 = Less Or Equal?(x=50, y=w3070) -> (x <= y?=w3067:bool)
          n1424 = case shown="No Error" w3071 {
            selector: w3071 -> [w3084 w3094]
            tunnel: w3068 -> [w3085 _]
            tunnel: [errorcluster {"status"=TRUE, "code"=0, "source"=""} ("No error") w3095] -> w3063
            tunnel: [w3076 FALSE ("TCP connected?")] -> w3064
            frame No Error {
              # "connection is ready, read data"
              n1425 = TCP Read(connection ID=w3085, bytes to read=512, error in (no error)=w3084, 7:T22."CRLF" ("mode (standard)"), 9:5000 ("timeout ms (25000)")) -> (connection ID out=w3078:refnum<k5>, data out=w3080:string, error out=w3077:errorcluster)
              n1426 = Concatenate Strings("alive" ("string"), "\r\n" ("End of Line Constant")) -> (w3081:string)
              n1427 = Equal?(x=w3081, y=w3080) -> (x = y?=w3079:bool)
              n1428 = case shown="False" w3079 {
                tunnel: w3078 -> [_ w3090]
                tunnel: w3077 -> [_ _]
                tunnel: [FALSE ("TCP connected?") TRUE ("TCP connected?")] -> w3076
                frame False {
                }
                frame True {
                  n1429 = call "TcpIDFGV.vi"("action"=enum16{"write", "read"}."write", "connection ID in"=w3090) -> ()  [unwired: 8 in, 2 out]
                }
              }
            }
            frame Error {
              # "connection not ready, keep waiting"
              n1430 = Unbundle By Name(w3094) -> ("code"=w3096:i32)
              n1431 = case shown="56" w3096 {
                tunnel: w3094 -> [w3097 _]
                tunnel: [w3097 w3098] -> w3095
                frame Default {
                }
                frame 56 {
                  w3098 = errorcluster {"status"=FALSE, "code"=0, "source"=""}  # No error
                }
              }
            }
          }
          n1432 = Select(t=errorcluster {"status"=TRUE, "code"=5001, "source"=""} ("error in (no error)"), s=w3067, f=errorcluster {"status"=FALSE, "code"=0, "source"=""} ("error in (no error)")) -> (s? t:f=w3062:errorcluster)
          n1433 = Merge Errors(w3063, w3062) -> (w3061:errorcluster)
        }
        n1434 = Unbundle By Name(w3048) -> ("code"=w3051:i32)
        n1435 = Bundle By Name(cluster=w3053, "System Status.TCP/IP"=w3052, "listener ID"=w3046) -> (w3058:T24)
        n1436 = global write "GlobalVariables.vi" "TCP connected?"(w3052) -> ()
        n1437 = Equal To 0?(x=w3051) -> (x = 0?=w3050:bool)
        n1438 = Select(t=errorcluster {"status"=FALSE, "code"=0, "source"=""} ("error in (no error)"), s=w3050, f=w3048) -> (s? t:f=w3047:errorcluster)
        n1439 = call <vilib>:"Add State(s) to Queue__JKI_lib_State_Machine.vi"("State(s) in (\"\")"=w3060) -> ("States Out"=w3059:string)  [unwired: 14 in]
      }
      frame "TCP: checkSource" {
        # "Check visualization PC video source\n(send !video_source message, listen for response, then parse it to binary mask)"
        n1440 = Unbundle By Name(w3105) -> ("System Status.TCP/IP"=w3108:bool)
        n1441 = case shown="True" w3108 {
          tunnel: w3107 -> [w3113 w3136]
          tunnel: [w3113 w3120] -> w3106
          tunnel: [w3112 w3125] -> w3103
          tunnel: [w3112 w3123] -> w3102
          tunnel: [w3112 w3124] -> w3101
          tunnel: [w3112 w3122] -> w3100
          tunnel: [w3112 w3114] -> w3099
          frame False {
            w3112 = FALSE
          }
          frame True {
            n1442 = call "TcpIDFGV.vi"("Error In"=w3136, "action"=enum16{"write", "read"}."read") -> ("Error Out"=w3133:errorcluster, "connection ID out"=w3135:refnum<k5>)  [unwired: 8 in]
            n1443 = call "TCP_WriteRead.vi"("error in (no error)"=w3133, "data in"="!video_source", "connectin ID in"=w3135) -> ("error out"=w3130:errorcluster, "data out"=w3132:string)  [unwired: 4 in, 1 out]
            n1444 = Scan From String(format string="!video_source:%d", input string=w3132, error in=w3130) -> (error out=w3121:errorcluster, output 1=w3119:i32)  [unwired: 2 in, 2 out]
            n1445 = case shown="5..7, 9..11, 13..15" w3119 {
              tunnel: w3121 -> [_ _ _ _]
              tunnel: [errorcluster {"status"=TRUE, "code"=5007, "source"="Visualization PC"} ("error out") errorcluster {"status"=FALSE, "code"=0, "source"=""} ("error out") errorcluster {"status"=FALSE, "code"=0, "source"=""} ("error out") errorcluster {"status"=FALSE, "code"=0, "source"=""} ("error out")] -> w3120
              tunnel: [FALSE FALSE FALSE TRUE] -> w3114
              frame 0, Default {
                # "No video source available or default"
                n1446 = property on="Video Source" class="RadioBtnsControl (strict)"("DisabledEnum"=T13."Disabled and Grayed Out" ("Disabled")) -> ()  [unwired: 2 in, 2 out]
              }
              frame 1..3 {
                # "one or both camera available"
                n1447 = local write "Video Source"(enum32{"Camera", "FrameGrabber"}."Camera" ("Video Source")) -> ()
                n1448 = property on="Video Source" class="RadioBtnsControl (strict)"("DisabledEnum"=T13."Disabled and Grayed Out" ("Disabled")) -> ()  [unwired: 2 in, 2 out]
              }
              frame 4, 8, 12 {
                # "one or both frame grabber available"
                n1449 = local write "Video Source"(enum32{"Camera", "FrameGrabber"}."FrameGrabber" ("Video Source")) -> ()
                n1450 = property on="Video Source" class="RadioBtnsControl (strict)"("DisabledEnum"=T13."Disabled and Grayed Out" ("Disabled")) -> ()  [unwired: 2 in, 2 out]
              }
              frame 5..7, 9..11, 13..15 {
                n1451 = property on="Video Source" class="RadioBtnsControl (strict)"("DisabledEnum"=T13."Enabled" ("Disabled")) -> ()  [unwired: 2 in, 2 out]
              }
            }
            n1452 = Integer to Fixed-Point Cast(fixed-point type=fxp<+,4,4> 0.0, integer=w3119) -> (fixed-point=w3118:fxp<+,4,4>)
            n1453 = Number To Boolean Array(number=w3118) -> (Boolean array=w3116:bool[])
            n1454 = Reverse 1D Array(array=w3116) -> (reversed array=w3115:bool[])
            n1455 = Index Array(array=w3115, index=0) -> (element=w3125:bool)
            n1456 = Index Array(array=w3115, index=1) -> (element=w3123:bool)
            n1457 = Index Array(array=w3115, index=2) -> (element=w3124:bool)
            n1458 = Index Array(array=w3115, index=3) -> (element=w3122:bool)
          }
        }
        n1459 = Bundle By Name(cluster=w3105, "video source.Main Frame Grabber"=w3103, "video source.Side Frame Grabber"=w3102, "video source.Main Camera"=w3101, "video source.Side Camera"=w3100, "bothVidSourceAvail"=w3099) -> (w3104:T24)
        n1460 = call <vilib>:"Add State(s) to Queue__JKI_lib_State_Machine.vi"("State(s) in (\"\")"=w3111) -> ("States Out"=w3110:string)  [unwired: 14 in]
      }
      frame "TCP: SyncTime" {
        # "Template Separator\n(You can make a copy of, or modify, this frame)"
        n1461 = Unbundle By Name(w3153) -> ("System Status.TCP/IP"=w3152:bool)
        n1462 = case shown="True" w3152 {
          tunnel: w3154 -> [_ w3162]
          frame False {
          }
          frame True {
            n1463 = call "TcpIDFGV.vi"("Error In"=w3162, "action"=enum16{"write", "read"}."read") -> ("Error Out"=w3161:errorcluster, "connection ID out"=w3158:refnum<k5>)  [unwired: 8 in]
            n1464 = call <userlib>:"Tick Count (ms)__ogtk.vi"("error in (no error)"=w3161) -> ("error out"=w3160:errorcluster, "millisecond timer value"=w3159:u32)  [unwired: 9 in]
            n1465 = while {
              tunnel: w3160 -> [w3182]
              tunnel: w3158 -> [w3181]
              tunnel: w3159 -> [w3170]
              stop <- w3165 stop-if-true
              n1466 = Concatenate Strings("latencycheck" ("string"), "\r\n" ("End of Line Constant")) -> (w3177:string)
              n1467 = TCP Read(connection ID=w3181, bytes to read=512, error in (no error)=w3182, 7:T22."CRLF" ("mode (standard)"), 9:2000 ("timeout ms (25000)")) -> (connection ID out=w3174:refnum<k5>, data out=w3172:string, error out=w3164:errorcluster)
              n1468 = Tick Count (ms)() -> (millisecond timer value=w3171:u32)
              n1469 = Subtract(x=w3171, y=w3170) -> (x-y=w3169:u32)
              n1470 = Equal?(x=w3172, y=w3177) -> (x = y?=w3173:bool)
              n1471 = case shown="False" w3173 {
                tunnel: w3174 -> [_ w3195]
                tunnel: w3172 -> [w3187 _]
                tunnel: [w3183 FALSE] -> w3167
                tunnel: w3164 -> [_ w3189]
                frame False {
                  n1472 = Concatenate Strings("synctimer" ("string"), "\r\n" ("End of Line Constant")) -> (w3184:string)
                  n1473 = Equal?(x=w3187, y=w3184) -> (x = y?=w3183:bool)
                  "Sync Success?" <- w3183
                }
                frame True {
                  n1474 = Concatenate Strings("latencycheck:" ("string"), "\r\n" ("End of Line Constant")) -> (w3194:string)
                  n1475 = TCP Write(connection ID=w3195, data in=w3194, error in (no error)=w3189, 9:1000 ("timeout ms (25000)")) -> (error out=w3188:errorcluster)  [unwired: 2 out]
                  n1476 = call <vilib>:"Clear Errors.vi"("error in (no error)"=w3188) -> ()  [unwired: 5 in, 2 out]
                }
              }
              n1477 = Greater?(x=w3169, y=u32 10000 ("x-y")) -> (0:w3166:bool)
              n1478 = Or(x=w3167, y=w3166) -> (x .or. y?=w3165:bool)
            }
          }
        }
        n1479 = call <vilib>:"Add State(s) to Queue__JKI_lib_State_Machine.vi"("State(s) in (\"\")"=w3157) -> ("States Out"=w3156:string)  [unwired: 14 in]
      }
      frame "TCP: SendSettingMacro" {
        # "Template Separator\n(You can make a copy of, or modify, this frame)"
        n1480 = Unbundle By Name(w3199) -> ("System Status.TCP/IP"=w3198:bool)
        n1481 = case shown="True" w3198 {
          tunnel: ["" ("Empty String Constant") "TCP: sendSubjectID\nTCP: sendScaleBarSetting\nTCP: sendScaleMaxMin\nTCP: sendDeconChannel\nTCP: sendANSI\nTCP: sendRadius\nTCP: send3Dsetting\nTCP: sendFirefly\nTCP: sendPentero"] -> w3197
          frame False {
          }
          frame True {
          }
        }
        n1482 = call <vilib>:"Add State(s) to Queue__JKI_lib_State_Machine.vi"("State(s) in Front (\"\")"=w3197, "State(s) in (\"\")"=w3202) -> ("States Out"=w3201:string)  [unwired: 13 in]
      }
      frame "TCP: sendRunNum" {
        # "Send run number to AB PC\n(You can make a copy of, or modify, this frame)"
        n1483 = Unbundle By Name(w3209) -> ("System Status.TCP/IP"=w3206:bool, "IDs.RunID"=w3210:i8)
        n1484 = Increment(x=w3210) -> (x+1=w3205:i8)
        n1485 = case shown="True" w3206 {
          tunnel: w3205 -> [_ w3224]
          tunnel: [w3214 w3216] -> w3208
          tunnel: w3207 -> [w3214 w3215]
          frame False {
          }
          frame True {
            n1486 = Number To Decimal String(number=w3224, width (-)=i16 3) -> (decimal integer string=w3219:string)
            n1487 = call "TcpIDFGV.vi"("Error In"=w3215, "action"=enum16{"write", "read"}."read") -> ("Error Out"=w3217:errorcluster, "connection ID out"=w3221:refnum<k5>)  [unwired: 8 in]
            n1488 = Concatenate Strings("!run:", w3219) -> (w3218:string)
            n1489 = call "TCP_WriteRead.vi"("error in (no error)"=w3217, "data in"=w3218, "connectin ID in"=w3221) -> ("error out"=w3216:errorcluster)  [unwired: 4 in, 2 out]
          }
        }
        n1490 = call <vilib>:"Add State(s) to Queue__JKI_lib_State_Machine.vi"("State(s) in (\"\")"=w3213) -> ("States Out"=w3212:string)  [unwired: 14 in]
      }
      frame "TCP: sendVideoSource" {
        # "Send video source \n(You can make a copy of, or modify, this frame)"
        n1491 = Unbundle By Name(w3226) -> ("System Status.TCP/IP"=w3225:bool)
        n1492 = case shown="True" w3225 {
          tunnel: [w3232 w3234] -> w3228
          tunnel: w3227 -> [w3232 w3233]
          frame False {
          }
          frame True {
            n1493 = case shown="\"Camera\", Default" "Video Source" {
              tunnel: [0 1] -> w3239
              frame "Camera", Default {
              }
              frame "FrameGrabber" {
              }
            }
            n1494 = call "TcpIDFGV.vi"("Error In"=w3233, "action"=enum16{"write", "read"}."read") -> ("Error Out"=w3235:errorcluster, "connection ID out"=w3241:refnum<k5>)  [unwired: 8 in]
            n1495 = Number To Decimal String(number=w3239) -> (decimal integer string=w3237:string)  [unwired: 1 in]
            n1496 = Concatenate Strings("!invivo:" ("data in"), w3237) -> (w3236:string)
            n1497 = call "TCP_WriteRead.vi"("error in (no error)"=w3235, "data in"=w3236, "connectin ID in"=w3241) -> ("error out"=w3234:errorcluster)  [unwired: 4 in, 2 out]
          }
        }
        n1498 = call <vilib>:"Add State(s) to Queue__JKI_lib_State_Machine.vi"("State(s) in (\"\")"=w3231) -> ("States Out"=w3230:string)  [unwired: 14 in]
      }
      frame "TCP: startRun" {
        # "Template Separator\n(You can make a copy of, or modify, this frame)"
        n1499 = Unbundle By Name(w3246) -> ("System Status.TCP/IP"=w3245:bool)
        n1500 = case shown="True" w3245 {
          tunnel: [w3252 w3254] -> w3248
          tunnel: w3247 -> [w3252 w3253]
          frame False {
          }
          frame True {
            n1501 = call "TcpIDFGV.vi"("Error In"=w3253, "action"=enum16{"write", "read"}."read") -> ("Error Out"=w3255:errorcluster, "connection ID out"=w3256:refnum<k5>)  [unwired: 8 in]
            n1502 = call "TCP_WriteRead.vi"("error in (no error)"=w3255, "data in"="!acquire:1", "connectin ID in"=w3256) -> ("error out"=w3254:errorcluster)  [unwired: 4 in, 2 out]
          }
        }
        n1503 = call <vilib>:"Add State(s) to Queue__JKI_lib_State_Machine.vi"("State(s) in (\"\")"=w3251) -> ("States Out"=w3250:string)  [unwired: 14 in]
      }
      frame "TCP: stopRun" {
        # "Send stop run to AB PC\n(You can make a copy of, or modify, this frame)"
        n1504 = Unbundle By Name(w3260) -> ("System Status.TCP/IP"=w3259:bool)
        n1505 = case shown="True" w3259 {
          tunnel: [w3266 w3268] -> w3262
          tunnel: w3261 -> [w3266 w3267]
          frame False {
            # "if not connected, do nothing"
          }
          frame True {
            # "If TCP connected, send stop run"
            n1506 = call "TcpIDFGV.vi"("Error In"=w3267, "action"=enum16{"write", "read"}."read") -> ("Error Out"=w3269:errorcluster, "connection ID out"=w3271:refnum<k5>)  [unwired: 8 in]
            n1507 = call "TCP_WriteRead.vi"("error in (no error)"=w3269, "data in"="!acquire:0", "connectin ID in"=w3271) -> ("error out"=w3268:errorcluster)  [unwired: 4 in, 2 out]
          }
        }
        n1508 = call <vilib>:"Add State(s) to Queue__JKI_lib_State_Machine.vi"("State(s) in (\"\")"=w3265) -> ("States Out"=w3264:string)  [unwired: 14 in]
      }
      frame "TCP: CheckConnection" {
        # "Check TCP/IP connection statuse\n(If connection is lost, throw error)"
        n1509 = Unbundle By Name(w3274) -> ("System Status.TCP/IP"=w3273:bool)
        n1510 = case shown="False" w3273 {
          frame False {
          }
          frame True {
            # "If TCP/IP is true check, otherwise skip"
          }
        }
        n1511 = call <vilib>:"Add State(s) to Queue__JKI_lib_State_Machine.vi"("State(s) in (\"\")"=w3278) -> ("States Out"=w3277:string)  [unwired: 14 in]
      }
      frame "TCP: sendSubjectID" {
        # "Send subject ID"
        n1512 = Unbundle By Name(w3280) -> ("System Status.TCP/IP"=w3279:bool, "CaseID"=w3283:string)
        n1513 = case shown="True" w3279 {
          tunnel: w3283 -> [_ w3294]
          tunnel: [w3287 w3289] -> w3282
          tunnel: w3281 -> [w3287 w3288]
          frame False {
          }
          frame True {
            n1514 = call "TcpIDFGV.vi"("Error In"=w3288, "action"=enum16{"write", "read"}."read") -> ("Error Out"=w3290:errorcluster, "connection ID out"=w3292:refnum<k5>)  [unwired: 8 in]
            n1515 = Concatenate Strings("!subject:", w3294) -> (w3291:string)
            n1516 = call "TCP_WriteRead.vi"("error in (no error)"=w3290, "data in"=w3291, "connectin ID in"=w3292) -> ("error out"=w3289:errorcluster)  [unwired: 4 in, 2 out]
          }
        }
        n1517 = call <vilib>:"Add State(s) to Queue__JKI_lib_State_Machine.vi"("State(s) in (\"\")"=w3286) -> ("States Out"=w3285:string)  [unwired: 14 in]
      }
      frame "TCP: sendScaleBarSetting" {
        # "Template Separator\n(You can make a copy of, or modify, this frame)"
        n1518 = Unbundle By Name(w3298) -> ("System Status.TCP/IP"=w3296:bool, "VideoConfig.Scale Bar"=w3297:bool)
        n1519 = case shown="True" w3296 {
          tunnel: [w3304 w3313] -> w3300
          tunnel: w3299 -> [w3304 w3312]
          tunnel: w3297 -> [_ w3311]
          frame False {
          }
          frame True {
            n1520 = Boolean To (0,1)(Boolean=w3311) -> (0, 1=w3310:i16)
            n1521 = call "TcpIDFGV.vi"("Error In"=w3312, "action"=enum16{"write", "read"}."read") -> ("Error Out"=w3314:errorcluster, "connection ID out"=w3315:refnum<k5>)  [unwired: 8 in]
            n1522 = Number To Fractional String(number=w3310, width (-)=i16 1, precision (6)=i16 0) -> (F-format string=w3308:string)  [unwired: 1 in]
            n1523 = Concatenate Strings("!autocolor:" ("data in"), w3308) -> (w3306:string)
            n1524 = call "TCP_WriteRead.vi"("error in (no error)"=w3314, "data in"=w3306, "connectin ID in"=w3315) -> ("error out"=w3313:errorcluster)  [unwired: 4 in, 2 out]
          }
        }
        n1525 = call <vilib>:"Add State(s) to Queue__JKI_lib_State_Machine.vi"("State(s) in (\"\")"=w3303) -> ("States Out"=w3302:string)  [unwired: 14 in]
      }
      frame "TCP: sendScaleMaxMin" {
        # "Send scale bar max and min to AB PC\n(You can make a copy of, or modify, this frame)"
        n1526 = Unbundle By Name(w3320) -> ("System Status.TCP/IP"=w3317:bool, "VideoConfig.Scale Low"=w3319:dbl, "VideoConfig.Scale High"=w3318:dbl)
        n1527 = case shown="True" w3317 {
          tunnel: [w3326 w3339] -> w3322
          tunnel: w3321 -> [w3326 w3338]
          tunnel: w3319 -> [_ w3337]
          tunnel: w3318 -> [_ w3328]
          frame False {
          }
          frame True {
            n1528 = call "TcpIDFGV.vi"("Error In"=w3338, "action"=enum16{"write", "read"}."read") -> ("Error Out"=w3340:errorcluster, "connection ID out"=w3341:refnum<k5>)  [unwired: 8 in]
            n1529 = Number To Fractional String(number=w3337, width (-)=i16 4, precision (6)=i16 2) -> (F-format string=w3333:string)  [unwired: 1 in]
            n1530 = Number To Fractional String(number=w3328, width (-)=i16 4, precision (6)=i16 2) -> (F-format string=w3329:string)  [unwired: 1 in]
            n1531 = Concatenate Strings("!color:" ("string"), w3333, ";" ("string"), w3329) -> (w3327:string)
            n1532 = call "TCP_WriteRead.vi"("error in (no error)"=w3340, "data in"=w3327, "connectin ID in"=w3341) -> ("error out"=w3339:errorcluster)  [unwired: 4 in, 2 out]
          }
        }
        n1533 = call <vilib>:"Add State(s) to Queue__JKI_lib_State_Machine.vi"("State(s) in (\"\")"=w3325) -> ("States Out"=w3324:string)  [unwired: 14 in]
      }
      frame "TCP: sendDeconChannel" {
        # "Send Decon channel\n(You can make a copy of, or modify, this frame)"
        n1534 = Unbundle By Name(w3344) -> ("System Status.TCP/IP"=w3343:bool)
        n1535 = case shown="True" w3343 {
          tunnel: [w3350 w3355] -> w3346
          tunnel: w3345 -> [w3350 w3354]
          frame False {
          }
          frame True {
            n1536 = local read "Radio Buttons"() -> (w3353:T10)
            n1537 = Increment(x=w3353) -> (x+1=w3352:T10)
            n1538 = Number To Decimal String(number=w3352) -> (decimal integer string=w3351:string)  [unwired: 1 in]
            n1539 = call "TcpIDFGV.vi"("Error In"=w3354, "action"=enum16{"write", "read"}."read") -> ("Error Out"=w3356:errorcluster, "connection ID out"=w3359:refnum<k5>)  [unwired: 8 in]
            n1540 = Concatenate Strings("!channel:", w3351) -> (w3357:string)
            n1541 = call "TCP_WriteRead.vi"("error in (no error)"=w3356, "data in"=w3357, "connectin ID in"=w3359) -> ("error out"=w3355:errorcluster)  [unwired: 4 in, 2 out]
          }
        }
        n1542 = call <vilib>:"Add State(s) to Queue__JKI_lib_State_Machine.vi"("State(s) in (\"\")"=w3349) -> ("States Out"=w3348:string)  [unwired: 14 in]
      }
      frame "TCP: sendANSI" {
        # "Template Separator\n(You can make a copy of, or modify, this frame)"
        n1543 = Unbundle By Name(w3363) -> ("System Status.TCP/IP"=w3361:bool, "VideoConfig.ANSI"=w3362:dbl)
        n1544 = case shown="True" w3361 {
          tunnel: [w3369 w3375] -> w3365
          tunnel: w3364 -> [w3369 w3374]
          tunnel: w3362 -> [_ w3373]
          frame False {
          }
          frame True {
            n1545 = Number To Fractional String(number=w3373) -> (F-format string=w3371:string)  [unwired: 3 in]
            n1546 = call "TcpIDFGV.vi"("Error In"=w3374, "action"=enum16{"write", "read"}."read") -> ("Error Out"=w3376:errorcluster, "connection ID out"=w3377:refnum<k5>)  [unwired: 8 in]
            n1547 = Concatenate Strings("!ansi:" ("data in"), w3371) -> (w3370:string)
            n1548 = call "TCP_WriteRead.vi"("error in (no error)"=w3376, "data in"=w3370, "connectin ID in"=w3377) -> ("error out"=w3375:errorcluster)  [unwired: 4 in, 2 out]
          }
        }
        n1549 = call <vilib>:"Add State(s) to Queue__JKI_lib_State_Machine.vi"("State(s) in (\"\")"=w3368) -> ("States Out"=w3367:string)  [unwired: 14 in]
      }
      frame "TCP: sendRadius" {
        # "Send drawing radius to AB PC\n(You can make a copy of, or modify, this frame)"
        n1550 = Unbundle By Name(w3381) -> ("System Status.TCP/IP"=w3379:bool, "VideoConfig.Radius"=w3380:dbl)
        n1551 = case shown="True" w3379 {
          tunnel: [w3387 w3393] -> w3383
          tunnel: w3382 -> [w3387 w3392]
          tunnel: w3380 -> [_ w3391]
          frame False {
          }
          frame True {
            n1552 = Number To Fractional String(number=w3391) -> (F-format string=w3390:string)  [unwired: 3 in]
            n1553 = Concatenate Strings("!radius:" ("data in"), w3390) -> (w3388:string)
            n1554 = call "TcpIDFGV.vi"("Error In"=w3392, "action"=enum16{"write", "read"}."read") -> ("Error Out"=w3394:errorcluster, "connection ID out"=w3395:refnum<k5>)  [unwired: 8 in]
            n1555 = call "TCP_WriteRead.vi"("error in (no error)"=w3394, "data in"=w3388, "connectin ID in"=w3395) -> ("error out"=w3393:errorcluster)  [unwired: 4 in, 2 out]
          }
        }
        n1556 = call <vilib>:"Add State(s) to Queue__JKI_lib_State_Machine.vi"("State(s) in (\"\")"=w3386) -> ("States Out"=w3385:string)  [unwired: 14 in]
      }
      frame "TCP: send3Dsetting" {
        # "Send 3D setting to AB computer\n(You can make a copy of, or modify, this frame)"
        n1557 = Unbundle By Name(w3399) -> ("System Status.TCP/IP"=w3397:bool, "VideoConfig.3D?"=w3398:bool)
        n1558 = case shown="True" w3397 {
          tunnel: [w3405 w3412] -> w3401
          tunnel: w3400 -> [w3405 w3411]
          tunnel: w3398 -> [_ w3410]
          frame False {
          }
          frame True {
            n1559 = Boolean To (0,1)(Boolean=w3410) -> (0, 1=w3409:i16)
            n1560 = Number To Fractional String(number=w3409) -> (F-format string=w3408:string)  [unwired: 3 in]
            n1561 = call "TcpIDFGV.vi"("Error In"=w3411, "action"=enum16{"write", "read"}."read") -> ("Error Out"=w3413:errorcluster, "connection ID out"=w3414:refnum<k5>)  [unwired: 8 in]
            n1562 = Concatenate Strings("!3dset:" ("data in"), w3408) -> (w3406:string)
            n1563 = call "TCP_WriteRead.vi"("error in (no error)"=w3413, "data in"=w3406, "connectin ID in"=w3414) -> ("error out"=w3412:errorcluster)  [unwired: 4 in, 2 out]
          }
        }
        n1564 = call <vilib>:"Add State(s) to Queue__JKI_lib_State_Machine.vi"("State(s) in (\"\")"=w3404) -> ("States Out"=w3403:string)  [unwired: 14 in]
      }
      frame "TCP: sendFirefly" {
        # "Template Separator\n(You can make a copy of, or modify, this frame)"
        n1565 = Unbundle By Name(w3417) -> ("System Status.TCP/IP"=w3416:bool)
        n1566 = case shown="False" w3416 {
          tunnel: [w3423 w3425] -> w3419
          tunnel: w3418 -> [w3423 w3424]
          frame False {
          }
          frame True {
            n1567 = call "TcpIDFGV.vi"("Error In"=w3424, "action"=enum16{"write", "read"}."read") -> ("Error Out"=w3426:errorcluster, "connection ID out"=w3428:refnum<k5>)  [unwired: 8 in]
            n1568 = call "TCP_WriteRead.vi"("error in (no error)"=w3426, "data in"="!firefly:0", "connectin ID in"=w3428) -> ("error out"=w3425:errorcluster)  [unwired: 4 in, 2 out]
          }
        }
        n1569 = call <vilib>:"Add State(s) to Queue__JKI_lib_State_Machine.vi"("State(s) in (\"\")"=w3422) -> ("States Out"=w3421:string)  [unwired: 14 in]
      }
      frame "TCP: sendPentero" {
        # "Send Pentero setting to AB computer\n(You can make a copy of, or modify, this frame)"
        n1570 = Unbundle By Name(w3431) -> ("System Status.TCP/IP"=w3430:bool)
        n1571 = case shown="True" w3430 {
          tunnel: [w3437 w3439] -> w3433
          tunnel: w3432 -> [w3437 w3438]
          frame False {
          }
          frame True {
            n1572 = call "TcpIDFGV.vi"("Error In"=w3438, "action"=enum16{"write", "read"}."read") -> ("Error Out"=w3440:errorcluster, "connection ID out"=w3442:refnum<k5>)  [unwired: 8 in]
            n1573 = call "TCP_WriteRead.vi"("error in (no error)"=w3440, "data in"="!pentero:0", "connectin ID in"=w3442) -> ("error out"=w3439:errorcluster)  [unwired: 4 in, 2 out]
          }
        }
        n1574 = call <vilib>:"Add State(s) to Queue__JKI_lib_State_Machine.vi"("State(s) in (\"\")"=w3436) -> ("States Out"=w3435:string)  [unwired: 14 in]
      }
      frame "TCP: sendChannel" {
        # "Send DeCon Channel to AB computer\n()"
        n1575 = Unbundle By Name(w3445) -> ("System Status.TCP/IP"=w3444:bool)
        n1576 = case shown="True" w3444 {
          tunnel: [w3451 w3455] -> w3447
          tunnel: w3446 -> [w3451 w3454]
          frame False {
          }
          frame True {
            n1577 = local read "Radio Buttons"() -> (w3453:T10)
            n1578 = case shown="\"No Selection\", Default" w3453 {
              tunnel: ["" ("data in") "!channel:1" ("data in") "!channel:2" ("data in") "!channel:3" ("data in")] -> w3452
              frame "No Selection", Default {
              }
              frame "Ch1" {
              }
              frame "Ch2" {
              }
              frame "Ch3" {
              }
            }
            n1579 = call "TcpIDFGV.vi"("Error In"=w3454, "action"=enum16{"write", "read"}."read") -> ("Error Out"=w3456:errorcluster, "connection ID out"=w3457:refnum<k5>)  [unwired: 8 in]
            n1580 = call "TCP_WriteRead.vi"("error in (no error)"=w3456, "data in"=w3452, "connectin ID in"=w3457) -> ("error out"=w3455:errorcluster)  [unwired: 4 in, 2 out]
          }
        }
        n1581 = call <vilib>:"Add State(s) to Queue__JKI_lib_State_Machine.vi"("State(s) in (\"\")"=w3450) -> ("States Out"=w3449:string)  [unwired: 14 in]
      }
      frame "TCP: startCam" {
        # "Send Pentero setting to AB computer\n(You can make a copy of, or modify, this frame)"
        n1582 = Unbundle By Name(w3464) -> ("System Status.TCP/IP"=w3463:bool)
        n1583 = case shown="True" w3463 {
          tunnel: [w3470 w3472] -> w3466
          tunnel: w3465 -> [w3470 w3471]
          frame False {
          }
          frame True {
            n1584 = call "TcpIDFGV.vi"("Error In"=w3471, "action"=enum16{"write", "read"}."read") -> ("Error Out"=w3473:errorcluster, "connection ID out"=w3475:refnum<k5>)  [unwired: 8 in]
            n1585 = call "TCP_WriteRead.vi"("error in (no error)"=w3473, "data in"="!focus:1", "connectin ID in"=w3475) -> ("error out"=w3472:errorcluster)  [unwired: 4 in, 2 out]
          }
        }
        n1586 = call <vilib>:"Add State(s) to Queue__JKI_lib_State_Machine.vi"("State(s) in (\"\")"=w3469) -> ("States Out"=w3468:string)  [unwired: 14 in]
      }
      frame "TCP: stopCam" {
        # "Send Pentero setting to AB computer\n(You can make a copy of, or modify, this frame)"
        n1587 = Unbundle By Name(w3478) -> ("System Status.TCP/IP"=w3477:bool)
        n1588 = case shown="True" w3477 {
          tunnel: [w3484 w3486] -> w3480
          tunnel: w3479 -> [w3484 w3485]
          frame False {
          }
          frame True {
            n1589 = call "TcpIDFGV.vi"("Error In"=w3485, "action"=enum16{"write", "read"}."read") -> ("Error Out"=w3487:errorcluster, "connection ID out"=w3489:refnum<k5>)  [unwired: 8 in]
            n1590 = call "TCP_WriteRead.vi"("error in (no error)"=w3487, "data in"="!focus:0", "connectin ID in"=w3489) -> ("error out"=w3486:errorcluster)  [unwired: 4 in, 2 out]
          }
        }
        n1591 = call <vilib>:"Add State(s) to Queue__JKI_lib_State_Machine.vi"("State(s) in (\"\")"=w3483) -> ("States Out"=w3482:string)  [unwired: 14 in]
      }
      frame "TCP: Close" {
        # "Close TCP connection\n()"
        n1592 = Unbundle By Name(w3493) -> ("System Status.TCP/IP"=w3491:bool)
        n1593 = case shown="True" w3491 {
          tunnel: [w3499 w3501] -> w3494
          tunnel: w3492 -> [w3499 w3500]
          frame False {
          }
          frame True {
            n1594 = call "TcpIDFGV.vi"("Error In"=w3500, "action"=enum16{"write", "read"}."read") -> ("Error Out"=w3503:errorcluster, "connection ID out"=w3504:refnum<k5>)  [unwired: 8 in]
            n1595 = TCP Close Connection(connection ID=w3504, error in (no error)=w3503) -> (error out=w3501:errorcluster)  [unwired: 1 in, 1 out]
          }
        }
        n1596 = case shown="Error .." w3494 {
          tunnel: [w3507 w3508] -> w3495
          tunnel: w3493 -> [w3506 w3508]
          frame No Error {
            w3505 = FALSE ("System Status.TCP/IP")
            n1597 = Bundle By Name(cluster=w3506, "System Status.TCP/IP"=w3505) -> (w3507:T24)
            n1598 = global write "GlobalVariables.vi" "TCP connected?"(w3505) -> ()
          }
          frame Error {
          }
        }
        n1599 = call <vilib>:"Add State(s) to Queue__JKI_lib_State_Machine.vi"("State(s) in (\"\")"=w3498) -> ("States Out"=w3497:string)  [unwired: 14 in]
      }
      frame "---------- PID ----------" {
        # "Template Separator\n(You can make a copy of, or modify, this frame)"
        n1600 = call <vilib>:"Add State(s) to Queue__JKI_lib_State_Machine.vi"("State(s) in (\"\")"=w3513) -> ("States Out"=w3512:string)  [unwired: 14 in]
      }
      frame "PID: loadPID" {
        # "Template Separator\n(You can make a copy of, or modify, this frame)"
        n1601 = call "readPIDSetting.vi"("Error In"=w3517) -> ("Error Out"=w3518:errorcluster, "Ch3 PID out"=w3514:T8, "Ch2 PID out"=w3515:T8, "Ch1 PID out"=w3516:T8)  [unwired: 7 in]
        n1602 = local write "Ch1 PID gains"(w3516) -> ()
        n1603 = local write "Ch2 PID gains"(w3515) -> ()
        n1604 = local write "Ch3 PID gains"(w3514) -> ()
        n1605 = local write "Ch4 PID gains"(w3514) -> ()
        n1606 = call <vilib>:"Add State(s) to Queue__JKI_lib_State_Machine.vi"("State(s) in (\"\")"=w3522) -> ("States Out"=w3521:string)  [unwired: 14 in]
      }
      frame "---------- Classifier ----------" {
        # "Template Separator\n(You can make a copy of, or modify, this frame)"
        n1607 = call <vilib>:"Add State(s) to Queue__JKI_lib_State_Machine.vi"("State(s) in (\"\")"=w3527) -> ("States Out"=w3526:string)  [unwired: 14 in]
      }
      frame "Classifier: Init" {
        # "Initilize Python\n(You can make a copy of, or modify, this frame)"
        n1608 = Unbundle By Name(w3529) -> ("OverlaySelection"=w3528:u16)
        n1609 = case shown="2" w3528 {
          tunnel: ["HN model path" "Brain model path"] -> w3532
          frame 0, 1, Default {
          }
          frame 2 {
          }
        }
        n1610 = call-poly <vilib>:"Open Virtual Environment Session.vi"("error in (no error)"=w3538, "Anaconda path"=path "C:/ProgramData/miniconda3", "Python version"="Python version", "Env name"="Env name") -> ("error out"=w3534:errorcluster, "session out"=w3537:refnum<k35>)  [unwired: 6 in]
        n1611 = Path To String(path=w3532) -> (string=w3531:string)
        n1612 = node "Python Node"(w3537, "module path", "load_model" ("function name"), w3534, w3531) -> (→"Python session":refnum<k35>, w3533:errorcluster)  [unwired: 3 in, 2 out]
        n1613 = call <vilib>:"Add State(s) to Queue__JKI_lib_State_Machine.vi"("State(s) in (\"\")"=w3544) -> ("States Out"=w3543:string)  [unwired: 14 in]
      }
      frame "Classifier: Close" {
        # "Template Separator\n(You can make a copy of, or modify, this frame)"
        n1614 = local read "Python session"() -> (w3550:refnum<k35>)
        n1615 = Close Python Session(session in=w3550, error in=w3549) -> (11:w3548:errorcluster)
        n1616 = case shown="Error .." w3548 {
          selector: w3548 -> [w3555 _]
          tunnel: [w3555 errorcluster {"status"=FALSE, "code"=0, "source"=""} ("error IO")] -> w3547
          frame No Error {
          }
          frame Error {
          }
        }
        n1617 = call <vilib>:"Add State(s) to Queue__JKI_lib_State_Machine.vi"("State(s) in (\"\")"=w3554) -> ("States Out"=w3553:string)  [unwired: 14 in]
      }
      frame "---------- DebugTDMS ----------" {
        # "Template Separator\n(You can make a copy of, or modify, this frame)"
        n1618 = call <vilib>:"Add State(s) to Queue__JKI_lib_State_Machine.vi"("State(s) in (\"\")"=w3561) -> ("States Out"=w3560:string)  [unwired: 14 in]
      }
      frame "DebugTDMS: Open" {
        # "Open Debug TDMS file"
        n1619 = Unbundle By Name(w3564) -> ("Pathes.DataPath"=w3573:path, "CaseID"=w3572:string, "IDs.RunID"=w3577:i8)
        n1620 = Increment(x=w3577) -> (x+1=w3571:i8)
        n1621 = Format Value(string ("")=w3572, format string="_%02d", value (0)=w3571) -> (output string=w3570:string)
        n1622 = Concatenate Strings(w3570, "RT_Result" ("string")) -> (w3568:string)
        n1623 = Build Path(base path=w3573, name or relative path=w3568) -> (appended path=w3576:path)
        n1624 = TDMS Open(8:w3562, 10:T16."create or replace" ("operation (0:open)"), 11:w3576) -> (0:w3567:errorcluster, 3:w3566:refnum<k34>)  [unwired: 4 in]
        n1625 = call "DebugTDMS_FGV.vi"("error in (no error)"=w3567, "Operation (Read)"=enum16{"Write", "Read"}."Write", "tdms file in"=w3566) -> ("error out"=w3563:errorcluster)  [unwired: 7 in, 1 out]
        n1626 = call <vilib>:"Add State(s) to Queue__JKI_lib_State_Machine.vi"("State(s) in (\"\")"=w3580) -> ("States Out"=w3579:string)  [unwired: 14 in]
      }
      frame "DebugTDMS: Close" {
        # "Close Debug TDMS"
        n1627 = call "DebugTDMS_FGV.vi"("error in (no error)"=w3581) -> ("error out"=w3583:errorcluster, "tdms file out"=w3584:refnum<k34>)  [unwired: 9 in]
        n1628 = TDMS Close(8:w3583, 11:w3584) -> (0:w3582:errorcluster)  [unwired: 1 out]
        n1629 = call <vilib>:"Add State(s) to Queue__JKI_lib_State_Machine.vi"("State(s) in (\"\")"=w3588) -> ("States Out"=w3587:string)  [unwired: 14 in]
      }
      frame "---------- Temp ----------" {
        # "Template Separator\n(You can make a copy of, or modify, this frame)"
        n1630 = call <vilib>:"Add State(s) to Queue__JKI_lib_State_Machine.vi"("State(s) in (\"\")"=w3593) -> ("States Out"=w3592:string)  [unwired: 14 in]
      }
      frame "Temp: KeepEmpty" {
        # "Template Separator\n(You can make a copy of, or modify, this frame)"
        n1631 = call <vilib>:"Add State(s) to Queue__JKI_lib_State_Machine.vi"("State(s) in (\"\")"=w3598) -> ("States Out"=w3597:string)  [unwired: 14 in]
      }
    }
    n1632 = Not(x=w87) -> (.not. x?=w86:bool)
    n1633 = local write "ML?"(w86) -> ()
    "ML?" <- TRUE ("main loop running?")
  }
  n1634 = while {
    tunnel: w2 -> [w3632]
    tunnel: w27 -> [w3601]
    tunnel: [w3600] -> w26
    tunnel: w7 -> [w3628]
    tunnel: [w3627] -> w25
    shift-right: [w3623] -> _
    shift-left: _ -> [w3624]
    stop <- w3603 stop-if-true
    # "Read data from notifier and deconvolve it and send to Aiming Beam computer"
    n1635 = Wait on Notification(notifier=w3632, ignore previous (F)=FALSE) -> (notification=w3619:T11, error out=w3603:errorcluster)  [unwired: 2 in, 2 out]
    n1636 = local read "Data Class"() -> (w3604:enum16{"Data", "BG", "Cali"})
    n1637 = Unbundle(w3619) -> ("idx"=w3602:i32, "CH1&2"=w3631:dbl[][], "CH3&4"=w3630:dbl[][], "V cluster"=w3609:cluster{"V1":dbl, "V2":dbl, "V3":dbl, "V4":dbl})
    n1638 = call "SeperateChanData.vi"("Input (Ch1&2)"=w3630) -> ("Ch1"=w3606:dbl[][], "Ch2"=w3614:dbl[][])
    n1639 = call "SeperateChanData.vi"("Input (Ch1&2)"=w3631) -> ("Ch1"=w3608:dbl[][], "Ch2"=w3607:dbl[][])
    n1640 = case shown="\"Data\"" w3604 {
      tunnel: w3609 -> [w3644 _]
      tunnel: w3608 -> [w3643 _]
      tunnel: w3607 -> [w3642 _]
      tunnel: w3606 -> [w3641 _]
      tunnel: w3603 -> [w3640 w3765]
      tunnel: w3602 -> [w3633 _]
      tunnel: w3601 -> [w3638 w3766]
      tunnel: [w3635 w3766] -> w3600
      tunnel: [w3634 w3765] -> w3599
      frame "Data" {
        # "If acquiring data"
        n1641 = case shown="1, 2" "Overlay selection" {
          tunnel: "Radio Buttons" -> [w3648 _]
          tunnel: [w3649 w3674] -> w3636
          tunnel: w3640 -> [w3649 w3673]
          tunnel: [w3647 w3661] -> w3639
          tunnel: w3644 -> [_ w3680]
          tunnel: w3643 -> [_ w3677]
          tunnel: w3642 -> [_ w3676]
          tunnel: w3641 -> [_ w3675]
          tunnel: w3633 -> [_ w3656]
          frame 0, Default {
            # "overlay gain"
            n1642 = case shown="\"Ch1\"" w3648 {
              tunnel: [0.0 ("Gain1") w3651 w3652 w3653 w3654] -> w3647
              frame "No Selection", Default {
              }
              frame "Ch1" {
                n1643 = local read "Gain1"() -> (w3651:dbl)
              }
              frame "Ch2" {
                n1644 = local read "Gain2"() -> (w3652:dbl)
              }
              frame "Ch3" {
                n1645 = local read "Gain3"() -> (w3653:dbl)
              }
              frame "Ch4" {
                n1646 = local read "Gain4"() -> (w3654:dbl)
              }
            }
          }
          frame 1, 2 {
            # "overlay lifetime or cancer probability"
            n1647 = call "DeConAPD2FGV.vi"("Error In"=w3673) -> ("Error Out"=w3679:errorcluster, "APDClass out"=w3670:T41)  [unwired: 9 in]
            n1648 = call "DeConAPD1FGV.vi"("Error In"=w3673) -> ("Error Out"=w3681:errorcluster, "APDClass out"=w3672:T41)  [unwired: 9 in]
            n1649 = call "DeConAPD3FGV.vi"("Error In"=w3673) -> ("Error Out"=w3678:errorcluster, "APDClass out"=w3668:T41)  [unwired: 9 in]
            n1650 = Unbundle By Name(w3680) -> ("V1"=w3671:dbl, "V2"=w3669:dbl, "V3"=w3667:dbl)
            n1651 = call "getGain.vi"("CtrlV"=w3667, "APD"=w3668) -> ("gain"=w3658:dbl)  [unwired: 8 in, 1 out]
            n1652 = call "getGain.vi"("CtrlV"=w3671, "APD"=w3672) -> ("gain"=w3660:dbl)  [unwired: 8 in, 1 out]
            n1653 = call "getGain.vi"("CtrlV"=w3669, "APD"=w3670) -> ("gain"=w3659:dbl)  [unwired: 8 in, 1 out]
            n1654 = Less?(x=w3660, y="Ch1GainLim") -> (x < y?=w3665:bool)
            n1655 = Less?(x=w3659, y="Ch2GainLim") -> (x < y?=w3664:bool)
            n1656 = Less?(x=w3658, y="Ch3GainLim") -> (x < y?=w3663:bool)
            n1657 = Compound Arithmetic op=AND(w3665, w3664, w3663) -> (w3662:bool)
            n1658 = case shown="True" w3662 {
              tunnel: w3681 -> [_ w3755]
              tunnel: w3679 -> [_ w3754]
              tunnel: w3678 -> [_ w3753]
              tunnel: w3677 -> [_ w3743]
              tunnel: w3676 -> [_ w3742]
              tunnel: w3675 -> [_ w3741]
              tunnel: [w3682 w3702] -> w3674
              tunnel: w3673 -> [w3682 w3734]
              tunnel: w3672 -> [_ w3733]
              tunnel: w3671 -> [_ w3732]
              tunnel: w3670 -> [_ w3731]
              tunnel: w3669 -> [_ w3730]
              tunnel: w3668 -> [_ w3729]
              tunnel: w3667 -> [_ w3728]
              tunnel: [0.0 ("Gain4") w3697] -> w3661
              tunnel: w3660 -> [_ w3720]
              tunnel: w3659 -> [_ w3719]
              tunnel: w3658 -> [_ w3718]
              tunnel: w3656 -> [_ w3690]
              frame False {
                # "give probability of 0.5"
                # "if gain is out of acceptable range"
              }
              frame True {
                # "if gain is within range"
                n1659 = Build Array(w3720, w3719, w3718) -> (w3717:dbl[])
                n1660 = call "getIrf (SubVI).vi"("error in"=w3755, "CtrlV"=w3732, "APD"=w3733) -> ("error out"=w3747:errorcluster, "irfTNorm"=w3750:dbl[])  [unwired: 6 in, 1 out]
                n1661 = call "getIrf (SubVI).vi"("error in"=w3754, "CtrlV"=w3730, "APD"=w3731) -> ("error out"=w3746:errorcluster, "irfTNorm"=w3749:dbl[])  [unwired: 6 in, 1 out]
                n1662 = call "getIrf (SubVI).vi"("error in"=w3753, "CtrlV"=w3728, "APD"=w3729) -> ("error out"=w3745:errorcluster, "irfTNorm"=w3748:dbl[])  [unwired: 6 in, 1 out]
                n1663 = call "DotNetFGV.vi"("Error In"=w3734) -> ("Error Out"=w3738:errorcluster, "reference out"=w3739:refnum<k24>)  [unwired: 9 in]
                n1664 = local read "OverlaySelection"() -> (w3696:T9)
                n1665 = local read "BGAll"() -> (w3752:dbl[][])
                n1666 = Merge Errors(w3738, w3747, w3746, w3745) -> (w3744:errorcluster)
                n1667 = Build Array(w3750, w3749, w3748) -> (w3735:dbl[][])
                n1668 = Build Array (concatenate)(w3743, w3742, w3741) -> (w3740:dbl[][])
                n1669 = local write "iRF Graph"(w3735) -> ()
                n1670 = Transpose 2D Array(2D array=w3752) -> (transposed array=w3751:dbl[][])
                n1671 = Transpose 2D Array(2D array=w3735) -> (transposed array=w3736:dbl[][])
                n1672 = Transpose 2D Array(2D array=w3740) -> (transposed array=w3737:dbl[][])
                n1673 = Reciprocal(x=w3717) -> (1/x=w3715:dbl[])
                n1674 = call "LagDeConAllCh (SubVI).vi"("new reference"=w3739, "error in (no error)"=w3744, "irf"=w3736, "BG"=w3751, "WF"=w3737) -> ("error out"=w3703:errorcluster, "LCs"=w3711:dbl[][], "INTs"=w3722:dbl[][], "LTs"=w3727:dbl[][])  [unwired: 3 in]
                n1675 = Index Array(array=w3727, index (col)=0 ("disabled index (col)")) -> (element=w3709:dbl[])  [unwired: 1 in]
                n1676 = Index Array(array=w3722, index (col)=0 ("disabled index (col)")) -> (element=w3716:dbl[])  [unwired: 1 in]
                n1677 = Multiply(x=w3716, y=w3715) -> (x*y=w3714:dbl[])
                n1678 = Index Array(array=w3711, index (col)=0 ("disabled index (col)")) -> (element=w3707:dbl[])  [unwired: 1 in]
                n1679 = Add Array Elements(numeric array=w3714) -> (sum=w3713:dbl)
                n1680 = Index Array(array=w3709, index=0) -> (element=w3700:dbl)
                "Ch1 Lifetime (ns)" <- w3700
                n1681 = Index Array(array=w3709, index=1) -> (element=w3699:dbl)
                "Ch2 Lifetime (ns)" <- w3699
                n1682 = Index Array(array=w3709, index=2) -> (element=w3698:dbl)
                "Ch3 Lifetime (ns)" <- w3698
                n1683 = Divide(x=w3714, y=w3713) -> (x/y=w3708:dbl[])
                n1684 = case shown="\"Brain Classifier\"" w3696 {
                  tunnel: w3709 -> [_ w3760 _]
                  tunnel: w3708 -> [_ w3759 _]
                  tunnel: w3707 -> [_ w3758 w3764]
                  tunnel: [dbl[] [] w3757 w3761] -> w3689
                  frame "Gain", Default {
                  }
                  frame "HN Classifier" {
                    n1685 = Build Array (concatenate)(w3760, w3759, w3758) -> (w3757:dbl[])
                  }
                  frame "Brain Classifier" {
                    # "Ch2&3 Lag Coeffi"
                    n1686 = Array Subset(array=w3764, index=12, length=24) -> (w3761:dbl[])
                  }
                }
                "DeConOut" <- w3689
                n1687 = Bundle(w3700, w3699, w3698) -> (→"Lifetime (ns)":cluster{dbl, dbl, dbl})  [unwired: 1 in]
                n1688 = call "DebugTDMS_FGV.vi"() -> ("error out"=w3694:errorcluster, "tdms file out"=w3695:refnum<k34>)  [unwired: 10 in]
                n1689 = local read "module path"() -> (w3705:path)
                n1690 = local read "Python session"() -> (w3706:refnum<k35>)
                n1691 = node(w3706, w3705, "Predict" ("function name"), w3703, 0.0, w3689) -> (w3702:errorcluster, w3688:dbl)  [unwired: 1 in, 3 out]
                "Cancer Prob" <- w3688
                n1692 = Greater?(x=w3688, y="CancerThreshold") -> (0:w3687:bool)
                n1693 = Build Array (concatenate)(w3690, w3689, w3688) -> (w3693:dbl[])
                n1694 = TDMS Write(0:w3695, 7:string[] ["DataAll"] ("channel name(s) in (Untitled)"), 9:w3693, 11:w3694) -> (15:→"error out":errorcluster)  [unwired: 2 in, 3 out]
                n1695 = Select(t=1.0, s=w3687, f=0.01) -> (s? t:f=w3697:dbl)
              }
            }
          }
        }
        n1696 = Bundle("idx"=w3633, "f"=w3639) -> (w3637:cluster{"idx":i32, "f":dbl})  [unwired: 1 in]
        n1697 = Send Notification(notification=w3637, notifier=w3638, error in (no error)=w3636) -> (notifier out=w3635:refnum<notifier>, error out=w3634:errorcluster)
      }
      frame "BG", Default {
        # "if not acquiting data"
      }
    }
    n1698 = call "AvgArrayTimeCritical.vi"("2D array"=w3608) -> ("1D Avg"=w3615:dbl[])  [unwired: 10 in]
    n1699 = call "AvgArrayTimeCritical.vi"("2D array"=w3607) -> ("1D Avg"=w3616:dbl[])  [unwired: 10 in]
    n1700 = call "AvgArrayTimeCritical.vi"("2D array"=w3606) -> ("1D Avg"=w3617:dbl[])  [unwired: 10 in]
    n1701 = call "AvgArrayTimeCritical.vi"("2D array"=w3614) -> ("1D Avg"=w3618:dbl[])  [unwired: 10 in]
    n1702 = Build Array(w3618) -> (w3613:dbl[][])
    n1703 = Build Array(w3617) -> (w3612:dbl[][])
    n1704 = Build Array(w3616) -> (w3611:dbl[][])
    n1705 = Build Array(w3615) -> (w3610:dbl[][])
    n1706 = flat-sequence {
      tunnel: [w3767] -> w3623
      tunnel: w3603 -> [_]
      frame #0 {
        n1707 = call <vilib>:"High Resolution Relative Seconds.vi"() -> ("relative seconds"=w3767:dbl)
      }
    }
    n1708 = Subtract(x=w3623, y=w3624) -> (x-y=w3626:dbl)
    n1709 = Multiply(x=w3626, y=1000.0) -> (x*y=→"Decon Loop timing (ms)" →"DeCon Speed(ms)":dbl)
    n1710 = Bundle(w3610, w3611, w3612, w3613, "V cluster"=w3609) -> (w3629:T50)  [unwired: 1 in]
    n1711 = Send Notification(notification=w3629, notifier=w3628, error in (no error)=w3603) -> (notifier out=w3627:refnum<notifier>, error out=w3605:errorcluster)
    n1712 = Merge Errors(w3599, w3605) -> (→"decon error out":errorcluster)
  }
  n1713 = while {
    tunnel: w27 -> [w3779]
    shift-right: [w3772] -> _
    shift-left: u32 0 -> [w3773]
    stop <- w3770 stop-if-true
    # "Send data to AB computer here"
    # "if TCP ip is not open loop will run once and stop. To re-establish connection and start this loop. Reboot softwrae."
    # "Data communication loop"
    n1714 = Wait on Notification(notifier=w3779, ignore previous (F)=FALSE) -> (notification=w3777:cluster{"idx":i32, "lifetime":dbl}, error out=w3771:errorcluster)  [unwired: 2 in, 2 out]
    n1715 = Wait Until Next ms Multiple(millisecond multiple=u32 25) -> ()  [unwired: 1 out]
    n1716 = Unbundle(w3777) -> ("idx"=w3776:i32, "lifetime"=w3775:dbl)
    n1717 = Tick Count (ms)() -> (millisecond timer value=w3772:u32)
    n1718 = global read "GlobalVariables.vi" "TCP connected?"() -> (w3769:bool)
    n1719 = Subtract(x=w3772, y=w3773) -> (x-y=→"Communication loop(ms)":u32)
    n1720 = case shown="True" w3769 {
      tunnel: w3776 -> [_ w3788]
      tunnel: w3775 -> [_ w3787]
      tunnel: w3771 -> [w3780 w3784]
      tunnel: [w3780 w3781] -> w3770
      frame False {
      }
      frame True {
        n1721 = Number To Decimal String(number=w3788) -> (decimal integer string=w3796:string)  [unwired: 1 in]
        n1722 = call "TcpIDFGV.vi"("Error In"=w3784, "action"=enum16{"write", "read"}."read") -> ("Error Out"=w3783:errorcluster, "connection ID out"=w3794:refnum<k5>)  [unwired: 8 in]
        n1723 = Concatenate Strings("!idx:", w3796) -> (w3797:string)
        n1724 = call "TCP_WriteRead.vi"("error in (no error)"=w3783, "data in"=w3797, "connectin ID in"=w3794) -> ("error out"=w3782:errorcluster, "connectin ID out"=w3795:refnum<k5>)  [unwired: 4 in, 1 out]
        n1725 = Number To Fractional String(number=w3787, precision (6)=i16 2) -> (F-format string=w3786:string)  [unwired: 2 in]
        n1726 = Concatenate Strings("!lifetime:", w3786) -> (w3793:string)
        n1727 = call "TCP_WriteRead.vi"("error in (no error)"=w3782, "data in"=w3793, "connectin ID in"=w3795) -> ("error out"=w3781:errorcluster, "data out"=→"data out(communcation loop)":string)  [unwired: 4 in, 1 out]
      }
    }
  }
  n1728 = while {
    tunnel: w7 -> [w3808]
    shift-right: [w3799] -> _
    shift-left: w24 -> [w3806]
    shift-right: [w3801] -> _
    shift-left: w24 -> [w3800]
    i -> [w3802]
    stop <- w3803 stop-if-true
    # "Data display loop(30Hz)"
    n1729 = Wait on Notification(notifier=w3808, ignore previous (F)=FALSE) -> (notification=w3804:T15, error out=w3803:errorcluster)  [unwired: 2 in, 2 out]
    n1730 = Wait Until Next ms Multiple(millisecond multiple=u32 40) -> ()  [unwired: 1 out]
    n1731 = Tick Count (ms)() -> (millisecond timer value=w3799:u32)
    n1732 = Subtract(x=w3799, y=w3806) -> (x-y=→"display loop timing(ms)":u32)
    n1733 = case shown="No Error" w3803 {
      tunnel: w3804 -> [w3881 _]
      tunnel: w3800 -> [w3853 w3953]
      tunnel: [w3855 w3953] -> w3801
      tunnel: w3799 -> [w3852 _]
      frame No Error {
        w3810 = u32 1 ("Active Plot")
        w3829 = 0 ("index (row)")
        n1734 = Subtract(x=w3852, y=w3853) -> (x-y=w3854:u32)
        n1735 = Unbundle(w3881) -> ("CH1"=w3876:dbl[][], "CH2"=w3874:dbl[][], "CH3"=w3871:dbl[][], "CH4"=w3824:dbl[][], "Gain cluster"=w3830:cluster{"V1":dbl, "V2":dbl, "V3":dbl, "V4":dbl})
        n1736 = Unbundle By Name(w3830) -> ("V1"=w3848:dbl, "V2"=w3846:dbl, "V3"=w3844:dbl, "V4"=w3822:dbl)
        n1737 = Index Array(array=w3876, index (row)=w3829) -> (element=w3860:dbl[])  [unwired: 1 in]
        n1738 = Index Array(array=w3874, index (row)=w3829) -> (element=w3858:dbl[])  [unwired: 1 in]
        n1739 = Index Array(array=w3871, index (row)=w3829) -> (element=w3859:dbl[])  [unwired: 1 in]
        n1740 = Index Array(array=w3824, index (row)=w3829) -> (element=w3828:dbl[])  [unwired: 1 in]
        n1741 = call "RemoveDCBG.vi"("Channel"=enum16{"DC Only", "Ch1", "Ch2", "Ch3", "Ch4"}."Ch4", "WF in"=w3828) -> ("DC"=w3826:dbl, "WF out"=w3815:dbl[])  [unwired: 7 in, 1 out]
        n1742 = Greater?(x=w3854, y=u32 200) -> (0:w3856:bool)
        n1743 = call "CtrlVtoGain.vi"("CtrlV(V)"=w3822, "Channel"=enum16{"Ch1", "Ch2", "Ch3", "Ch4"}."Ch4") -> ("Gain"=w3814:dbl)  [unwired: 8 in, 1 out]
        n1744 = call "CtrlVtoGain.vi"("CtrlV(V)"=w3848, "Channel"=enum16{"Ch1", "Ch2", "Ch3"}."Ch1") -> ("Gain"=w3842:dbl)  [unwired: 8 in, 1 out]
        n1745 = call "RemoveDCBG.vi"("Channel"=enum16{"DC Only", "Ch1", "Ch2", "Ch3"}."Ch1", "WF in"=w3860) -> ("DC"=w3877:dbl, "WF out"=w3849:dbl[])  [unwired: 7 in, 1 out]
        n1746 = call "RemoveDCBG.vi"("Channel"=enum16{"DC Only", "Ch1", "Ch2", "Ch3"}."Ch2", "WF in"=w3858) -> ("DC"=w3873:dbl, "WF out"=w3850:dbl[])  [unwired: 7 in, 1 out]
        n1747 = call "CtrlVtoGain.vi"("CtrlV(V)"=w3846, "Channel"=enum16{"Ch1", "Ch2", "Ch3"}."Ch2") -> ("Gain"=w3837:dbl)  [unwired: 8 in, 1 out]
        n1748 = call "RemoveDCBG.vi"("Channel"=enum16{"DC Only", "Ch1", "Ch2", "Ch3"}."Ch3", "WF in"=w3859) -> ("DC"=w3870:dbl, "WF out"=w3851:dbl[])  [unwired: 7 in, 1 out]
        n1749 = call "CtrlVtoGain.vi"("CtrlV(V)"=w3844, "Channel"=enum16{"Ch1", "Ch2", "Ch3"}."Ch3") -> ("Gain"=w3833:dbl)  [unwired: 8 in, 1 out]
        n1750 = formula code="int32 out = 2;\nif (G<5){\nout = 1;\n}\nif (G>200){\nout = 3;\n}"("G"=w3814) -> ("out"=→"output variable":i32)
        n1751 = Add(x=w3815, y=w3826) -> (x+y=w3825:dbl[])
        n1752 = Less?(x=w3814, y=5.0) -> (x < y?=w3820:bool)
        n1753 = case shown="True" w3856 {
          tunnel: w3849 -> [_ w3910]
          tunnel: w3850 -> [_ w3913]
          tunnel: w3851 -> [_ w3912]
          tunnel: w3852 -> [_ w3928]
          tunnel: [w3892 w3928] -> w3855
          tunnel: w3853 -> [w3892 _]
          tunnel: w3842 -> [_ w3906]
          tunnel: w3837 -> [_ w3905]
          tunnel: w3833 -> [_ w3904]
          tunnel: w3815 -> [_ w3900]
          tunnel: w3814 -> [_ w3897]
          frame False {
          }
          frame True {
            n1754 = call "GetSNR(SubVI).vi"("Waveform"=w3910) -> ("SNR"=→"SNR1":dbl)  [unwired: 10 in]
            n1755 = Array Size(array=w3910) -> (size(s)=w3911:i32)
            n1756 = call "GetSNR(SubVI).vi"("Waveform"=w3913) -> ("SNR"=→"SNR2":dbl)  [unwired: 10 in]
            n1757 = call "GetSNR(SubVI).vi"("Waveform"=w3912) -> ("SNR"=→"SNR3":dbl)  [unwired: 10 in]
            n1758 = call "GetSNR(SubVI).vi"("Waveform"=w3900) -> ("SNR"=→"SNR4":dbl)  [unwired: 10 in]
            n1759 = global read "GlobalVariables.vi" "BG Idx2"() -> (w3899:i32)
            n1760 = Subtract(x=w3911, y=w3899) -> (x-y=w3898:i32)
            n1761 = Array Subset(array=w3910, index=w3899, length=w3898) -> (w3917:dbl[])
            n1762 = Array Subset(array=w3913, index=w3899, length=w3898) -> (w3919:dbl[])
            n1763 = Array Subset(array=w3912, index=w3899, length=w3898) -> (w3921:dbl[])
            n1764 = Array Subset(array=w3900, index=w3899, length=w3898) -> (w3901:dbl[])
            n1765 = Add Array Elements(numeric array=w3917) -> (sum=w3918:dbl)
            n1766 = Add Array Elements(numeric array=w3919) -> (sum=w3920:dbl)
            n1767 = Add Array Elements(numeric array=w3921) -> (sum=w3922:dbl)
            n1768 = Add Array Elements(numeric array=w3901) -> (sum=w3902:dbl)
            n1769 = Divide(x=w3918, y=w3906) -> (x/y=w3923:dbl)
            n1770 = Divide(x=w3920, y=w3905) -> (x/y=w3924:dbl)
            n1771 = Divide(x=w3922, y=w3904) -> (x/y=w3925:dbl)
            n1772 = Divide(x=w3902, y=w3897) -> (x/y=w3896:dbl)
            n1773 = Build Array(w3923, w3924, w3925, w3896) -> (w3926:dbl[])
            n1774 = Add Array Elements(numeric array=w3926) -> (sum=w3927:dbl)
            n1775 = Divide(x=w3926, y=w3927) -> (x/y=w3895:dbl[])
            n1776 = Index Array(array=w3895, index=2) -> (element=→"IntR3":dbl)
            n1777 = Index Array(array=w3895, index=1) -> (element=→"IntR2":dbl)
            n1778 = Index Array(array=w3895, index=0) -> (element=→"IntR1":dbl)
            n1779 = Index Array(array=w3895, index=3) -> (element=→"IntR4":dbl)
          }
        }
        n1780 = Add(x=w3849, y=w3877) -> (x+y=w3875:dbl[])
        n1781 = Add(x=w3850, y=w3873) -> (x+y=w3872:dbl[])
        n1782 = Add(x=w3851, y=w3870) -> (x+y=w3869:dbl[])
        n1783 = Less?(x=w3842, y=5.0 ("x")) -> (x < y?=w3840:bool)
        n1784 = Less?(x=w3837, y=5.0 ("x")) -> (x < y?=w3836:bool)
        n1785 = Less?(x=w3833, y=5.0 ("x")) -> (x < y?=w3832:bool)
        n1786 = case shown="False" w3832 {
          tunnel: [u32 16448250 ("Plot.Plot Color") u32 16711680 ("Plot.Plot Color")] -> w3831
          frame False {
          }
          frame True {
          }
        }
        n1787 = case shown="True" "Show BG removed?" {
          tunnel: w3876 -> [w3935 w3951]
          tunnel: w3875 -> [_ w3941]
          tunnel: [w3935 w3950] -> w3868
          tunnel: w3874 -> [w3934 w3949]
          tunnel: [w3934 w3948] -> w3812
          tunnel: w3872 -> [_ w3937]
          tunnel: w3871 -> [w3933 w3947]
          tunnel: [w3933 w3946] -> w3863
          tunnel: w3869 -> [_ w3942]
          tunnel: [w3932 w3945] -> w3819
          tunnel: w3825 -> [_ w3939]
          tunnel: w3824 -> [w3932 w3944]
          frame False {
          }
          frame True {
            n1788 = Insert Into Array(array=w3947, index (row)=1, new element=w3942) -> (w3946:dbl[][])  [unwired: 1 in]
            n1789 = Insert Into Array(array=w3951, index (row)=1, new element=w3941) -> (w3950:dbl[][])  [unwired: 1 in]
            n1790 = Insert Into Array(array=w3949, index (row)=1, new element=w3937) -> (w3948:dbl[][])  [unwired: 1 in]
            n1791 = Insert Into Array(array=w3944, index (row)=1, new element=w3939) -> (w3945:dbl[][])  [unwired: 1 in]
          }
        }
        "Channel 1" <- w3868
        "Channel 2" <- w3812
        "Channel 3" <- w3863
        "Channel 4" <- w3819
        n1792 = case shown="False" w3840 {
          tunnel: [u32 16448250 ("Plot.Plot Color") u32 16711680 ("Plot.Plot Color")] -> w3839
          frame False {
          }
          frame True {
          }
        }
        n1793 = case shown="False" w3836 {
          tunnel: [u32 16448250 ("Plot.Plot Color") u32 16711680 ("Plot.Plot Color")] -> w3835
          frame False {
          }
          frame True {
          }
        }
        n1794 = case shown="False" w3820 {
          tunnel: [u32 16448250 ("Plot.Plot Color") u32 16711680 ("Plot.Plot Color")] -> w3816
          frame False {
          }
          frame True {
          }
        }
        n1795 = case shown="False" "Show BG removed?" {
          tunnel: [u32 16744703 ("Plot.Plot Color") u32 16741120 ("Plot.Plot Color")] -> w3809
          frame False {
          }
          frame True {
          }
        }
        n1796 = property on="Channel 1" class="WFGraph (strict)"("Active Plot"=w3810, "Plot.Plot Color"=w3809, "Plot.Line Style"=u8 1, "Plot.Line Width"=u8 2, "BG Color"=w3839) -> ()  [unwired: 2 in, 2 out]
        n1797 = property on="Channel 2" class="WFGraph (strict)"("Active Plot"=w3810, "Plot.Plot Color"=w3809, "Plot.Line Style"=u8 1, "Plot.Line Width"=u8 2, "BG Color"=w3835) -> ()  [unwired: 2 in, 2 out]
        n1798 = property on="Channel 4" class="WFGraph (strict)"("Active Plot"=w3810, "Plot.Plot Color"=w3809, "Plot.Line Style"=u8 1, "Plot.Line Width"=u8 2, "BG Color"=w3816) -> ()  [unwired: 2 in, 2 out]
        n1799 = property on="Channel 3" class="WFGraph (strict)"("Active Plot"=w3810, "Plot.Plot Color"=w3809, "Plot.Line Style"=u8 1, "Plot.Line Width"=u8 2, "BG Color"=w3831) -> ()  [unwired: 2 in, 2 out]
      }
      frame Error {
        w3952 = u32 16448250 ("Plot Area:Colors:BG Color")
        n1800 = property on="Channel 1" class="WFGraph (strict)"("BG Color"=w3952) -> ()  [unwired: 2 in, 2 out]
        n1801 = property on="Channel 2" class="WFGraph (strict)"("BG Color"=w3952) -> ()  [unwired: 2 in, 2 out]
        n1802 = property on="Channel 3" class="WFGraph (strict)"("BG Color"=w3952) -> ()  [unwired: 2 in, 2 out]
      }
    }
    "DisplayLoop" <- w3802
  }
  n1803 = while {
    tunnel: w72 -> [w3968]
    tunnel: w63 -> [w3967]
    tunnel: [w3966] -> w70
    tunnel: w28 -> [w3965]
    tunnel: [w3964] -> w66
    tunnel: w47 -> [w3962]
    tunnel: w56 -> [w3961]
    tunnel: w43 -> [w3956]
    tunnel: w2 -> [w3955]
    tunnel: [w3954] -> w1
    stop <- w3959 stop-if-true
    # "acquire data and send it to processing loop"
    # "Data Aquisition Loop"
    n1804 = event shown="[1] <Start digitizer>: User Event" {
      selector: w3967 -> [_ _]
      dyn-events: [_ _] -> w3966
      timeout: 30 -> [_ _]
      tunnel: w3968 -> [w3975 w3989]
      tunnel: [w3970 _] -> w3959
      tunnel: w3965 -> [w3974 w3996]
      tunnel: [w3974 w3995] -> w3964
      tunnel: w3962 -> [_ w3993]
      tunnel: w3961 -> [w3973 w3988]
      tunnel: w3956 -> [_ w3986]
      tunnel: w3955 -> [w3969 w3979]
      tunnel: [w3969 w3978] -> w3954
      event Timeout {
        # "use queue to stop data loop\nwhen queue ref is released, error will stop this loop"
        n1805 = event-data() -> ()  [unwired: 1 in, 3 out]
        n1806 = Get Queue Status(queue=w3975) -> (error out=w3972:errorcluster)  [unwired: 2 in, 7 out]
        n1807 = Get Queue Status(queue=w3973) -> (error out=w3971:errorcluster)  [unwired: 2 in, 7 out]
        n1808 = Merge Errors(w3972, w3971) -> (w3970:errorcluster)
      }
      event User Event {
        w3976 = dbl[][] []
        w3994 = enum16{"Write", "Read"}."Read" ("Operation")
        n1809 = event-data() -> ("Time"=→"RunStartTime":u32)  [unwired: 1 in, 3 out]
        n1810 = call "FLImDAQ_FGV.vi"() -> ("Read data"=w3991:T5)  [unwired: 10 in, 1 out]
        n1811 = call "Digitizer1_FGV.vi"("Operation (Read)"=w3994) -> ("Read data"=w3985:refnum<k15>)  [unwired: 9 in, 1 out]
        n1812 = call "Digitizer2_FGV.vi"("Operation (Read)"=w3994) -> ("Read data"=w3992:refnum<k15>)  [unwired: 9 in, 1 out]
        n1813 = Unbundle By Name(w3991) -> ("Waveform to Avg"=w3990:i16)
        n1814 = property on="Property Node" class="niScope"(reference=w3985) -> (reference out=w3984:refnum<k15>, "Vertical Range"=w3983:dbl, "Vertical Offset"=w3982:dbl)  [unwired: 1 in, 1 out]
        n1815 = Tick Count (ms)() -> (millisecond timer value=w3981:u32)
        n1816 = while {
          tunnel: w3996 -> [w4074]
          tunnel: [w4073] -> w3995
          tunnel: w3992 -> [w4067]
          tunnel: w3984 -> [w4066]
          tunnel: w3993 -> [w4065]
          shift-right: [w4037] -> _
          shift-left: u32 0 ("millisecond timer value") -> [w4059]
          tunnel: w3990 -> [w4021]
          tunnel: w3989 -> [w4057]
          tunnel: w3988 -> [w4056]
          tunnel: w3986 -> [w4050]
          tunnel: w3983 -> [w4047]
          tunnel: w3982 -> [w4048]
          shift-right: [w4042] -> _
          shift-left: w3981 -> [w4041]
          tunnel: w3979 -> [w4019]
          tunnel: [w4017] -> w3978
          shift-right: [w4016] -> _
          shift-left: T51 {"V1 out"=0.0, "V2 out"=0.0, "V3 out"=0.0, "V3 out"=0.0} -> [w4015]
          shift-right: [w4011] -> _
          shift-left: w3976 -> [w4005]
          shift-right: [w4008] -> _
          shift-left: w3976 -> [w4002]
          i -> [w4014]
          stop <- w4040 stop-if-true
          w4032 = enum16{"write", "read"}."read" ("action")
          w4060 = 65536
          # "enqueue V"
          # "enqueue ch3&4 data"
          # "enqueue ch1&2 data"
          # "acquire ch3&4"
          # "acquire ch1&2"
          # "send data for gain adjustment"
          n1817 = Multiply(x=w4021, y=w4014) -> (x*y=w4029:i32)
          "Fetch Record #" <- w4029
          n1818 = property on="Property Node" class="niScope"(reference=w4066, "Fetch Record Number"=w4029) -> (reference out=w4078:refnum<k15>, error out=w4077:errorcluster, "Records Done"=w4049:i32)  [unwired: 1 in]
          n1819 = Subtract(x=w4049, y=w4029) -> (x-y=→"Record Backlog":i32)
          n1820 = call-poly <instrlib>:"niScope Fetch (poly).vi"("timeout"=1.0, "error in"=w4077, "channels"="0,1", "instrument handle"=w4078) -> ("error out"=w4026:errorcluster, "wfm"=w4027:i16[][], "wfm info"=w4046:T52)  [unwired: 4 in, 1 out]
          n1821 = property on="Property Node" class="niScope"(reference=w4067, "Fetch Record Number"=w4029) -> (reference out=w4071:refnum<k15>, error out=w4068:errorcluster, "Records Done"=w4030:i32)  [unwired: 1 in]
          n1822 = Divide(x=w4027, y=w4060) -> (x/y=w4036:dbl[][])
          n1823 = Tick Count (ms)() -> (millisecond timer value=w4037:u32)
          n1824 = Subtract(x=w4030, y=w4029) -> (x-y=→"Record Backlog 2":i32)
          n1825 = Subtract(x=w4037, y=w4059) -> (x-y=→"Aquisition loop timing(ms)":u32)
          n1826 = Subtract(x=w4037, y=w4041) -> (x-y=w4045:u32)
          n1827 = Multiply(x=w4036, y=w4047) -> (x*y=w4064:dbl[][])
          n1828 = call-poly <instrlib>:"niScope Fetch (poly).vi"("timeout"=0.25, "error in"=w4068, "channels"="0,1", "instrument handle"=w4071) -> ("error out"=w4025:errorcluster, "wfm"=w4061:i16[][])  [unwired: 4 in, 2 out]
          n1829 = Greater?(x=w4045, y=u32 1000) -> (0:w4043:bool)
          n1830 = Add(x=w4064, y=w4048) -> (x+y=w4010:dbl[][])
          n1831 = case shown="True" w4043 {
            tunnel: w4046 -> [_ w4098]
            tunnel: w4037 -> [_ w4097]
            tunnel: [w4091 w4097] -> w4042
            tunnel: w4041 -> [w4091 _]
            tunnel: [errorcluster {"status"=FALSE, "code"=0, "source"=""} ("error constant") w4094] -> w4038
            frame False {
            }
            frame True {
              # "[Covers: REQ29]"
              n1832 = call "CheckFrequency(SubVI).vi"("wfm info"=w4098) -> ("f (Hz)"=w4096:dbl)  [unwired: 10 in]
              "Laser f (Hz)" <- w4096
              n1833 = local read "Laser Rep Rate"() -> (w4093:dbl)
              n1834 = Increment(x=w4093) -> (x+1=w4092:dbl)
              n1835 = Greater?(x=w4096, y=w4092) -> (0:w4095:bool)
              n1836 = case shown="True" w4095 {
                tunnel: [errorcluster {"status"=FALSE, "code"=0, "source"=""} ("error constant") errorcluster {"status"=TRUE, "code"=0, "source"=""} ("error constant")] -> w4094
                frame False {
                }
                frame True {
                }
              }
            }
          }
          n1837 = Divide(x=w4061, y=w4060) -> (x/y=w4063:dbl[][])
          n1838 = Enqueue Element(queue=w4057, element=w4010, error in (no error)=w4026) -> (error out=w4024:errorcluster)  [unwired: 1 in, 2 out]
          n1839 = Multiply(x=w4063, y=w4047) -> (x*y=w4062:dbl[][])
          n1840 = Add(x=w4062, y=w4048) -> (x+y=w4009:dbl[][])
          n1841 = Enqueue Element(queue=w4056, element=w4009, error in (no error)=w4025) -> (error out=w4023:errorcluster)  [unwired: 1 in, 2 out]
          n1842 = Merge Errors(w4024, w4023) -> (w4022:errorcluster)
          n1843 = call "V1FGV.vi"("Error In"=w4022, "action (write)"=w4032) -> ("Error Out"=w4054:errorcluster, "V1 out"=w4052:dbl)  [unwired: 8 in]
          n1844 = call "V2FGV.vi"("Error In"=w4054, "action(write)"=w4032) -> ("Error Out"=w4053:errorcluster, "V2 out"=w4051:dbl)  [unwired: 8 in]
          n1845 = call "V3FGV.vi"("Error In"=w4053, "action(write)"=w4032) -> ("Error Out"=w4035:errorcluster, "V3 out"=w4034:dbl)  [unwired: 8 in]
          n1846 = call "V4FGV.vi"("Error In"=w4035, "action(write)"=w4032, "V3 in"=w4034) -> ("Error Out"=w4033:errorcluster, "V3 out"=w4031:dbl)  [unwired: 7 in]
          n1847 = Bundle("V1 out"=w4052, "V2 out"=w4051, "V3 out"=w4034, "V3 out"=w4031) -> (w4016:T51)  [unwired: 1 in]
          n1848 = Bundle(w4014, w4010, w4009, w4016) -> (w4020:T53)  [unwired: 1 in]
          n1849 = Enqueue Element(queue=w4050, element=w4016, error in (no error)=w4033) -> (error out=w4018:errorcluster)  [unwired: 1 in, 2 out]
          n1850 = Send Notification(notification=w4020, notifier=w4074, error in (no error)=w4018) -> (notifier out=w4073:refnum<notifier>, error out=w4039:errorcluster)
          n1851 = Delete From Array(array=w4009, length=4, index (row)=0) -> (deleted portion=w4001:dbl[][], array with subset deleted=w4008:dbl[][])  [unwired: 1 in]
          n1852 = Delete From Array(array=w4010, length=4, index (row)=0) -> (deleted portion=w4004:dbl[][], array with subset deleted=w4011:dbl[][])  [unwired: 1 in]
          n1853 = Decrement(x=w4014) -> (x-1=w3998:i32)
          n1854 = Build Array (concatenate)(w4002, w4001) -> (w4000:dbl[][])
          n1855 = Greater Or Equal To 0?(x=w3998) -> (x >= 0?=w3997:bool)
          n1856 = Build Array (concatenate)(w4005, w4004) -> (w4003:dbl[][])
          n1857 = case shown="False" w3997 {
            tunnel: w4019 -> [w4079 w4089]
            tunnel: w4018 -> [_ w4088]
            tunnel: [w4079 w4087] -> w4017
            tunnel: w4015 -> [_ w4086]
            tunnel: w3998 -> [_ w4085]
            tunnel: w4003 -> [_ w4083]
            tunnel: w4000 -> [_ w4082]
            tunnel: [errorcluster {"status"=FALSE, "code"=0, "source"=""} ("error out") w4081] -> w3999
            frame False {
            }
            frame True {
              # "send data for DeCon"
              n1858 = Bundle(w4085, w4083, w4082, w4086) -> (w4084:T53)  [unwired: 1 in]
              n1859 = Send Notification(notification=w4084, notifier=w4089, error in (no error)=w4088) -> (notifier out=w4087:refnum<notifier>, error out=w4081:errorcluster)
            }
          }
          n1860 = Merge Errors(w3999, w4038, w4039) -> (w4055:errorcluster)
          n1861 = case shown="Error .." w4055 {
            selector: w4055 -> [w4101 w4102]
            tunnel: w4065 -> [_ w4105]
            tunnel: [w4101 w4102] -> w4040
            frame No Error {
            }
            frame Error {
              # "Send user event to signal aquisition has stoped"
              n1862 = Generate User Event(priority (normal)=usereventprio."high priority", user event=w4105, event data cluster=TRUE ("event data")) -> ()  [unwired: 1 in, 2 out]
            }
          }
          "aquisition loop Error Out" <- w4040
          "Auisition Loop idx" <- w4014
        }
      }
    }
    n1863 = Unbundle By Name(w3959) -> ("status"=w3958:bool)
    n1864 = Not(x=w3958) -> (.not. x?=w3957:bool)
    n1865 = local write "Aq Loop?"(w3957) -> ()
    "Aq Loop?" <- TRUE ("Aq L?")
  }
  n1866 = disable-structure "Diagram Disable Structure" shown="Disabled" {
    frame Disabled {
      w4106 = T54 {"Horizontal"=500, "Vertical"=100}  # Top Left Corner
      n1867 = Control Help Window(0:w4106, 1:TRUE ("Show")) -> ()
      n1868 = call <vilib>:"TDMS - File Viewer.vi"() -> ()  [unwired: 6 in, 2 out]
    }
    frame Enabled {
    }
  }
  n1869 = while {
    tunnel: w28 -> [w4155]
    shift-right: [w4119] -> _
    shift-left: _ -> [w4151]
    tunnel: [w4110] -> w11 mode=indexing
    i -> [w4135]
    stop <- w4116 stop-if-true
    # "Channel 3"
    # "Channel 2"
    # "Channel 1"
    # "use FGV for gain value"
    # "stop on error"
    # "Gain adjustment and Data processing"
    n1870 = Tick Count (ms)() -> (millisecond timer value=w4119:u32)
    n1871 = Wait on Notification(notifier=w4155, ignore previous (F)=TRUE) -> (notification=w4129:T11, error out=w4109:errorcluster)  [unwired: 2 in, 2 out]
    n1872 = Subtract(x=w4119, y=w4151) -> (x-y=→"PID loop timing(ms)":u32)
    n1873 = Unbundle(w4129) -> ("CH1&2"=w4145:dbl[][], "CH3&4"=w4144:dbl[][])  [unwired: 2 out]
    n1874 = call "SeperateChanData.vi"("Input (Ch1&2)"=w4145) -> ("Ch1"=w4140:dbl[][], "Ch2"=w4138:dbl[][])
    n1875 = call "SeperateChanData.vi"("Input (Ch1&2)"=w4144) -> ("Ch1"=w4134:dbl[][], "Ch2"=w4127:dbl[][])
    n1876 = call "AvgArrayTimeCritical.vi"("2D array"=w4140) -> ("1D Avg"=w4139:dbl[])  [unwired: 10 in]
    n1877 = call "AvgArrayTimeCritical.vi"("2D array"=w4138) -> ("1D Avg"=w4149:dbl[])  [unwired: 10 in]
    n1878 = call "AvgArrayTimeCritical.vi"("2D array"=w4134) -> ("1D Avg"=w4146:dbl[])  [unwired: 10 in]
    n1879 = call "AvgArrayTimeCritical.vi"("2D array"=w4127) -> ("1D Avg"=w4126:dbl[])  [unwired: 10 in]
    n1880 = Array Max & Min(array=w4139) -> (max value=w4137:dbl)  [unwired: 3 out]
    n1881 = Array Max & Min(array=w4149) -> (max value=w4136:dbl)  [unwired: 3 out]
    n1882 = Array Max & Min(array=w4146) -> (max value=w4120:dbl)  [unwired: 3 out]
    n1883 = Array Max & Min(array=w4126) -> (max value=w4124:dbl)  [unwired: 3 out]
    n1884 = local read "Auto gain ch4"() -> (w4125:bool)
    n1885 = local read "Auto gain ch1"() -> (w4143:bool)
    n1886 = local read "Auto gain ch2"() -> (w4142:bool)
    n1887 = local read "Auto gain ch3"() -> (w4141:bool)
    n1888 = case shown="True" w4125 {
      tunnel: w4124 -> [_ w4202]
      tunnel: "V target(1.0)" -> [_ w4200]
      tunnel: [FALSE w4197] -> w4122
      tunnel: [0.0 ("CtrlV") w4192] -> w4123
      frame False {
        # "Manual control"
      }
      frame True {
        # "PID control"
        n1889 = global read "GlobalVariables.vi" "Ch4GainLim(Log)"() -> (w4203:cluster{"GainMax":dbl, "GainMin":dbl})
        n1890 = call-poly <vilib>:"PID.vi"("output range"=w4203, "PID gains"="Ch4 PID gains", "process variable"=w4202, "setpoint"=w4200) -> ("output"=w4201:dbl)  [unwired: 6 in, 1 out]
        n1891 = Power Of 10(x=w4201) -> (10^x=w4193:dbl)
        "Gain4" <- w4193
        n1892 = call "V4FGV.vi"("action(write)"=enum16{"write", "read"}."read") -> ("Error Out"=w4196:errorcluster, "V3 out"=w4198:dbl)  [unwired: 9 in]
        n1893 = call "GainToCtrlV.vi"("Gain"=w4193, "Channel"=enum16{"Ch1", "Ch2", "Ch3", "Ch4"}."Ch4") -> ("CtrlV"=w4192:dbl)  [unwired: 8 in, 1 out]
        n1894 = call "V4FGV.vi"("Error In"=w4196, "V3 in"=w4192) -> ()  [unwired: 8 in, 2 out]
        n1895 = local write "V 4"(w4192) -> ()
        n1896 = Not Equal?(x=w4192, y=w4198) -> (x != y?=w4197:bool)
      }
    }
    n1897 = case shown="True" w4143 {
      tunnel: "V target(1.0)" -> [_ w4217]
      tunnel: w4137 -> [_ w4214]
      tunnel: [0.0 ("CtrlV") w4206] -> w4117
      tunnel: [FALSE w4208] -> w4133
      frame False {
        # "Manual control"
      }
      frame True {
        # "PID control"
        n1898 = global read "GlobalVariables.vi" "Ch1GainLim(Log)"() -> (w4213:cluster{"GainMax":dbl, "GainMin":dbl})
        n1899 = call-poly <vilib>:"PID.vi"("output range"=w4213, "PID gains"="Ch1 PID gains", "process variable"=w4214, "setpoint"=w4217) -> ("output"=w4212:dbl)  [unwired: 6 in, 1 out]
        n1900 = Power Of 10(x=w4212) -> (10^x=w4211:dbl)
        "Gain1" <- w4211
        n1901 = call "V1FGV.vi"("action (write)"=enum16{"write", "read"}."read") -> ("Error Out"=w4207:errorcluster, "V1 out"=w4209:dbl)  [unwired: 9 in]
        n1902 = call "GainToCtrlV.vi"("Gain"=w4211, "Channel"=enum16{"Ch1", "Ch2", "Ch3"}."Ch1") -> ("CtrlV"=w4206:dbl)  [unwired: 8 in, 1 out]
        n1903 = local write "V 1"(w4206) -> ()
        n1904 = call "V1FGV.vi"("Error In"=w4207, "V1 in"=w4206) -> ()  [unwired: 8 in, 2 out]
        n1905 = Not Equal?(x=w4206, y=w4209) -> (x != y?=w4208:bool)
      }
    }
    n1906 = case shown="True" w4142 {
      tunnel: w4136 -> [_ w4244]
      tunnel: "V target(1.0)" -> [_ w4245]
      tunnel: [FALSE w4238] -> w4132
      tunnel: [0.0 ("CtrlV") w4234] -> w4128
      frame False {
        # "Manual control"
      }
      frame True {
        # "PID control"
        n1907 = global read "GlobalVariables.vi" "Ch2GainLim(Log)"() -> (w4242:cluster{"GainMax":dbl, "GainMin":dbl})
        n1908 = call-poly <vilib>:"PID.vi"("output range"=w4242, "PID gains"="Ch2 PID gains", "process variable"=w4244, "setpoint"=w4245) -> ("output"=w4241:dbl)  [unwired: 6 in, 1 out]
        n1909 = Power Of 10(x=w4241) -> (10^x=w4239:dbl)
        "Gain2" <- w4239
        n1910 = call "V2FGV.vi"("action(write)"=enum16{"write", "read"}."read") -> ("Error Out"=w4235:errorcluster, "V2 out"=w4236:dbl)  [unwired: 9 in]
        n1911 = call "GainToCtrlV.vi"("Gain"=w4239, "Channel"=enum16{"Ch1", "Ch2", "Ch3"}."Ch2") -> ("CtrlV"=w4234:dbl)  [unwired: 8 in, 1 out]
        n1912 = local write "V 2"(w4234) -> ()
        n1913 = call "V2FGV.vi"("Error In"=w4235, "V2 in"=w4234) -> ()  [unwired: 8 in, 2 out]
        n1914 = Not Equal?(x=w4234, y=w4236) -> (x != y?=w4238:bool)
      }
    }
    n1915 = case shown="True" w4141 {
      tunnel: w4120 -> [_ w4229]
      tunnel: "V target(1.0)" -> [_ w4226]
      tunnel: [FALSE w4222] -> w4131
      tunnel: [0.0 ("CtrlV") w4220] -> w4130
      frame False {
        # "Manual control"
      }
      frame True {
        # "PID control"
        n1916 = global read "GlobalVariables.vi" "Ch3GainLim(Log)"() -> (w4230:cluster{"GainMax":dbl, "GainMin":dbl})
        n1917 = call-poly <vilib>:"PID.vi"("output range"=w4230, "PID gains"="Ch3 PID gains", "process variable"=w4229, "setpoint"=w4226) -> ("output"=w4228:dbl)  [unwired: 6 in, 1 out]
        n1918 = Power Of 10(x=w4228) -> (10^x=w4225:dbl)
        "Gain3" <- w4225
        n1919 = call "V3FGV.vi"("action(write)"=enum16{"write", "read"}."read") -> ("Error Out"=w4221:errorcluster, "V3 out"=w4223:dbl)  [unwired: 9 in]
        n1920 = call "GainToCtrlV.vi"("Gain"=w4225, "Channel"=enum16{"Ch1", "Ch2", "Ch3"}."Ch3") -> ("CtrlV"=w4220:dbl)  [unwired: 8 in, 1 out]
        n1921 = local write "V 3"(w4220) -> ()
        n1922 = call "V3FGV.vi"("Error In"=w4221, "V3 in"=w4220) -> ()  [unwired: 8 in, 2 out]
        n1923 = Not Equal?(x=w4220, y=w4223) -> (x != y?=w4222:bool)
      }
    }
    n1924 = call "LabJack_FGV.vi"("Operation(Read)"=enum16{"Write", "Read"}."Read" ("Operation"), "error in (no error)"=w4109) -> ("error out"=w4118:errorcluster, "Read data"=w4153:i32)  [unwired: 8 in]
    n1925 = flat-sequence {
      tunnel: [w4157] -> w4115
      tunnel: w4109 -> [_]
      frame #0 {
        n1926 = Tick Count (ms)() -> (millisecond timer value=w4157:u32)
      }
    }
    n1927 = case "Channel 1" shown="True" w4133 {
      tunnel: w4118 -> [w4183 w4189]
      tunnel: w4153 -> [w4182 w4188]
      tunnel: [w4183 w4184] -> w4113
      tunnel: [w4182 w4187] -> w4148
      tunnel: w4117 -> [_ w4185]
      frame False {
        # "Do nothing"
      }
      frame True {
        # "request V\nupdate FGV"
        n1928 = global read "GlobalVariables.vi" "Ch1 LJ pin"() -> (w4186:string)
        n1929 = call "LJM_eWriteName.vi"("Handle In"=w4188, "Name"=w4186, "Value"=w4185, "error in"=w4189) -> ("Handle Out"=w4187:i32, "error out"=w4184:errorcluster)  [unwired: 10 in]
      }
    }
    n1930 = case "Channel 2" shown="True" w4132 {
      tunnel: w4113 -> [w4174 w4181]
      tunnel: [w4174 w4176] -> w4112
      tunnel: w4148 -> [w4175 w4180]
      tunnel: [w4175 w4179] -> w4147
      tunnel: w4128 -> [_ w4177]
      frame False {
        # "Do nothing"
      }
      frame True {
        # "request V\nupdate FGV"
        n1931 = global read "GlobalVariables.vi" "Ch2 LJ pin"() -> (w4178:string)
        n1932 = call "LJM_eWriteName.vi"("Handle In"=w4180, "Name"=w4178, "Value"=w4177, "error in"=w4181) -> ("Handle Out"=w4179:i32, "error out"=w4176:errorcluster)  [unwired: 10 in]
      }
    }
    n1933 = case "Channel 3" shown="True" w4131 {
      tunnel: w4112 -> [w4167 w4173]
      tunnel: [w4167 w4169] -> w4111
      tunnel: w4147 -> [w4166 w4172]
      tunnel: w4130 -> [_ w4170]
      tunnel: [w4166 w4168] -> w4121
      frame False {
        # "Do nothing"
      }
      frame True {
        # "request V\nupdate FGV"
        n1934 = global read "GlobalVariables.vi" "Ch3 LJ pin"() -> (w4171:string)
        n1935 = call "LJM_eWriteName.vi"("Handle In"=w4172, "Name"=w4171, "Value"=w4170, "error in"=w4173) -> ("Handle Out"=w4168:i32, "error out"=w4169:errorcluster)  [unwired: 10 in]
      }
    }
    n1936 = case "Channel 4" shown="True" w4122 {
      tunnel: w4111 -> [w4159 w4165]
      tunnel: w4121 -> [w4158 w4164]
      tunnel: [w4159 w4160] -> w4116
      tunnel: [w4158 w4163] -> _
      tunnel: w4123 -> [_ w4161]
      frame False {
        # "Do nothing"
      }
      frame True {
        # "request V\nupdate FGV"
        n1937 = global read "GlobalVariables.vi" "Ch4 LJ pin"() -> (w4162:string)
        n1938 = call "LJM_eWriteName.vi"("Handle In"=w4164, "Name"=w4162, "Value"=w4161, "error in"=w4165) -> ("Handle Out"=w4163:i32, "error out"=w4160:errorcluster)  [unwired: 10 in]
      }
    }
    "PID loop error out" <- w4116
    n1939 = flat-sequence {
      tunnel: [w4156] -> w4114
      tunnel: w4116 -> [_]
      frame #0 {
        n1940 = Tick Count (ms)() -> (millisecond timer value=w4156:u32)
      }
    }
    n1941 = Subtract(x=w4114, y=w4115) -> (x-y=w4110:u32)
    "LJ process (ms)" <- w4110
    "PID loop" <- w4135
  }
  "LJ time(ms)" <- w11
  n1942 = Unregister For Events(event registration refnum=w54, error in=w14) -> (error out=w60:errorcluster)
  n1943 = Destroy User Event(user event=w47, error in=w60) -> (error out=w13:errorcluster)
  n1944 = Close File(refnum=w30, error in=w13) -> ()  [unwired: 2 out]
  n1945 = Release Notifier(notifier=w25, error in (no error)=w57) -> (error out=w58:errorcluster)  [unwired: 1 in, 2 out]
  n1946 = Release Notifier(notifier=w26, error in (no error)=w46) -> (error out=w51:errorcluster)  [unwired: 1 in, 2 out]
  n1947 = call <vilib>:"Simple Error Handler.vi"("error in (no error)"=w58) -> ()  [unwired: 4 in, 5 out]
  n1948 = call <vilib>:"Simple Error Handler.vi"("error in (no error)"=w51) -> ()  [unwired: 4 in, 5 out]
  n1949 = Release Notifier(notifier=w66, error in (no error)=w65) -> (error out=w4:errorcluster)  [unwired: 1 in, 2 out]
  n1950 = Release Notifier(notifier=w1, error in (no error)=w6) -> (error out=w5:errorcluster)  [unwired: 1 in, 2 out]
  n1951 = Unregister For Events(event registration refnum=w70, error in=w68) -> (error out=w69:errorcluster)
  n1952 = Merge Errors(w4, w5) -> (w3:errorcluster)
  n1953 = Destroy User Event(user event=w61, error in=w69) -> ()  [unwired: 1 out]
  n1954 = call <vilib>:"Simple Error Handler.vi"("error in (no error)"=w3) -> ()  [unwired: 4 in, 5 out]
